vi "main4ChBK20240509.vi"() -> ()   [LabVIEW 2024]
doc: "Main VI for FLS imaging system."
uses:
  SubVI/DigitizerConfiguration/FLImDAQ.ctl
  <instrlib>/niScope/Controls/niScope trigger source.ctl
  SubVI/LabJack/LJ Pin Setting.ctl
  ConfigFiles/AimingBeamVideoConfig.ctl
  LaguerreDeconLib/DeconEngineClass/LaguerreDeconEngineClass.lvclass/LaguerreDeconEngineClass.ctl
  <vilib>/Utility/error.llb/DialogType.ctl
  LaguerreDeconLib/DeconEngineClass/LaguerreDeconEngineClass.lvclass
  <vilib>/event_ctls.llb/usereventprio.ctl
  <vilib>/Utility/miscctls.llb/LVMinMaxIncTypeDef.ctl
  SubVI/APD/APDClass.lvclass
  <vilib>/Analysis/baseanly.llb/Mean (DBL).vi
  SubVI/GlobalVariables.vi
  <vilib>/addons/control/pid/pid.llb/PID (DBL).vi
  <instrlib>/niScope/Acquire/Fetch/niScope Multi Fetch Binary 16.vi
  <vilib>/Instr/_visa.llb/VISA Configure Serial Port (Instr).vi
  <userlib>/_OpenG.lib/file/file.llb/openg_file.lvlib
  <userlib>/_OpenG.lib/time/time.llb/openg_time.lvlib
  <vilib>/Analysis/NI_AALBase.lvlib
  <vilib>/Utility/miscctls.llb/LVPointTypeDef.ctl
  <vilib>/addons/control/pid/NI_PID_pid.lvlib
panel:
  out "Record Backlog 2":i32
  in  "Auto gain ch4":bool=TRUE caption="Auto gain ch3"
  in  "V 4":dbl caption="Gain 3" min=0.0 max=4.67 step=0.1
  out "Gain4":dbl
  out "Lifetime 4":dbl caption="Lifetime 3"
  out "IntR4":dbl format="%#_2g"
  out "SNR4":dbl format="%#_3g"
  out "Channel 4":dbl[][](graph) caption="Channel 3"
  out "RunStartTime":u32
  out "Dig1 Temp":dbl
  out "Dig2 Temp":dbl
  out "Visualization PC video source":T1
  in  "V target(1.0)":dbl=1.0 caption="V target(1.5)" min=0.3 max=1.5 step=0.1 format="%#_4g"
  out "SNR3":dbl format="%#_3g"
  out "SNR2":dbl format="%#_3g"
  out "SNR1":dbl format="%#_3g"
  in  "Show BG removed?":bool=TRUE
  out "IntR3":dbl format="%#_2g"
  out "IntR2":dbl format="%#_2g"
  out "IntR1":dbl format="%#_2g"
  in  "Video Display":bool
  out "Gain3":dbl
  out "Gain2":dbl
  out "Gain1":dbl
  in  "Skip Data Save?":bool
  out "Aq Loop?":bool
  out "ML?":bool
  out "aquisition loop Error Out":errorcluster
  out "Laser f (Hz)":dbl
  out "Record Backlog":i32
  out "Fetch Record #":i32
  out "Sync Success?":bool
  out "Disclamer":picture
  out "Calibration #":i8
  out "BG #":i8
  in  "TCP Connect":bool
  out "Help":string
  in  "355nm Laser toggle":bool caption="355nm 460Hz"
  in  "Cali&iRF alignment":bool
  in  "Background":bool
  in  "Aiming beam toggle":bool caption="445nm 0Hz 18mA"
  out "Lifetime 3":dbl
  out "Lifetime 2":dbl
  in  "Auto gain ch3":bool=TRUE
  in  "Auto gain ch2":bool=TRUE
  in  "Auto gain ch1":bool=TRUE
  out "Run #":i8
  in  "StopButton":bool caption="Stop"
  out "Aquisition Status:":bool
  in  "StartButton":bool caption="Start"
  in  "V 3":dbl caption="Gain 3" min=0.0 max=4.68 step=0.1
  in  "V 2":dbl caption="Gain 2" min=0.0 max=4.62 step=0.1
  out "Lifetime 1":dbl
  in  "V 1":dbl caption="Gain 1" min=0.0 max=4.66 step=0.1 format="%#_4g"
  in  "Video Source":enum32{"Camera", "FrameGrabber"}(radio)
  out "Case #":string
  out "System Hardware Connection Status":T2
  out "Channel 3":dbl[][](graph)
  out "Channel 2":dbl[][](graph)
  out "Channel 1":dbl[][](graph)
  in  "Tab Control":T3(tab)
  out "display loop timing(ms)":u32
  out "Aquisition loop timing(ms)":u32 format="%.2f"
  out "DisplayLoop":i32
  out "PID loop":i32 caption="processing loop"
  out "PID loop timing(ms)":u32 caption="processing loop timing(ms)"
  out "Communication loop(ms)":u32
  out "laser EM lamp V":dbl format="%0.6f"
  out "Decon Loop timing (ms)":dbl
  out "Auisition Loop idx":i32
  out "LJ process (ms)":u32
  out "LJ time(ms)":u32[](array[numeric])
  out "output variable":i32
  out "Lifetime (ns)":dbl(graph)
  out "Waveform Chart":dbl(graph)
  in  "Truncation":u32=600
  out "iRF Graph":dbl[][](graph)
  in  "Show BG":bool
  out "iRF length":i32
  out "BG length":i32
  out "data length":i32
  out "SysConfigCluster":T4
  out "LJ Pinout":T5={"Ch1 Bias"="DAC0", "Ch2 Bias"="DAC1", "Ch3 Bias"="DAC2", "Ch4 Bias"="DAC0", "355 PWM"="FIO0", "AimingBeam PWM"="FIO2", "Laser Ready"="FIO3", "Interlock"="FIO1", "Laser Start/Stop"="FIO1", "Red LED"="FIO1", "Green LED"="DIO3", "Foot Pedal"="DIO15"}
  out "FLImDAQ":T6={"Digitizer 1"="", "Digitizer 2"="", "Channel"=enum."Channel 0", "trigger source"="VAL_EXTERNAL", "trigger level"=0.5, "trigger delay"=1.35e-07, "min sample rate"=12500000000.0, "min record length"=2500, "vertical range"=1.0, "vertical offset"=-0.25, "Waveform to Avg"=2000} caption="FLIm DAQ Configuration" {"trigger delay" format="%^#.4e"; "trigger level" min=0.0 max=3.5 step=0.5 format="%.2f"; "vertical offset" format="%.4f"; "vertical range" format="%.2f"; "min sample rate" format="%#.2p"}
  in  "Sys Reconfig":bool
  out "data out(communcation loop)":string
  out "PID loop error out":errorcluster caption="processing Error Out"
  out "decon error out":errorcluster
  out "Laser Rep Rate":dbl
  out "V4 Size":i32 caption="V3 Size"
  in  "Data Class":enum16{"Data", "BG", "Cali"}(ring)
  out "V1 Size":i32
  out "V2 Size":i32
  out "V3 Size":i32
  out "data Size":i32[](array[numeric])
  out "State log":string
  in  "Ch4 PID gains":T8={"proportional gain (Kc)"=30.0, "integral time (Ti, min)"=0.0003, "derivative time (Td, min)"=1e-05}
  in  "Ch3 PID gains":T8={"proportional gain (Kc)"=30.0, "integral time (Ti, min)"=0.0003, "derivative time (Td, min)"=1e-05}
  in  "Ch2 PID gains":T8={"proportional gain (Kc)"=30.0, "integral time (Ti, min)"=0.0003, "derivative time (Td, min)"=1e-05}
  in  "Ch1 PID gains":T8={"proportional gain (Kc)"=30.0, "integral time (Ti, min)"=0.0003, "derivative time (Td, min)"=1e-05}
  in  "Quit":bool
  in  "Radio Buttons":T9(radio)=enum."Ch2" caption="DeCon Chan"
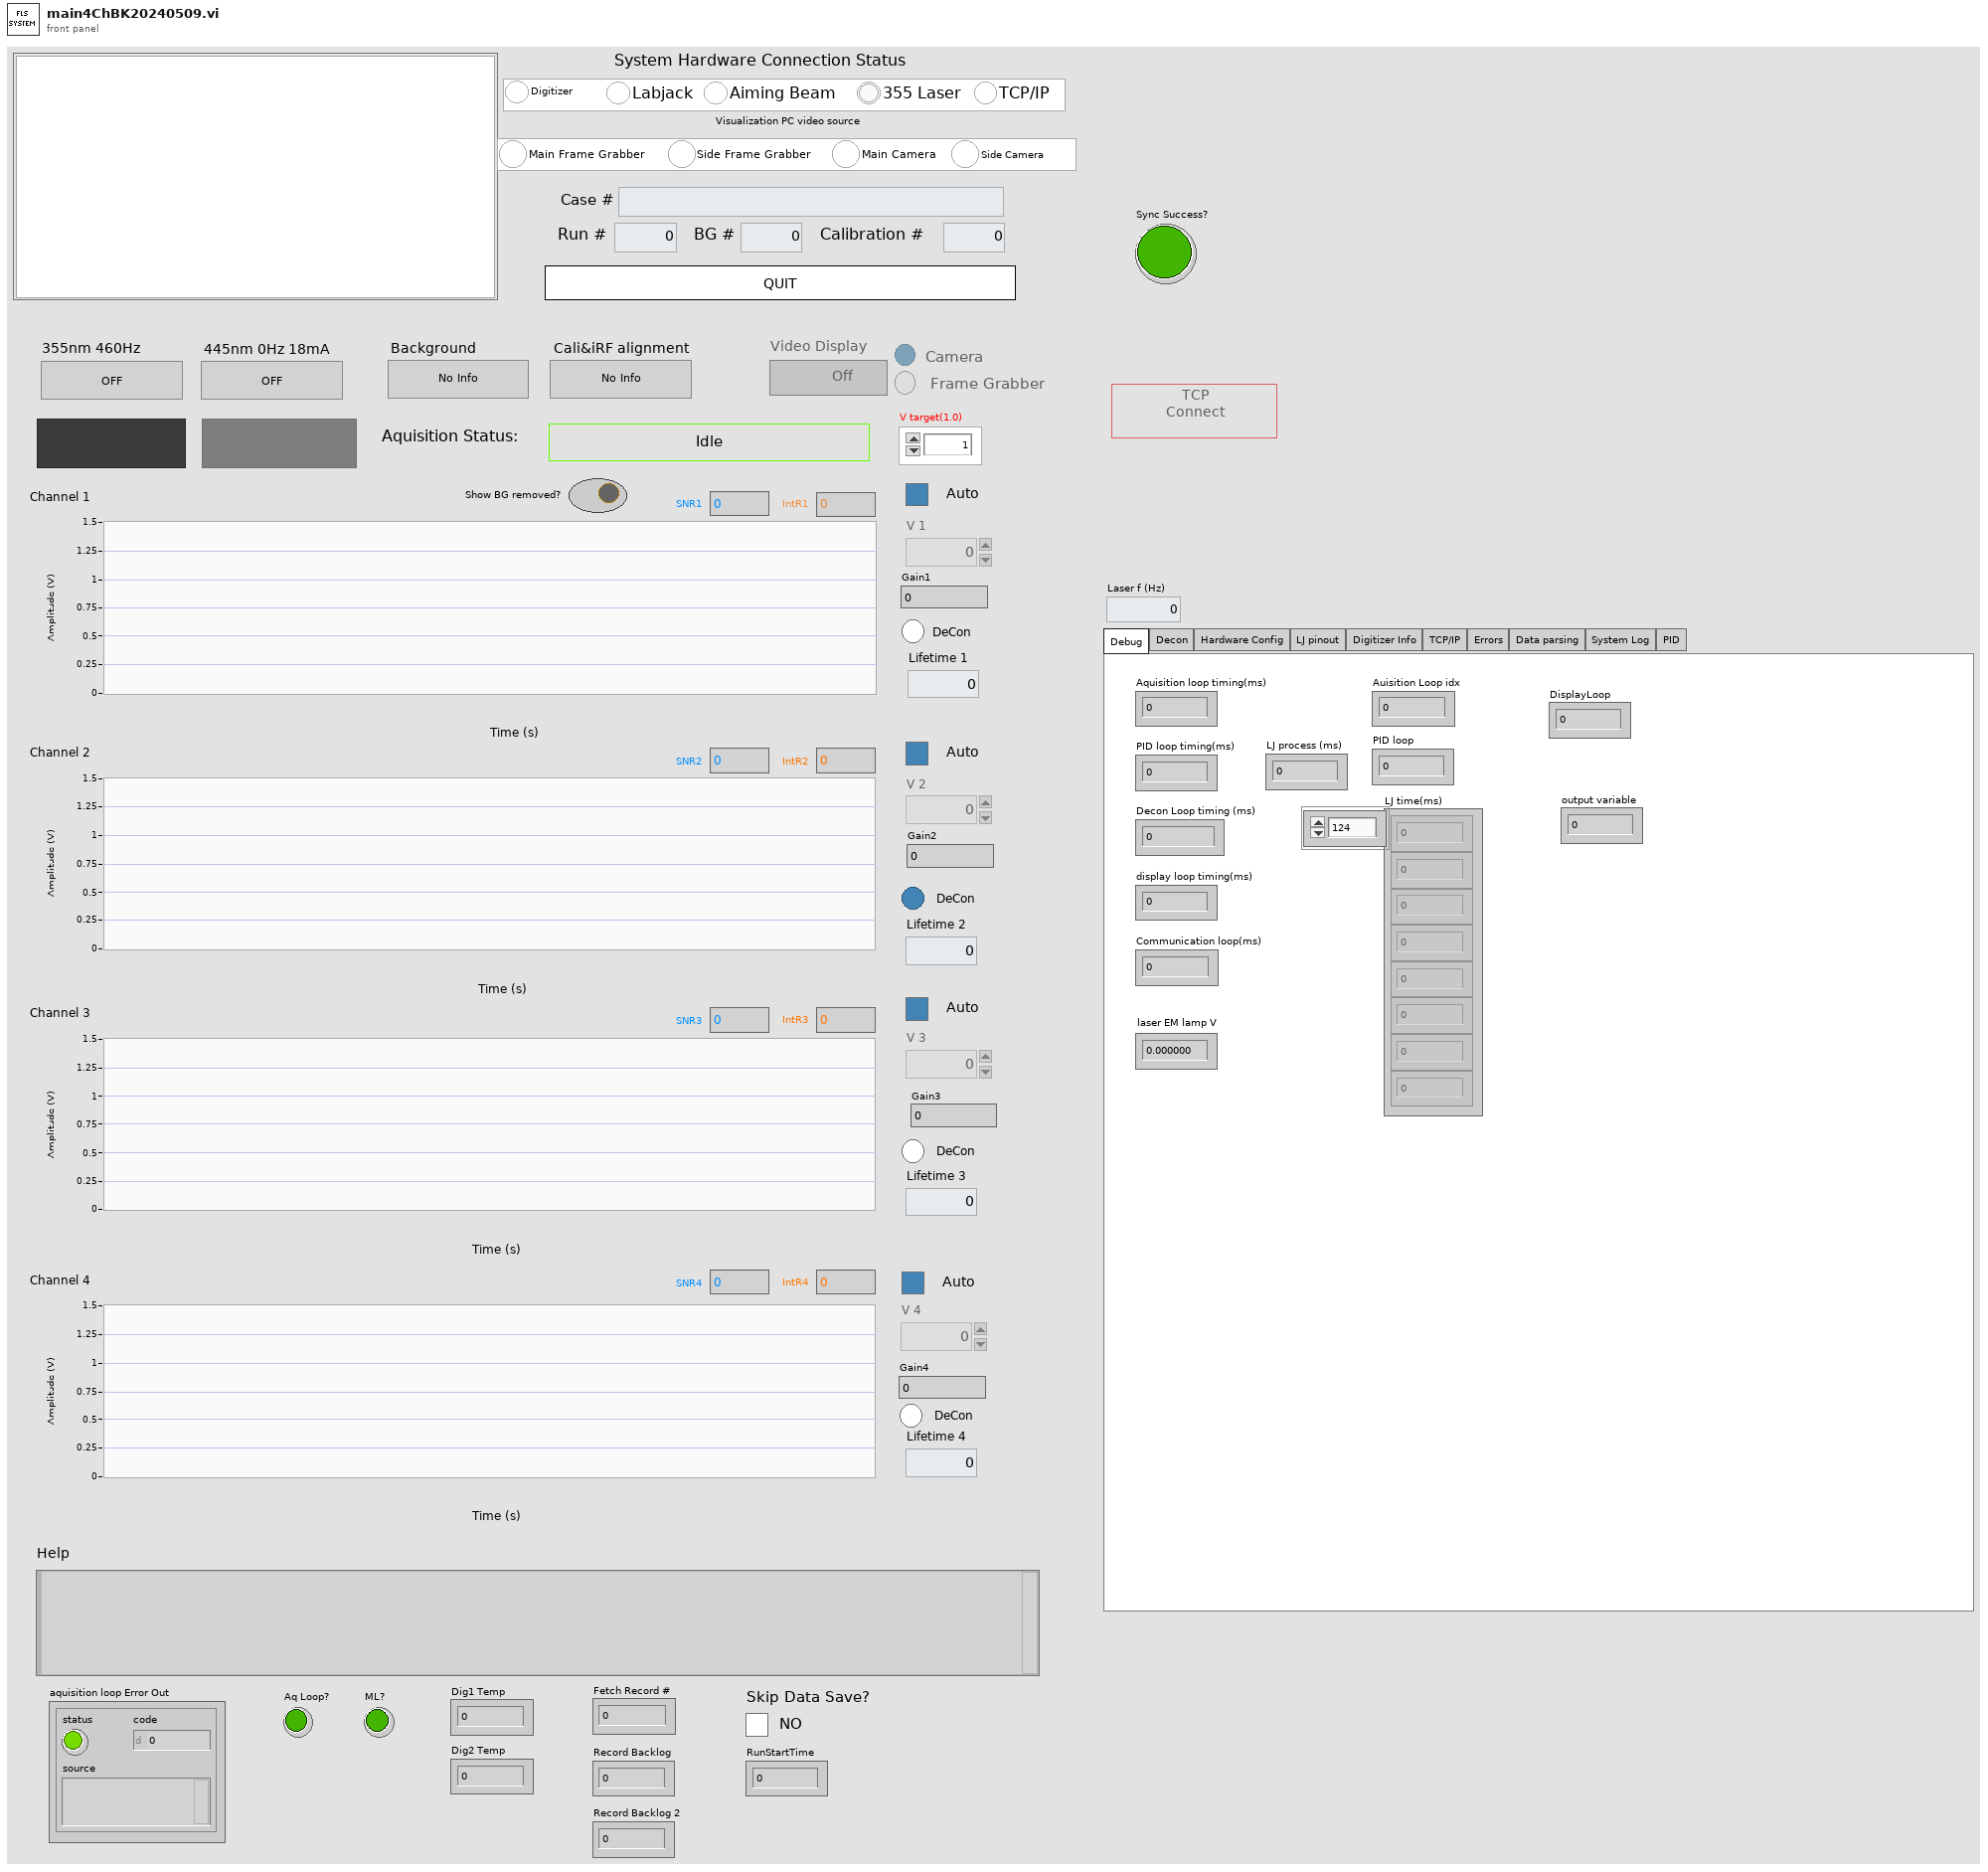
[diagram p1: front panel]
types:
  T1 = cluster{"Main Frame Grabber":bool, "Side Frame Grabber":bool, "Main Camera":bool, "Side Camera":bool}
  T2 = cluster{"Digitizer":bool, "Labjack":bool, "Aiming Beam":bool, "355 Laser":bool, "TCP/IP":bool}
  T3 = enum32{"Debug", "Decon", "Hardware Config", "LJ pinout", "Digitizer Info", "TCP/IP", "Errors", "Data parsing", "System Log", "PID"}
  T4 = cluster{"Ch1Enable?":bool, "Ch2Enable?":bool, "Ch3Enable?":bool, "Ch1AutoGain?":bool, "Ch2AutoGain?":bool, "Ch3AutoGain?":bool, "AimingBeamEnable?":bool}
  T5 = typedef "LJ Pin Setting.ctl" = cluster{"Ch1 Bias":string, "Ch2 Bias":string, "Ch3 Bias":string, "Ch4 Bias":string, "355 PWM":string, "AimingBeam PWM":string, "Laser Ready":string, "Interlock":string, "Laser Start/Stop":string, "Red LED":string, "Green LED":string, "Foot Pedal":string}
  T6 = typedef "FLImDAQ.ctl" = cluster{"Digitizer 1":refnum<k15>, "Digitizer 2":refnum<k15>, "Channel":enum16{"Channel 0", "Channel 1", "Channel 0&1"}, "trigger source":T7, "trigger level":dbl, "trigger delay":dbl, "min sample rate":dbl, "min record length":i32, "vertical range":dbl, "vertical offset":dbl, "Waveform to Avg":i16}
  T7 = typedef "niScope trigger source.ctl" = string
  T8 = cluster{"proportional gain (Kc)":dbl, "integral time (Ti, min)":dbl, "derivative time (Td, min)":dbl}
  T9 = enum32{"No Selection", "Ch1", "Ch2", "Ch3", "Ch4"}
  T10 = cluster{"remote start event":refnum<user-event>, "remote stop  event":refnum<user-event>}
  T11 = enum8{"Enabled", "Disabled", "Disabled and Grayed Out"}
  T12 = enum16{"open", "replace", "create", "open or create", "replace or create", "replace or create with confirmation"}
  T13 = cluster{"CH1":dbl[][], "CH2":dbl[][], "CH3":dbl[][], "CH4":dbl[][], "Gain cluster":cluster{"V1":dbl, "V2":dbl, "V3":dbl, "V4":dbl}}
  T14 = cluster{"idx":i32, "CH1&2":dbl[][], "CH3":dbl[][], "V cluster":cluster{"V1":dbl, "V2":dbl, "V3":dbl, "V4":dbl}}
  T15 = typedef "usereventprio.ctl" = enum32{"high priority", "normal priority"}
  T16 = cluster{"actualSamples":i32, "absoluteInitialX":dbl, "relativeInitialX":dbl, "xIncrement":dbl, "offset":dbl, "gain":dbl, "reserved1":dbl, "reserved2":dbl}[]
  T17 = cluster{"V1 out":dbl, "V2 out":dbl, "V3 out":dbl, "V3 out":dbl}
  T18 = cluster{i32, dbl[][], dbl[][], cluster{"V1 out":dbl, "V2 out":dbl, "V3 out":dbl, "V3 out":dbl}}
  T19 = cluster{"Ch1 iRF":dbl[], "Ch2 iRF":dbl[], "Ch3 iRF":dbl[], "Ch4 iRF":dbl[]}
  T20 = enum16{"open", "open or create", "create or replace", "create", "open (read-only)"}
  T21 = enum32{"Invalid", "Standard", "Closed", "Hidden", "Minimized", "Maximized"}
  T22 = enum32{"invalid app kind", "Development System", "Run Time System", "Student Edition", "Embedded LabVIEW", "Evaluation", "Custom"}
  T23 = enum32{"Bad", "Idle", "Run top level", "Running"}
  T24 = enum16{"Standard", "Buffered", "CRLF", "Immediate"}
  T25 = typedef "AimingBeamVideoConfig.ctl" = cluster{"DeCon Channel":enum16{"1", "2", "3"}, "Scale Bar":bool, "Scale Low":dbl, "Scale High":dbl, "ANSI":dbl, "Radius":dbl, "3D?":bool, "Firefly?":bool, "Pentero?":bool}
  T26 = cluster{"Core":cluster{"Current VI Reference":refnum<vi>, "Close Panel on Exit?":bool}, "SysConfigCluster":cluster{"Ch1Enable?":bool, "Ch2Enable?":bool, "Ch3Enable?":bool, "Ch1AutoGain?":bool, "Ch2AutoGain?":bool, "Ch3AutoGain?":bool, "AimingBeamEnable?":bool}, "System Status":cluster{"Digitizer":bool, "Labjack":bool, "Aiming Beam":bool, "355 Laser":bool, "TCP/IP":bool}, "IDs":cluster{"RunID":i8, "BG ID":i8, "Cali ID":i8}, "CaseID":string, "DefaultPath":path, "Pathes":cluster{"DataPath":path, "BG Path":path, "iRFPath":path, "CaliPath":path}, "FLImDAQ":cluster{"resource name":refnum<k15>, "resource name 2":refnum<k15>, "Channel":enum16{"Channel 0", "Channel 1", "Channel 0&1"}, "trigger source":T7, "trigger level":dbl, "trigger delay":dbl, "min sample rate":dbl, "min record length":i32, "vertical range":dbl, "vertical offset":dbl, "Waveform to Avg":i32}, "SysRunning?":bool, "AB Cluster":cluster{"Aiming Beam COM Port":refnum<visa-resource-name>, "Min Current":dbl, "Max Current":dbl, "Default Current":dbl, "Freq":i32}, "LJ Pinout":T5, "355 PWM setting":cluster{"DIO_EF_CLOCK1_DIVISOR":i16, "DIO_EF_CLOCK1_ROLL_VALUE":i32, "DIO#_EF_INDEX":i16, "DIO#_EF_OPTIONS":i16, "DIO#_EF_CONFIG_A":i32}, "AB PWM setting":cluster{"DIO_EF_CLOCK1_DIVISOR":i16, "DIO_EF_CLOCK1_ROLL_VALUE":i32, "DIO#_EF_INDEX":i16, "DIO#_EF_OPTIONS":i16, "DIO#_EF_CONFIG_A":i32}, "Last Trigger":u32, "niTClk sessions":refnum<k20>[], "Laser start tic":u32, "TCP attempt count":i32, "Ch1Data":dbl[][], "Ch2Data":dbl[][], "Ch3Data":dbl[][], "Ch4Data":dbl[][], "V1":dbl[], "V2":dbl[], "V3":dbl[], "V4":dbl[], "SlowTimer":u32, "FastTimer":u32, "listener ID":refnum<k5>, "TempPath":path, "CaliPath":path, "LED vi reference":refnum<vi>, "Aquisition Timer":u32, "APDSerialNum":cluster{"Ch1APDSerial#":string, "Ch2APDSerial#":string, "Ch3APDSerial#":string, "Ch4APDSerial#":string}, "VideoConfig":T25, "LED vi ref open?":bool, "video source":cluster{"Main Frame Grabber":bool, "Side Frame Grabber":bool, "Main Camera":bool, "Side Camera":bool}, "bothVidSourceAvail":bool}
  T27 = typedef "LVCursorListTypeDef.ctl" = cluster{"Name":string, "Color":u32, "Style":u8, "Point Style":u8, "Name Visible":bool, "Allow Drag":bool, "Cursor Mode":u32, "Plot":i32, "Index":i32, "Position":cluster{"X":dbl, "Y":dbl}, "X Scale":u32, "Y Scale":u32, "Watch Plots":i32[], "Watch All Plots":bool, "Plot Area":i32, "Label Offset":cluster{"X":dbl, "Y":dbl}}[]
  T28 = cluster{"Name":string, "Color":u32, "Style":u8, "Point Style":u8, "Name Visible":bool, "Allow Drag":bool, "Cursor Mode":u32, "Plot":i32, "Index":i32, "Position":cluster{"X":dbl, "Y":dbl}, "X Scale":u32, "Y Scale":u32, "Watch Plots":i32[], "Watch All Plots":bool, "Plot Area":i32, "Label Offset":cluster{"X":dbl, "Y":dbl}}
  T29 = cluster{"Ch1APDSerial#":string, "Ch2APDSerial#":string, "Ch3APDSerial#":string, "Ch4APDSerial#":string}
  T30 = cluster{"DataPath":path, "BG Path":path, "iRFPath":path, "CaliPath":path}
  T31 = cluster{"DIO_EF_CLOCK1_DIVISOR":i16, "DIO_EF_CLOCK1_ROLL_VALUE":i32, "DIO#_EF_INDEX":i16, "DIO#_EF_OPTIONS":i16, "DIO#_EF_CONFIG_A":i32}
  T32 = cluster{"Aiming Beam COM Port":refnum<visa-resource-name>, "Min Current":dbl, "Max Current":dbl, "Default Current":dbl, "Freq":i32}
  T33 = cluster{"resource name":refnum<k15>, "resource name 2":refnum<k15>, "Channel":enum16{"Channel 0", "Channel 1", "Channel 0&1"}, "trigger source":T7, "trigger level":dbl, "trigger delay":dbl, "min sample rate":dbl, "min record length":i32, "vertical range":dbl, "vertical offset":dbl, "Waveform to Avg":i32}
  T34 = cluster{"Current VI Reference":refnum<vi>, "Close Panel on Exit?":bool}
  T35 = cluster{"Channel 1":dbl[], "Channel 2":dbl[], "Channel 3":dbl[], "Channel 4":dbl[]}
  T36 = cluster{"V 1":dbl[], "V 2":dbl[], "V 3":dbl[], "V 4":dbl[]}
  T37 = cluster{"Ch1 WF":dbl[], "Ch2 WF":dbl[], "Ch3 WF":dbl[], "Ch4 WF":dbl[], "V1":dbl, "V2":dbl, "V3":dbl, "V4":dbl}
  T38 = typedef "iRFData.ctl" = cluster{"dt":dbl, "NumOfWFs":i32, "WFLength":i32, "iRFCtrlV":dbl[], "iRFWFsAvg":dbl[][], "iRFRaw":dbl[][]}
  T39 = cluster{"mean":dbl, "mean":dbl, "mean":dbl, "mean":dbl}
  T40 = cluster{"V1":dbl, "V2":dbl, "V3":dbl, "V4":dbl}[]
  T41 = cluster{"DataPath":path, "CaseID":string, "RunID":i16, "Ch1Data":dbl[][], "Ch2Data":dbl[][], "Ch3Data":dbl[][], "Ch4Data":dbl[][], "V1":dbl[], "V2":dbl[], "V3":dbl[], "V4":dbl[], "LaserRepRate":u16, "WFAverage":i16, "RunStartTime":u64}
  T42 = typedef "DialogType.ctl" = u16
  T43 = typedef "LJ PWM Setting.ctl" = cluster{"DIO_EF_CLOCK1_DIVISOR":i16, "DIO_EF_CLOCK1_ROLL_VALUE":i32, "DIO#_EF_INDEX":i16, "DIO#_EF_OPTIONS":i16, "DIO#_EF_CONFIG_A":i32}
  T44 = typedef "AimingBeam.ctl" = cluster{"Aiming Beam COM Port":refnum<visa-resource-name>, "Min Current":dbl, "Max Current":dbl, "Default Current":dbl, "Frequency(Hz)":u32}
  T45 = cluster{"DC1":i32, "DC2":i32, "BG1":i32, "BG2":i32}
  T46 = typedef "LVMinMaxIncTypeDef.ctl" = cluster{"Minimum":dbl, "Maximum":dbl, "Increment":dbl}
  T47 = typedef "LVBoundsTypeDef.ctl" = cluster{"Width":u32, "Height":u32}
  T48 = typedef "imagedata.ctl" = cluster{"image type":i32, "image depth":i32, "image":u8[], "mask":u8[], "colors":u32[], "Rectangle":cluster{"left":i16, "top":i16, "right":i16, "bottom":i16}}
  T49 = cluster{"DC Idx1":i32, "DC Idx2":i32, "BG Idx1":i32, "BG Idx2":i32}
  T50 = cluster{dbl[][], dbl[][], dbl[][], dbl[][], "V cluster":cluster{"V1":dbl, "V2":dbl, "V3":dbl, "V4":dbl}}
  T51 = typedef "LVPointTypeDef.ctl" = cluster{"Horizontal":i16, "Vertical":i16}
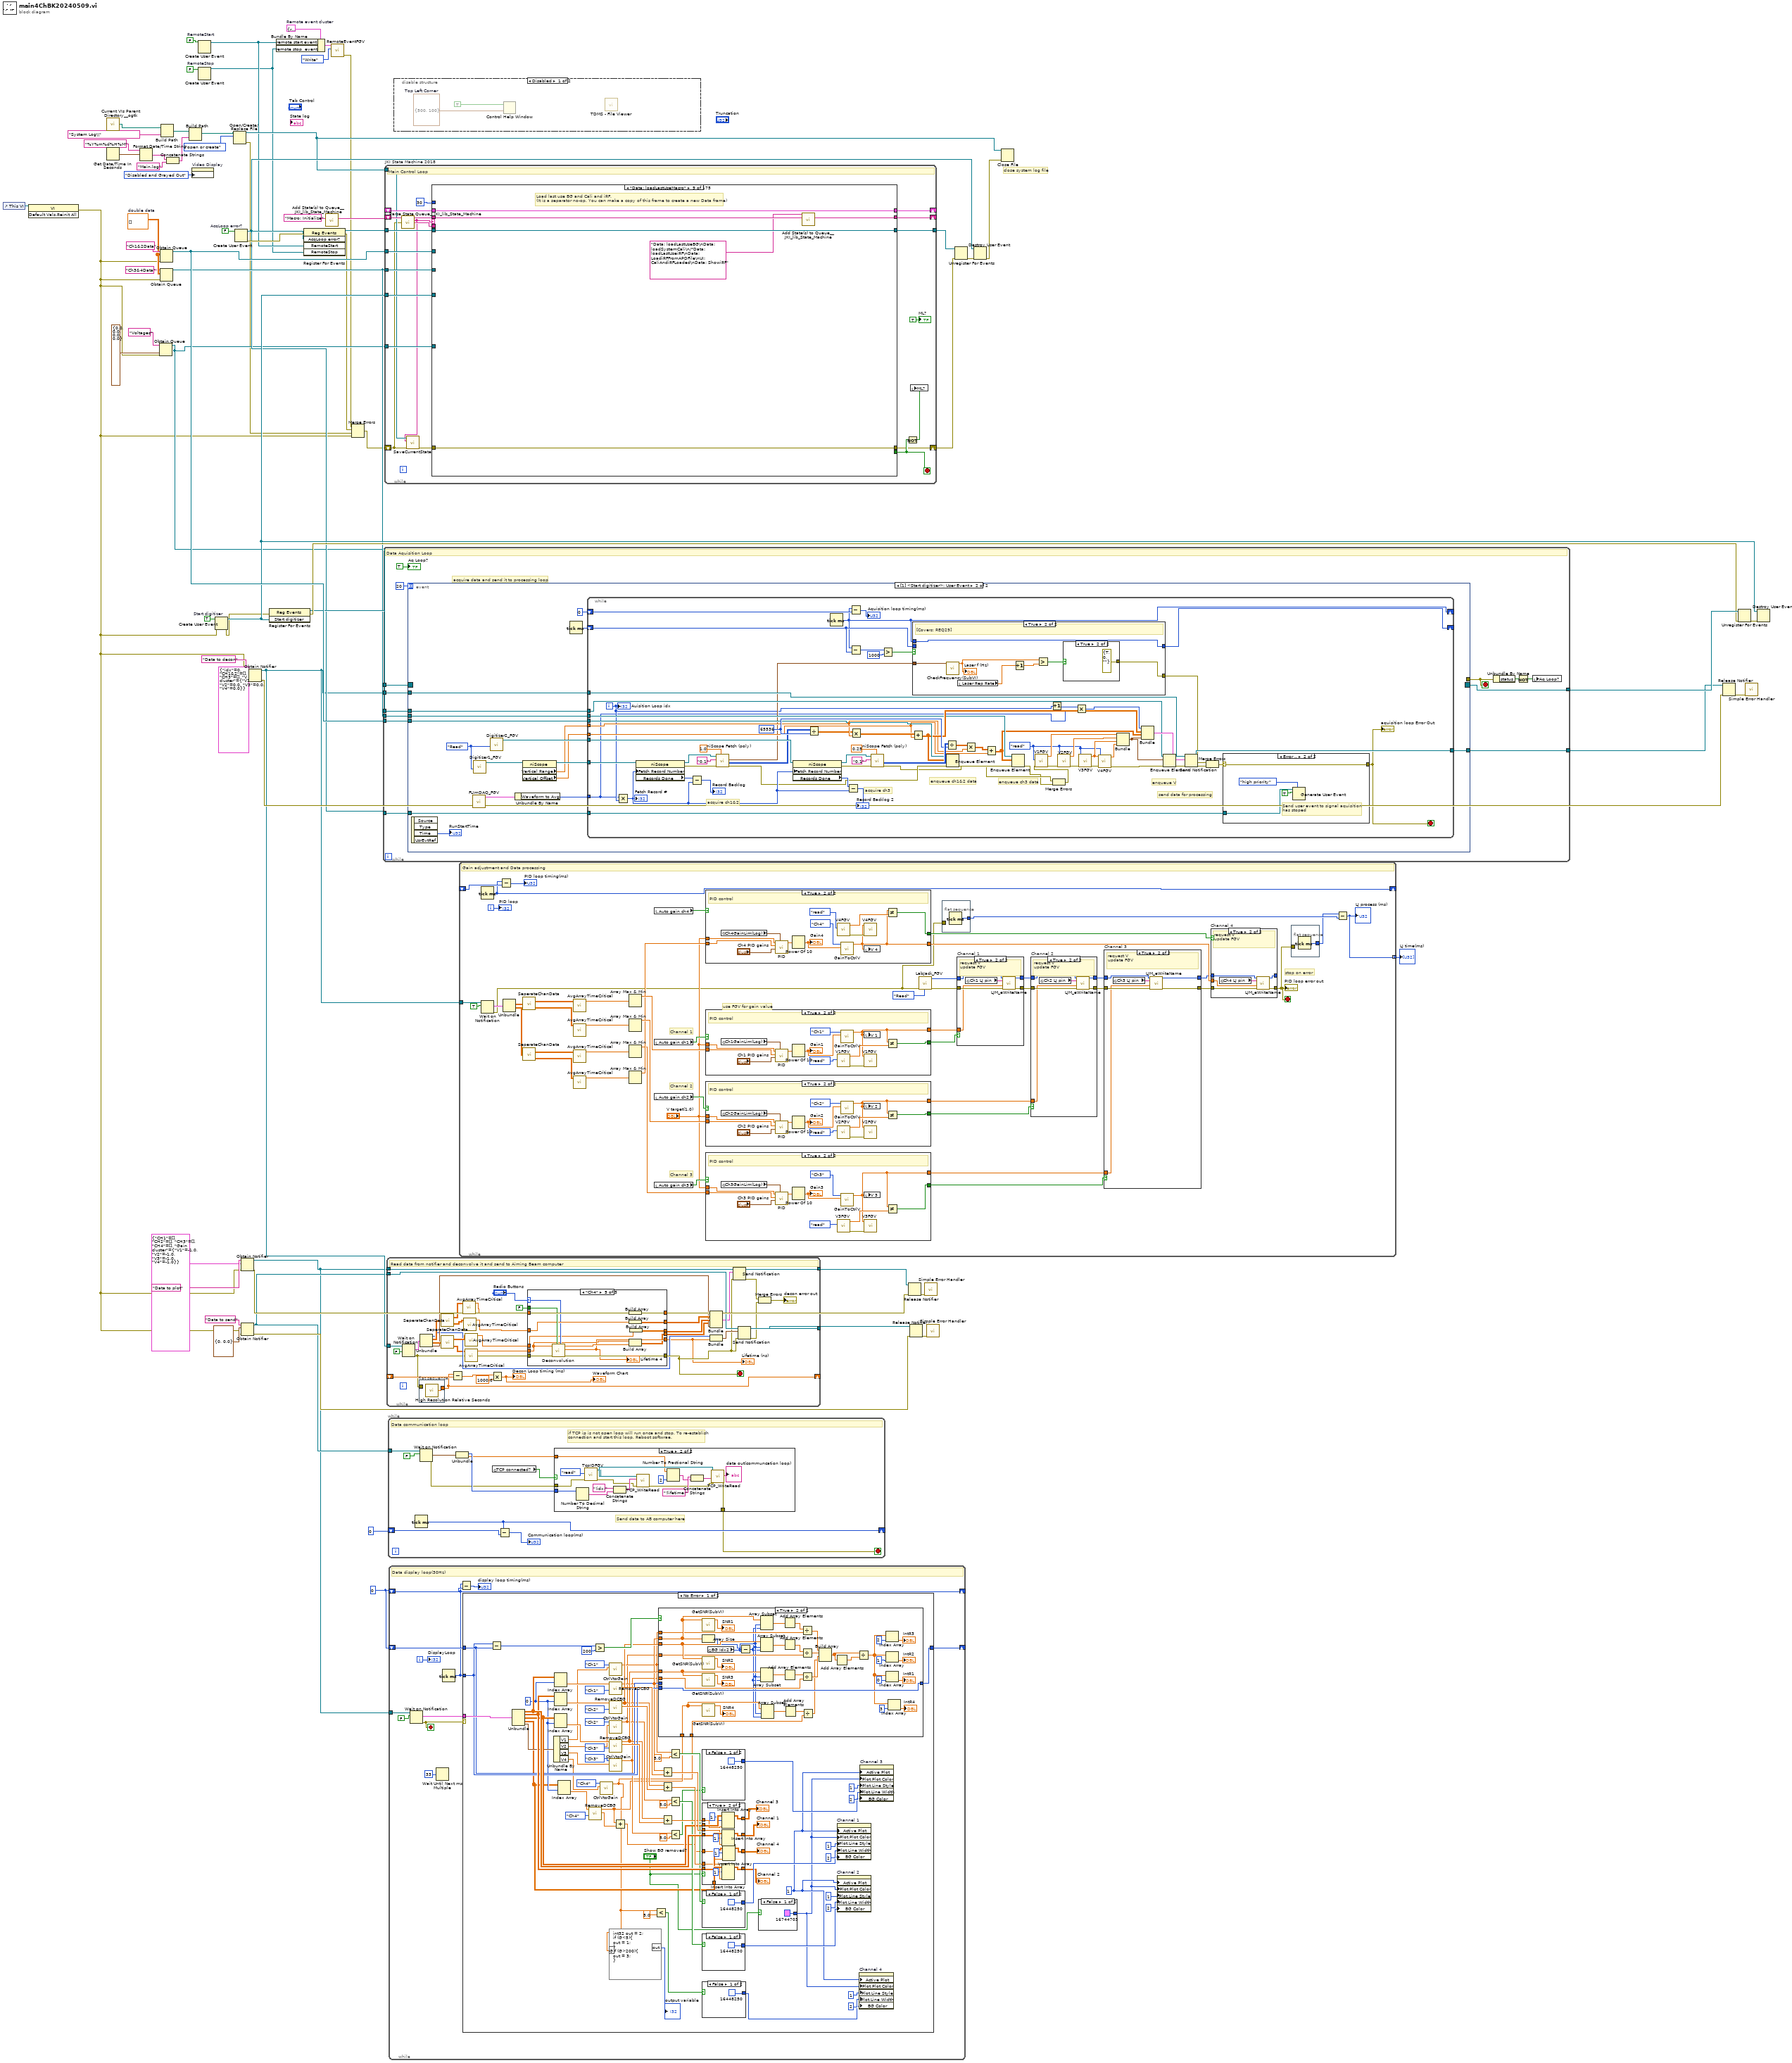
[diagram p0: block diagram]
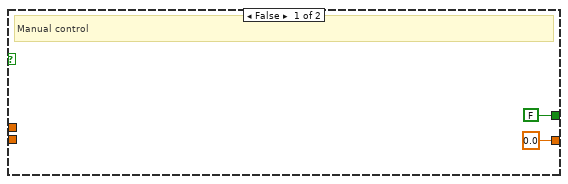
[diagram p6: hidden frame]
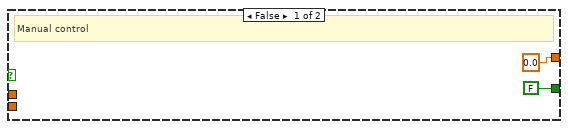
[diagram p7: hidden frame]
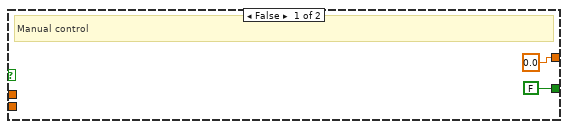
[diagram p8: hidden frame]
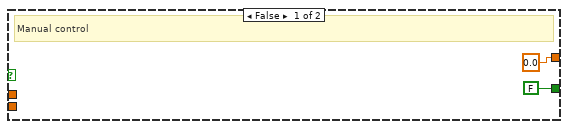
[diagram p9: hidden frame]
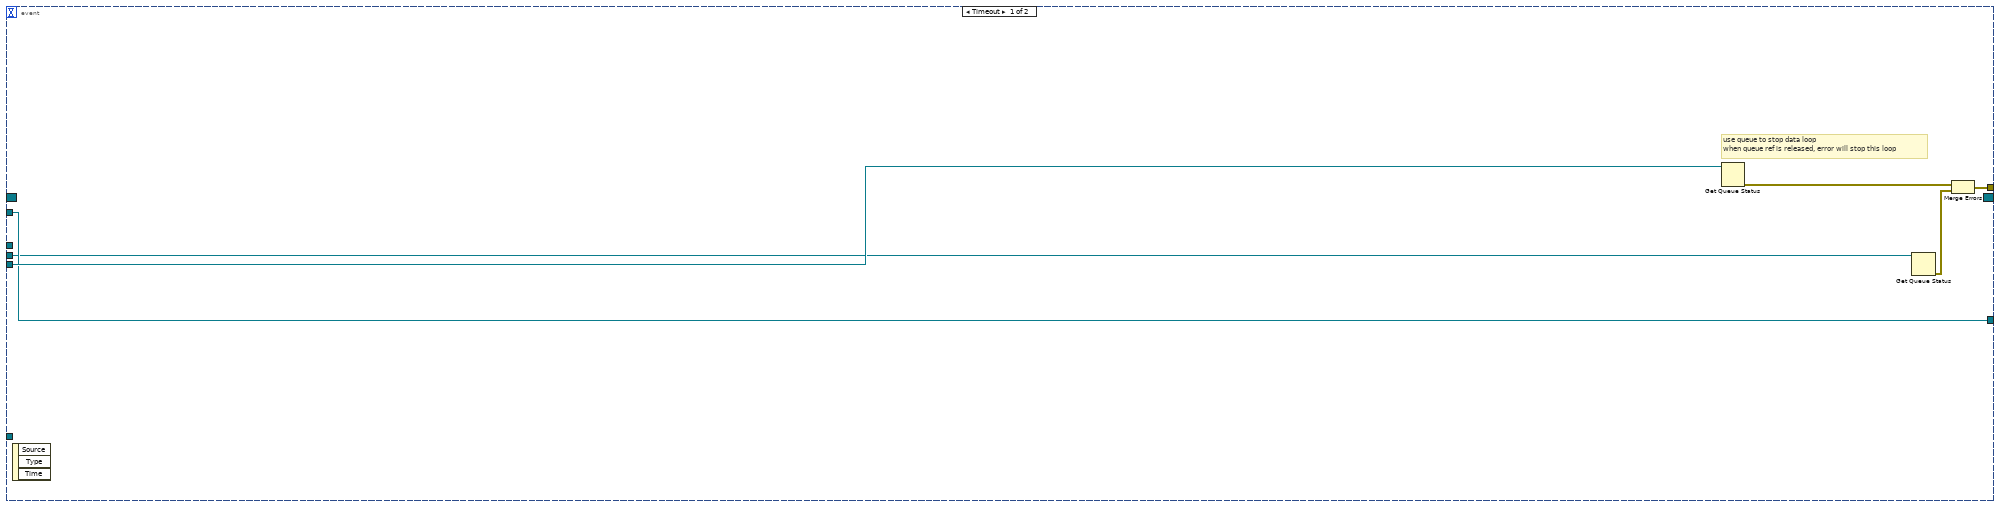
[diagram p10: hidden frame]
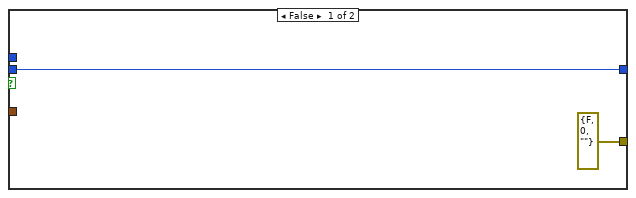
[diagram p11: hidden frame]
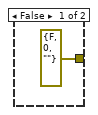
[diagram p12: hidden frame]
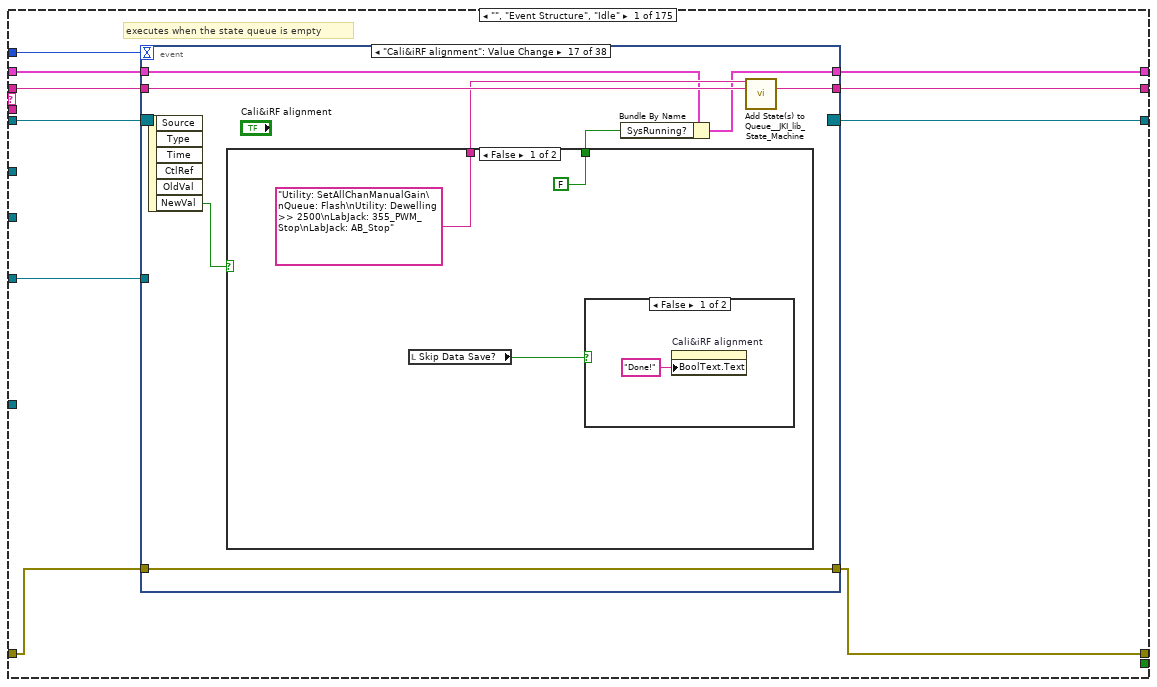
[diagram p14: hidden frame]
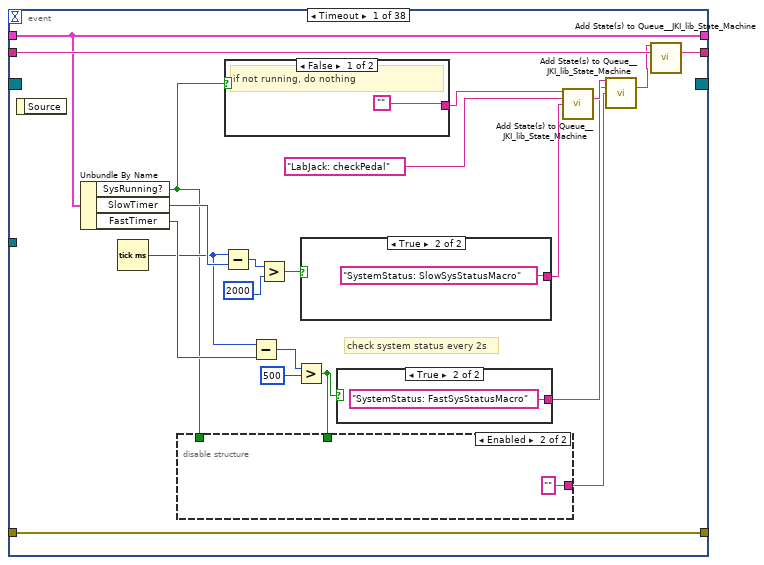
[diagram p15: hidden frame]
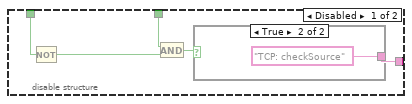
[diagram p16: hidden frame]
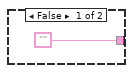
[diagram p17: hidden frame]
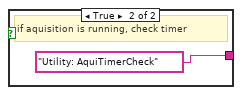
[diagram p18: hidden frame]
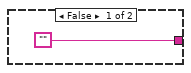
[diagram p19: hidden frame]
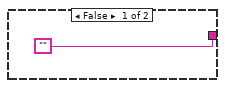
[diagram p20: hidden frame]
diagram:
  w8 = T10 {"remote start event"=refnum, "remote stop  event"=refnum}  # Remote event cluster
  w11 = FALSE  # RemoteStop
  w12 = FALSE  # RemoteStart
  w15 = u32 0 ("millisecond timer value")
  w54 = FALSE  # AcqLoop error?
  w64 = TRUE  # Start digitizer
  w67 = dbl[][] []  # double data
  # "close system log file"
  n1 = control-ref of="This VI"() -> (w69:refnum<vi>)
  n2 = invoke on="Invoke Node" class="VI" method="Default Vals.Reinit All"(reference=w69) -> (error out=w23:errorcluster)  [unwired: 2 in, 2 out]
  n3 = call <userlib>:"Current VIs Parent Directory__ogtk.vi"() -> ("Parent Directory (+ Relative)"=w34:path)  [unwired: 5 in]
  n4 = Get Date/Time In Seconds() -> (seconds since 1Jan1904=w32:timestamp)
  n5 = Format Date/Time String(time format string (%c)="%Y%m%d%H%M", seconds (now)=w32) -> (date/time string=w29:string)  [unwired: 1 in]
  n6 = Obtain Queue(name (unnamed)="Voltages", element data type=cluster{"V1":dbl, "V2":dbl, "V3":dbl, "V4":dbl} {"V1"=0.0, "V2"=0.0, "V3"=0.0, "V4"=0.0}, error in (no error)=w23) -> (queue out=w35:refnum<queue>)  [unwired: 2 in, 2 out]
  n7 = Obtain Queue(name (unnamed)="Ch3&4Data", element data type=w67, error in (no error)=w23) -> (queue out=w48:refnum<queue>)  [unwired: 2 in, 2 out]
  n8 = Obtain Queue(name (unnamed)="Ch1&2Data", element data type=w67, error in (no error)=w23) -> (queue out=w65:refnum<queue>)  [unwired: 2 in, 2 out]
  n9 = Build Path(base path=w34, name or relative path="System Log\\") -> (appended path=w25:path)
  n10 = Concatenate Strings(w29, "Main.log" ("string")) -> (w27:string)
  n11 = Build Path(base path=w25, name or relative path=w27) -> (appended path=w30:path)
  n12 = property on="Video Display" class="Bool (strict)"("DisabledEnum"=T11."Disabled and Grayed Out" ("Disabled")) -> ()  [unwired: 2 in, 2 out]
  n13 = Create User Event(user event datatype=w12) -> (user event=w10:refnum<user-event>)  [unwired: 1 in, 1 out]
  n14 = Create User Event(user event datatype=w11) -> (user event=w9:refnum<user-event>)  [unwired: 1 in, 1 out]
  n15 = Create User Event(user event datatype=w64, error in=w23) -> (user event=w53:refnum<user-event>, error out=w40:errorcluster)
  n16 = Open/Create/Replace File(file path (use dialog)=w30, operation (0:open)=T12."open or create") -> (refnum out=w21:refnum<file>, error out=w22:errorcluster)  [unwired: 4 in, 1 out]
  n17 = Create User Event(user event datatype=w54) -> (user event=w39:refnum<user-event>, error out=w41:errorcluster)  [unwired: 1 in]
  n18 = Obtain Notifier(name (unnamed)="Data to plot", notification data type=T13 {"CH1"=[], "CH2"=[], "CH3"=[], "CH4"=[], "Gain cluster"={"V1"=-1.0, "V2"=-1.0, "V3"=-1.0, "V4"=-1.0}}, error in (no error)=w23) -> (notifier out=w13:refnum<notifier>, error out=w49:errorcluster)  [unwired: 1 in, 1 out]
  n19 = Obtain Notifier(name (unnamed)="Data to send", notification data type=cluster{"idx":i32, "lifetime":dbl} {"idx"=0, "lifetime"=0.0}, error in (no error)=w23) -> (notifier out=w18:refnum<notifier>, error out=w38:errorcluster)  [unwired: 1 in, 1 out]
  n20 = Obtain Notifier(name (unnamed)="Data to decon", notification data type=T14 {"idx"=0, "CH1&2"=[], "CH3"=[], "V cluster"={"V1"=0.0, "V2"=0.0, "V3"=0.0, "V4"=0.0}}, error in (no error)=w23) -> (notifier out=w19:refnum<notifier>, error out=w58:errorcluster)  [unwired: 1 in, 1 out]
  n21 = register-events(error in=w40, w53) -> (reference out=w55:refnum<event-registration>, error out=w61:errorcluster)  [unwired: 1 in]
  n22 = Bundle By Name(cluster=w8, "remote start event"=w10, "remote stop  event"=w9) -> (w6:T10)
  n23 = register-events(error in=w41, w39, w10, w9) -> (reference out=w47:refnum<event-registration>, error out=w5:errorcluster)  [unwired: 1 in]
  n24 = call <vilib>:"Add State(s) to Queue__JKI_lib_State_Machine.vi"("State(s) in (\"\")"="Macro: Initialize") -> ("States Out"=w71:string)  [unwired: 14 in]
  n25 = call "RemoteEventFGV.vi"("Operation (Read)"=enum16{"Read", "Write"}."Write", "Remote Event in"=w6) -> ("Error Out"=w2:errorcluster)  [unwired: 8 in, 1 out]
  n26 = Merge Errors(w2, w5, w22, w23) -> (w24:errorcluster)
  n27 = while {
    tunnel: w65 -> [w84]
    tunnel: w55 -> [w83]
    tunnel: [w82] -> w63
    tunnel: w19 -> [w81]
    tunnel: [w80] -> w59
    tunnel: w39 -> [w78]
    tunnel: w48 -> [w77]
    tunnel: w35 -> [w72]
    stop <- w75 stop-if-true
    # "acquire data and send it to processing loop"
    # "Data Aquisition Loop"
    n28 = event shown="[1] <Start digitizer>: User Event" {
      selector: w83 -> [_ _]
      dyn-events: [_ _] -> w82
      timeout: 20 -> [_ _]
      tunnel: w84 -> [w90 w100]
      tunnel: [w85 _] -> w75
      tunnel: w81 -> [w89 w107]
      tunnel: [w89 w106] -> w80
      tunnel: w78 -> [_ w104]
      tunnel: w77 -> [w88 w99]
      tunnel: w72 -> [_ w97]
      event Timeout {
        # "use queue to stop data loop\nwhen queue ref is released, error will stop this loop"
        n29 = event-data() -> ()  [unwired: 1 in, 3 out]
        n30 = Get Queue Status(queue=w90) -> (error out=w87:errorcluster)  [unwired: 2 in, 7 out]
        n31 = Get Queue Status(queue=w88) -> (error out=w86:errorcluster)  [unwired: 2 in, 7 out]
        n32 = Merge Errors(w87, w86) -> (w85:errorcluster)
      }
      event User Event {
        w105 = enum16{"Write", "Read"}."Read" ("Operation")
        n33 = event-data() -> ("Time"=→"RunStartTime":u32)  [unwired: 1 in, 3 out]
        n34 = call "FLImDAQ_FGV.vi"() -> ("Read data"=w102:T6)  [unwired: 10 in, 1 out]
        n35 = call "Digitizer1_FGV.vi"("Operation (Read)"=w105) -> ("Read data"=w96:refnum<k15>)  [unwired: 9 in, 1 out]
        n36 = call "Digitizer2_FGV.vi"("Operation (Read)"=w105) -> ("Read data"=w103:refnum<k15>)  [unwired: 9 in, 1 out]
        n37 = Unbundle By Name(w102) -> ("Waveform to Avg"=w101:i16)
        n38 = property on="Property Node" class="niScope"(reference=w96) -> (reference out=w95:refnum<k15>, "Vertical Range"=w94:dbl, "Vertical Offset"=w93:dbl)  [unwired: 1 in, 1 out]
        n39 = Tick Count (ms)() -> (millisecond timer value=w92:u32)
        n40 = while {
          tunnel: w107 -> [w169]
          tunnel: [w168] -> w106
          tunnel: w103 -> [w162]
          tunnel: w95 -> [w161]
          tunnel: w104 -> [w160]
          shift-right: [w129] -> _
          shift-left: u32 0 ("millisecond timer value") -> [w154]
          tunnel: w101 -> [w108]
          tunnel: w100 -> [w151]
          tunnel: w99 -> [w149]
          tunnel: w97 -> [w142]
          tunnel: w94 -> [w139]
          tunnel: w93 -> [w140]
          shift-right: [w134] -> _
          shift-left: w92 -> [w133]
          i -> [w111]
          stop <- w132 stop-if-true
          w122 = enum16{"write", "read"}."read" ("action")
          w155 = 65536
          # "enqueue V"
          # "enqueue ch3 data"
          # "enqueue ch1&2 data"
          # "acquire ch3"
          # "acquire ch1&2"
          # "send data for processing"
          n41 = Multiply(x=w108, y=w111) -> (x*y=w119:i32)
          "Fetch Record #" <- w119
          n42 = property on="Property Node" class="niScope"(reference=w161, "Fetch Record Number"=w119) -> (reference out=w173:refnum<k15>, error out=w172:errorcluster, "Records Done"=w141:i32)  [unwired: 1 in]
          n43 = Subtract(x=w141, y=w119) -> (x-y=→"Record Backlog":i32)
          n44 = call-poly <instrlib>:"niScope Fetch (poly).vi"("timeout"=1.0, "error in"=w172, "channels"="0,1", "instrument handle"=w173) -> ("error out"=w116:errorcluster, "wfm"=w117:i16[][], "wfm info"=w138:T16)  [unwired: 4 in, 1 out]
          n45 = property on="Property Node" class="niScope"(reference=w162, "Fetch Record Number"=w119) -> (reference out=w166:refnum<k15>, error out=w163:errorcluster, "Records Done"=w120:i32)  [unwired: 1 in]
          n46 = Divide(x=w117, y=w155) -> (x/y=w128:dbl[][])
          n47 = Tick Count (ms)() -> (millisecond timer value=w129:u32)
          n48 = Subtract(x=w120, y=w119) -> (x-y=→"Record Backlog 2":i32)
          n49 = Subtract(x=w129, y=w154) -> (x-y=→"Aquisition loop timing(ms)":u32)
          n50 = Subtract(x=w129, y=w133) -> (x-y=w137:u32)
          n51 = Multiply(x=w128, y=w139) -> (x*y=w159:dbl[][])
          n52 = call-poly <instrlib>:"niScope Fetch (poly).vi"("timeout"=0.25, "error in"=w163, "channels"="0,1", "instrument handle"=w166) -> ("error out"=w115:errorcluster, "wfm"=w156:i16[][])  [unwired: 4 in, 2 out]
          n53 = Greater?(x=w137, y=u32 1000) -> (0:w135:bool)
          n54 = Add(x=w159, y=w140) -> (x+y=w150:dbl[][])
          n55 = case shown="True" w135 {
            tunnel: w138 -> [_ w182]
            tunnel: w129 -> [_ w181]
            tunnel: [w175 w181] -> w134
            tunnel: w133 -> [w175 _]
            tunnel: [errorcluster {"status"=FALSE, "code"=0, "source"=""} ("error constant") w178] -> w130
            frame False {
            }
            frame True {
              # "[Covers: REQ29]"
              n56 = call "CheckFrequency(SubVI).vi"("wfm info"=w182) -> ("f (Hz)"=w180:dbl)  [unwired: 10 in]
              "Laser f (Hz)" <- w180
              n57 = local read "Laser Rep Rate"() -> (w177:dbl)
              n58 = Increment(x=w177) -> (x+1=w176:dbl)
              n59 = Greater?(x=w180, y=w176) -> (0:w179:bool)
              n60 = case shown="True" w179 {
                tunnel: [errorcluster {"status"=FALSE, "code"=0, "source"=""} ("error constant") errorcluster {"status"=TRUE, "code"=0, "source"=""} ("error constant")] -> w178
                frame False {
                }
                frame True {
                }
              }
            }
          }
          n61 = Divide(x=w156, y=w155) -> (x/y=w158:dbl[][])
          n62 = Enqueue Element(queue=w151, element=w150, error in (no error)=w116) -> (error out=w114:errorcluster)  [unwired: 1 in, 2 out]
          n63 = Multiply(x=w158, y=w139) -> (x*y=w157:dbl[][])
          n64 = Add(x=w157, y=w140) -> (x+y=w148:dbl[][])
          n65 = Enqueue Element(queue=w149, element=w148, error in (no error)=w115) -> (error out=w113:errorcluster)  [unwired: 1 in, 2 out]
          n66 = Increment(x=w111) -> (x+1=w110:i32)
          n67 = Merge Errors(w114, w113) -> (w112:errorcluster)
          n68 = call "V1FGV.vi"("Error In"=w112, "action (write)"=w122) -> ("Error Out"=w146:errorcluster, "V1 out"=w144:dbl)  [unwired: 8 in]
          n69 = call "V2FGV.vi"("Error In"=w146, "action(write)"=w122) -> ("Error Out"=w145:errorcluster, "V2 out"=w143:dbl)  [unwired: 8 in]
          n70 = Multiply(x=w110, y=w108) -> (x*y=w109:i32)
          n71 = call "V3FGV.vi"("Error In"=w145, "action(write)"=w122) -> ("Error Out"=w125:errorcluster, "V3 out"=w124:dbl)  [unwired: 8 in]
          n72 = call "V4FGV.vi"("Error In"=w125, "action(write)"=w122, "V3 in"=w124) -> ("Error Out"=w123:errorcluster, "V3 out"=w121:dbl)  [unwired: 7 in]
          n73 = Bundle("V1 out"=w144, "V2 out"=w143, "V3 out"=w124, "V3 out"=w121) -> (w127:T17)  [unwired: 1 in]
          n74 = Bundle(w109, w150, w148, w127) -> (w152:T18)  [unwired: 1 in]
          n75 = Enqueue Element(queue=w142, element=w127, error in (no error)=w123) -> (error out=w126:errorcluster)  [unwired: 1 in, 2 out]
          n76 = Send Notification(notification=w152, notifier=w169, error in (no error)=w126) -> (notifier out=w168:refnum<notifier>, error out=w131:errorcluster)
          n77 = Merge Errors(w130, w131) -> (w147:errorcluster)
          n78 = case shown="Error .." w147 {
            selector: w147 -> [w185 w186]
            tunnel: w160 -> [_ w189]
            tunnel: [w185 w186] -> w132
            frame No Error {
            }
            frame Error {
              # "Send user event to signal aquisition has stoped"
              n79 = Generate User Event(priority (normal)=usereventprio."high priority", user event=w189, event data cluster=TRUE ("event data")) -> ()  [unwired: 1 in, 2 out]
            }
          }
          "aquisition loop Error Out" <- w132
          "Auisition Loop idx" <- w111
        }
      }
    }
    n80 = Unbundle By Name(w75) -> ("status"=w74:bool)
    n81 = Not(x=w74) -> (.not. x?=w73:bool)
    n82 = local write "Aq Loop?"(w73) -> ()
    "Aq Loop?" <- TRUE ("Aq L?")
  }
  n83 = while "JKI State Machine 2018" {
    shift-right: [w206] -> _
    shift-left: _ -> [w205]
    shift-right: [w190] -> w4
    shift-left: w24 -> [w192]
    shift-right: [w207] -> _
    shift-left: w71 -> [w208]
    tunnel: w65 -> [w203]
    tunnel: w48 -> [w202]
    tunnel: w53 -> [w201]
    tunnel: w47 -> [w200]
    tunnel: [w199] -> w46
    tunnel: w35 -> [w195]
    tunnel: w21 -> [w194]
    stop <- w198 stop-if-true
    # "Main Control Loop"
    n84 = call <vilib>:"Parse State Queue__JKI_lib_State_Machine.vi"("State Queue"=w208, "Error In (no error)"=w192) -> ("Remaining States"=w210:string, "Current State"=w193:string, "Arguments"=w209:string)  [unwired: 11 in]
    n85 = call "SaveCurrentState.vi"("error in (no error)"=w192, "Current State"=w193, "Byte Stream File in"=w194) -> ("error out"=w191:errorcluster)  [unwired: 8 in]
    n86 = case shown="\"Data: loadLastUseMacro\"" w193 {
      selector: w193 -> [_ _ _ _ _ _ _ _ _ _ _ _ _ _ _ _ _ _ _ _ _ _ _ _ w1196 _ _ _ _ _ _ _ _ _ _ _ _ _ _ _ _ _ _ _ _ _ _ _ _ _ _ _ _ _ _ _ _ _ _ _ _ _ _ _ _ _ _ _ _ _ _ _ _ _ _ _ _ _ _ _ _ _ _ _ _ _ _ _ _ _ _ _ _ _ _ _ _ _ _ _ _ _ _ _ _ _ _ _ _ _ _ _ _ _ _ _ _ _ _ _ _ _ _ _ _ _ _ _ _ _ _ _ _ _ _ _ _ _ _ _ _ _ _ _ _ _ _ _ _ _ _ _ _ _ _ _ _ _ _ _ _ _ _ _ _ _ _ _ _ _ _ _ _ _ _]
      tunnel: w210 -> [w220 w628 w637 w643 w649 w671 w684 w726 w732 w759 w778 w849 w864 w899 w926 w958 w972 w1001 w1015 w1100 w1137 w1176 w1189 w1194 w1200 w1228 w1236 w1259 w1264 w1277 w1296 w1324 w1352 w1390 w1395 w1401 w1425 w1449 w1473 w1497 w1502 w1519 w1566 w1588 w1604 w1619 w1639 w1644 w1656 w1685 w1711 w1723 w1761 w1774 w1780 w1791 w1803 w1834 w1847 w1861 w1876 w1895 w1930 w1935 w1949 w1959 w1975 w1987 w1999 w2027 w2042 w2047 w2059 w2071 w2076 w2084 w2092 w2101 w2110 w2115 w2123 w2132 w2150 w2167 w2187 w2198 w2220 w2235 w2252 w2257 w2265 w2273 w2278 w2286 w2293 w2301 w2308 w2318 w2346 w2354 w2361 w2369 w2374 w2382 w2389 w2395 w2404 w2420 w2425 w2432 w2444 w2514 w2526 w2535 w2552 w2561 w2584 w2601 w2612 w2625 w2650 w2673 w2679 w2695 w2717 w2725 w2731 w2736 w2743 w2753 w2765 w2774 w2779 w2791 w2796 w2806 w2812 w2818 w2823 w2828 w2833 w2843 w2867 w2888 w2893 w2904 w2929 w2956 w2979 w2984 w2999 w3050 w3096 w3141 w3152 w3170 w3190 w3204 w3217 w3225 w3242 w3264 w3288 w3307 w3325 w3343 w3361 w3375 w3389 w3408 w3422 w3437 w3452 w3461 w3466]
      tunnel: w209 -> [_ _ _ _ _ _ _ _ _ _ _ _ _ _ _ _ _ _ _ _ _ _ _ _ _ _ _ _ _ _ _ _ _ _ _ _ _ _ _ _ _ _ _ _ _ _ _ _ _ _ _ _ _ _ _ _ w1801 _ _ _ _ _ _ _ _ _ _ _ _ _ _ _ _ _ _ _ _ _ _ _ _ _ _ _ _ _ _ _ _ _ _ _ _ _ _ _ _ w2309 _ _ _ _ _ _ _ _ _ _ _ w2427 w2438 _ _ _ _ w2558 _ _ _ _ _ w2669 _ _ _ _ _ _ w2738 _ _ _ _ _ _ w2802 _ _ _ _ _ _ _ _ _ _ _ _ _ _ _ _ _ _ _ _ _ _ _ _ _ _ _ _ _ _ _ _ _ _ _ _ _ _ _]
      tunnel: w205 -> [w218 w625 w633 w640 w646 w668 w681 _ w728 w755 w774 w846 w855 w896 w918 w949 w969 w998 w1012 w1061 w1129 w1164 w1184 w1191 w1198 w1221 w1233 w1257 w1261 w1265 w1286 w1316 w1344 w1386 w1392 w1398 w1406 w1430 w1455 w1479 w1499 w1512 w1556 w1585 w1589 w1616 w1636 w1641 w1645 w1674 w1701 w1716 w1744 w1772 w1777 w1784 w1799 w1817 w1842 w1853 w1871 w1888 w1913 w1932 w1945 w1953 w1972 w1984 w1996 w2015 w2031 w2044 w2057 w2069 w2073 w2078 w2085 w2097 w2106 w2112 w2119 w2129 w2137 w2154 w2182 w2188 w2217 w2228 w2250 w2254 w2258 w2266 w2275 w2284 w2290 w2298 w2305 w2315 w2343 w2351 w2358 w2366 w2371 w2376 w2387 w2392 w2398 w2417 w2422 w2430 w2440 w2511 w2516 w2529 w2550 w2559 w2574 w2598 w2609 w2619 w2643 w2670 w2676 w2688 w2713 w2722 w2728 w2733 w2740 w2747 w2761 w2771 w2776 w2788 w2793 w2799 w2809 w2815 w2820 w2825 w2830 w2840 w2865 w2886 w2890 w2902 w2927 w2954 w2977 w2981 w2992 w3044 w3092 w3138 w3148 w3165 w3185 w3199 w3213 w3219 w3237 w3259 w3283 w3302 w3320 w3338 w3356 w3370 w3384 w3403 w3417 w3432 w3449 w3459 w3463]
      tunnel: [w211 w626 w635 w641 w647 w669 w682 w724 w730 w751 w770 w823 w851 w897 w906 w938 w962 w989 w1013 w1037 w1126 w1163 w1185 w1192 w1202 w1225 errorcluster {"status"=FALSE, "code"=0, "source"=""} ("error out") w1256 w1262 w1275 w1294 w1308 w1331 w1388 w1393 w1399 w1407 w1431 w1456 w1480 w1500 w1503 w1548 w1579 w1593 w1617 w1627 w1642 w1648 w1672 w1700 w1715 w1731 w1766 w1778 w1789 w1793 w1808 w1837 w1849 w1867 w1887 w1904 w1933 w1937 w1955 w1970 w1982 w1994 w2017 w2032 w2045 w2049 w2066 w2074 w2082 w2090 w2094 w2103 w2113 w2116 w2125 w2140 w2162 w2181 w2192 w2210 w2232 w2248 w2255 w2263 w2271 w2276 w2283 w2291 w2299 w2306 w2316 w2344 w2352 w2359 w2367 w2372 w2380 w2386 w2393 w2401 w2418 w2423 w2428 w2441 w2512 w2520 w2532 w2542 w2555 w2575 w2599 w2608 w2621 w2645 w2671 w2677 w2685 w2707 w2723 w2729 w2734 w2741 w2751 w2763 w2772 w2777 w2789 w2794 w2804 w2810 w2816 w2821 w2826 w2831 w2841 w2855 w2879 w2891 w2895 w2914 w2946 w2971 w2982 w2986 w3045 w3093 w3139 w3147 w3167 w3187 w3201 w3215 w3221 w3239 w3261 w3285 w3304 w3322 w3340 w3358 w3372 w3386 w3405 w3419 w3433 w3450 w3457 w3464] -> w190
      tunnel: w191 -> [w217 w626 w635 w641 w647 w669 w682 w724 w730 w752 w768 w823 w850 w897 w907 w945 w962 w979 w1013 w1037 w1127 w1166 w1186 w1192 w1201 w1225 w1229 w1256 w1262 w1275 w1294 w1307 w1343 w1388 w1393 w1399 w1411 w1435 w1460 w1484 w1500 w1510 w1551 w1578 w1592 w1617 w1629 w1642 w1647 w1673 w1691 w1721 w1742 w1765 w1778 w1786 w1796 w1807 w1836 w1852 w1866 w1886 w1903 w1933 w1943 w1956 w1969 w1981 w1993 w2016 w2033 w2045 w2048 w2061 w2074 w2082 w2090 w2093 w2102 w2113 w2117 w2126 w2145 w2161 w2180 w2191 w2216 w2231 w2247 w2255 w2263 w2271 w2276 w2283 w2291 w2299 w2306 w2316 w2344 w2352 w2359 w2367 w2372 w2380 w2386 w2393 w2401 w2418 w2423 w2429 w2442 w2512 w2521 w2531 w2538 w2554 w2576 w2599 w2608 w2616 w2648 w2671 w2677 w2690 w2706 w2723 w2729 w2734 w2741 w2751 w2763 w2772 w2777 w2789 w2794 w2804 w2810 w2816 w2821 w2826 w2831 w2841 w2854 w2878 w2891 w2894 w2913 w2936 w2962 w2982 _ w3046 w3093 w3139 w3146 w3166 w3186 w3200 w3215 w3220 w3238 w3260 w3284 w3303 w3321 w3339 w3357 w3371 w3385 w3404 w3418 w3431 w3450 w3456 w3464]
      tunnel: [w219 w627 w636 w642 w648 w670 w683 w725 w731 w758 w777 w848 w863 w898 w925 w957 w971 w1000 w1014 w1099 w1136 w1175 w1188 w1193 w1199 w1227 w1235 w1258 w1263 w1276 w1295 w1323 w1351 w1389 w1394 w1400 w1424 w1448 w1472 w1496 w1501 w1518 w1565 w1587 w1603 w1618 w1638 w1643 w1655 w1684 w1710 w1722 w1760 w1773 w1779 w1790 w1802 w1833 w1846 w1860 w1875 w1894 w1929 w1934 w1948 w1958 w1974 w1986 w1998 w2026 w2041 w2046 w2058 w2070 w2075 w2083 w2091 w2100 w2109 w2114 w2122 w2131 w2149 w2166 w2186 w2197 w2219 w2234 w2251 w2256 w2264 w2272 w2277 w2285 w2292 w2300 w2307 w2317 w2345 w2353 w2360 w2368 w2373 w2381 w2388 w2394 w2403 w2419 w2424 w2431 w2443 w2513 w2525 w2534 w2551 w2560 w2583 w2600 w2611 w2624 w2649 w2672 w2678 w2694 w2716 w2724 w2730 w2735 w2742 w2752 w2764 w2773 w2778 w2790 w2795 w2805 w2811 w2817 w2822 w2827 w2832 w2842 w2866 w2887 w2892 w2903 w2928 w2955 w2978 w2983 w2998 w3049 w3095 w3140 w3151 w3169 w3189 w3203 w3216 w3224 w3241 w3263 w3287 w3306 w3324 w3342 w3360 w3374 w3388 w3407 w3421 w3436 w3451 w3460 w3465] -> w207
      tunnel: [_ _ _ _ _ _ _ _ _ _ _ _ _ _ _ _ _ _ _ _ _ _ _ _ _ _ _ TRUE _ _ _ _ _ _ _ _ _ _ _ _ _ _ _ _ _ _ _ _ _ _ _ _ _ _ _ _ _ _ _ _ _ _ _ _ _ _ _ _ _ _ _ _ _ _ _ _ _ _ _ _ _ _ _ _ _ _ _ _ _ _ _ _ _ _ _ _ _ _ _ _ _ _ _ _ _ _ _ _ _ _ _ _ _ _ _ _ _ _ _ _ _ _ _ _ _ _ _ _ _ _ _ _ _ _ _ _ _ _ _ _ _ _ _ _ _ _ _ _ _ _ _ _ _ _ _ _ _ _ _ _ _ _ _ _ _ _ _ _ _ _ _ _ _ _ _] -> w198
      tunnel: [w216 w625 w633 w640 w646 w668 w681 w699 w728 w755 w774 w846 w855 w896 w918 w949 w969 w998 w1012 w1061 w1130 w1165 w1184 w1191 w1198 w1226 w1233 w1257 w1261 w1266 w1287 w1317 w1345 w1387 w1392 w1398 w1406 w1430 w1455 w1479 w1499 w1512 w1557 w1585 w1590 w1616 w1637 w1641 w1646 w1674 w1701 w1720 w1744 w1772 w1777 w1787 w1799 w1817 w1842 w1853 w1871 w1888 w1913 w1932 w1946 w1953 w1972 w1984 w1996 w2015 w2031 w2044 w2057 w2069 w2073 w2079 w2086 w2098 w2107 w2112 w2120 w2130 w2138 w2160 w2169 w2193 w2218 w2229 w2250 w2254 w2259 w2267 w2275 w2284 w2290 w2298 w2305 w2315 w2343 w2351 w2358 w2366 w2371 w2376 w2387 w2392 w2398 w2417 w2422 w2430 w2440 w2511 w2517 w2530 w2550 w2559 w2574 w2598 w2609 w2620 w2644 w2670 w2676 w2689 w2713 w2722 w2728 w2733 w2740 w2748 w2761 w2771 w2776 w2788 w2793 w2799 w2809 w2815 w2820 w2825 w2830 w2840 w2865 w2886 w2890 w2902 w2927 w2954 w2977 w2981 w2997 w3043 w3092 w3138 w3148 w3165 w3185 w3199 w3213 w3219 w3237 w3259 w3283 w3302 w3320 w3338 w3356 w3370 w3384 w3403 w3417 w3434 w3449 w3459 w3463] -> w206
      tunnel: 30 ("Timeout") -> [w215 _ _ _ _ _ _ _ _ _ _ _ _ _ _ _ _ _ _ _ _ _ _ _ _ _ _ _ _ _ _ _ _ _ _ _ _ _ _ _ _ _ _ _ _ _ _ _ _ _ _ _ _ _ _ _ _ _ _ _ _ _ _ _ _ _ _ _ _ _ _ _ _ _ _ _ _ _ _ _ _ _ _ _ _ _ _ _ _ _ _ _ _ _ _ _ _ _ _ _ _ _ _ _ _ _ _ _ _ _ _ _ _ _ _ _ _ _ _ _ _ _ _ _ _ _ _ _ _ _ _ _ _ _ _ _ _ _ _ _ _ _ _ _ _ _ _ _ _ _ _ _ _ _ _ _ _ _ _ _ _ _ _ _ _ _ _ _ _ _ _ _ _ _ _]
      tunnel: w203 -> [_ _ _ _ _ _ _ _ _ _ _ _ _ _ _ _ _ _ _ _ w1134 _ _ _ _ _ _ _ _ _ _ _ _ _ _ _ _ _ _ _ _ _ _ _ _ _ _ _ _ _ _ _ _ _ _ _ _ _ _ _ _ _ _ _ _ _ _ _ _ _ _ _ w2054 w2065 _ _ _ _ _ _ _ _ _ _ _ _ _ _ _ _ _ _ _ _ _ _ _ _ _ _ _ _ _ _ _ _ _ _ _ _ _ _ _ _ _ _ _ _ _ _ _ _ _ _ _ _ _ _ _ _ _ _ _ _ _ _ _ _ _ _ _ _ _ _ _ _ _ _ _ _ _ _ _ _ _ _ _ _ _ _ _ _ _ _ _ _ _ _ _ _ _ _ _ _ _]
      tunnel: w202 -> [_ _ _ _ _ _ _ _ _ _ _ _ _ _ _ _ _ _ _ _ w1133 _ _ _ _ _ _ _ _ _ _ _ _ _ _ _ _ _ _ _ _ _ _ _ _ _ _ _ _ _ _ _ _ _ _ _ _ _ _ _ _ _ _ _ _ _ _ _ _ _ _ _ w2055 w2064 _ _ _ _ _ _ _ _ _ _ _ _ _ _ _ _ _ _ _ _ _ _ _ _ _ _ _ _ _ _ _ _ _ _ _ _ _ _ _ _ _ _ _ _ _ _ _ _ _ _ _ _ _ _ _ _ _ _ _ _ _ _ _ _ _ _ _ _ _ _ _ _ _ _ _ _ _ _ _ _ _ _ _ _ _ _ _ _ _ _ _ _ _ _ _ _ _ _ _ _ _]
      tunnel: w201 -> [w214 _ _ _ _ _ _ _ _ _ _ _ _ _ _ _ _ _ _ _ _ _ _ _ _ _ _ _ _ _ _ _ _ _ _ _ _ _ _ _ _ _ _ w1581 _ _ _ _ _ _ _ _ _ _ _ _ _ _ _ _ _ _ _ _ _ _ _ _ _ _ _ _ _ _ _ _ _ _ _ _ _ _ _ _ _ _ _ _ _ _ _ _ _ _ _ _ _ _ _ _ _ _ _ _ _ _ _ _ _ _ _ _ _ _ _ _ _ _ _ _ _ _ _ _ _ _ _ _ _ _ _ _ _ _ _ _ _ _ _ _ _ _ _ _ _ _ _ _ _ _ _ _ _ _ _ _ _ _ _ _ _ _ _ _ _ _ _ _ _ _ _ _ _ _ _]
      tunnel: w200 -> [w213 w624 w634 w639 w645 w660 w680 w709 w729 w757 w776 w847 w862 w895 w924 w956 w970 w999 w1011 w1098 w1135 w1174 w1183 w1190 w1195 w1213 w1232 w1255 w1260 w1274 w1293 w1322 w1342 w1385 w1391 w1397 w1405 w1429 w1454 w1478 w1498 w1507 w1531 w1586 w1602 w1615 w1624 w1640 w1654 w1683 w1709 w1714 w1759 w1764 w1776 w1783 w1792 w1804 w1835 w1851 w1865 w1885 w1900 w1931 w1947 w1957 w1973 w1985 w1997 w2025 w2028 w2043 w2056 w2063 w2072 w2081 w2089 w2096 w2105 w2111 w2121 w2124 w2136 w2155 w2170 w2189 w2215 w2233 w2249 w2253 w2261 w2269 w2274 w2282 w2289 w2297 w2304 w2314 w2342 w2350 w2357 w2362 w2370 w2379 w2385 w2391 w2400 w2412 w2421 w2426 w2437 w2510 w2515 w2527 w2537 w2553 w2582 w2597 w2610 w2622 w2646 w2666 w2674 w2687 w2715 w2720 w2726 w2732 w2739 w2750 w2762 w2770 w2775 w2787 w2792 w2803 w2808 w2814 w2819 w2824 w2829 w2839 w2864 w2885 w2889 w2901 w2926 w2953 w2976 w2980 w2996 w3048 w3094 w3135 w3150 w3168 w3188 w3202 w3214 w3223 w3240 w3262 w3286 w3305 w3323 w3341 w3359 w3373 w3387 w3406 w3420 w3435 w3448 w3458 w3462]
      tunnel: [w212 w624 w634 w639 w645 w660 w680 w709 w729 w757 w776 w847 w862 w895 w924 w956 w970 w999 w1011 w1098 w1135 w1174 w1183 w1190 w1195 w1213 w1232 w1255 w1260 w1274 w1293 w1322 w1342 w1385 w1391 w1397 w1405 w1429 w1454 w1478 w1498 w1507 w1531 w1586 w1602 w1615 w1624 w1640 w1654 w1683 w1709 w1714 w1759 w1764 w1776 w1783 w1792 w1804 w1835 w1851 w1865 w1885 w1900 w1931 w1947 w1957 w1973 w1985 w1997 w2025 w2028 w2043 w2056 w2063 w2072 w2081 w2089 w2096 w2105 w2111 w2121 w2124 w2136 w2155 w2170 w2189 w2215 w2233 w2249 w2253 w2261 w2269 w2274 w2282 w2289 w2297 w2304 w2314 w2342 w2350 w2357 w2362 w2370 w2379 w2385 w2391 w2400 w2412 w2421 w2426 w2437 w2510 w2515 w2527 w2537 w2553 w2582 w2597 w2610 w2622 w2646 w2666 w2674 w2687 w2715 w2720 w2726 w2732 w2739 w2750 w2762 w2770 w2775 w2787 w2792 w2803 w2808 w2814 w2819 w2824 w2829 w2839 w2864 w2885 w2889 w2901 w2926 w2953 w2976 w2980 w2996 w3048 w3094 w3135 w3150 w3168 w3188 w3202 w3214 w3223 w3240 w3262 w3286 w3305 w3323 w3341 w3359 w3373 w3387 w3406 w3420 w3435 w3448 w3458 w3462] -> w199
      tunnel: w195 -> [_ _ _ _ _ _ _ _ _ _ _ _ _ _ _ _ _ _ _ _ w1128 _ _ _ _ _ _ _ _ _ _ _ _ _ _ _ _ _ _ _ _ _ _ _ _ _ _ _ _ _ _ _ _ _ _ _ _ _ _ _ _ _ _ _ _ _ _ _ _ _ _ _ w2053 w2062 _ _ _ _ _ _ _ _ _ _ _ _ _ _ _ _ _ _ _ _ _ _ _ _ _ _ _ _ _ _ _ _ _ _ _ _ _ _ _ _ _ _ _ _ _ _ _ _ _ _ _ _ _ _ _ _ _ _ _ _ _ _ _ _ _ _ _ _ _ _ _ _ _ _ _ _ _ _ _ _ _ _ _ _ _ _ _ _ _ _ _ _ _ _ _ _ _ _ _ _ _]
      frame "", "Event Structure", "Idle" {
        # "executes when the state queue is empty"
        n87 = event shown="[16] \"Cali&iRF alignment\": Value Change" {
          selector: w213 -> [_ _ _ _ _ _ _ _ _ _ _ _ _ _ _ _ _ _ _ _ _ _ _ _ _ _ _ _ _ _ _ _ _ _ _ _ _ _]
          dyn-events: [_ _ _ _ _ _ _ _ _ _ _ _ _ _ _ _ _ _ _ _ _ _ _ _ _ _ _ _ _ _ _ _ _ _ _ _ _ _] -> w212
          timeout: w215 -> [_ _ _ _ _ _ _ _ _ _ _ _ _ _ _ _ _ _ _ _ _ _ _ _ _ _ _ _ _ _ _ _ _ _ _ _ _ _]
          tunnel: w220 -> [w240 w259 w267 w271 w275 w283 w289 w297 w305 w315 w322 w351 w371 w391 w411 w415 w422 w445 w459 w473 w487 w492 w495 w501 w508 w515 w521 w527 w533 w540 w553 w564 w576 w583 w587 w591 w607 w623]
          tunnel: [w241 w259 w266 w271 w274 w283 w289 w297 w305 w315 w321 w351 w371 w391 w411 w415 w421 w445 w459 w473 w487 w491 w494 w501 w509 w516 w520 w526 w533 w541 w554 w564 w577 w583 w587 w590 w608 w622] -> w219
          tunnel: w218 -> [w224 w257 w261 w269 w276 w282 w290 w298 w306 w313 w317 w349 w369 w389 w409 w413 w417 w444 w458 w472 w486 w488 w496 w499 w504 w511 w523 w528 w531 w535 w548 w562 w572 w581 w585 w592 w605 w620]
          tunnel: [w239 w258 w262 w270 w277 w281 w288 w296 w304 w314 w323 w350 w370 w390 w410 w414 w423 w442 w446 w469 w484 w490 w497 w500 w505 w512 w524 w529 w532 w539 w552 w563 w573 w582 w586 w593 w609 w621] -> w211
          tunnel: w217 -> [w239 w258 w262 w270 w277 w281 w288 w296 w304 w314 w323 w350 w370 w390 w410 w414 w423 w439 w448 w460 w476 w490 w497 w500 w505 w512 w524 w529 w532 w539 w552 w563 w575 w582 w586 w593 w609 w621]
          tunnel: [w224 w257 w261 w269 w276 w282 w290 w298 w306 w313 w318 w349 w369 w389 w409 w413 w418 w444 w458 w472 w486 w488 w496 w499 w506 w513 w523 w528 w531 w536 w549 w562 w578 w581 w585 w592 w606 w620] -> w216
          tunnel: w214 -> [_ _ _ _ _ _ _ _ _ _ _ _ _ _ _ _ _ _ _ _ _ _ _ _ _ _ _ _ _ _ _ _ _ _ _ _ _ _]
          event Timeout {
            # "check system status every 2s"
            n88 = event-data() -> ()  [unwired: 1 in, 1 out]
            n89 = Unbundle By Name(w224) -> ("SysRunning?"=w222:bool, "SlowTimer"=w238:u32, "FastTimer"=w232:u32)
            n90 = Tick Count (ms)() -> (millisecond timer value=w225:u32)
            n91 = Subtract(x=w225, y=w238) -> (x-y=w235:u32)
            n92 = case shown="False" w222 {
              tunnel: ["" "Utility: AquiTimerCheck" ("State(s) in Front (\"\")")] -> w230
              frame False {
                # "if not running, do nothing"
              }
              frame True {
                # "if aquisition is running, check timer"
              }
            }
            n93 = Subtract(x=w225, y=w232) -> (x-y=w233:u32)
            n94 = Greater?(x=w235, y=u32 2000) -> (0:w236:bool)
            n95 = Greater?(x=w233, y=u32 500) -> (0:w223:bool)
            n96 = disable-structure shown="Enabled" {
              disable-tunnel: w223 -> [w246 _]
              disable-tunnel: w222 -> [w245 _]
              disable-tunnel: [w242 "" ("State(s) at Back (\"\")")] -> w221
              frame Disabled {
                n97 = Not(x=w245) -> (.not. x?=w244:bool)
                n98 = And(x=w246, y=w244) -> (x .and. y?=w243:bool)
                n99 = case shown="True" w243 {
                  tunnel: ["" ("Empty String Constant") "TCP: checkSource" ("State(s) in Front (\"\")")] -> w242
                  frame False {
                  }
                  frame True {
                  }
                }
              }
              frame Enabled {
              }
            }
            n100 = case shown="True" w236 {
              tunnel: ["" ("Empty String Constant") "SystemStatus: SlowSysStatusMacro" ("State(s) in Front (\"\")")] -> w228
              frame False {
              }
              frame True {
              }
            }
            n101 = case shown="True" w223 {
              tunnel: ["" ("Empty String Constant") "SystemStatus: FastSysStatusMacro" ("State(s) in Front (\"\")")] -> w226
              frame False {
              }
              frame True {
              }
            }
            n102 = call <vilib>:"Add State(s) to Queue__JKI_lib_State_Machine.vi"("State(s) in Front (\"\")"=w230, "State(s) in (\"\")"="LabJack: checkPedal" ("State(s) in Front (\"\")"), "State(s) at Back (\"\")"=w228) -> ("States Out"=w227:string)  [unwired: 12 in]
            n103 = call <vilib>:"Add State(s) to Queue__JKI_lib_State_Machine.vi"("State(s) in Front (\"\")"=w227, "State(s) in (\"\")"=w226, "State(s) at Back (\"\")"=w221) -> ("States Out"=w231:string)  [unwired: 12 in]
            n104 = call <vilib>:"Add State(s) to Queue__JKI_lib_State_Machine.vi"("State(s) in Front (\"\")"=w231, "State(s) in (\"\")"=w240) -> ("States Out"=w241:string)  [unwired: 13 in]
          }
          event "355nm Laser toggle": Mouse Enter {
            n105 = event-data() -> ()  [unwired: 1 in, 4 out]
            n106 = local write "Help"("Toggle 355nm laser." ("Help")) -> ()
          }
          event "355nm Laser toggle": Value Change {
            # "[Covers: REQ34]"
            n107 = event-data() -> ()  [unwired: 1 in, 6 out]
            n108 = Select(t="LabJack: 355_PWM_Start\nLabJack: AB_Start", s="355nm Laser toggle", f="LabJack: 355_PWM_Stop\nLabJack: AB_Stop") -> (s? t:f=w264:string)
            n109 = call <vilib>:"Add State(s) to Queue__JKI_lib_State_Machine.vi"("State(s) in Front (\"\")"=w264, "State(s) in (\"\")"=w267) -> ("States Out"=w266:string)  [unwired: 13 in]
          }
          event "Aiming beam toggle": Mouse Enter {
            n110 = event-data() -> ()  [unwired: 1 in, 4 out]
            n111 = local write "Help"("Toggle aiming beam laser." ("Help")) -> ()
          }
          event "Aiming beam toggle": Value Change {
            # "[Covers: REQ33]"
            n112 = event-data() -> ()  [unwired: 1 in, 6 out]
            n113 = case shown="True" "Aiming beam toggle" {
              tunnel: ["LabJack: AB_Stop" ("State(s) in Front (\"\")") "LabJack: AB_Start" ("State(s) in Front (\"\")")] -> w273
              frame False {
              }
              frame True {
              }
            }
            n114 = call <vilib>:"Add State(s) to Queue__JKI_lib_State_Machine.vi"("State(s) in Front (\"\")"=w273, "State(s) in (\"\")"=w275) -> ("States Out"=w274:string)  [unwired: 13 in]
          }
          event "Auto gain ch1": Value Change {
            n115 = event-data() -> ("NewVal"=w280:bool)  [unwired: 1 in, 5 out]
            n116 = case shown="True" w280 {
              frame False {
                n117 = local read "V 1"() -> (w284:dbl)
                n118 = call "V1FGV.vi"("action (write)"=enum16{"write", "read"}."write" ("action"), "V1 in"=w284) -> ()  [unwired: 8 in, 2 out]
                n119 = property on="V 1" class="DigNum (strict)"("DisabledEnum"=T11."Enabled" ("Disabled")) -> ()  [unwired: 2 in, 2 out]
              }
              frame True {
                n120 = property on="V 1" class="DigNum (strict)"("DisabledEnum"=T11."Disabled and Grayed Out" ("Disabled")) -> ()  [unwired: 2 in, 2 out]
              }
            }
          }
          event "Auto gain ch2": Value Change {
            n121 = event-data() -> ("NewVal"=w291:bool)  [unwired: 1 in, 5 out]
            n122 = case shown="False" w291 {
              frame False {
                n123 = local read "V 2"() -> (w292:dbl)
                n124 = property on="V 2" class="DigNum (strict)"("DisabledEnum"=T11."Enabled" ("Disabled")) -> ()  [unwired: 2 in, 2 out]
                n125 = call "V2FGV.vi"("action(write)"=enum16{"write", "read"}."write" ("action"), "V2 in"=w292) -> ()  [unwired: 8 in, 2 out]
              }
              frame True {
                n126 = property on="V 2" class="DigNum (strict)"("DisabledEnum"=T11."Disabled and Grayed Out" ("Disabled")) -> ()  [unwired: 2 in, 2 out]
              }
            }
          }
          event "Auto gain ch3": Value Change {
            n127 = event-data() -> ("NewVal"=w299:bool)  [unwired: 1 in, 5 out]
            n128 = case shown="False" w299 {
              frame False {
                n129 = local read "V 3"() -> (w300:dbl)
                n130 = property on="V 3" class="DigNum (strict)"("DisabledEnum"=T11."Enabled" ("Disabled")) -> ()  [unwired: 2 in, 2 out]
                n131 = call "V3FGV.vi"("action(write)"=enum16{"write", "read"}."write" ("action"), "V3 in"=w300) -> ()  [unwired: 8 in, 2 out]
              }
              frame True {
                n132 = property on="V 3" class="DigNum (strict)"("DisabledEnum"=T11."Disabled and Grayed Out" ("Disabled")) -> ()  [unwired: 2 in, 2 out]
              }
            }
          }
          event "Auto gain ch4": Value Change {
            n133 = event-data() -> ("NewVal"=w307:bool)  [unwired: 1 in, 5 out]
            n134 = case shown="False" w307 {
              frame False {
                n135 = local read "V 4"() -> (w308:dbl)
                n136 = property on="V 4" class="DigNum (strict)"("DisabledEnum"=T11."Enabled" ("Disabled")) -> ()  [unwired: 2 in, 2 out]
                n137 = call "V4FGV.vi"("action(write)"=enum16{"write", "read"}."write" ("action"), "V3 in"=w308) -> ()  [unwired: 8 in, 2 out]
              }
              frame True {
                n138 = property on="V 4" class="DigNum (strict)"("DisabledEnum"=T11."Disabled and Grayed Out" ("Disabled")) -> ()  [unwired: 2 in, 2 out]
              }
            }
          }
          event "Background": Mouse Enter {
            n139 = event-data() -> ()  [unwired: 1 in, 4 out]
            n140 = local write "Help"("Click to record a background." ("Help")) -> ()
          }
          event "Background": Value Change {
            n141 = event-data() -> ("NewVal"=w319:bool)  [unwired: 1 in, 5 out]
            n142 = case shown="True" w319 {
              tunnel: ["Utility: SetAllChanManualGain\nQueue: Flash\nUtility: Dewelling >> 2500\nLabJack: 355_PWM_Stop\nLabJack: AB_Stop" "Utility: SetDataClass >> Bg\nUI: Update\nLabJack: 355_PWM_Start\nLabJack: AB_Start\nUtility: SaveDeconChan\nUtility: Dewelling >> 50\nLabJack: SetV\nDigitizer: Start\nUtility: AquiTimerReset\nLED: BreathGreen\nUI: duringBGAcquire"] -> w320
              tunnel: [FALSE TRUE] -> w316
              frame False {
                n143 = local read "Skip Data Save?"() -> (w324:bool)
                n144 = case shown="False" w324 {
                  frame False {
                    n145 = property on="Background" class="Bool (strict)"("BoolText.Text"="Done!" ("Boolean Text.Text")) -> ()  [unwired: 2 in, 2 out]
                  }
                  frame True {
                  }
                }
              }
              frame True {
                # "[Covers: REQ6]"
                n146 = property on="Background" class="Bool (strict)"("BoolText.Text"="Running" ("Boolean Text.Text"), "Colors [4]"=cluster{u32, u32}[] [{6618880, 6618880}, {16711680, 16711680}]) -> ()  [unwired: 2 in, 2 out]
              }
            }
            n147 = Bundle By Name(cluster=w317, "SysRunning?"=w316) -> (w318:T26)
            n148 = call <vilib>:"Add State(s) to Queue__JKI_lib_State_Machine.vi"("State(s) in Front (\"\")"=w320, "State(s) in (\"\")"=w322) -> ("States Out"=w321:string)  [unwired: 13 in]
          }
          event "Channel 1": Cursor Move {
            n149 = event-data() -> ("CursIdx"=w335:i32, "CursLoc"=w347:cluster{"X":dbl, "Y":dbl})  [unwired: 1 in, 7 out]
            n150 = property on="Channel 3" class="WFGraph (strict)"() -> ("CrsrList"=w342:T27)  [unwired: 2 in, 2 out]
            n151 = property on="Channel 4" class="WFGraph (strict)"() -> ("CrsrList"=w334:T27)  [unwired: 2 in, 2 out]
            n152 = property on="Channel 2" class="WFGraph (strict)"() -> ("CrsrList"=w345:T27)  [unwired: 2 in, 2 out]
            n153 = Index Array(array=w342, index=w335) -> (element=w346:T28)
            n154 = Index Array(array=w334, index=w335) -> (element=w337:T28)
            n155 = Unbundle By Name(w347) -> ("X"=w336:dbl)
            n156 = Index Array(array=w345, index=w335) -> (element=w348:T28)
            n157 = Bundle By Name(cluster=w346, "Position.X"=w336) -> (w341:T28)
            n158 = Bundle By Name(cluster=w337, "Position.X"=w336) -> (w333:T28)
            n159 = Bundle By Name(cluster=w348, "Position.X"=w336) -> (w344:T28)
            n160 = control-ref of="Channel 1"() -> (w338:refnum<vi>)
            n161 = Replace Array Subset(array=w342, new element=w341, index=w335) -> (w340:T27)
            n162 = Replace Array Subset(array=w334, new element=w333, index=w335) -> (w332:T27)
            n163 = Replace Array Subset(array=w345, new element=w344, index=w335) -> (w343:T27)
            n164 = property on="Channel 3" class="WFGraph (strict)"("CrsrList"=w340) -> (error out=w339:errorcluster)  [unwired: 2 in, 1 out]
            n165 = property on="Channel 4" class="WFGraph (strict)"("CrsrList"=w332) -> ()  [unwired: 2 in, 2 out]
            n166 = property on="Channel 2" class="WFGraph (strict)"("CrsrList"=w343) -> ()  [unwired: 2 in, 2 out]
            n167 = call "UpdateCurserIdx(SubVI).vi"("error in (no error)"=w339, "WaveformGraph in"=w338) -> ()  [unwired: 9 in, 1 out]
          }
          event "Channel 2": Cursor Move {
            n168 = event-data() -> ("CursIdx"=w354:i32, "CursLoc"=w368:cluster{"X":dbl, "Y":dbl})  [unwired: 1 in, 7 out]
            n169 = Unbundle By Name(w368) -> ("X"=w356:dbl)
            n170 = property on="Channel 1" class="WFGraph (strict)"() -> ("CrsrList"=w362:T27)  [unwired: 2 in, 2 out]
            n171 = property on="Channel 3" class="WFGraph (strict)"() -> ("CrsrList"=w364:T27)  [unwired: 2 in, 2 out]
            n172 = property on="Channel 4" class="WFGraph (strict)"() -> ("CrsrList"=w355:T27)  [unwired: 2 in, 2 out]
            n173 = Index Array(array=w362, index=w354) -> (element=w367:T28)
            n174 = Index Array(array=w364, index=w354) -> (element=w366:T28)
            n175 = Index Array(array=w355, index=w354) -> (element=w357:T28)
            n176 = Bundle By Name(cluster=w357, "Position.X"=w356) -> (w353:T28)
            n177 = Bundle By Name(cluster=w367, "Position.X"=w356) -> (w365:T28)
            n178 = Bundle By Name(cluster=w366, "Position.X"=w356) -> (w363:T28)
            n179 = Replace Array Subset(array=w362, new element=w365, index=w354) -> (w361:T27)
            n180 = Replace Array Subset(array=w364, new element=w363, index=w354) -> (w360:T27)
            n181 = Replace Array Subset(array=w355, new element=w353, index=w354) -> (w352:T27)
            n182 = control-ref of="Channel 1"() -> (w359:refnum<vi>)
            n183 = property on="Channel 1" class="WFGraph (strict)"("CrsrList"=w361) -> ()  [unwired: 2 in, 2 out]
            n184 = property on="Channel 3" class="WFGraph (strict)"("CrsrList"=w360) -> (error out=w358:errorcluster)  [unwired: 2 in, 1 out]
            n185 = property on="Channel 4" class="WFGraph (strict)"("CrsrList"=w352) -> ()  [unwired: 2 in, 2 out]
            n186 = call "UpdateCurserIdx(SubVI).vi"("error in (no error)"=w358, "WaveformGraph in"=w359) -> ()  [unwired: 9 in, 1 out]
          }
          event "Channel 3": Cursor Move {
            n187 = event-data() -> ("CursIdx"=w374:i32, "CursLoc"=w388:cluster{"X":dbl, "Y":dbl})  [unwired: 1 in, 7 out]
            n188 = Unbundle By Name(w388) -> ("X"=w376:dbl)
            n189 = property on="Channel 4" class="WFGraph (strict)"() -> ("CrsrList"=w375:T27)  [unwired: 2 in, 2 out]
            n190 = property on="Channel 1" class="WFGraph (strict)"() -> ("CrsrList"=w385:T27)  [unwired: 2 in, 2 out]
            n191 = property on="Channel 2" class="WFGraph (strict)"() -> ("CrsrList"=w383:T27)  [unwired: 2 in, 2 out]
            n192 = Index Array(array=w375, index=w374) -> (element=w377:T28)
            n193 = Index Array(array=w385, index=w374) -> (element=w387:T28)
            n194 = Index Array(array=w383, index=w374) -> (element=w386:T28)
            n195 = Bundle By Name(cluster=w377, "Position.X"=w376) -> (w373:T28)
            n196 = Bundle By Name(cluster=w387, "Position.X"=w376) -> (w384:T28)
            n197 = Bundle By Name(cluster=w386, "Position.X"=w376) -> (w382:T28)
            n198 = Replace Array Subset(array=w375, new element=w373, index=w374) -> (w372:T27)
            n199 = Replace Array Subset(array=w385, new element=w384, index=w374) -> (w381:T27)
            n200 = Replace Array Subset(array=w383, new element=w382, index=w374) -> (w380:T27)
            n201 = control-ref of="Channel 1"() -> (w378:refnum<vi>)
            n202 = property on="Channel 4" class="WFGraph (strict)"("CrsrList"=w372) -> ()  [unwired: 2 in, 2 out]
            n203 = property on="Channel 1" class="WFGraph (strict)"("CrsrList"=w381) -> ()  [unwired: 2 in, 2 out]
            n204 = property on="Channel 2" class="WFGraph (strict)"("CrsrList"=w380) -> (error out=w379:errorcluster)  [unwired: 2 in, 1 out]
            n205 = call "UpdateCurserIdx(SubVI).vi"("error in (no error)"=w379, "WaveformGraph in"=w378) -> ()  [unwired: 9 in, 1 out]
          }
          event "Channel 4": Cursor Move {
            n206 = event-data() -> ("CursIdx"=w396:i32, "CursLoc"=w408:cluster{"X":dbl, "Y":dbl})  [unwired: 1 in, 7 out]
            n207 = Unbundle By Name(w408) -> ("X"=w394:dbl)
            n208 = property on="Channel 1" class="WFGraph (strict)"() -> ("CrsrList"=w406:T27)  [unwired: 2 in, 2 out]
            n209 = property on="Channel 2" class="WFGraph (strict)"() -> ("CrsrList"=w402:T27)  [unwired: 2 in, 2 out]
            n210 = property on="Channel 3" class="WFGraph (strict)"() -> ("CrsrList"=w397:T27)  [unwired: 2 in, 2 out]
            n211 = Index Array(array=w406, index=w396) -> (element=w407:T28)
            n212 = Index Array(array=w402, index=w396) -> (element=w403:T28)
            n213 = Index Array(array=w397, index=w396) -> (element=w399:T28)
            n214 = Bundle By Name(cluster=w407, "Position.X"=w394) -> (w405:T28)
            n215 = Bundle By Name(cluster=w403, "Position.X"=w394) -> (w401:T28)
            n216 = Bundle By Name(cluster=w399, "Position.X"=w394) -> (w398:T28)
            n217 = Replace Array Subset(array=w406, new element=w405, index=w396) -> (w404:T27)
            n218 = Replace Array Subset(array=w402, new element=w401, index=w396) -> (w400:T27)
            n219 = Replace Array Subset(array=w397, new element=w398, index=w396) -> (w395:T27)
            n220 = control-ref of="Channel 1"() -> (w392:refnum<vi>)
            n221 = call "UpdateCurserIdx(SubVI).vi"() -> ()  [unwired: 11 in, 1 out]
            n222 = call "UpdateCurserIdx(SubVI).vi"() -> ()  [unwired: 11 in, 1 out]
            n223 = property on="Channel 1" class="WFGraph (strict)"("CrsrList"=w404) -> ()  [unwired: 2 in, 2 out]
            n224 = property on="Channel 2" class="WFGraph (strict)"("CrsrList"=w400) -> ()  [unwired: 2 in, 2 out]
            n225 = property on="Channel 3" class="WFGraph (strict)"("CrsrList"=w395) -> (error out=w393:errorcluster)  [unwired: 2 in, 1 out]
            n226 = call "UpdateCurserIdx(SubVI).vi"("error in (no error)"=w393, "WaveformGraph in"=w392) -> ()  [unwired: 9 in, 1 out]
          }
          event "Cali&iRF alignment": Mouse Enter {
            n227 = event-data() -> ()  [unwired: 1 in, 4 out]
            n228 = local write "Help"("Click to run system intensity calibration and irf alignment" ("Help")) -> ()
          }
          event "Cali&iRF alignment": Value Change {
            n229 = event-data() -> ("NewVal"=w419:bool)  [unwired: 1 in, 5 out]
            n230 = case shown="False" w419 {
              tunnel: ["Utility: SetAllChanManualGain\nQueue: Flash\nUtility: Dewelling >> 2500\nLabJack: 355_PWM_Stop\nLabJack: AB_Stop" "Utility: SetDataClass >> Cali\nUI: Update\nUtility: SaveDeconChan\nLabJack: 355_PWM_Start\nLabJack: AB_Start\nLabJack: SetV\nDigitizer: Start\nUtility: AquiTimerReset\nLED: BreathGreen\nUI: duringIRFAlign"] -> w420
              tunnel: [FALSE TRUE] -> w416
              frame False {
                n231 = local read "Skip Data Save?"() -> (w424:bool)
                n232 = case shown="False" w424 {
                  frame False {
                    n233 = property on="Cali&iRF alignment" class="Bool (strict)"("BoolText.Text"="Done!" ("Boolean Text.Text")) -> ()  [unwired: 2 in, 2 out]
                  }
                  frame True {
                  }
                }
              }
              frame True {
                n234 = property on="Cali&iRF alignment" class="Bool (strict)"("BoolText.Text"="Running" ("Boolean Text.Text"), "Colors [4]"=cluster{u32, u32}[] [{6618880, 6618880}, {16711680, 16711680}]) -> ()  [unwired: 2 in, 2 out]
              }
            }
            n235 = Bundle By Name(cluster=w417, "SysRunning?"=w416) -> (w418:T26)
            n236 = call <vilib>:"Add State(s) to Queue__JKI_lib_State_Machine.vi"("State(s) in Front (\"\")"=w420, "State(s) in (\"\")"=w422) -> ("States Out"=w421:string)  [unwired: 13 in]
          }
          event "V 1": Value Change {
            n237 = event-data() -> ()  [unwired: 1 in, 6 out]
            n238 = call "LabJack_FGV.vi"("Operation(Read)"=enum16{"Write", "Read"}."Read" ("Operation"), "error in (no error)"=w439) -> ("error out"=w436:errorcluster, "Read data"=w437:i32)  [unwired: 8 in]
            n239 = global read "GlobalVariables.vi" "Ch1 LJ pin"() -> (w435:string)
            n240 = call "LJM_eWriteName.vi"("Handle In"=w437, "Name"=w435, "Value"="V 1", "error in"=w436) -> ("error out"=w433:errorcluster)  [unwired: 10 in, 1 out]
            n241 = call "V1FGV.vi"("Error In"=w433, "action (write)"=enum16{"write", "read"}."write" ("action"), "V1 in"="V 1") -> ("Error Out"=w432:errorcluster)  [unwired: 7 in, 1 out]
            n242 = call "CtrlVtoGain.vi"("error in (no error)"=w432, "CtrlV(V)"="V 1", "Channel"=enum16{"Ch1", "Ch2", "Ch3"}."Ch1" ("Enum")) -> ("error out"=w442:errorcluster, "Gain"=w441:dbl)  [unwired: 7 in]
            n243 = local write "Gain1"(w441) -> ()
          }
          event "V 2": Value Change {
            n244 = event-data() -> ()  [unwired: 1 in, 6 out]
            n245 = call "LabJack_FGV.vi"("Operation(Read)"=enum16{"Write", "Read"}."Read" ("Operation"), "error in (no error)"=w448) -> ("error out"=w453:errorcluster, "Read data"=w454:i32)  [unwired: 8 in]
            n246 = global read "GlobalVariables.vi" "Ch2 LJ pin"() -> (w452:string)
            n247 = call "LJM_eWriteName.vi"("Handle In"=w454, "Name"=w452, "Value"="V 2", "error in"=w453) -> ("error out"=w451:errorcluster)  [unwired: 10 in, 1 out]
            n248 = call "V2FGV.vi"("Error In"=w451, "action(write)"=enum16{"write", "read"}."write" ("action"), "V2 in"="V 2") -> ("Error Out"=w450:errorcluster)  [unwired: 7 in, 1 out]
            n249 = call "CtrlVtoGain.vi"("error in (no error)"=w450, "CtrlV(V)"="V 2", "Channel"=enum16{"Ch1", "Ch2", "Ch3"}."Ch2" ("Enum")) -> ("error out"=w446:errorcluster, "Gain"=w447:dbl)  [unwired: 7 in]
            n250 = local write "Gain2"(w447) -> ()
          }
          event "V 3": Value Change {
            n251 = event-data() -> ()  [unwired: 1 in, 6 out]
            n252 = call "LabJack_FGV.vi"("Operation(Read)"=enum16{"Write", "Read"}."Read" ("Operation"), "error in (no error)"=w460) -> ("error out"=w465:errorcluster, "Read data"=w466:i32)  [unwired: 8 in]
            n253 = global read "GlobalVariables.vi" "Ch3 LJ pin"() -> (w464:string)
            n254 = call "LJM_eWriteName.vi"("Handle In"=w466, "Name"=w464, "Value"="V 3", "error in"=w465) -> ("error out"=w462:errorcluster)  [unwired: 10 in, 1 out]
            n255 = call "V3FGV.vi"("Error In"=w462, "action(write)"=enum16{"write", "read"}."write" ("action"), "V3 in"="V 3") -> ("Error Out"=w461:errorcluster)  [unwired: 7 in, 1 out]
            n256 = call "CtrlVtoGain.vi"("error in (no error)"=w461, "CtrlV(V)"="V 3", "Channel"=enum16{"Ch1", "Ch2", "Ch3"}."Ch3" ("Enum")) -> ("error out"=w469:errorcluster, "Gain"=w468:dbl)  [unwired: 7 in]
            n257 = local write "Gain3"(w468) -> ()
          }
          event "V 4": Value Change {
            n258 = event-data() -> ()  [unwired: 1 in, 6 out]
            n259 = call "LabJack_FGV.vi"("Operation(Read)"=enum16{"Write", "Read"}."Read" ("Operation"), "error in (no error)"=w476) -> ("error out"=w480:errorcluster, "Read data"=w481:i32)  [unwired: 8 in]
            n260 = global read "GlobalVariables.vi" "Ch4 LJ pin"() -> (w479:string)
            n261 = call "LJM_eWriteName.vi"("Handle In"=w481, "Name"=w479, "Value"="V 4", "error in"=w480) -> ("error out"=w478:errorcluster)  [unwired: 10 in, 1 out]
            n262 = call "V4FGV.vi"("Error In"=w478, "action(write)"=enum16{"write", "read"}."write" ("action"), "V3 in"="V 4") -> ("Error Out"=w477:errorcluster)  [unwired: 7 in, 1 out]
            n263 = call "CtrlVtoGain.vi"("error in (no error)"=w477, "CtrlV(V)"="V 4", "Channel"=enum16{"Ch1", "Ch2", "Ch3", "Ch4"}."Ch4") -> ("error out"=w484:errorcluster, "Gain"=w483:dbl)  [unwired: 7 in]
            n264 = local write "Gain4"(w483) -> ()
          }
          event "Quit": Value Change {
            # "Exit Button Value Change (pressed) Event\n(when pressed.  quite)"
            n265 = event-data() -> ()  [unwired: 1 in, 1 out]
            n266 = call <vilib>:"Add State(s) to Queue__JKI_lib_State_Machine.vi"("State(s) in Front (\"\")"="LED: Off\nMacro: Exit", "State(s) in (\"\")"=w492) -> ("States Out"=w491:string)  [unwired: 13 in]
          }
          event "Show BG": Value Change {
            n267 = event-data() -> ()  [unwired: 1 in, 6 out]
            n268 = call <vilib>:"Add State(s) to Queue__JKI_lib_State_Machine.vi"("State(s) in Front (\"\")"="Data: showBG" ("State(s) in Front (\"\")"), "State(s) in (\"\")"=w495) -> ("States Out"=w494:string)  [unwired: 13 in]
          }
          event "StartButton": Mouse Enter {
            n269 = event-data() -> ()  [unwired: 1 in, 4 out]
            n270 = local write "Help"("Press to start aquisition." ("Help")) -> ()
          }
          event "StartButton": Value Change {
            # "[Covers: REQ32]"
            # "start PWM before acquisition"
            # "Initialize both digitizer aquisition and\n send user event to trigger aquisition loop"
            n271 = event-data() -> ()  [unwired: 1 in, 6 out]
            n272 = local write "StartButton"(FALSE ("StartButton")) -> ()
            n273 = Bundle By Name(cluster=w504, "SysRunning?"=TRUE) -> (w506:T26)
            n274 = call <vilib>:"Add State(s) to Queue__JKI_lib_State_Machine.vi"("State(s) in Front (\"\")"="TCP: stopCam\nUtility: SetDataClass >> Data\nQueue: Flash\nUI: Update\nUtility: StartBeep\nLabJack: 355_PWM_Start\nLabJack: AB_Start\nLabJack: SetV\nDigitizer: Start\nUtility: AquiTimerReset\nUI: DuringAquisition\nLED: BreathGreen\nTCP: sendRunNum\nTCP: sendVideoSource\nTCP: sendChannel\nTCP: startRun", "State(s) in (\"\")"=w508) -> ("States Out"=w509:string)  [unwired: 13 in]
          }
          event User Event {
            # "[Covers: REQ32]"
            # "start PWM before acquisition"
            # "Initialize both digitizer aquisition and\n send user event to trigger aquisition loop"
            n275 = event-data() -> ()  [unwired: 1 in, 5 out]
            n276 = Bundle By Name(cluster=w511, "SysRunning?"=TRUE) -> (w513:T26)
            n277 = call <vilib>:"Add State(s) to Queue__JKI_lib_State_Machine.vi"("State(s) in Front (\"\")"="TCP: stopCam\nUtility: SetDataClass >> Data\nQueue: Flash\nUI: Update\nUtility: StartBeep\nLabJack: 355_PWM_Start\nLabJack: AB_Start\nLabJack: SetV\nDigitizer: Start\nUtility: AquiTimerReset\nUI: DuringAquisition\nLED: BreathGreen\nTCP: sendRunNum\nTCP: sendVideoSource\nTCP: sendChannel\nTCP: startRun", "State(s) in (\"\")"=w515) -> ("States Out"=w516:string)  [unwired: 13 in]
          }
          event "Video Display": Value Change {
            n278 = event-data() -> ("NewVal"=w522:bool)  [unwired: 1 in, 5 out]
            n279 = Select(t="TCP: startCam", s=w522, f="TCP: stopCam") -> (s? t:f=w519:string)
            n280 = call <vilib>:"Add State(s) to Queue__JKI_lib_State_Machine.vi"("State(s) in (\"\")"=w521, "State(s) at Back (\"\")"=w519) -> ("States Out"=w520:string)  [unwired: 13 in]
          }
          event "Video Source": Value Change {
            n281 = event-data() -> ()  [unwired: 1 in, 6 out]
            n282 = call <vilib>:"Add State(s) to Queue__JKI_lib_State_Machine.vi"("State(s) in Front (\"\")"="TCP: sendVideoSource" ("State(s) in Front (\"\")"), "State(s) in (\"\")"=w527) -> ("States Out"=w526:string)  [unwired: 13 in]
          }
          event "StopButton": Mouse Enter {
            n283 = event-data() -> ()  [unwired: 1 in, 4 out]
            n284 = local write "Help"("Press to stop data aquisition." ("Help")) -> ()
          }
          event "StopButton": Value Change {
            # "if system is running, send stop command, if not do nothing."
            # "stop aquisition\nupdate UI"
            n285 = event-data() -> ()  [unwired: 1 in, 6 out]
            n286 = Unbundle By Name(w535) -> ("SysRunning?"=w537:bool)
            n287 = case shown="True" w537 {
              tunnel: ["" ("Empty String Constant") "LabJack: AB_Stop\nLabJack: 355_PWM_Stop\n/*Digitizer: Abort"] -> w538
              tunnel: w535 -> [w542 w546]
              tunnel: [w542 w545] -> w536
              frame False {
              }
              frame True {
                n288 = Bundle By Name(cluster=w546, "SysRunning?"=FALSE) -> (w545:T26)
              }
            }
            n289 = call <vilib>:"Add State(s) to Queue__JKI_lib_State_Machine.vi"("State(s) in Front (\"\")"=w538, "State(s) in (\"\")"=w540) -> ("States Out"=w541:string)  [unwired: 13 in]
            n290 = local write "StopButton"(FALSE ("StopButton")) -> ()
          }
          event User Event {
            # "if system is running, send stop command, if not do nothing."
            # "stop aquisition\nupdate UI"
            n291 = event-data() -> ()  [unwired: 1 in, 5 out]
            n292 = Unbundle By Name(w548) -> ("SysRunning?"=w550:bool)
            n293 = case shown="True" w550 {
              tunnel: ["" ("Empty String Constant") "LabJack: AB_Stop\nLabJack: 355_PWM_Stop\n/*Digitizer: Abort"] -> w551
              tunnel: w548 -> [w555 w559]
              tunnel: [w555 w558] -> w549
              frame False {
              }
              frame True {
                n294 = Bundle By Name(cluster=w559, "SysRunning?"=FALSE) -> (w558:T26)
              }
            }
            n295 = call <vilib>:"Add State(s) to Queue__JKI_lib_State_Machine.vi"("State(s) in Front (\"\")"=w551, "State(s) in (\"\")"=w553) -> ("States Out"=w554:string)  [unwired: 13 in]
          }
          event "Sys Reconfig": Mouse Enter {
            n296 = event-data() -> ()  [unwired: 1 in, 4 out]
            n297 = local write "Help"("Click to reconfig digitizer settings." ("Help")) -> ()
          }
          event "Sys Reconfig": Value Change {
            # "everytime the user change data aquisition setting, need to reinitilize decon engine and realign iRF.\ncheck whether data length has changed, if changed, reinitialize Decon engine\nreset BG ready, need a new BG"
            # "update DAQ FGV"
            n298 = event-data() -> ()  [unwired: 1 in, 6 out]
            n299 = call "SystemConfigEditorV6.vi"("error in"=w575) -> ("error out"=w574:errorcluster, "FLImDAQ out"=w569:T6)  [unwired: 1 in]
            n300 = Unbundle By Name(w572) -> ("FLImDAQ.min record length"=w571:i32)
            n301 = Unbundle By Name(w569) -> ("min record length"=w570:i32)
            n302 = call "FLImDAQ_FGV.vi"("error in (no error)"=w574, "Operation (Read)"=enum16{"Write", "Read"}."Write" ("Operation"), "Write data"=w569) -> ("error out"=w573:errorcluster, "Read data"=w568:T6)  [unwired: 7 in]
            n303 = Equal?(x=w571, y=w570) -> (x = y?=w567:bool)
            n304 = case shown="False" w567 {
              tunnel: ["UI: Cursor Set >> Busy\nDigitizer: Config\nDeconEngine: InitializeCh1\nDeconEngine: InitializeCh2\nDeconEngine: InitializeCh3\nUI: CaliAndiRFNotReady\n/*UI iRF not ready\nUI: Update\nUI: Cursor Set >> Idle" "UI: Cursor Set >> Busy\nDigitizer: Config\nUI: Update\nUI: Cursor Set >> Idle"] -> w566
              frame False {
              }
              frame True {
              }
            }
            n305 = Bundle By Name(cluster=w572, "FLImDAQ"=w568) -> (w578:T26)
            n306 = call <vilib>:"Add State(s) to Queue__JKI_lib_State_Machine.vi"("State(s) in Front (\"\")"=w566, "State(s) in (\"\")"=w576) -> ("States Out"=w577:string)  [unwired: 13 in]
          }
          event "System Hardware Connection Status", "StartButton", "StopButton", "355nm Laser toggle", "Aiming beam toggle", "Cali&iRF alignment", "Background", "Sys Reconfig": Mouse Leave {
            n307 = event-data() -> ()  [unwired: 1 in, 4 out]
            n308 = invoke on="Help" class="Str" method="Reinit To Default"() -> ()  [unwired: 3 in, 3 out]
          }
          event "System Hardware Connection Status.Digitizer": Mouse Enter {
            n309 = event-data() -> ()  [unwired: 1 in, 4 out]
            n310 = local write "Help"("Status of hardware connections. TCP/IP is optional." ("Help")) -> ()
          }
          event "TCP Connect": Value Change {
            n311 = event-data() -> ("NewVal"=w588:bool)  [unwired: 1 in, 5 out]
            n312 = case shown="True" w588 {
              tunnel: ["TCP: Close\nUI: Update" ("State(s) in Front (\"\")") "TCP: SendSettingMacro\nUI: Update" ("State(s) in Front (\"\")")] -> w589
              frame False {
              }
              frame True {
              }
            }
            n313 = call <vilib>:"Add State(s) to Queue__JKI_lib_State_Machine.vi"("State(s) in Front (\"\")"=w589, "State(s) in (\"\")"=w591) -> ("States Out"=w590:string)  [unwired: 13 in]
          }
          event User Event {
            # "if aquisition loop is error out. Stop digitizer, update front panel indicator, stop both laser and \nOption 1: parse and save data\nOption 2: Flash queue if scout run. [Covers: REQ23]"
            n314 = event-data() -> ()  [unwired: 1 in, 5 out]
            n315 = case shown="\"Cali\"" "Data Class" {
              tunnel: [w613 "UI: Cursor Set >> Busy\nUtility: SetAllChanAutoGain\nUtility: RestoreDeConChan\nData: parseRunData\nData: irfAlignment\nUI: Cursor Set >> Idle" "UI: Cursor Set >> Busy\nUtility: SetAllChanAutoGain\nUtility: RestoreDeConChan\nData: parseRunData\nData: saveBGtoFGV\nData: saveBGtoFile\nUI: Cursor Set >> Idle\nData: showBG\nRun: BGIncrement"] -> w603
              frame "Data", Default {
                n316 = local read "Video Display"() -> (w615:bool)
                n317 = Select(t="TCP: startCam", s=w615, f="") -> (s? t:f=w611:string)
                n318 = call <vilib>:"Add State(s) to Queue__JKI_lib_State_Machine.vi"("State(s) in Front (\"\")"="UI: Cursor Set >> Busy\nData: parseRunData\nData: saveRunData\nUI: Cursor Set>>Idle" ("State(s) in Front (\"\")"), "State(s) in (\"\")"=w611) -> ("States Out"=w613:string)  [unwired: 13 in]
              }
              frame "Cali" {
              }
              frame "BG" {
              }
            }
            n319 = Bundle By Name(cluster=w605, "SysRunning?"=FALSE) -> (w606:T26)
            n320 = Select(t="" ("State(s) in Front (\"\")"), s="Skip Data Save?", f=w603) -> (s? t:f=w600:string)
            n321 = call <vilib>:"Add State(s) to Queue__JKI_lib_State_Machine.vi"("State(s) in Front (\"\")"="TCP: stopRun\nUI: Update\nLabJack: AB_Stop\nLabJack: 355_PWM_Stop\nDigitizer: Abort\nLabJack: ZeroV\nUtility: EndBeep\nLED: BreathOff" ("State(s) in Front (\"\")"), "State(s) in (\"\")"=w600, "State(s) at Back (\"\")"="Macro: SysReadyForAq\nUI: Update" ("State(s) in Front (\"\")")) -> ("States Out"=w598:string)  [unwired: 12 in]
            n322 = call <vilib>:"Add State(s) to Queue__JKI_lib_State_Machine.vi"("State(s) in Front (\"\")"=w598, "State(s) in (\"\")"=w607) -> ("States Out"=w608:string)  [unwired: 13 in]
          }
          event Panel Close? {
            # "Discard the event because we'll close the front panel ourselves in Macro: Exit"
            # "Close Panel button (pressed) Event\n(this executes Macro: Exit to terminate the VI)"
            n323 = event-data() -> ()  [unwired: 1 in, 1 out]
            n324 = event-data ("Event Filter Node")("Discard?"=TRUE) -> ()  [unwired: 1 in, 1 out]
            n325 = call <vilib>:"Add State(s) to Queue__JKI_lib_State_Machine.vi"("State(s) in Front (\"\")"="Macro: Exit", "State(s) in (\"\")"=w623) -> ("States Out"=w622:string)  [unwired: 13 in]
          }
        }
      }
      frame "---------- Macro ----------" {
        # "Do not put any code in this frame.\n(It is a separator no-op. You can make a copy of this frame to create a new Macro frame)"
        n326 = call <vilib>:"Add State(s) to Queue__JKI_lib_State_Machine.vi"("State(s) in (\"\")"=w628) -> ("States Out"=w627:string)  [unwired: 14 in]
      }
      frame "Macro: Initialize" {
        # "load Labjack setting 1st as it contaisn laser pin infortmation"
        # "start laser 1st, need 7.5s for laser to get ready"
        # "Initialization Macro\n(This is called once, when the VI starts)"
        n327 = call <vilib>:"Add State(s) to Queue__JKI_lib_State_Machine.vi"("State(s) in Front (\"\")"="UI: showDisclaimer\nUI: Cursor Set >> Busy\nData: Initialize\nInitialize Core Data\nUI: Initialize\nUI: Front Panel State >> Open\nMacro: LoadSysConfig\nTCP: InitializeNew\nTCP: checkSource\nUI: Update\nLabJack: Open\nLabJack: SetDefaultSub\nLED: OpenVIRef\nLED: BreathOrange\nUI: Update\n355 Laser: CheckControllerStatus\n355 Laser: Laser enable\n355 Laser: Dewelling>>500\n355 Laser: CheckControllerStatus\nUI: Update\nLabJack: 355_PWM_Config\nLabJack: AB_PWM_Config\nUI: Update", "State(s) in (\"\")"="Digitizer: Initialize\nDigitizer: Config\nUI: Update\nAimingBeam: Initialize\nAimingBeam: Set Status>>Enable\nAimingBeam: Set Current\nUI: Update\n355 Laser: Check Dewelling\nUI: Cursor Set >> Idle\nCase: GetID\nUI: Update\nTCP: SendSettingMacro\nCase: CreatFileStruct\nUI: Update\nData: loadLastUseMacro\nDeconEngine: InitilizeMacro\nGraph: SetXMultiplier\nGraph: AddCursors\nAPD: Initialize\nAPD: LoadFromSerial\nAPD: UpdateCtrlVLimit\nAPD: GetGainLimits\nPID: loadPID\nLED: BreathOff\nMacro: SysReadyForAq") -> ("States Out"=w629:string)  [unwired: 13 in]
        n328 = call <vilib>:"Add State(s) to Queue__JKI_lib_State_Machine.vi"("State(s) in Front (\"\")"=w629, "State(s) in (\"\")"=w637) -> ("States Out"=w636:string)  [unwired: 13 in]
        "Help" <- "Hover over controls to see help!" ("Help")
      }
      frame "Macro: LoadSysConfig" {
        # "System configuration Macro. [Covers: REQ15]\n(Load configurations for different component of the system)"
        n329 = call <vilib>:"Add State(s) to Queue__JKI_lib_State_Machine.vi"("State(s) in Front (\"\")"="SysConfig: Load Sys Config\nSysConfig: Load Digitizer Setting\nSysConfig: Load AB setting\nSysConfig: Load LJ Pinout\nSysConfig: Load 355 PWM\nSysConfig: LoadAPDSerialNumber\nSysConfig: LoadABVideoSetting\nSysConfig: LoadCursorLocation", "State(s) in (\"\")"=w643) -> ("States Out"=w642:string)  [unwired: 13 in]
      }
      frame "Macro: SysReadyForAq" {
        # "Macro for system ready\n(It is a separator no-op. You can make a copy of this frame to create a new Macro frame)"
        n330 = call <vilib>:"Add State(s) to Queue__JKI_lib_State_Machine.vi"("State(s) in Front (\"\")"="UI: ReadyForAquisition\nLED: Green" ("State(s) in Front (\"\")"), "State(s) in (\"\")"=w649) -> ("States Out"=w648:string)  [unwired: 13 in]
      }
      frame "Macro: Exit" {
        # "close LJ last"
        # "check whether hardware is initilized, if so close, if not do nothing"
        # "Exit Macro, close all hardware\n(This is called once, when the VI exits)"
        n331 = Unbundle By Name(w668) -> ("System Status.Digitizer"=w664:bool, "System Status.Aiming Beam"=w663:bool, "System Status.355 Laser"=w662:bool, "System Status.Labjack"=w653:bool, "Core.Close Panel on Exit?"=w657:bool)
        n332 = case shown="True" w664 {
          tunnel: ["" ("Empty String Constant") "Digitizer: Close"] -> w659
          frame False {
          }
          frame True {
          }
        }
        n333 = case shown="True" w653 {
          tunnel: ["" ("Empty String Constant") "LabJack: SetDefaultAndClose"] -> w650
          frame False {
          }
          frame True {
          }
        }
        n334 = case shown="True" w663 {
          tunnel: ["" ("Empty String Constant") w675] -> w652
          frame False {
          }
          frame True {
            w675 = "AimingBeam: Set Status >> Disable\nAimingBeam: Close"  # AimingBeam: Set Status >> Disable AimingBeam: Close
          }
        }
        n335 = case shown="True" w662 {
          tunnel: ["" ("Empty String Constant") "355 Laser: Close\n355 Laser: CheckControllerStatus"] -> w651
          frame False {
          }
          frame True {
          }
        }
        n336 = Select(t="UI: Front Panel State >> Close", s=w657, f="" ("Empty String Constant")) -> (s? t:f=w654:string)
        n337 = call <vilib>:"Add State(s) to Queue__JKI_lib_State_Machine.vi"("State(s) in Front (\"\")"="TCP: Close", "State(s) in (\"\")"=w659, "State(s) at Back (\"\")"=w652) -> ("States Out"=w661:string)  [unwired: 12 in]
        n338 = call <vilib>:"Add State(s) to Queue__JKI_lib_State_Machine.vi"("State(s) in Front (\"\")"=w661, "State(s) in (\"\")"=w651, "State(s) at Back (\"\")"=w650) -> ("States Out"=w656:string)  [unwired: 12 in]
        n339 = call <vilib>:"Add State(s) to Queue__JKI_lib_State_Machine.vi"("State(s) in Front (\"\")"=w656, "State(s) in (\"\")"="UI: Update\nUI: Reset\nGraph: SaveCursorLoc\nLED: CloseVIRef\nQueue: Destory\nData: Cleanup\nExit", "State(s) at Back (\"\")"=w654) -> ("States Out"=w665:string)  [unwired: 12 in]
        n340 = call <vilib>:"Add State(s) to Queue__JKI_lib_State_Machine.vi"("State(s) in Front (\"\")"=w665, "State(s) in (\"\")"=w671) -> ("States Out"=w670:string)  [unwired: 13 in]
      }
      frame "---------- Data ----------" {
        # "Do not put any code in this frame.\n(It is a separator no-op. You can make a copy of this frame to create a new Data frame)"
        n341 = call <vilib>:"Add State(s) to Queue__JKI_lib_State_Machine.vi"("State(s) in (\"\")"=w684) -> ("States Out"=w683:string)  [unwired: 14 in]
      }
      frame "Data: Initialize" {
        w685 = path ""  # CaliPath
        w686 = dbl[] []  # V4
        w687 = dbl[][] []  # Ch4Data
        w688 = FALSE  # bothVidSourceAvail
        w689 = T1 {"Main Frame Grabber"=FALSE, "Side Frame Grabber"=FALSE, "Main Camera"=FALSE, "Side Camera"=FALSE}  # video source
        w690 = FALSE  # LED vi ref open?
        w692 = T25 {"DeCon Channel"=enum."1", "Scale Bar"=FALSE, "Scale Low"=3.0, "Scale High"=8.0, "ANSI"=20.0, "Radius"=1.0, "3D?"=FALSE, "Firefly?"=FALSE, "Pentero?"=FALSE}  # VideoConfig
        w693 = T29 {"Ch1APDSerial#"="", "Ch2APDSerial#"="", "Ch3APDSerial#"="", "Ch4APDSerial#"=""}  # APDSerialNum
        w694 = u32 0  # Aquisition Timer
        w695 = cluster{"RunID":i8, "BG ID":i8, "Cali ID":i8} {"RunID"=1, "BG ID"=1, "Cali ID"=1}  # IDs
        w696 = refnum<vi> refnum  # LED vi reference
        w697 = path ""  # TempPath
        w698 = T30 {"DataPath"=path "", "BG Path"=path "", "iRFPath"=path "", "CaliPath"=path ""}  # Pathes
        w700 = dbl[] []  # V3
        w701 = dbl[] []  # V2
        w702 = dbl[] []  # V1
        w704 = u32 0  # FastTimer
        w705 = u32 0  # SlowTimer
        w706 = dbl[][] []  # Ch3Data
        w707 = dbl[][] []  # Ch2Data
        w691 = dbl[][] []  # Ch1Data
        w710 = T2 {"Digitizer"=FALSE, "Labjack"=FALSE, "Aiming Beam"=FALSE, "355 Laser"=FALSE, "TCP/IP"=FALSE}  # System Status
        w711 = T31 {"DIO_EF_CLOCK1_DIVISOR"=16, "DIO_EF_CLOCK1_ROLL_VALUE"=25000, "DIO#_EF_INDEX"=0, "DIO#_EF_OPTIONS"=1, "DIO#_EF_CONFIG_A"=6250}  # AB PWM setting
        w712 = T5 {"Ch1 Bias"="TDA11", "Ch2 Bias"="DAC10", "Ch3 Bias"="DAC0", "Ch4 Bias"="DAC0", "355 PWM"="FIO0", "AimingBeam PWM"="FIO2", "Laser Ready"="FIO3", "Interlock"="FIO1", "Laser Start/Stop"="FIO1", "Red LED"="FIO1", "Green LED"="FIO1", "Foot Pedal"="DIO15"}  # LJ Pinout
        w713 = 0  # TCP attempt count
        w714 = u32 0  # Laser start tic
        w715 = refnum<k20>[] []  # niTClk sessions
        w716 = u32 0  # Last Trigger
        w717 = T31 {"DIO_EF_CLOCK1_DIVISOR"=16, "DIO_EF_CLOCK1_ROLL_VALUE"=25000, "DIO#_EF_INDEX"=0, "DIO#_EF_OPTIONS"=1, "DIO#_EF_CONFIG_A"=6250}  # 355 PWM setting
        w718 = T32 {"Aiming Beam COM Port"="COM3", "Min Current"=0.0, "Max Current"=63.0, "Default Current"=20.0, "Freq"=0}  # AB Cluster
        w719 = T33 {"resource name"="", "resource name 2"="", "Channel"=enum."Channel 0", "trigger source"="VAL_EXTERNAL", "trigger level"=0.5, "trigger delay"=1.35e-07, "min sample rate"=12500000000.0, "min record length"=2500, "vertical range"=1.0, "vertical offset"=-0.25, "Waveform to Avg"=2000}  # FLImDAQ
        w720 = FALSE  # SysRunning?
        w708 = path ""  # DefaultPath
        w721 = ""  # CaseID
        w722 = T4 {"Ch1Enable?"=FALSE, "Ch2Enable?"=FALSE, "Ch3Enable?"=FALSE, "Ch1AutoGain?"=FALSE, "Ch2AutoGain?"=FALSE, "Ch3AutoGain?"=FALSE, "AimingBeamEnable?"=FALSE}  # SysConfigCluster
        w723 = T34 {"Current VI Reference"=refnum, "Close Panel on Exit?"=FALSE}  # Core
        # "Initialize the shift-register data, here.\n(data names are defined by what you wire into the bundle function)"
        n342 = Bundle("Core"=w723, "SysConfigCluster"=w722, "System Status"=w710, "IDs"=w695, "CaseID"=w721, "DefaultPath"=w708, "Pathes"=w698, "FLImDAQ"=w719, "SysRunning?"=w720, "AB Cluster"=w718, "LJ Pinout"=w712, "355 PWM setting"=w717, "AB PWM setting"=w711, "Last Trigger"=w716, "niTClk sessions"=w715, "Laser start tic"=w714, "TCP attempt count"=w713, "Ch1Data"=w691, "Ch2Data"=w707, "Ch3Data"=w706, "Ch4Data"=w687, "V1"=w702, "V2"=w701, "V3"=w700, "V4"=w686, "SlowTimer"=w705, "FastTimer"=w704, "listener ID"=refnum<k5> refnum, "TempPath"=w697, "CaliPath"=w685, "LED vi reference"=w696, "Aquisition Timer"=w694, "APDSerialNum"=w693, "VideoConfig"=w692, "LED vi ref open?"=w690, "video source"=w689, "bothVidSourceAvail"=w688) -> (w699:T26)  [unwired: 1 in]
        n343 = call <vilib>:"Add State(s) to Queue__JKI_lib_State_Machine.vi"("State(s) in (\"\")"=w726) -> ("States Out"=w725:string)  [unwired: 14 in]
      }
      frame "Data: loadLastUseMacro" {
        # "Load last use BG and Cali and iRF.\n(It is a separator no-op. You can make a copy of this frame to create a new Data frame)"
        n344 = call <vilib>:"Add State(s) to Queue__JKI_lib_State_Machine.vi"("State(s) in Front (\"\")"="Data: loadLastUseBG\nData: loadSystemCali\n/*Data: loadLastUseiRF\nData: LoadiRFFromAPDFile\nUI: CaliAndiRFLoaded\nData: ShowiRF" ("State(s) in Front (\"\")"), "State(s) in (\"\")"=w732) -> ("States Out"=w731:string)  [unwired: 13 in]
      }
      frame "Data: loadLastUseBG" {
        w736 = enum16{"write", "read"}."write" ("action")
        # "Load last use BG.\n()"
        n345 = Unbundle By Name(w755) -> ("TempPath"=w754:path)
        n346 = call "FLImDAQ_FGV.vi"() -> ("Read data"=w750:T6)  [unwired: 10 in, 1 out]
        n347 = Build Path(base path=w754, name or relative path="Background.tdms") -> (appended path=w753:path)
        n348 = call "ReadBGorCali (SubVI).vi"("DataType"=enum16{"BG", "Cali"}."BG", "error in (no error)"=w752, "file path in"=w753) -> ("error out"=w751:errorcluster, "AvgDataCluster"=w746:T35)  [unwired: 6 in, 1 out]
        n349 = Unbundle By Name(w746) -> ("Channel 1"=w733:dbl[], "Channel 2"=w745:dbl[], "Channel 3"=w738:dbl[], "Channel 4"=w735:dbl[])
        n350 = Unbundle By Name(w750) -> ("min record length"=w742:i32)
        n351 = Array Size(array=w733) -> (size(s)=w744:i32)
        "BG length" <- w744
        n352 = Equal?(x=w744, y=w742) -> (x = y?=w743:bool)
        n353 = Select(t="UI: BGLoaded" ("State(s) in Front (\"\")"), s=w743, f="UI: BGSizeError" ("State(s) in Front (\"\")")) -> (s? t:f=w747:string)
        n354 = case shown="True" w743 {
          tunnel: w733 -> [_ w766]
          tunnel: w745 -> [_ w765]
          tunnel: w738 -> [_ w764]
          tunnel: w742 -> [w761 _]
          tunnel: [w760 w766] -> w741
          tunnel: [w760 w765] -> w740
          tunnel: [w760 w764] -> w739
          tunnel: w735 -> [_ w763]
          tunnel: [w760 w763] -> w734
          frame False {
            # "If error set BG all 0, update UI"
            n355 = for {
              N: w761 -> [_]
              tunnel: [0.0] -> w760 mode=indexing
            }
          }
          frame True {
            # "If no error, check size match"
          }
        }
        n356 = call "BG4FGV.vi"("action"=w736, "BG4 in"=w734) -> ()  [unwired: 8 in, 2 out]
        n357 = call "BG3FGV.vi"("action"=w736, "BG3 in"=w739) -> ()  [unwired: 8 in, 2 out]
        n358 = call "BG1FGV.vi"("action"=w736, "BG1 in"=w741) -> ()  [unwired: 8 in, 2 out]
        n359 = call "BG2FGV.vi"("action"=w736, "BG2 in"=w740) -> ()  [unwired: 8 in, 2 out]
        n360 = call <vilib>:"Add State(s) to Queue__JKI_lib_State_Machine.vi"("State(s) in Front (\"\")"=w747, "State(s) in (\"\")"=w759) -> ("States Out"=w758:string)  [unwired: 13 in]
      }
      frame "Data: loadSystemCali" {
        # "Load last use calibration.\n()"
        n361 = Unbundle By Name(w774) -> ("CaliPath"=w773:path)
        n362 = Build Path(base path=w773, name or relative path="Calibration.tdms") -> (appended path=w769:path)
        n363 = call "ReadBGorCali (SubVI).vi"("DataType"=enum16{"BG", "Cali"}."Cali", "error in (no error)"=w768, "file path in"=w769) -> ("error out"=w770:errorcluster, "CtrlVCluster"=w772:T36, "AvgDataCluster"=w771:T35)  [unwired: 6 in]
        n364 = case shown="No Error" w770 {
          tunnel: w772 -> [w793 _]
          tunnel: w771 -> [w792 _]
          frame No Error {
            w783 = T37 {"Ch1 WF"=[], "Ch2 WF"=[], "Ch3 WF"=[], "Ch4 WF"=[], "V1"=0.0, "V2"=0.0, "V3"=0.0, "V4"=0.0}  # SysCaliData
            n365 = Unbundle By Name(w792) -> ("Channel 1"=w791:dbl[], "Channel 2"=w790:dbl[], "Channel 3"=w789:dbl[], "Channel 4"=w782:dbl[])
            n366 = Unbundle By Name(w793) -> ("V 1"=w788:dbl[], "V 2"=w787:dbl[], "V 3"=w781:dbl[], "V 4"=w779:dbl[])
            n367 = Index Array(array=w788) -> (element=w786:dbl)  [unwired: 1 in]
            n368 = Index Array(array=w787) -> (element=w785:dbl)  [unwired: 1 in]
            n369 = Index Array(array=w781) -> (element=w784:dbl)  [unwired: 1 in]
            n370 = Index Array(array=w779) -> (element=w780:dbl)  [unwired: 1 in]
            n371 = Bundle By Name(cluster=w783, "Ch1 WF"=w791, "Ch2 WF"=w790, "Ch3 WF"=w789, "Ch4 WF"=w782, "V1"=w786, "V2"=w785, "V3"=w784, "V4"=w780) -> (w794:T37)
            n372 = global write "GlobalVariables.vi" "SysCaliData"(w794) -> ()
          }
          frame Error {
          }
        }
        n373 = call <vilib>:"Add State(s) to Queue__JKI_lib_State_Machine.vi"("State(s) in (\"\")"=w778) -> ("States Out"=w777:string)  [unwired: 14 in]
      }
      frame "Data: LoadiRFFromAPDFile" {
        w824 = T19 {"Ch1 iRF"=[], "Ch2 iRF"=[], "Ch3 iRF"=[], "Ch4 iRF"=[]}  # LastUseiRF
        # "only load the last 5th  iRF for the moment"
        # "Load APD detector data\n(It is a separator no-op. You can make a copy of this frame to create a new Data frame)"
        n374 = Unbundle By Name(w846) -> ("APDSerialNum.Ch1APDSerial#"=w845:string, "APDSerialNum.Ch2APDSerial#"=w826:string, "APDSerialNum.Ch3APDSerial#"=w825:string, "APDSerialNum.Ch4APDSerial#"=w822:string)
        n375 = call "CreatFromSerialNumNoRaw.vi"("error in (no error)"=w823, "APD Serial #"=w845) -> ("error out"=w843:errorcluster, "APDClass out"=w844:refnum<class "APDClass.lvclass">)  [unwired: 8 in]
        n376 = call "CreatFromSerialNumNoRaw.vi"("error in (no error)"=w823, "APD Serial #"=w826) -> ("error out"=w834:errorcluster, "APDClass out"=w835:refnum<class "APDClass.lvclass">)  [unwired: 8 in]
        n377 = call "CreatFromSerialNumNoRaw.vi"("error in (no error)"=w823, "APD Serial #"=w825) -> ("error out"=w828:errorcluster, "APDClass out"=w829:refnum<class "APDClass.lvclass">)  [unwired: 8 in]
        n378 = call "CreatFromSerialNumNoRaw.vi"("error in (no error)"=w823, "APD Serial #"=w822) -> ("error out"=w820:errorcluster, "APDClass out"=w821:refnum<class "APDClass.lvclass">)  [unwired: 8 in]
        n379 = call-dynamic "Read iRFData.vi"("error in (no error)"=w843, "APDClass in"=w844) -> ("iRFData"=w842:T38)  [unwired: 7 in, 2 out]
        n380 = call-dynamic "Read iRFData.vi"("error in (no error)"=w834, "APDClass in"=w835) -> ("iRFData"=w838:T38)  [unwired: 7 in, 2 out]
        n381 = call-dynamic "Read iRFData.vi"("error in (no error)"=w828, "APDClass in"=w829) -> ("iRFData"=w832:T38)  [unwired: 7 in, 2 out]
        n382 = call-dynamic "Read iRFData.vi"("error in (no error)"=w820, "APDClass in"=w821) -> ("iRFData"=w819:T38)  [unwired: 7 in, 2 out]
        n383 = Unbundle By Name(w842) -> ("iRFWFsAvg"=w841:dbl[][])
        n384 = Unbundle By Name(w838) -> ("iRFWFsAvg"=w837:dbl[][])
        n385 = Unbundle By Name(w832) -> ("iRFWFsAvg"=w831:dbl[][])
        n386 = Unbundle By Name(w819) -> ("iRFWFsAvg"=w816:dbl[][])
        n387 = Array Size(array=w841) -> (size(s)=w840:i32[])
        n388 = Array Size(array=w837) -> (size(s)=w833:i32[])
        n389 = Array Size(array=w831) -> (size(s)=w827:i32[])
        n390 = Array Size(array=w816) -> (size(s)=w817:i32[])
        n391 = Index Array(array=w840, index=0) -> (element=w815:i32)
        n392 = Index Array(array=w833, index=0) -> (element=w811:i32)
        n393 = Index Array(array=w827, index=0) -> (element=w808:i32)
        n394 = Index Array(array=w817, index=0) -> (element=w805:i32)
        n395 = Subtract(x=w815, y=5) -> (x-y=w813:i32)
        n396 = Subtract(x=w811, y=5) -> (x-y=w810:i32)
        n397 = Subtract(x=w808, y=5) -> (x-y=w807:i32)
        n398 = Subtract(x=w805, y=5) -> (x-y=w804:i32)
        n399 = Index Array(array=w841, index (row)=w813) -> (element=w803:dbl[])  [unwired: 1 in]
        n400 = Index Array(array=w837, index (row)=w810) -> (element=w802:dbl[])  [unwired: 1 in]
        n401 = Index Array(array=w831, index (row)=w807) -> (element=w801:dbl[])  [unwired: 1 in]
        n402 = Index Array(array=w816, index (row)=w804) -> (element=w800:dbl[])  [unwired: 1 in]
        n403 = call "DownSampleAndShiftiRF (SubVI).vi"("ArrayIn"=w803) -> ("ArrayOut"=w799:dbl[])  [unwired: 10 in]
        n404 = call "DownSampleAndShiftiRF (SubVI).vi"("ArrayIn"=w802) -> ("ArrayOut"=w795:dbl[])  [unwired: 10 in]
        n405 = call "DownSampleAndShiftiRF (SubVI).vi"("ArrayIn"=w801) -> ("ArrayOut"=w796:dbl[])  [unwired: 10 in]
        n406 = call "DownSampleAndShiftiRF (SubVI).vi"("ArrayIn"=w800) -> ("ArrayOut"=w798:dbl[])  [unwired: 10 in]
        n407 = call <vilib>:"Add State(s) to Queue__JKI_lib_State_Machine.vi"("State(s) in (\"\")"=w849) -> ("States Out"=w848:string)  [unwired: 14 in]
        n408 = Bundle(cluster=w824, "Ch1 iRF"=w799, "Ch2 iRF"=w795, "Ch3 iRF"=w796, "Ch4 iRF"=w798) -> (w797:T19)
        n409 = global write "GlobalVariables.vi" "LastUseiRF"(w797) -> ()
      }
      frame "Data: loadLastUseiRF" {
        # "Load last use iRF.\n()"
        n410 = Unbundle By Name(w855) -> ("TempPath"=w854:path)
        n411 = Build Path(base path=w854, name or relative path="iRF.tdms") -> (appended path=w860:path)
        n412 = TDMS Open(8:w850, 11:w860) -> (0:w858:errorcluster, 3:w859:refnum<k34>)  [unwired: 5 in]
        n413 = TDMS Read(0:w859, 11:w858, 12:dbl[][] []) -> (4:w853:refnum<k34>, 10:w856:dbl[][], 15:w852:errorcluster)  [unwired: 5 in, 3 out]
        n414 = TDMS Close(8:w852, 11:w853) -> (0:w851:errorcluster)  [unwired: 1 out]
        n415 = case shown="No Error" w852 {
          tunnel: w856 -> [w874 _]
          frame No Error {
            w877 = T19 {"Ch1 iRF"=[], "Ch2 iRF"=[], "Ch3 iRF"=[], "Ch4 iRF"=[]}  # LastUseiRF
            n416 = Index Array(array=w874, index (row)=0) -> (element=w866:dbl[])  [unwired: 1 in]
            n417 = Index Array(array=w874, index (row)=1) -> (element=w868:dbl[])  [unwired: 1 in]
            n418 = Index Array(array=w874, index (row)=2) -> (element=w870:dbl[])  [unwired: 1 in]
            n419 = Index Array(array=w874, index (row)=3) -> (element=w872:dbl[])  [unwired: 1 in]
            n420 = call "TrancateData(SubVI).vi"("DataIn"=w866) -> ("DataOut"=w865:dbl[])  [unwired: 10 in]
            n421 = call "TrancateData(SubVI).vi"("DataIn"=w868) -> ("DataOut"=w867:dbl[])  [unwired: 10 in]
            n422 = call "TrancateData(SubVI).vi"("DataIn"=w870) -> ("DataOut"=w869:dbl[])  [unwired: 10 in]
            n423 = call "TrancateData(SubVI).vi"("DataIn"=w872) -> ("DataOut"=w871:dbl[])  [unwired: 10 in]
            n424 = Add Array Elements(numeric array=w865) -> (sum=w883:dbl)
            n425 = Add Array Elements(numeric array=w867) -> (sum=w881:dbl)
            n426 = Add Array Elements(numeric array=w869) -> (sum=w879:dbl)
            n427 = Add Array Elements(numeric array=w871) -> (sum=w875:dbl)
            n428 = Divide(x=w865, y=w883) -> (x/y=w882:dbl[])
            n429 = Divide(x=w867, y=w881) -> (x/y=w880:dbl[])
            n430 = Divide(x=w869, y=w879) -> (x/y=w878:dbl[])
            n431 = Divide(x=w871, y=w875) -> (x/y=w873:dbl[])
            n432 = Bundle(cluster=w877, "Ch1 iRF"=w882, "Ch2 iRF"=w880, "Ch3 iRF"=w878, "Ch4 iRF"=w873) -> (w885:T19)
            n433 = Array Size(array=w865) -> (size(s)=→"iRF length":i32)
            n434 = global write "GlobalVariables.vi" "LastUseiRF"(w885) -> ()
          }
          frame Error {
          }
        }
        n435 = call <vilib>:"Add State(s) to Queue__JKI_lib_State_Machine.vi"("State(s) in (\"\")"=w864) -> ("States Out"=w863:string)  [unwired: 14 in]
      }
      frame "Data: ShowiRF" {
        # "Show loaded iRF.\n(It is a separator no-op. You can make a copy of this frame to create a new Data frame)"
        n436 = global read "GlobalVariables.vi" "LastUseiRF"() -> (w894:T19)
        n437 = Unbundle By Name(w894) -> ("Ch1 iRF"=w893:dbl[], "Ch2 iRF"=w892:dbl[], "Ch3 iRF"=w891:dbl[], "Ch4 iRF"=w890:dbl[])
        n438 = Build Array(w893, w892, w891, w890) -> (→"iRF Graph":dbl[][])
        n439 = call <vilib>:"Add State(s) to Queue__JKI_lib_State_Machine.vi"("State(s) in (\"\")"=w899) -> ("States Out"=w898:string)  [unwired: 14 in]
      }
      frame "Data: saveCalibration" {
        # "Average data and save calibration file. [Covers: REQ11]\n(It is a separator no-op. You can make a copy of this frame to create a new Data frame)"
        n440 = Unbundle By Name(w918) -> ("Ch1Data"=w917:dbl[][], "V1"=w916:dbl[], "Ch2Data"=w915:dbl[][], "V2"=w914:dbl[], "Ch3Data"=w913:dbl[][], "V3"=w912:dbl[], "Ch4Data"=w903:dbl[][], "V4"=w902:dbl[], "Pathes.CaliPath"=w921:path, "IDs.Cali ID"=w920:i8)
        n441 = Increment(x=w920) -> (x+1=w904:i8)
        n442 = Bundle("Ch1Data"=w917, "V1"=w916) -> (w911:cluster{"Ch1Data":dbl[][], "V1":dbl[]})  [unwired: 1 in]
        n443 = Bundle("Ch4Data"=w903, "V4"=w902) -> (w901:cluster{"Ch4Data":dbl[][], "V4":dbl[]})  [unwired: 1 in]
        n444 = Bundle("Ch2Data"=w915, "V2"=w914) -> (w910:cluster{"Ch2Data":dbl[][], "V2":dbl[]})  [unwired: 1 in]
        n445 = Bundle("Ch3Data"=w913, "V3"=w912) -> (w909:cluster{"Ch3Data":dbl[][], "V3":dbl[]})  [unwired: 1 in]
        n446 = Format Value(string ("")="Calibration" ("default name"), format string="%02d", value (0)=w904) -> (output string=w923:string)
        n447 = Build Path(base path=w921, name or relative path=w923) -> (appended path=w908:path)
        n448 = call "SaveBGorCali(SubVI).vi"("Channel1"=w911, "BG path"=w908, "DataType"=enum16{"BG", "Cali"}."Cali", "Channel 2"=w910, "Channel 3"=w909, "Channel 4"=w901, "error in (no error)"=w907, "SytemID"="UCDVetMed") -> ("error out"=w906:errorcluster)  [unwired: 7 in]
        n449 = call <vilib>:"Add State(s) to Queue__JKI_lib_State_Machine.vi"("State(s) in (\"\")"=w926) -> ("States Out"=w925:string)  [unwired: 14 in]
      }
      frame "Data: saveiRF" {
        w932 = enum16{"write", "read"}."read" ("action")
        # "Get iRF from decon stracture and save it on disk.\n(It is a separator no-op. You can make a copy of this frame to create a new Data frame)"
        n450 = Unbundle By Name(w949) -> ("TempPath"=w948:path)
        n451 = call "Ch1DeconEngineFGV.vi"("action(read)"=w932) -> ("Error Out"=w954:errorcluster, "Ch1DeconEngine out"=w955:refnum<class "LaguerreDeconEngineClass.lvclass">)  [unwired: 9 in]
        n452 = call "Ch2DeconEngineFGV.vi"("action(read)"=w932) -> ("Error Out"=w952:errorcluster, "Ch2DeconEngine out"=w953:refnum<class "LaguerreDeconEngineClass.lvclass">)  [unwired: 9 in]
        n453 = call "Ch3DeconEngineFGV.vi"("action(read)"=w932) -> ("Error Out"=w950:errorcluster, "Ch3DeconEngine out"=w951:refnum<class "LaguerreDeconEngineClass.lvclass">)  [unwired: 9 in]
        n454 = call "Ch4DeconEngineFGV.vi"("action(read)"=w932) -> ("Error Out"=w931:errorcluster, "Ch3DeconEngine out"=w930:refnum<class "LaguerreDeconEngineClass.lvclass">)  [unwired: 9 in]
        n455 = Build Path(base path=w948, name or relative path="iRF" ("default name")) -> (appended path=w946:path)
        n456 = call "getIRF.vi"("error in (no error)"=w931, "LaguerreDeconEngineClass in"=w930) -> ("iRF"=w929:dbl[])  [unwired: 7 in, 2 out]
        n457 = call "getIRF.vi"("error in (no error)"=w954, "LaguerreDeconEngineClass in"=w955) -> ("iRF"=w937:dbl[])  [unwired: 7 in, 2 out]
        n458 = call "getIRF.vi"("error in (no error)"=w952, "LaguerreDeconEngineClass in"=w953) -> ("iRF"=w936:dbl[])  [unwired: 7 in, 2 out]
        n459 = call "getIRF.vi"("error in (no error)"=w950, "LaguerreDeconEngineClass in"=w951) -> ("iRF"=w935:dbl[])  [unwired: 7 in, 2 out]
        n460 = TDMS Open(8:w945, 10:T20."create or replace" ("operation (0:open)"), 11:w946) -> (0:w942:errorcluster, 3:w943:refnum<k34>)  [unwired: 4 in]
        n461 = Bundle(cluster=T19 {"Ch1 iRF"=[], "Ch2 iRF"=[], "Ch3 iRF"=[], "Ch4 iRF"=[]} ("LastUseiRF"), "Ch1 iRF"=w937, "Ch2 iRF"=w936, "Ch3 iRF"=w935, "Ch4 iRF"=w929) -> (w933:T19)
        n462 = Build Array(w937, w936, w935, w929) -> (w941:dbl[][])
        n463 = global write "GlobalVariables.vi" "LastUseiRF"(w933) -> ()
        n464 = TDMS Write(0:w943, 5:"iRF" ("group name in (Untitled)"), 7:string[] ["Ch1", "Ch2", "Ch3", "Ch4"] ("channel name(s) in (Untitled)"), 9:w941, 11:w942) -> (4:w940:refnum<k34>, 15:w939:errorcluster)  [unwired: 1 in, 2 out]
        n465 = TDMS Close(8:w939, 11:w940) -> (0:w938:errorcluster)  [unwired: 1 out]
        n466 = call <vilib>:"Add State(s) to Queue__JKI_lib_State_Machine.vi"("State(s) in (\"\")"=w958) -> ("States Out"=w957:string)  [unwired: 14 in]
      }
      frame "Data: saveBGtoFGV" {
        w959 = enum16{"write", "read"}."write" ("action")
        # "Save BG and pass it to FGV.\n(save BG to disk and set it to FGV)"
        n467 = Unbundle By Name(w969) -> ("Ch1Data"=w968:dbl[][], "Ch2Data"=w967:dbl[][], "Ch3Data"=w966:dbl[][], "Ch4Data"=w961:dbl[][])
        n468 = call "AvgArrayTimeCritical.vi"("2D array"=w968) -> ("1D Avg"=w965:dbl[])  [unwired: 10 in]
        n469 = call "AvgArrayTimeCritical.vi"("2D array"=w967) -> ("1D Avg"=w964:dbl[])  [unwired: 10 in]
        n470 = call "AvgArrayTimeCritical.vi"("2D array"=w966) -> ("1D Avg"=w963:dbl[])  [unwired: 10 in]
        n471 = call "AvgArrayTimeCritical.vi"("2D array"=w961) -> ("1D Avg"=w960:dbl[])  [unwired: 10 in]
        n472 = call "BG1FGV.vi"("action"=w959, "BG1 in"=w965) -> ()  [unwired: 8 in, 2 out]
        n473 = call "BG2FGV.vi"("action"=w959, "BG2 in"=w964) -> ()  [unwired: 8 in, 2 out]
        n474 = call "BG3FGV.vi"("action"=w959, "BG3 in"=w963) -> ()  [unwired: 8 in, 2 out]
        n475 = call "BG4FGV.vi"("action"=w959, "BG4 in"=w960) -> ()  [unwired: 8 in, 2 out]
        n476 = call <vilib>:"Add State(s) to Queue__JKI_lib_State_Machine.vi"("State(s) in (\"\")"=w972) -> ("States Out"=w971:string)  [unwired: 14 in]
      }
      frame "Data: saveBGtoFile" {
        w994 = "Background" ("name or relative path")
        # "Save BG to file.\n(save BG to disk both data folder and temp folder)"
        n477 = Unbundle By Name(w998) -> ("Pathes.BG Path"=w991:path, "IDs.BG ID"=w990:i8, "Ch1Data"=w988:dbl[][], "V1"=w987:dbl[], "Ch2Data"=w986:dbl[][], "V2"=w985:dbl[], "Ch3Data"=w984:dbl[][], "V3"=w983:dbl[], "Ch4Data"=w975:dbl[][], "V4"=w974:dbl[], "TempPath"=w996:path)
        n478 = Increment(x=w990) -> (x+1=w995:i8)
        n479 = Format Value(string ("")=w994, format string="%02d", value (0)=w995) -> (output string=w993:string)
        n480 = Build Path(base path=w996, name or relative path=w994) -> (appended path=w977:path)
        n481 = call "File Dialog2"("start path"=w991, "prompt"="Please select BG name, DO NOT CANCEL!", "default name"=w993) -> ("selected path"=w978:path)  [unwired: 9 in, 3 out]
        n482 = Bundle("Ch1Data"=w988, "V1"=w987) -> (w982:cluster{"Ch1Data":dbl[][], "V1":dbl[]})  [unwired: 1 in]
        n483 = Bundle("Ch4Data"=w975, "V4"=w974) -> (w973:cluster{"Ch4Data":dbl[][], "V4":dbl[]})  [unwired: 1 in]
        n484 = Bundle("Ch2Data"=w986, "V2"=w985) -> (w981:cluster{"Ch2Data":dbl[][], "V2":dbl[]})  [unwired: 1 in]
        n485 = Bundle("Ch3Data"=w984, "V3"=w983) -> (w980:cluster{"Ch3Data":dbl[][], "V3":dbl[]})  [unwired: 1 in]
        n486 = Build Array(w978, w977) -> (w976:path[])
        n487 = for {
          tunnel: w982 -> [w1009]
          tunnel: w981 -> [w1008]
          tunnel: w980 -> [w1007]
          shift-right: [w1010] -> w989
          shift-left: w979 -> [w1006]
          tunnel: w976 -> [w1005] mode=indexing
          tunnel: w973 -> [w1003]
          n488 = call "SaveBGorCali(SubVI).vi"("Channel1"=w1009, "BG path"=w1005, "DataType"=enum16{"BG", "Cali"}."BG", "Channel 2"=w1008, "Channel 3"=w1007, "Channel 4"=w1003, "error in (no error)"=w1006, "SytemID"="UCDVetMed") -> ("error out"=w1010:errorcluster)  [unwired: 7 in]
        }
        n489 = call <vilib>:"Add State(s) to Queue__JKI_lib_State_Machine.vi"("State(s) in (\"\")"=w1001) -> ("States Out"=w1000:string)  [unwired: 14 in]
      }
      frame "Data: showBG" {
        # "Show BG in seperate window.\n()"
        n490 = call "showBG.vi"() -> ()  [unwired: 12 in]
        n491 = call <vilib>:"Add State(s) to Queue__JKI_lib_State_Machine.vi"("State(s) in (\"\")"=w1015) -> ("States Out"=w1014:string)  [unwired: 14 in]
      }
      frame "Data: irfAlignment" {
        w1016 = enum16{"write", "read"}."write" ("action")
        # "do iRF alignment in this state\n(It is a separator no-op. You can make a copy of this frame to create a new Data frame)"
        n492 = Unbundle By Name(w1061) -> ("Ch1Data"=w1097:dbl[][], "Ch2Data"=w1096:dbl[][], "Ch3Data"=w1095:dbl[][], "Ch4Data"=w1038:dbl[][])
        n493 = call "Ch1DeconEngineFGV.vi"("Error In"=w1037) -> ("Error Out"=w1093:errorcluster, "Ch1DeconEngine out"=w1094:refnum<class "LaguerreDeconEngineClass.lvclass">)  [unwired: 9 in]
        n494 = call "Ch2DeconEngineFGV.vi"("Error In"=w1037) -> ("Error Out"=w1091:errorcluster, "Ch2DeconEngine out"=w1092:refnum<class "LaguerreDeconEngineClass.lvclass">)  [unwired: 9 in]
        n495 = call "Ch3DeconEngineFGV.vi"("Error In"=w1037) -> ("Error Out"=w1089:errorcluster, "Ch3DeconEngine out"=w1090:refnum<class "LaguerreDeconEngineClass.lvclass">)  [unwired: 9 in]
        n496 = call "Ch4DeconEngineFGV.vi"("Error In"=w1037) -> ("Error Out"=w1028:errorcluster, "Ch3DeconEngine out"=w1027:refnum<class "LaguerreDeconEngineClass.lvclass">)  [unwired: 9 in]
        n497 = call "AvgArray.vi"("2D array in"=w1096) -> ("1D Avg out"=w1043:dbl[])  [unwired: 10 in]
        n498 = call "AvgArray.vi"("2D array in"=w1095) -> ("1D Avg out"=w1042:dbl[])  [unwired: 10 in]
        n499 = call "AvgArray.vi"("2D array in"=w1038) -> ("1D Avg out"=w1017:dbl[])  [unwired: 10 in]
        n500 = call "AvgArray.vi"("2D array in"=w1097) -> ("1D Avg out"=w1044:dbl[])  [unwired: 10 in]
        n501 = call "RemoveDCBG.vi"("WF in"=w1044) -> ("DC"=w1051:dbl, "WF out"=w1041:dbl[])  [unwired: 8 in, 1 out]
        n502 = call "RemoveDCBG.vi"("WF in"=w1043) -> ("DC"=w1048:dbl, "WF out"=w1054:dbl[])  [unwired: 8 in, 1 out]
        n503 = call "RemoveDCBG.vi"("WF in"=w1042) -> ("DC"=w1046:dbl, "WF out"=w1053:dbl[])  [unwired: 8 in, 1 out]
        n504 = call "RemoveDCBG.vi"("WF in"=w1017) -> ("DC"=w1021:dbl, "WF out"=w1019:dbl[])  [unwired: 8 in, 1 out]
        n505 = call "computeIRFAlignment.vi"("error in (no error)"=w1093, "fIRF temp"=w1041, "LaguerreDeconEngineClass in"=w1094) -> ("error out"=w1085:errorcluster, "LaguerreDeconEngineClass out"=w1086:refnum<class "LaguerreDeconEngineClass.lvclass">)  [unwired: 6 in, 1 out]
        n506 = call "computeIRFAlignment.vi"("error in (no error)"=w1091, "fIRF temp"=w1054, "LaguerreDeconEngineClass in"=w1092) -> ("error out"=w1083:errorcluster, "LaguerreDeconEngineClass out"=w1084:refnum<class "LaguerreDeconEngineClass.lvclass">)  [unwired: 6 in, 1 out]
        n507 = call "computeIRFAlignment.vi"("error in (no error)"=w1089, "fIRF temp"=w1053, "LaguerreDeconEngineClass in"=w1090) -> ("error out"=w1087:errorcluster, "LaguerreDeconEngineClass out"=w1088:refnum<class "LaguerreDeconEngineClass.lvclass">)  [unwired: 6 in, 1 out]
        n508 = call "computeIRFAlignment.vi"("error in (no error)"=w1028, "fIRF temp"=w1019, "LaguerreDeconEngineClass in"=w1027) -> ("error out"=w1035:errorcluster, "LaguerreDeconEngineClass out"=w1036:refnum<class "LaguerreDeconEngineClass.lvclass">)  [unwired: 6 in, 1 out]
        n509 = call "Ch1DeconEngineFGV.vi"("Error In"=w1085, "action(read)"=w1016, "Ch1DeconEngine in"=w1086) -> ("Error Out"=w1081:errorcluster, "Ch1DeconEngine out"=w1082:refnum<class "LaguerreDeconEngineClass.lvclass">)  [unwired: 7 in]
        n510 = call "Ch2DeconEngineFGV.vi"("Error In"=w1083, "action(read)"=w1016, "Ch2DeconEngine in"=w1084) -> ("Error Out"=w1071:errorcluster, "Ch2DeconEngine out"=w1072:refnum<class "LaguerreDeconEngineClass.lvclass">)  [unwired: 7 in]
        n511 = call "Ch3DeconEngineFGV.vi"("Error In"=w1087, "action(read)"=w1016, "Ch3DeconEngine in"=w1088) -> ("Error Out"=w1065:errorcluster, "Ch3DeconEngine out"=w1066:refnum<class "LaguerreDeconEngineClass.lvclass">)  [unwired: 7 in]
        n512 = call "Ch4DeconEngineFGV.vi"("Error In"=w1035, "action(read)"=w1016, "Ch3DeconEngine in"=w1036) -> ("Error Out"=w1029:errorcluster, "Ch3DeconEngine out"=w1030:refnum<class "LaguerreDeconEngineClass.lvclass">)  [unwired: 7 in]
        n513 = call "setfIRF.vi"("error in (no error)"=w1065, "fIRF"=w1053, "LaguerreDeconEngineClass in"=w1066) -> ("error out"=w1069:errorcluster, "LaguerreDeconEngineClass out"=w1070:refnum<class "LaguerreDeconEngineClass.lvclass">)  [unwired: 7 in]
        n514 = call "setfIRF.vi"("error in (no error)"=w1029, "fIRF"=w1019, "LaguerreDeconEngineClass in"=w1030) -> ("error out"=w1033:errorcluster, "LaguerreDeconEngineClass out"=w1034:refnum<class "LaguerreDeconEngineClass.lvclass">)  [unwired: 7 in]
        n515 = call "setfIRF.vi"("error in (no error)"=w1071, "fIRF"=w1054, "LaguerreDeconEngineClass in"=w1072) -> ("error out"=w1075:errorcluster, "LaguerreDeconEngineClass out"=w1076:refnum<class "LaguerreDeconEngineClass.lvclass">)  [unwired: 7 in]
        n516 = call "setfIRF.vi"("error in (no error)"=w1081, "fIRF"=w1041, "LaguerreDeconEngineClass in"=w1082) -> ("error out"=w1079:errorcluster, "LaguerreDeconEngineClass out"=w1080:refnum<class "LaguerreDeconEngineClass.lvclass">)  [unwired: 7 in]
        n517 = Unbundle By Name(w1061) -> ("V1"=w1040:dbl[], "V2"=w1060:dbl[], "V3"=w1059:dbl[], "V4"=w1026:dbl[])
        n518 = call "computeLCs.vi"("error in (no error)"=w1079, "LaguerreDeconClass in"=w1080) -> ("error out"=w1077:errorcluster, "LaguerreDeconClass out"=w1078:refnum<class "LaguerreDeconEngineClass.lvclass">)  [unwired: 8 in]
        n519 = call "computeLCs.vi"("error in (no error)"=w1075, "LaguerreDeconClass in"=w1076) -> ("error out"=w1073:errorcluster, "LaguerreDeconClass out"=w1074:refnum<class "LaguerreDeconEngineClass.lvclass">)  [unwired: 8 in]
        n520 = call "computeLCs.vi"("error in (no error)"=w1069, "LaguerreDeconClass in"=w1070) -> ("error out"=w1067:errorcluster, "LaguerreDeconClass out"=w1068:refnum<class "LaguerreDeconEngineClass.lvclass">)  [unwired: 8 in]
        n521 = call "computeLCs.vi"("error in (no error)"=w1033, "LaguerreDeconClass in"=w1034) -> ("error out"=w1031:errorcluster, "LaguerreDeconClass out"=w1032:refnum<class "LaguerreDeconEngineClass.lvclass">)  [unwired: 8 in]
        n522 = call-poly <vilib>:"Mean.vi"("X"=w1040) -> ("mean"=w1039:dbl)  [unwired: 1 out]
        n523 = call-poly <vilib>:"Mean.vi"("X"=w1026) -> ("mean"=w1025:dbl)  [unwired: 1 out]
        n524 = call-poly <vilib>:"Mean.vi"("X"=w1060) -> ("mean"=w1058:dbl)  [unwired: 1 out]
        n525 = call "getFitting.vi"("error in (no error)"=w1077, "LaguerreDeconEngineClass in"=w1078) -> ("Fitting"=w1050:dbl[])  [unwired: 7 in, 2 out]
        n526 = call "getFitting.vi"("error in (no error)"=w1073, "LaguerreDeconEngineClass in"=w1074) -> ("Fitting"=w1047:dbl[])  [unwired: 7 in, 2 out]
        n527 = call "getFitting.vi"("error in (no error)"=w1067, "LaguerreDeconEngineClass in"=w1068) -> ("Fitting"=w1023:dbl[])  [unwired: 7 in, 2 out]
        n528 = call "getFitting.vi"("error in (no error)"=w1031, "LaguerreDeconEngineClass in"=w1032) -> ("Fitting"=w1022:dbl[])  [unwired: 7 in, 2 out]
        n529 = Add(x=w1051, y=w1050) -> (x+y=w1052:dbl[])
        n530 = Add(x=w1048, y=w1047) -> (x+y=w1049:dbl[])
        n531 = call-poly <vilib>:"Mean.vi"("X"=w1059) -> ("mean"=w1057:dbl)  [unwired: 1 out]
        n532 = Add(x=w1046, y=w1023) -> (x+y=w1045:dbl[])
        n533 = Build Array(w1044, w1052) -> (w1064:dbl[][])
        n534 = Build Array(w1043, w1049) -> (w1063:dbl[][])
        n535 = Build Array(w1042, w1045) -> (w1062:dbl[][])
        n536 = Add(x=w1021, y=w1022) -> (x+y=w1020:dbl[])
        n537 = Bundle("mean"=w1039, "mean"=w1058, "mean"=w1057, "mean"=w1025) -> (w1024:T39)  [unwired: 1 in]
        n538 = Build Array(w1017, w1020) -> (w1018:dbl[][])
        n539 = call "Calib_and_iRFAlign_confirm.vi"("Current V"=w1024, "Ch4 Data"=w1018, "Ch3 Data"=w1062, "Ch2 Data"=w1063, "Ch1 Data"=w1064) -> ("Save?"=w1056:bool)  [unwired: 6 in]
        n540 = case shown="True" w1056 {
          tunnel: ["" ("Empty String Constant") "Data: saveCalibration\nData: saveiRF\nRun: CaliIncrement"] -> w1055
          frame False {
          }
          frame True {
            # "[Covers: REQ2]"
          }
        }
        n541 = call <vilib>:"Add State(s) to Queue__JKI_lib_State_Machine.vi"("State(s) in Front (\"\")"=w1055, "State(s) in (\"\")"=w1100) -> ("States Out"=w1099:string)  [unwired: 13 in]
      }
      frame "Data: parseRunData" {
        # "All APD bias"
        # "flash queue"
        # "Ch3&4"
        # "Ch1&2"
        # "Flash data from queue and save it in structure\n()"
        n542 = Flush Queue(queue=w1128, error in (no error)=w1127) -> (remaining elements=w1122:T40, error out=w1123:errorcluster)  [unwired: 1 out]
        n543 = Flush Queue(queue=w1133, error in (no error)=w1127) -> (remaining elements=w1131:cluster{"double data":dbl[][]}[], error out=w1124:errorcluster)  [unwired: 1 out]
        n544 = Flush Queue(queue=w1134, error in (no error)=w1127) -> (remaining elements=w1132:cluster{"double data":dbl[][]}[], error out=w1125:errorcluster)  [unwired: 1 out]
        n545 = for {
          tunnel: w1132 -> [w1150] mode=indexing
          tunnel: [w1148] -> w1117 mode=concatenating
          tunnel: [w1147] -> w1118 mode=concatenating
          n546 = Unbundle By Name(w1150) -> ("double data"=w1149:dbl[][])
          n547 = call "SeperateChanData.vi"("Input (Ch1&2)"=w1149) -> ("Ch1"=w1148:dbl[][], "Ch2"=w1147:dbl[][])
        }
        n548 = for {
          tunnel: w1131 -> [w1146] mode=indexing
          tunnel: [w1145] -> w1107 mode=concatenating
          tunnel: [w1143] -> w1108 mode=concatenating
          n549 = Unbundle By Name(w1146) -> ("double data"=w1144:dbl[][])
          n550 = call "SeperateChanData.vi"("Input (Ch1&2)"=w1144) -> ("Ch1"=w1145:dbl[][], "Ch2"=w1143:dbl[][])
        }
        n551 = call "FLImDAQ_FGV.vi"() -> ("Read data"=w1115:T6)  [unwired: 10 in, 1 out]
        n552 = Unbundle By Name(w1115) -> ("Waveform to Avg"=w1105:i16)
        n553 = for {
          tunnel: w1122 -> [w1142] mode=indexing
          tunnel: [w1141] -> w1114 mode=indexing
          tunnel: [w1140] -> w1112 mode=indexing
          tunnel: [w1139] -> w1110 mode=indexing
          tunnel: [w1138] -> w1106 mode=indexing
          n554 = Unbundle By Name(w1142) -> ("V1"=w1141:dbl, "V2"=w1140:dbl, "V3"=w1139:dbl, "V4"=w1138:dbl)
        }
        n555 = call "DuplicateV(SubVI).vi"("Averaging"=w1105, "V in"=w1114) -> ("V out"=w1113:dbl[])  [unwired: 9 in]
        n556 = Array Size(array=w1107) -> (size(s)=→"data Size":i32[])
        n557 = call "DuplicateV(SubVI).vi"("Averaging"=w1105, "V in"=w1112) -> ("V out"=w1111:dbl[])  [unwired: 9 in]
        n558 = call "DuplicateV(SubVI).vi"("Averaging"=w1105, "V in"=w1110) -> ("V out"=w1109:dbl[])  [unwired: 9 in]
        n559 = call "DuplicateV(SubVI).vi"("Averaging"=w1105, "V in"=w1106) -> ("V out"=w1103:dbl[])  [unwired: 9 in]
        n560 = Bundle By Name(cluster=w1129, "Ch1Data"=w1117, "Ch2Data"=w1118, "Ch3Data"=w1107, "Ch4Data"=w1108, "V1"=w1113, "V2"=w1111, "V3"=w1109, "V4"=w1103) -> (w1130:T26)
        n561 = Merge Errors(w1125, w1124, w1123) -> (w1126:errorcluster)
        n562 = Array Size(array=w1113) -> (size(s)=→"V1 Size":i32)
        n563 = Array Size(array=w1111) -> (size(s)=→"V2 Size":i32)
        n564 = Array Size(array=w1109) -> (size(s)=→"V3 Size":i32)
        n565 = Array Size(array=w1103) -> (size(s)=→"V4 Size":i32)
        n566 = call <vilib>:"Add State(s) to Queue__JKI_lib_State_Machine.vi"("State(s) in (\"\")"=w1137) -> ("States Out"=w1136:string)  [unwired: 14 in]
      }
      frame "Data: saveRunData" {
        w1153 = T41 {"DataPath"=path "", "CaseID"="", "RunID"=0, "Ch1Data"=[], "Ch2Data"=[], "Ch3Data"=[], "Ch4Data"=[], "V1"=[], "V2"=[], "V3"=[], "V4"=[], "LaserRepRate"=0, "WFAverage"=0, "RunStartTime"=0}  # Data cluster
        # "Save FLIm data to disk.\n(Save to LV tdms file format)"
        n567 = Unbundle By Name(w1164) -> ("Pathes.DataPath"=w1160:path, "CaseID"=w1172:string, "IDs.RunID"=w1162:i8, "Ch1Data"=w1171:dbl[][], "Ch2Data"=w1170:dbl[][], "Ch3Data"=w1159:dbl[][], "Ch4Data"=w1152:dbl[][], "V1"=w1154:dbl[], "V2"=w1169:dbl[], "V3"=w1168:dbl[], "V4"=w1151:dbl[])
        n568 = call "FLImDAQ_FGV.vi"() -> ("Read data"=w1157:T6)  [unwired: 10 in, 1 out]
        n569 = Unbundle By Name(w1157) -> ("Waveform to Avg"=w1156:i16)
        n570 = local read "RunStartTime"() -> (w1155:u32)
        n571 = local read "Laser Rep Rate"() -> (w1158:dbl)
        n572 = Increment(x=w1162) -> (x+1=w1161:i8)
        n573 = Bundle By Name(cluster=w1153, "DataPath"=w1160, "CaseID"=w1172, "RunID"=w1161, "Ch1Data"=w1171, "Ch2Data"=w1170, "Ch3Data"=w1159, "Ch4Data"=w1152, "V1"=w1154, "V2"=w1169, "V3"=w1168, "V4"=w1151, "LaserRepRate"=w1158, "WFAverage"=w1156, "RunStartTime"=w1155) -> (w1167:T41)
        n574 = call "SaveRunData(SubVI).vi"("Data cluster"=w1167, "error in (no error)"=w1166) -> ("error out"=w1163:errorcluster)  [unwired: 13 in]
        n575 = flat-sequence {
          tunnel: w1164 -> [w1180]
          tunnel: [w1179] -> w1165
          tunnel: w1163 -> [_]
          frame #0 {
            w1177 = dbl[][] [] ("Ch1Data")
            w1178 = dbl[] [] ("V1")
            # "reset local data"
            n576 = Bundle By Name(cluster=w1180, "Ch1Data"=w1177, "Ch2Data"=w1177, "Ch3Data"=w1177, "Ch4Data"=w1177, "V1"=w1178, "V2"=w1178, "V3"=w1178, "V4"=w1178) -> (w1179:T26)
          }
        }
        n577 = case shown="No Error" w1163 {
          tunnel: ["Run: Increment" "" ("Empty String Constant")] -> w1173
          frame No Error {
          }
          frame Error {
          }
        }
        n578 = call <vilib>:"Add State(s) to Queue__JKI_lib_State_Machine.vi"("State(s) in Front (\"\")"=w1173, "State(s) in (\"\")"=w1176) -> ("States Out"=w1175:string)  [unwired: 13 in]
      }
      frame "Data: Cleanup" {
        # "Cleanup any data and references, here.\n(this is called automatically, by the Macro: Exit)"
        n579 = Unbundle By Name(w1184) -> ("Core.Current VI Reference"=w1187:refnum<vi>)
        n580 = Close Reference(reference=w1187, error in (no error)=w1186) -> (error out=w1185:errorcluster)
        n581 = call <vilib>:"Add State(s) to Queue__JKI_lib_State_Machine.vi"("State(s) in (\"\")"=w1189) -> ("States Out"=w1188:string)  [unwired: 14 in]
      }
      frame "---------- Core ----------" {
        # "Do not put any code in this frame.\n(it is a separator no-op)"
        n582 = call <vilib>:"Add State(s) to Queue__JKI_lib_State_Machine.vi"("State(s) in (\"\")"=w1194) -> ("States Out"=w1193:string)  [unwired: 14 in]
      }
      frame Default {
        w1205 = 42 items=["No error", "Argument error", "Memory is full", "Out of zone", "End of file", "File already open", "Generic file I/O error", "File not found", "File permission error", "Disk is full", "Duplicate path", "Too many files open", "System feature not enabled", "Resource file not found", "Cannot add resource", "Resource not found", "Image not found", "Image memory error", "Pen does not exist", "Config type invalid", "Config token not found", "Config parse error", "Config memory error", "Bad external code format", "Bad external code offset", "External code not present", "Null window", "Destroy window error", "Null menu", "Print aborted", "Bad print record", "Print driver error", "Windows error during printing", "Memory error during printing", "Print dialog error", "Generic print error", "Invalid device refnum", "Device not found", "Device parameter error", "Device unit error", "Cannot open device", "Device call aborted", "Generic error", "Cancelled by user", "Object ID too low", "Object ID too high", "Object not in heap", "Unknown heap", "Unknown object (invalid DefProc)", "Unknown object (DefProc not in table)", "Message out of range", "Invalid (null) method", "Unknown message", "Manager call not supported", "Bad address", "Network operation in progress", "Network operation timed out", "Connection is busy", "Network attribute not supported", "Network error", "Address in use", "System out of memory", "Connection aborted", "Connection refused", "Not connected", "Already connected", "Connection closed", "Initialization error (interapplication manager)", "Bad occurrence", "Wait on unbound occurrence handler", "Occurrence queue overflow", "Datalog type conflict", "Unused", "Unrecognized type (interapplication manager)", "Memory corrupt", "Failed to make temporary DLL", "Old CIN version", "Drag socket not found", "Failed to load drop-object", "Failed to register OLE object", "Failed to release OLE object", "Format specifier type mismatch", "Unknown format specifier", "Too few format specifiers", "Too many format specifiers", "Scan failed", "Newer CIN version", "Error converting to variant", "Runtime menu error", "Password tampered", "Variant attribute not found", "Incompatible variant data type", "Event data is not available", "Event Store is not present", "Occurrence is not found", "Event Queue is not created", "Event info is not available", "Refnum passed is NULL", "Error retrieving Class GUID", "Error retrieving CoClass GUID", "Error retrieving TypeLib GUID.", "Bad built application magic bytes.", "Specific driver is different from the specific driver associated with the Logical Name.", "There is no session opened to the class driver.", "Max Error", "MAX - Error with config objects", "MAX - Error loading configuration", "MAX - Group not supported"]
        # "Current State"
        # "Do not delete, rename, or modify this frame.\n(this is used to capture unhandled states and typos)"
        # "Handle mistyped state name (developer tool)"
        n583 = Format Into String(format string="Software Exception: Unhandled State \"%s\"." ("message"), error in=w1201, w1196) -> (resulting string=w1204:string, error out=w1203:errorcluster)  [unwired: 1 in]
        n584 = call <vilib>:"Error Cluster From Error Code.vi"("show call chain? (False)"=TRUE, "error in (no error)"=w1203, "error message (\"\")"=w1204, "error code (0)"=w1205) -> ("error out"=w1202:errorcluster)  [unwired: 5 in]
        n585 = call <vilib>:"Add State(s) to Queue__JKI_lib_State_Machine.vi"("State(s) in (\"\")"=w1200) -> ("States Out"=w1199:string)  [unwired: 14 in]
      }
      frame "Initialize Core Data" {
        # "Build default path based on the location of project"
        # "Do not delete, rename, or modify this frame.\n(this is used to determine panel behavior on exit)"
        # "originally closed?"
        # "exe?"
        # "If panel starts closed or is an EXE, then close it when we exit"
        n586 = call <vilib>:"Application Directory.vi"() -> ("Application Directory"=w1208:path)
        n587 = property on="Property Node" class="App"() -> ("App.Kind"=w1224:T22)  [unwired: 2 in, 2 out]
        n588 = property on="Property Node" class="VI"() -> ("FP.State"=w1218:T21)  [unwired: 2 in, 2 out]
        n589 = control-ref of="Current VI Reference"() -> (w1219:refnum<vi>)
        n590 = Equal?(x=w1218, y=T21."Closed" ("Front Panel Window:State")) -> (x = y?=w1216:bool)
        n591 = Strip Path(path=w1208) -> (stripped path=w1207:path)  [unwired: 1 out]
        n592 = Equal?(x=w1224, y=T22."Run Time System" ("Application:Kind")) -> (x = y?=w1222:bool)
        n593 = Build Path(base path=w1207, name or relative path="Data") -> (appended path=w1214:path)
        n594 = Build Path(base path=w1208, name or relative path="SystemTemp") -> (appended path=w1211:path)
        n595 = Build Path(base path=w1208, name or relative path="SystemCalibrationFile") -> (appended path=w1209:path)
        n596 = Or(x=w1216, y=w1222) -> (x .or. y?=w1220:bool)
        n597 = Bundle By Name(cluster=w1221, "Core.Current VI Reference"=w1219, "Core.Close Panel on Exit?"=w1220, "DefaultPath"=w1214, "TempPath"=w1211, "CaliPath"=w1209) -> (w1226:T26)
        n598 = call <vilib>:"Add State(s) to Queue__JKI_lib_State_Machine.vi"("State(s) in (\"\")"=w1228) -> ("States Out"=w1227:string)  [unwired: 14 in]
      }
      frame "Error Handler" {
        # "Unhandled Error -- Display it"
        # "Handle any errors here.\nYou can also output any states to clean-up after errors occur"
        # "Clear error"
        n599 = Unbundle By Name(w1229) -> ("code"=w1231:i32)
        n600 = case shown="Default" w1231 {
          tunnel: ["Macro: Exit" w1241 w1247] -> w1230
          tunnel: w1229 -> [w1237 _ _]
          frame Default {
            w1239 = T42 1 items=["no dialog", "OK message", "continue or stop message", "OK message + warnings", "continue/stop + warnings"] ("type of dialog (OK msg:1)")
            n601 = call <vilib>:"General Error Handler.vi"("type of dialog (OK msg:1)"=w1239, "error in (no error)"=w1237) -> ()  [unwired: 9 in, 5 out]
          }
          frame 5002 {
            n602 = Two Button Dialog(message="Laser interlock open! Please close interlock and try again! ", 1:"Safely Shutdown" ("F button name (\"Cancel\")"), 2:"OK" ("T button name (\"OK\")")) -> (T button?=w1242:bool)
            n603 = case shown="True" w1242 {
              tunnel: ["Macro: Exit" "355 Laser: CheckControllerStatus"] -> w1241
              frame False {
              }
              frame True {
              }
            }
          }
          frame 5001 {
            n604 = Two Button Dialog(message="Unable to connect to imaging computer, do you want to run data aquisiton alone? ", 1:"No" ("F button name (\"Cancel\")"), 2:"Yes" ("T button name (\"OK\")")) -> (T button?=w1248:bool)
            n605 = case shown="False" w1248 {
              tunnel: ["Macro: Exit" "" ("Empty String Constant")] -> w1247
              frame False {
              }
              frame True {
              }
            }
          }
        }
        n606 = call <vilib>:"Add State(s) to Queue__JKI_lib_State_Machine.vi"("State(s) in Front (\"\")"=w1230, "State(s) in (\"\")"=w1236) -> ("States Out"=w1235:string)  [unwired: 13 in]
      }
      frame "Exit" {
        # "Do not put any code in this frame.\n(No errors that occur here will be handled.)"
        n607 = call <vilib>:"Add State(s) to Queue__JKI_lib_State_Machine.vi"("State(s) in (\"\")"=w1259) -> ("States Out"=w1258:string)  [unwired: 14 in]
      }
      frame "---------- Case ----------" {
        # "Template Separator\n(You can make a copy of, or modify, this frame)"
        n608 = call <vilib>:"Add State(s) to Queue__JKI_lib_State_Machine.vi"("State(s) in (\"\")"=w1264) -> ("States Out"=w1263:string)  [unwired: 14 in]
      }
      frame "Case: getCaliID" {
        # "Get Calibration file #\n(You can make a copy of, or modify, this frame)"
        n609 = Unbundle By Name(w1265) -> ("Pathes.CaliPath"=w1268:path)
        n610 = call <vilib>:"Recursive File List.vi"("pattern"="*.tdms", "Treat LLBs as Folders?"=FALSE, "Folder Path"=w1268) -> ("All Files in Dir"=w1273:path[])  [unwired: 4 in, 4 out]
        n611 = for {
          tunnel: w1273 -> [w1283] mode=indexing
          tunnel: [w1282] -> w1272 mode=indexing
          tunnel: "Calibration" -> [w1279]
          n612 = Strip Path(path=w1283) -> (name=w1280:string)  [unwired: 1 out]
          n613 = Search and Replace String(input string=w1280, search string=w1279) -> (result string=w1278:string)  [unwired: 6 in, 3 out]
          n614 = Scan From String(format string="%d" ("string"), input string=w1278) -> (output 1=w1282:i32)  [unwired: 3 in, 3 out]
        }
        n615 = Array Max & Min(array=w1272) -> (max value=w1271:i32)  [unwired: 3 out]
        n616 = Bundle By Name(cluster=w1265, "IDs.Cali ID"=w1271) -> (w1266:T26)
        n617 = call <vilib>:"Add State(s) to Queue__JKI_lib_State_Machine.vi"("State(s) in (\"\")"=w1277) -> ("States Out"=w1276:string)  [unwired: 14 in]
      }
      frame "Case: getBGID" {
        # "Get background #\n(You can make a copy of, or modify, this frame)"
        n618 = Unbundle By Name(w1286) -> ("Pathes.BG Path"=w1291:path)
        n619 = call <vilib>:"Recursive File List.vi"("pattern"="*.tdms", "Treat LLBs as Folders?"=FALSE, "Folder Path"=w1291) -> ("All Files in Dir"=w1289:path[])  [unwired: 4 in, 4 out]
        n620 = for {
          tunnel: w1289 -> [w1306] mode=indexing
          tunnel: "Background" ("name or relative path") -> [w1304]
          shift-right: [w1297] -> w1284
          shift-left: 0 -> [w1301]
          n621 = Strip Path(path=w1306) -> (name=w1305:string)  [unwired: 1 out]
          n622 = Search and Replace String(input string=w1305, search string=w1304) -> (number of replacements=w1303:i32)  [unwired: 6 in, 3 out]
          n623 = Greater Than 0?(x=w1303) -> (x > 0?=w1302:bool)
          n624 = Select(t=1, s=w1302, f=0) -> (s? t:f=w1300:i32)
          n625 = Add(x=w1300, y=w1301) -> (x+y=w1297:i32)
        }
        n626 = Bundle By Name(cluster=w1286, "IDs.BG ID"=w1284) -> (w1287:T26)
        n627 = call <vilib>:"Add State(s) to Queue__JKI_lib_State_Machine.vi"("State(s) in (\"\")"=w1296) -> ("States Out"=w1295:string)  [unwired: 14 in]
      }
      frame "Case: getRunID" {
        # "Check folder for run ID\n(You can make a copy of, or modify, this frame)"
        n628 = Unbundle By Name(w1316) -> ("Pathes.DataPath"=w1315:path, "CaseID"=w1311:string)
        n629 = Build Array("Background" ("name or relative path"), "Calibration", "3DScanData" ("element")) -> (w1321:string[])
        n630 = call <vilib>:"Recursive File List.vi"("Folders to Exclude"=w1321, "pattern"="*.tdms", "Treat LLBs as Folders?"=FALSE, "Folder Path"=w1315) -> ("All Files in Dir"=w1312:path[])  [unwired: 3 in, 4 out]
        n631 = for {
          tunnel: w1312 -> [w1330] mode=indexing
          tunnel: [w1329] -> w1318 mode=indexing
          tunnel: w1311 -> [w1326]
          n632 = Strip Path(path=w1330) -> (name=w1327:string)  [unwired: 1 out]
          n633 = Search and Replace String(input string=w1327, search string=w1326) -> (result string=w1325:string)  [unwired: 6 in, 3 out]
          n634 = Scan From String(format string="_%d" ("string"), input string=w1325) -> (output 1=w1329:i32)  [unwired: 3 in, 3 out]
        }
        n635 = Array Max & Min(array=w1318) -> (max value=w1309:i32)  [unwired: 3 out]
        n636 = Bundle By Name(cluster=w1316, "IDs.RunID"=w1309) -> (w1317:T26)
        n637 = call "RunIDFGV.vi"("Error In"=w1307, "RunID in"=w1309) -> ("Error Out"=w1308:errorcluster)  [unwired: 8 in, 1 out]
        n638 = call <vilib>:"Add State(s) to Queue__JKI_lib_State_Machine.vi"("State(s) in (\"\")"=w1324) -> ("States Out"=w1323:string)  [unwired: 14 in]
      }
      frame "Case: CreatFileStruct" {
        # "Creat case file structure"
        n639 = Unbundle By Name(w1344) -> ("DefaultPath"=w1350:path, "CaseID"=w1337:string)
        n640 = Build Path(base path=w1350, name or relative path=w1337) -> (appended path=w1349:path)
        n641 = call <vilib>:"Check if File or Folder Exists.vi"("error in (no error)"=w1343, "path"=w1349) -> ("error out"=w1346:errorcluster, "file or folder exists?"=w1348:bool, "dup path"=w1347:path)  [unwired: 7 in]
        n642 = case shown="True" w1348 {
          tunnel: w1347 -> [w1367 w1375]
          tunnel: w1346 -> [w1365 w1370]
          tunnel: [w1359 w1375] -> w1335
          tunnel: [w1363 w1377] -> w1334
          tunnel: [u32 0 u32 0] -> w1333
          tunnel: [w1361 w1380] -> w1341
          tunnel: "Background" ("name or relative path") -> [w1360 w1372]
          tunnel: "Calibration" -> [w1358 w1371]
          tunnel: [w1354 w1373] -> w1338
          tunnel: w1337 -> [_ _]
          tunnel: ["" ("Empty String Constant") "Case: getRunID\nCase: getBGID\nCase: getCaliID\nUI: Update"] -> w1336
          frame False {
            # "Folder not exist. Creat folders."
            n643 = Create Folder(path (use dialog)=w1367, error in=w1365) -> (created path=w1359:path, error out=w1356:errorcluster)  [unwired: 1 in, 1 out]
            n644 = Build Path(base path=w1359, name or relative path=w1358) -> (appended path=w1357:path)
            n645 = Build Path(base path=w1359, name or relative path=w1360) -> (appended path=w1366:path)
            n646 = Create Folder(path (use dialog)=w1366, error in=w1356) -> (created path=w1361:path, error out=w1362:errorcluster)  [unwired: 1 in, 1 out]
            n647 = Create Folder(path (use dialog)=w1357, error in=w1356) -> (created path=w1354:path, error out=w1355:errorcluster)  [unwired: 1 in, 1 out]
            n648 = Merge Errors(w1362, w1355) -> (w1363:errorcluster)
          }
          frame True {
            # "Folder exsit, check file #"
            n649 = Build Path(base path=w1375, name or relative path=w1371) -> (appended path=w1376:path)
            n650 = Build Path(base path=w1375, name or relative path=w1372) -> (appended path=w1381:path)
            n651 = call <vilib>:"Check if File or Folder Exists.vi"("path"=w1376) -> ("file or folder exists?"=w1374:bool, "dup path"=w1373:path)  [unwired: 8 in, 1 out]
            n652 = call <vilib>:"Check if File or Folder Exists.vi"("path"=w1381) -> ("file or folder exists?"=w1379:bool, "dup path"=w1380:path)  [unwired: 8 in, 1 out]
            n653 = And(x=w1379, y=w1374) -> (x .and. y?=w1378:bool)
            n654 = case shown="False" w1378 {
              tunnel: w1370 -> [_ w1383]
              tunnel: [errorcluster {"status"=TRUE, "code"=5003, "source"="File structure error."} ("error out") w1383] -> w1377
              frame False {
              }
              frame True {
              }
            }
          }
        }
        n655 = Bundle By Name(cluster=w1344, "Pathes.DataPath"=w1335, "Pathes.BG Path"=w1341, "Pathes.CaliPath"=w1338, "IDs.RunID"=w1333, "IDs.BG ID"=w1333, "IDs.Cali ID"=w1333) -> (w1345:T26)
        n656 = call "DataRootPathFGV.vi"("Error In"=w1334, "PathIn"=w1335) -> ("Error Out"=w1332:errorcluster)  [unwired: 8 in, 1 out]
        n657 = call "RunIDFGV.vi"("Error In"=w1332, "RunID in"=w1333) -> ("Error Out"=w1331:errorcluster)  [unwired: 8 in, 1 out]
        n658 = call <vilib>:"Add State(s) to Queue__JKI_lib_State_Machine.vi"("State(s) in Front (\"\")"=w1336, "State(s) in (\"\")"=w1352) -> ("States Out"=w1351:string)  [unwired: 13 in]
      }
      frame "Case: GetID" {
        # "Template Separator\n(You can make a copy of, or modify, this frame)"
        n659 = call "set_subjectID.vi"() -> ("subject_id"=w1384:string)  [unwired: 10 in]
        n660 = Bundle By Name(cluster=w1386, "CaseID"=w1384) -> (w1387:T26)
        n661 = call <vilib>:"Add State(s) to Queue__JKI_lib_State_Machine.vi"("State(s) in (\"\")"=w1390) -> ("States Out"=w1389:string)  [unwired: 14 in]
      }
      frame "---------- DeconEngine ----------" {
        # "start data aquisition and then set irfAligh to ture and decon channel to 1,2 and 3."
        # "Template Separator\n(You can make a copy of, or modify, this frame)"
        n662 = call <vilib>:"Add State(s) to Queue__JKI_lib_State_Machine.vi"("State(s) in (\"\")"=w1395) -> ("States Out"=w1394:string)  [unwired: 14 in]
      }
      frame "DeconEngine: InitilizeMacro" {
        # "start data aquisition and then set irfAligh to ture and decon channel to 1,2 and 3."
        # "Initilize Decon Engine for all channel\n(You can make a copy of, or modify, this frame)"
        n663 = call <vilib>:"Add State(s) to Queue__JKI_lib_State_Machine.vi"("State(s) in Front (\"\")"="DeconEngine: InitializeCh1\nDeconEngine: InitializeCh2\nDeconEngine: InitializeCh3\nDeconEngine: InitializeCh4" ("State(s) in Front (\"\")"), "State(s) in (\"\")"=w1401) -> ("States Out"=w1400:string)  [unwired: 13 in]
      }
      frame "DeconEngine: InitializeCh1" {
        w1423 = refnum<class "LaguerreDeconEngineClass.lvclass"> refnum  # Ch1DeconObj
        # "Initilize Laguerre Deconvolution engine Object\n(You can make a copy of, or modify, this frame)"
        n664 = global read "GlobalVariables.vi" "LastUseiRF"() -> (w1404:T19)
        n665 = local read "Truncation"() -> (w1402:u32)
        n666 = call "setLaguerreOrder.vi"("error in (no error)"=w1411, "LaguerreOrder"=u32 12, "LaguerreDeconClass in"=w1423) -> ("error out"=w1420:errorcluster, "LaguerreDeconClass out"=w1421:refnum<class "LaguerreDeconEngineClass.lvclass">)  [unwired: 7 in]
        n667 = Unbundle By Name(w1404) -> ("Ch1 iRF"=w1403:dbl[])
        n668 = call "setDataLength.vi"("error in (no error)"=w1420, "dataLength"=w1402, "LaguerreDeconClass in"=w1421) -> ("error out"=w1419:errorcluster, "LaguerreDeconClass out"=w1418:refnum<class "LaguerreDeconEngineClass.lvclass">)  [unwired: 7 in]
        n669 = call "setIRF.vi"("error in (no error)"=w1419, "iRF"=w1403, "LaguerreDeconClass in"=w1418) -> ("error out"=w1416:errorcluster, "LaguerreDeconClass out"=w1417:refnum<class "LaguerreDeconEngineClass.lvclass">)  [unwired: 7 in]
        n670 = call "computeAlpha.vi"("error in (no error)"=w1416, "LaguerreDeconClass in"=w1417) -> ("error out"=w1414:errorcluster, "LaguerreDeconClass out"=w1415:refnum<class "LaguerreDeconEngineClass.lvclass">)  [unwired: 8 in]
        n671 = call "dataInitilize.vi"("error in (no error)"=w1414, "LaguerreDeconClass in"=w1415) -> ("error out"=w1412:errorcluster, "LaguerreDeconClass out"=w1413:refnum<class "LaguerreDeconEngineClass.lvclass">)  [unwired: 8 in]
        n672 = call "computeDeconMatrix.vi"("error in (no error)"=w1412, "LaguerreDeconClass in"=w1413) -> ("error out"=w1408:errorcluster, "LaguerreDeconClass out"=w1410:refnum<class "LaguerreDeconEngineClass.lvclass">)  [unwired: 8 in]
        n673 = call "Ch1DeconEngineFGV.vi"("Error In"=w1408, "action(read)"=enum16{"write", "read"}."write" ("action"), "Ch1DeconEngine in"=w1410) -> ("Error Out"=w1407:errorcluster)  [unwired: 7 in, 1 out]
        n674 = call <vilib>:"Add State(s) to Queue__JKI_lib_State_Machine.vi"("State(s) in (\"\")"=w1425) -> ("States Out"=w1424:string)  [unwired: 14 in]
      }
      frame "DeconEngine: InitializeCh2" {
        w1447 = refnum<class "LaguerreDeconEngineClass.lvclass"> refnum  # Ch2DeconObj
        # "Initilize Laguerre Deconvolution engine Object\n(You can make a copy of, or modify, this frame)"
        n675 = global read "GlobalVariables.vi" "LastUseiRF"() -> (w1428:T19)
        n676 = call "setLaguerreOrder.vi"("error in (no error)"=w1435, "LaguerreOrder"=u32 12, "LaguerreDeconClass in"=w1447) -> ("error out"=w1444:errorcluster, "LaguerreDeconClass out"=w1445:refnum<class "LaguerreDeconEngineClass.lvclass">)  [unwired: 7 in]
        n677 = local read "Truncation"() -> (w1426:u32)
        n678 = Unbundle By Name(w1428) -> ("Ch2 iRF"=w1427:dbl[])
        n679 = call "setDataLength.vi"("error in (no error)"=w1444, "dataLength"=w1426, "LaguerreDeconClass in"=w1445) -> ("error out"=w1443:errorcluster, "LaguerreDeconClass out"=w1442:refnum<class "LaguerreDeconEngineClass.lvclass">)  [unwired: 7 in]
        n680 = call "setIRF.vi"("error in (no error)"=w1443, "iRF"=w1427, "LaguerreDeconClass in"=w1442) -> ("error out"=w1440:errorcluster, "LaguerreDeconClass out"=w1441:refnum<class "LaguerreDeconEngineClass.lvclass">)  [unwired: 7 in]
        n681 = call "computeAlpha.vi"("error in (no error)"=w1440, "LaguerreDeconClass in"=w1441) -> ("error out"=w1438:errorcluster, "LaguerreDeconClass out"=w1439:refnum<class "LaguerreDeconEngineClass.lvclass">)  [unwired: 8 in]
        n682 = call "dataInitilize.vi"("error in (no error)"=w1438, "LaguerreDeconClass in"=w1439) -> ("error out"=w1436:errorcluster, "LaguerreDeconClass out"=w1437:refnum<class "LaguerreDeconEngineClass.lvclass">)  [unwired: 8 in]
        n683 = call "computeDeconMatrix.vi"("error in (no error)"=w1436, "LaguerreDeconClass in"=w1437) -> ("error out"=w1432:errorcluster, "LaguerreDeconClass out"=w1434:refnum<class "LaguerreDeconEngineClass.lvclass">)  [unwired: 8 in]
        n684 = call "Ch2DeconEngineFGV.vi"("Error In"=w1432, "action(read)"=enum16{"write", "read"}."write" ("action"), "Ch2DeconEngine in"=w1434) -> ("Error Out"=w1431:errorcluster)  [unwired: 7 in, 1 out]
        n685 = call <vilib>:"Add State(s) to Queue__JKI_lib_State_Machine.vi"("State(s) in (\"\")"=w1449) -> ("States Out"=w1448:string)  [unwired: 14 in]
      }
      frame "DeconEngine: InitializeCh3" {
        w1451 = refnum<class "LaguerreDeconEngineClass.lvclass"> refnum  # Ch3DeconObj
        # "Initilize Laguerre Deconvolution engine Object\n(You can make a copy of, or modify, this frame)"
        n686 = global read "GlobalVariables.vi" "LastUseiRF"() -> (w1453:T19)
        n687 = local read "Truncation"() -> (w1450:u32)
        n688 = call "setLaguerreOrder.vi"("error in (no error)"=w1460, "LaguerreOrder"=u32 12, "LaguerreDeconClass in"=w1451) -> ("error out"=w1469:errorcluster, "LaguerreDeconClass out"=w1470:refnum<class "LaguerreDeconEngineClass.lvclass">)  [unwired: 7 in]
        n689 = Unbundle By Name(w1453) -> ("Ch3 iRF"=w1452:dbl[])
        n690 = call "setDataLength.vi"("error in (no error)"=w1469, "dataLength"=w1450, "LaguerreDeconClass in"=w1470) -> ("error out"=w1468:errorcluster, "LaguerreDeconClass out"=w1467:refnum<class "LaguerreDeconEngineClass.lvclass">)  [unwired: 7 in]
        n691 = call "setIRF.vi"("error in (no error)"=w1468, "iRF"=w1452, "LaguerreDeconClass in"=w1467) -> ("error out"=w1465:errorcluster, "LaguerreDeconClass out"=w1466:refnum<class "LaguerreDeconEngineClass.lvclass">)  [unwired: 7 in]
        n692 = call "computeAlpha.vi"("error in (no error)"=w1465, "LaguerreDeconClass in"=w1466) -> ("error out"=w1463:errorcluster, "LaguerreDeconClass out"=w1464:refnum<class "LaguerreDeconEngineClass.lvclass">)  [unwired: 8 in]
        n693 = call "dataInitilize.vi"("error in (no error)"=w1463, "LaguerreDeconClass in"=w1464) -> ("error out"=w1461:errorcluster, "LaguerreDeconClass out"=w1462:refnum<class "LaguerreDeconEngineClass.lvclass">)  [unwired: 8 in]
        n694 = call "computeDeconMatrix.vi"("error in (no error)"=w1461, "LaguerreDeconClass in"=w1462) -> ("error out"=w1457:errorcluster, "LaguerreDeconClass out"=w1459:refnum<class "LaguerreDeconEngineClass.lvclass">)  [unwired: 8 in]
        n695 = call "Ch3DeconEngineFGV.vi"("Error In"=w1457, "action(read)"=enum16{"write", "read"}."write" ("action"), "Ch3DeconEngine in"=w1459) -> ("Error Out"=w1456:errorcluster)  [unwired: 7 in, 1 out]
        n696 = call <vilib>:"Add State(s) to Queue__JKI_lib_State_Machine.vi"("State(s) in (\"\")"=w1473) -> ("States Out"=w1472:string)  [unwired: 14 in]
      }
      frame "DeconEngine: InitializeCh4" {
        w1475 = refnum<class "LaguerreDeconEngineClass.lvclass"> refnum  # Ch3DeconObj
        # "Initilize Laguerre Deconvolution engine Object\n(You can make a copy of, or modify, this frame)"
        n697 = global read "GlobalVariables.vi" "LastUseiRF"() -> (w1477:T19)
        n698 = local read "Truncation"() -> (w1474:u32)
        n699 = call "setLaguerreOrder.vi"("error in (no error)"=w1484, "LaguerreOrder"=u32 12, "LaguerreDeconClass in"=w1475) -> ("error out"=w1493:errorcluster, "LaguerreDeconClass out"=w1494:refnum<class "LaguerreDeconEngineClass.lvclass">)  [unwired: 7 in]
        n700 = Unbundle By Name(w1477) -> ("Ch4 iRF"=w1476:dbl[])
        n701 = call "setDataLength.vi"("error in (no error)"=w1493, "dataLength"=w1474, "LaguerreDeconClass in"=w1494) -> ("error out"=w1492:errorcluster, "LaguerreDeconClass out"=w1491:refnum<class "LaguerreDeconEngineClass.lvclass">)  [unwired: 7 in]
        n702 = call "setIRF.vi"("error in (no error)"=w1492, "iRF"=w1476, "LaguerreDeconClass in"=w1491) -> ("error out"=w1489:errorcluster, "LaguerreDeconClass out"=w1490:refnum<class "LaguerreDeconEngineClass.lvclass">)  [unwired: 7 in]
        n703 = call "computeAlpha.vi"("error in (no error)"=w1489, "LaguerreDeconClass in"=w1490) -> ("error out"=w1487:errorcluster, "LaguerreDeconClass out"=w1488:refnum<class "LaguerreDeconEngineClass.lvclass">)  [unwired: 8 in]
        n704 = call "dataInitilize.vi"("error in (no error)"=w1487, "LaguerreDeconClass in"=w1488) -> ("error out"=w1485:errorcluster, "LaguerreDeconClass out"=w1486:refnum<class "LaguerreDeconEngineClass.lvclass">)  [unwired: 8 in]
        n705 = call "computeDeconMatrix.vi"("error in (no error)"=w1485, "LaguerreDeconClass in"=w1486) -> ("error out"=w1481:errorcluster, "LaguerreDeconClass out"=w1483:refnum<class "LaguerreDeconEngineClass.lvclass">)  [unwired: 8 in]
        n706 = call "Ch4DeconEngineFGV.vi"("Error In"=w1481, "action(read)"=enum16{"write", "read"}."write" ("action"), "Ch3DeconEngine in"=w1483) -> ("Error Out"=w1480:errorcluster)  [unwired: 7 in, 1 out]
        n707 = call <vilib>:"Add State(s) to Queue__JKI_lib_State_Machine.vi"("State(s) in (\"\")"=w1497) -> ("States Out"=w1496:string)  [unwired: 14 in]
      }
      frame "---------- Digitizer ----------" {
        # "Template Separator\n(You can make a copy of, or modify, this frame)"
        n708 = call <vilib>:"Add State(s) to Queue__JKI_lib_State_Machine.vi"("State(s) in (\"\")"=w1502) -> ("States Out"=w1501:string)  [unwired: 14 in]
      }
      frame "Digitizer: Initialize" {
        # "reset digitizer to everytime the system runs"
        # "reset digitizer to everytime the system runs"
        # "Initialize digitizer.\nInitialize both digitizer and update status."
        n709 = call "FLImDAQ_FGV.vi"("error in (no error)"=w1510) -> ("error out"=w1504:errorcluster, "Read data"=w1509:T6)  [unwired: 9 in]
        n710 = Unbundle By Name(w1512) -> ("SysConfigCluster.Ch1Enable?"=w1517:bool, "SysConfigCluster.Ch2Enable?"=w1516:bool, "SysConfigCluster.Ch3Enable?"=w1514:bool)
        n711 = Unbundle By Name(w1509) -> ("Digitizer 1"=w1505:refnum<k15>, "Digitizer 2"=w1508:refnum<k15>)
        n712 = property on="Digitizer" class="Bool (strict)"("Blinking"=TRUE) -> ()  [unwired: 2 in, 2 out]
        n713 = Or(x=w1517, y=w1516) -> (x .or. y?=w1515:bool)
        n714 = case shown="True" w1515 {
          tunnel: w1504 -> [w1525 w1528]
          tunnel: [w1525 w1527] -> w1506
          tunnel: w1505 -> [_ w1529]
          frame False {
          }
          frame True {
            n715 = call <instrlib>:"niScope Initialize.vi"("resource name"=w1529, "reset device"=TRUE, "error in"=w1528) -> ("error out"=w1527:errorcluster)  [unwired: 11 in, 1 out]
          }
        }
        n716 = case shown="True" w1514 {
          tunnel: w1504 -> [w1520 w1522]
          tunnel: [w1520 w1524] -> w1511
          tunnel: w1508 -> [_ w1523]
          frame False {
          }
          frame True {
            n717 = call <instrlib>:"niScope Initialize.vi"("resource name"=w1523, "reset device"=TRUE, "error in"=w1522) -> ("error out"=w1524:errorcluster)  [unwired: 11 in, 1 out]
          }
        }
        n718 = Merge Errors(w1506, w1511) -> (w1503:errorcluster)
        n719 = call <vilib>:"Add State(s) to Queue__JKI_lib_State_Machine.vi"("State(s) in (\"\")"=w1519) -> ("States Out"=w1518:string)  [unwired: 14 in]
      }
      frame "Digitizer: Config" {
        # "Synchronize is taking time ~3s."
        # "Config  digitizer\nCall subVi to config digitizer"
        n720 = call "FLImDAQ_FGV.vi"() -> ("Read data"=w1547:T6)  [unwired: 10 in, 1 out]
        n721 = Unbundle By Name(w1556) -> ("SysConfigCluster.Ch1Enable?"=w1564:bool, "SysConfigCluster.Ch2Enable?"=w1563:bool, "SysConfigCluster.Ch3Enable?"=w1561:bool, "FLImDAQ"=w1558:T33)
        n722 = Unbundle By Name(w1547) -> ("Digitizer 1"=w1550:refnum<k15>, "Digitizer 2"=w1549:refnum<k15>)
        n723 = property on="Digitizer" class="Bool (strict)"(error in=w1551, "Blinking"=TRUE) -> (error out=w1552:errorcluster)  [unwired: 1 in, 1 out]
        n724 = Or(x=w1564, y=w1563) -> (x .or. y?=w1562:bool)
        n725 = case shown="True" w1562 {
          tunnel: w1558 -> [_ w1577]
          tunnel: w1552 -> [w1573 w1576]
          tunnel: [w1573 w1575] -> w1559
          tunnel: w1550 -> [_ w1574]
          frame False {
          }
          frame True {
            n726 = call "DigitizerConfig.vi"("error in (no error)"=w1576, "FLImDAQ"=w1577, "IVI Refnum in"=w1574) -> ("error out"=w1575:errorcluster)  [unwired: 7 in, 1 out]
          }
        }
        n727 = case shown="True" w1561 {
          tunnel: w1558 -> [_ w1572]
          tunnel: w1559 -> [w1567 w1571]
          tunnel: [w1567 w1570] -> w1535
          tunnel: w1549 -> [_ w1568]
          frame False {
          }
          frame True {
            n728 = call "DigitizerConfig.vi"("Config Trigger? (T)"=FALSE ("Config Trigge(T)r:"), "error in (no error)"=w1571, "FLImDAQ"=w1572, "IVI Refnum in"=w1568) -> ("error out"=w1570:errorcluster)  [unwired: 6 in, 1 out]
          }
        }
        n729 = call "Digitizer1_FGV.vi"("error in (no error)"=w1535) -> ("error out"=w1545:errorcluster, "Read data"=w1546:refnum<k15>)  [unwired: 9 in]
        n730 = call <instrlib>:"niScope Get Session Reference.vi"("instrument handle"=w1546, "error in"=w1545) -> ("session reference"=w1539:refnum<k20>, "error out"=w1537:errorcluster)  [unwired: 11 in, 1 out]
        n731 = call "Digitizer2_FGV.vi"("error in (no error)"=w1537) -> ("error out"=w1543:errorcluster, "Read data"=w1544:refnum<k15>)  [unwired: 9 in]
        n732 = call <instrlib>:"niScope Get Session Reference.vi"("instrument handle"=w1544, "error in"=w1543) -> ("session reference"=w1538:refnum<k20>, "error out"=w1536:errorcluster)  [unwired: 11 in, 1 out]
        n733 = Build Array(w1539, w1538) -> (w1542:refnum<k20>[])
        n734 = call <instrlib>:"niTClk Configure For Homogeneous Triggers.vi"("error in (no error)"=w1536, "sessions"=w1542) -> ("error out"=w1541:errorcluster, "sessions out"=w1540:refnum<k20>[])  [unwired: 8 in]
        n735 = call <instrlib>:"niTClk Synchronize.vi"("error in (no error)"=w1541, "sessions"=w1540) -> ("error out"=w1534:errorcluster, "sessions out"=w1532:refnum<k20>[])  [unwired: 8 in]
        n736 = call <userlib>:"Wait (ms)__ogtk.vi"("error in (no error)"=w1534, "milliseconds to wait"=u32 1500) -> ("error out"=w1530:errorcluster)  [unwired: 8 in, 1 out]
        n737 = Unbundle By Name(w1530) -> ("status"=w1555:bool)
        n738 = Not(x=w1555) -> (.not. x?=w1554:bool)
        n739 = Bundle By Name(cluster=w1556, "System Status.Digitizer"=w1554, "niTClk sessions"=w1532) -> (w1557:T26)
        n740 = property on="Digitizer" class="Bool (strict)"(error in=w1530, "Blinking"=FALSE) -> (error out=w1548:errorcluster)  [unwired: 1 in, 1 out]
        n741 = call <vilib>:"Add State(s) to Queue__JKI_lib_State_Machine.vi"("State(s) in (\"\")"=w1566) -> ("States Out"=w1565:string)  [unwired: 14 in]
      }
      frame "Digitizer: Start" {
        # "send trigger to start acquisition loop"
        # "initilize aquisition"
        # "Start Digitizer\n(TClk start)"
        n742 = Unbundle By Name(w1585) -> ("niTClk sessions"=w1584:refnum<k20>[])
        n743 = call <instrlib>:"niTClk Initiate.vi"("error in (no error)"=w1578, "sessions"=w1584) -> ("error out"=w1580:errorcluster)  [unwired: 8 in, 1 out]
        n744 = Generate User Event(priority (normal)=usereventprio."high priority", user event=w1581, event data cluster=TRUE ("event data"), error in=w1580) -> (error out=w1579:errorcluster)  [unwired: 1 out]
        n745 = call <vilib>:"Add State(s) to Queue__JKI_lib_State_Machine.vi"("State(s) in (\"\")"=w1588) -> ("States Out"=w1587:string)  [unwired: 14 in]
      }
      frame "Digitizer: Abort" {
        # "Template Separator\n(You can make a copy of, or modify, this frame)"
        n746 = call "Digitizer1_FGV.vi"("error in (no error)"=w1592, "Operation (Read)"=enum16{"Write", "Read"}."Read" ("Operation")) -> ("error out"=w1599:errorcluster, "Read data"=w1596:refnum<k15>)  [unwired: 8 in]
        n747 = call "Digitizer2_FGV.vi"("error in (no error)"=w1592, "Operation (Read)"=enum16{"Write", "Read"}."Read" ("Operation")) -> ("error out"=w1595:errorcluster, "Read data"=w1597:refnum<k15>)  [unwired: 8 in]
        n748 = Bundle By Name(cluster=w1589, "SysRunning?"=FALSE ("System Status")) -> (w1590:T26)
        n749 = call <instrlib>:"niScope Abort.vi"("instrument handle"=w1596, "error in"=w1599) -> ("error out"=w1601:errorcluster)  [unwired: 12 in, 1 out]
        n750 = call <instrlib>:"niScope Abort.vi"("instrument handle"=w1597, "error in"=w1595) -> ("error out"=w1600:errorcluster)  [unwired: 12 in, 1 out]
        n751 = Merge Errors(w1601, w1600) -> (w1593:errorcluster)
        n752 = call <vilib>:"Add State(s) to Queue__JKI_lib_State_Machine.vi"("State(s) in (\"\")"=w1604) -> ("States Out"=w1603:string)  [unwired: 14 in]
      }
      frame "Digitizer: checkTemp" {
        w1607 = 65.0 ("y")
        w1612 = enum16{"Write", "Read"}."Read" ("Operation")
        # "Template Separator\n(You can make a copy of, or modify, this frame)"
        n753 = call "Digitizer1_FGV.vi"("Operation (Read)"=w1612) -> ("error out"=w1613:errorcluster, "Read data"=w1614:refnum<k15>)  [unwired: 9 in]
        n754 = call "Digitizer2_FGV.vi"("Operation (Read)"=w1612) -> ("error out"=w1610:errorcluster, "Read data"=w1611:refnum<k15>)  [unwired: 9 in]
        n755 = property on="Property Node" class="niScope"(reference=w1611, error in=w1610) -> ("Device Temperature"=w1608:dbl)  [unwired: 2 out]
        "Dig2 Temp" <- w1608
        n756 = property on="Property Node" class="niScope"(reference=w1614, error in=w1613) -> ("Device Temperature"=w1609:dbl)  [unwired: 2 out]
        "Dig1 Temp" <- w1609
        n757 = Greater?(x=w1609, y=w1607) -> (0:w1606:bool)
        n758 = Greater?(x=w1608, y=w1607) -> (0:w1605:bool)
        n759 = case shown="True" w1606 {
          frame False {
          }
          frame True {
            n760 = One Button Dialog(message="Digitizer 1 over heating!", button name ("OK")="OK") -> ()  [unwired: 1 out]
          }
        }
        n761 = case shown="True" w1605 {
          frame False {
          }
          frame True {
            n762 = One Button Dialog(message="Digitizer 2 over heating!", button name ("OK")="OK") -> ()  [unwired: 1 out]
          }
        }
        n763 = call <vilib>:"Add State(s) to Queue__JKI_lib_State_Machine.vi"("State(s) in (\"\")"=w1619) -> ("States Out"=w1618:string)  [unwired: 14 in]
      }
      frame "Digitizer: Close" {
        # "Close Digitizer"
        n764 = call "Digitizer1_FGV.vi"("error in (no error)"=w1629, "Operation (Read)"=enum16{"Write", "Read"}."Read" ("Operation")) -> ("error out"=w1631:errorcluster, "Read data"=w1635:refnum<k15>)  [unwired: 8 in]
        n765 = call "Digitizer2_FGV.vi"("error in (no error)"=w1629, "Operation (Read)"=enum16{"Write", "Read"}."Read" ("Operation")) -> ("error out"=w1630:errorcluster, "Read data"=w1633:refnum<k15>)  [unwired: 8 in]
        n766 = call <instrlib>:"niScope Close.vi"("instrument handle"=w1635, "error in"=w1631) -> ("error out"=w1628:errorcluster)  [unwired: 13 in]
        n767 = call <instrlib>:"niScope Close.vi"("instrument handle"=w1633, "error in"=w1630) -> ("error out"=w1627:errorcluster)  [unwired: 13 in]
        n768 = Merge Errors(w1628, w1627) -> (w1626:errorcluster)
        n769 = Unbundle By Name(w1626) -> ("status"=w1625:bool)
        n770 = Bundle By Name(cluster=w1636, "System Status.Digitizer"=w1625) -> (w1637:T26)
        n771 = call <vilib>:"Add State(s) to Queue__JKI_lib_State_Machine.vi"("State(s) in (\"\")"=w1639) -> ("States Out"=w1638:string)  [unwired: 14 in]
      }
      frame "---------- LabJack ----------" {
        # "Template Separator\n(You can make a copy of, or modify, this frame)"
        n772 = call <vilib>:"Add State(s) to Queue__JKI_lib_State_Machine.vi"("State(s) in (\"\")"=w1644) -> ("States Out"=w1643:string)  [unwired: 14 in]
      }
      frame "LabJack: checkPedal" {
        # "Template Separator\n(You can make a copy of, or modify, this frame)"
        n773 = Unbundle By Name(w1645) -> ("LJ Pinout.Foot Pedal"=w1649:string)
        n774 = call "LabJack_FGV.vi"("Operation(Read)"=enum16{"Write", "Read"}."Read" ("Operation"), "error in (no error)"=w1647) -> ("error out"=w1651:errorcluster, "Read data"=w1652:i32)  [unwired: 8 in]
        n775 = call "LJM_eReadName.vi"("Handle In"=w1652, "Name"=w1649, "error in"=w1651) -> ("Value"=w1650:dbl, "error out"=w1648:errorcluster)  [unwired: 10 in, 1 out]
        n776 = case shown="1" w1650 {
          tunnel: w1645 -> [w1657 w1660]
          tunnel: [w1657 w1658] -> w1646
          frame 0, Default {
          }
          frame 1 {
            # "If Pedal pressed"
            n777 = Tick Count (ms)() -> (millisecond timer value=w1664:u32)
            n778 = Unbundle By Name(w1660) -> ("Last Trigger"=w1659:u32)
            n779 = Subtract(x=w1664, y=w1659) -> (x-y=w1663:u32)
            n780 = Greater Or Equal?(x=w1663, y=u32 2000) -> (x >= y?=w1661:bool)
            n781 = case shown="True" w1661 {
              tunnel: w1660 -> [w1665 w1666]
              tunnel: w1659 -> [_ _]
              tunnel: [w1665 w1667] -> w1658
              frame False {
              }
              frame True {
                n782 = Tick Count (ms)() -> (millisecond timer value=w1668:u32)
                n783 = Unbundle By Name(w1666) -> ("SysRunning?"=w1669:bool)
                n784 = case shown="False" w1669 {
                  frame False {
                    n785 = property on="StartButton" class="Bool (strict)"("Val(Sgnl)"=TRUE ("Value (Signaling)")) -> ()  [unwired: 2 in, 2 out]
                  }
                  frame True {
                    n786 = property on="StopButton" class="Bool (strict)"("Val(Sgnl)"=TRUE ("Value (Signaling)")) -> ()  [unwired: 2 in, 2 out]
                  }
                }
                n787 = Bundle By Name(cluster=w1666, "Last Trigger"=w1668) -> (w1667:T26)
              }
            }
          }
        }
        n788 = call <vilib>:"Add State(s) to Queue__JKI_lib_State_Machine.vi"("State(s) in (\"\")"=w1656) -> ("States Out"=w1655:string)  [unwired: 14 in]
      }
      frame "LabJack: ZeroV" {
        # "Just Zero V\nDO not update FGV and front panel\nWIll resume from last V"
        # "set bias to 0"
        # "Zero APD bias\n(You can make a copy of, or modify, this frame)"
        n789 = Unbundle By Name(w1674) -> ("LJ Pinout.Ch1 Bias"=w1679:string, "LJ Pinout.Ch2 Bias"=w1678:string, "LJ Pinout.Ch3 Bias"=w1677:string)
        n790 = Build Array(w1679, w1678, w1677) -> (w1676:string[])
        n791 = call "LabJack_FGV.vi"("Operation(Read)"=enum16{"Write", "Read"}."Read" ("Operation"), "error in (no error)"=w1673) -> ("error out"=w1680:errorcluster, "Read data"=w1681:i32)  [unwired: 8 in]
        n792 = call "LJM_eWriteNames.vi"("Handle In"=w1681, "aNames"=w1676, "aValuesIn"=dbl[] [0.0, 0.0, 0.0], "error in"=w1680) -> ("error out"=w1672:errorcluster)  [unwired: 9 in, 2 out]
        n793 = call <vilib>:"Add State(s) to Queue__JKI_lib_State_Machine.vi"("State(s) in (\"\")"=w1685) -> ("States Out"=w1684:string)  [unwired: 14 in]
      }
      frame "LabJack: SetV" {
        w1692 = enum16{"write", "read"}."read" ("action (write)")
        # "set bias to user specifid"
        # "Set APD bias\n(You can make a copy of, or modify, this frame)"
        n794 = Unbundle By Name(w1701) -> ("LJ Pinout.Ch1 Bias"=w1705:string, "LJ Pinout.Ch2 Bias"=w1704:string, "LJ Pinout.Ch3 Bias"=w1703:string, "LJ Pinout.Ch4 Bias"=w1695:string)
        n795 = call "V2FGV.vi"("Error In"=w1691, "action(write)"=w1692) -> ("Error Out"=w1689:errorcluster, "V2 out"=w1697:dbl)  [unwired: 8 in]
        n796 = call "V4FGV.vi"("Error In"=w1691, "action(write)"=w1692) -> ("Error Out"=w1687:errorcluster, "V3 out"=w1693:dbl)  [unwired: 8 in]
        n797 = call "V1FGV.vi"("Error In"=w1691, "action (write)"=w1692) -> ("Error Out"=w1690:errorcluster, "V1 out"=w1694:dbl)  [unwired: 8 in]
        n798 = call "V3FGV.vi"("Error In"=w1691, "action(write)"=w1692) -> ("Error Out"=w1688:errorcluster, "V3 out"=w1696:dbl)  [unwired: 8 in]
        n799 = local write "V 3"(w1696) -> ()
        n800 = local write "V 2"(w1697) -> ()
        n801 = local write "V 4"(w1693) -> ()
        n802 = local write "V 1"(w1694) -> ()
        n803 = Build Array(w1705, w1704, w1703, w1695) -> (w1702:string[])
        n804 = call "LabJack_FGV.vi"("Operation(Read)"=enum16{"Write", "Read"}."Read" ("Operation"), "error in (no error)"=w1691) -> ("error out"=w1706:errorcluster, "Read data"=w1707:i32)  [unwired: 8 in]
        n805 = Build Array(w1694, w1697, w1696, w1693) -> (w1698:dbl[])
        n806 = call "LJM_eWriteNames.vi"("Handle In"=w1707, "aNames"=w1702, "aValuesIn"=w1698, "error in"=w1706) -> ("error out"=w1699:errorcluster)  [unwired: 9 in, 2 out]
        n807 = Merge Errors(w1690, w1689, w1688, w1687) -> (w1686:errorcluster)
        n808 = call <vilib>:"Add State(s) to Queue__JKI_lib_State_Machine.vi"("State(s) in (\"\")"=w1711) -> ("States Out"=w1710:string)  [unwired: 14 in]
        n809 = Merge Errors(w1686, w1699) -> (w1700:errorcluster)
      }
      frame "LabJack: Open" {
        # "Initialize LabJack T7\nEstablish connection and initialize pins"
        n810 = call "LJ_Open.vi"("error in"=w1721, "DeviceType"="LJM_dtT7") -> ("error out"=w1718:errorcluster, "Success?"=w1719:bool, "Handle Out"=w1713:i32)  [unwired: 7 in]
        n811 = call "LabJack_FGV.vi"("Operation(Read)"=enum16{"Write", "Read"}."Write" ("Operation"), "error in (no error)"=w1718, "Write data"=w1713) -> ("error out"=w1715:errorcluster)  [unwired: 7 in, 1 out]
        n812 = Bundle By Name(cluster=w1716, "System Status.Labjack"=w1719) -> (w1720:T26)
        n813 = call <vilib>:"Add State(s) to Queue__JKI_lib_State_Machine.vi"("State(s) in (\"\")"=w1723) -> ("States Out"=w1722:string)  [unwired: 14 in]
      }
      frame "LabJack: SetDefaultSub" {
        w1733 = enum16{"write", "read"}."write" ("action")
        w1734 = 0.0 ("V1 in")
        w1747 = "_EF_ENABLE" ("string")
        # "1. Disable PWM\n2. Set all V to 0\n3. Set 355 relay to open\n4. Set LED to off"
        # "read once to set DIO to input"
        # "set all initila V to 0. Set footpedal to input. Set PWM to low. Set laser relay to open. Set LEDs to yellow."
        # "Set Labjack to correct input and output state and initial values"
        n814 = disable-structure shown="Disabled" {
          frame Disabled {
            (unwired) dbl[] [0.0, 0.0, 0.0, 0.0, 0.0, 0.0, 0.0, 0.0, 0.0] ("aValuesIn")
          }
          frame Enabled {
          }
        }
        n815 = Unbundle By Name(w1744) -> ("LJ Pinout.355 PWM"=w1749:string, "LJ Pinout.AimingBeam PWM"=w1748:string, "LJ Pinout.Ch1 Bias"=w1754:string, "LJ Pinout.Ch2 Bias"=w1724:string, "LJ Pinout.Ch3 Bias"=w1758:string, "LJ Pinout.Ch4 Bias"=w1738:string, "LJ Pinout.Laser Start/Stop"=w1757:string, "LJ Pinout.Red LED"=w1756:string, "LJ Pinout.Green LED"=w1755:string)
        n816 = call "V1FGV.vi"("Error In"=w1742, "action (write)"=w1733, "V1 in"=w1734) -> ("Error Out"=w1737:errorcluster, "V1 out"=w1741:dbl)  [unwired: 7 in]
        n817 = local write "V 1"(w1741) -> ()
        n818 = call "V2FGV.vi"("Error In"=w1737, "action(write)"=w1733, "V2 in"=w1734) -> ("Error Out"=w1736:errorcluster, "V2 out"=w1740:dbl)  [unwired: 7 in]
        n819 = call "LabJack_FGV.vi"("Operation(Read)"=enum16{"Write", "Read"}."Read" ("Operation"), "error in (no error)"=w1742) -> ("error out"=w1730:errorcluster, "Read data"=w1752:i32)  [unwired: 8 in]
        n820 = Concatenate Strings(w1749, w1747) -> (w1746:string)
        n821 = Concatenate Strings(w1748, w1747) -> (w1745:string)
        n822 = local write "V 2"(w1740) -> ()
        n823 = call "V3FGV.vi"("Error In"=w1736, "action(write)"=w1733, "V3 in"=w1734) -> ("Error Out"=w1735:errorcluster, "V3 out"=w1739:dbl)  [unwired: 7 in]
        n824 = Build Array(w1746, w1745, w1754, w1724, w1758, w1738, w1757, w1756, w1755) -> (w1728:string[])
        n825 = local write "V 3"(w1739) -> ()
        n826 = call "V4FGV.vi"("Error In"=w1735, "action(write)"=w1733, "V3 in"=w1734) -> ("Error Out"=w1731:errorcluster, "V3 out"=w1732:dbl)  [unwired: 7 in]
        n827 = Array Size(array=w1728) -> (size(s)=w1727:i32)
        n828 = local write "V 4"(w1732) -> ()
        n829 = Initialize Array(0.0 ("element"), w1727) -> (w1725:dbl[])
        n830 = Unbundle By Name(w1744) -> ("LJ Pinout.Foot Pedal"=w1743:string)
        n831 = call "LJM_eWriteNames.vi"("Handle In"=w1752, "aNames"=w1728, "aValuesIn"=w1725, "error in"=w1730) -> ("Handle Out"=w1751:i32, "error out"=w1750:errorcluster)  [unwired: 9 in, 1 out]
        n832 = call "LJM_eReadName.vi"("Handle In"=w1751, "Name"=w1743, "error in"=w1750) -> ("error out"=w1729:errorcluster)  [unwired: 10 in, 2 out]
        n833 = case shown="Error .." w1729 {
          frame No Error {
            # "no error"
          }
          frame Error {
            # "handle error"
            n834 = One Button Dialog(message="Labjack error! The pin assignment is likely wrong. Please check pin setting of Labjack. Program will terminate.", button name ("OK")="OK") -> ()  [unwired: 1 out]
          }
        }
        n835 = call <vilib>:"Add State(s) to Queue__JKI_lib_State_Machine.vi"("State(s) in (\"\")"=w1761) -> ("States Out"=w1760:string)  [unwired: 14 in]
      }
      frame "LabJack: FootPedalConfig" {
        # "Setup footPedal\n(You can make a copy of, or modify, this frame)"
        n836 = call "LabJack_FGV.vi"("Operation(Read)"=enum16{"Write", "Read"}."Read" ("Operation"), "error in (no error)"=w1765) -> ("error out"=w1769:errorcluster, "Read data"=w1770:i32)  [unwired: 8 in]
        n837 = call "LJM_eWriteName.vi"("Handle In"=w1770, "Name"="DIO15", "Value"=1.0, "error in"=w1769) -> ("error out"=w1766:errorcluster)  [unwired: 10 in, 1 out]
        n838 = call <vilib>:"Add State(s) to Queue__JKI_lib_State_Machine.vi"("State(s) in (\"\")"=w1774) -> ("States Out"=w1773:string)  [unwired: 14 in]
      }
      frame "LabJack: SetDefaultAndClose" {
        # "Template Separator\n(You can make a copy of, or modify, this frame)"
        n839 = call <vilib>:"Add State(s) to Queue__JKI_lib_State_Machine.vi"("State(s) in Front (\"\")"="LabJack: SetDefaultSub\nLabJack: Close" ("State(s) in Front (\"\")"), "State(s) in (\"\")"=w1780) -> ("States Out"=w1779:string)  [unwired: 13 in]
      }
      frame "LabJack: Close" {
        # "Close LabJack Refnum"
        n840 = call "LabJack_FGV.vi"("Operation(Read)"=enum16{"Write", "Read"}."Read" ("Operation"), "error in (no error)"=w1786) -> ("error out"=w1781:errorcluster, "Read data"=w1782:i32)  [unwired: 8 in]
        n841 = Bundle By Name(cluster=w1784, "System Status.Labjack"=FALSE ("System Status.Gain Control")) -> (w1787:T26)
        n842 = call "LJM_Close.vi"("error in"=w1781, "Handle"=w1782) -> ("error out"=w1789:errorcluster)  [unwired: 9 in]
        n843 = call <vilib>:"Add State(s) to Queue__JKI_lib_State_Machine.vi"("State(s) in (\"\")"=w1791) -> ("States Out"=w1790:string)  [unwired: 14 in]
      }
      frame "LabJack: Interlock enable/disable" {
        w1800 = i8 0  # int8
        # "[Covers: REQ8]"
        # "Interlock enable/disable\n(Usage: \"LabJack: Interlock enable/disable >> 1|0\")"
        n844 = Fract/Exp String To Number(string=w1801, default (0 dbl)=w1800) -> (number=w1797:i8)  [unwired: 2 in, 1 out]
        n845 = Unbundle By Name(w1799) -> ("LJ Pinout.Interlock"=w1798:string)
        n846 = call "LabJack_FGV.vi"("Operation(Read)"=enum16{"Write", "Read"}."Read" ("Operation")) -> ("Read data"=w1795:i32)  [unwired: 9 in, 1 out]
        n847 = call "LJM_eWriteName.vi"("Handle In"=w1795, "Name"=w1798, "Value"=w1797, "error in"=w1796) -> ("error out"=w1793:errorcluster)  [unwired: 10 in, 1 out]
        n848 = call <vilib>:"Add State(s) to Queue__JKI_lib_State_Machine.vi"("State(s) in (\"\")"=w1803) -> ("States Out"=w1802:string)  [unwired: 14 in]
      }
      frame "LabJack: 355_PWM_Config" {
        w1805 = 0.0 ("element")
        w1825 = "DIO_EF_CLOCK1_ENABLE"
        # "Config PWM frequency"
        n849 = Unbundle By Name(w1817) -> ("LJ Pinout.355 PWM"=w1824:string)
        n850 = Unbundle By Name(w1817) -> ("355 PWM setting.DIO_EF_CLOCK1_DIVISOR"=w1816:i16, "355 PWM setting.DIO_EF_CLOCK1_ROLL_VALUE"=w1815:i32, "355 PWM setting.DIO#_EF_INDEX"=w1812:i16, "355 PWM setting.DIO#_EF_OPTIONS"=w1811:i16, "355 PWM setting.DIO#_EF_CONFIG_A"=w1810:i32)
        n851 = Concatenate Strings(w1824, "_EF_ENABLE" ("string")) -> (w1820:string)
        n852 = Concatenate Strings(w1824, "_EF_INDEX") -> (w1823:string)
        n853 = Concatenate Strings(w1824, "_EF_OPTIONS") -> (w1822:string)
        n854 = Concatenate Strings(w1824, "_EF_CONFIG_A") -> (w1821:string)
        n855 = call "LabJack_FGV.vi"("Operation(Read)"=enum16{"Write", "Read"}."Read" ("Operation")) -> ("Read data"=w1818:i32)  [unwired: 9 in, 1 out]
        n856 = Build Array(w1805, w1805, w1816, w1815, 1.0 ("element"), 0.0 ("element"), w1812, w1811, w1810) -> (w1809:dbl[])
        n857 = Build Array("DIO_EF_CLOCK0_ENABLE", w1825, "DIO_EF_CLOCK1_DIVISOR", "DIO_EF_CLOCK1_ROLL_VALUE", w1825, w1820, w1823, w1822, w1821) -> (w1819:string[])
        n858 = call "LJM_eWriteNames.vi"("Handle In"=w1818, "aNames"=w1819, "aValuesIn"=w1809, "error in"=w1807) -> ("error out"=w1808:errorcluster)  [unwired: 9 in, 2 out]
        n859 = call <vilib>:"Add State(s) to Queue__JKI_lib_State_Machine.vi"("State(s) in (\"\")"=w1834) -> ("States Out"=w1833:string)  [unwired: 14 in]
      }
      frame "LabJack: 355_PWM_Start" {
        # "Template Separator\n(You can make a copy of, or modify, this frame)"
        n860 = Unbundle By Name(w1842) -> ("LJ Pinout.355 PWM"=w1841:string)
        n861 = call "LabJack_FGV.vi"("Operation(Read)"=enum16{"Write", "Read"}."Read" ("Operation"), "error in (no error)"=w1836) -> ("error out"=w1843:errorcluster, "Read data"=w1844:i32)  [unwired: 8 in]
        n862 = Concatenate Strings(w1841, "_EF_ENABLE" ("string")) -> (w1839:string)
        n863 = call "LJM_eWriteName.vi"("Handle In"=w1844, "Name"=w1839, "Value"=1.0, "error in"=w1843) -> ("error out"=w1837:errorcluster)  [unwired: 10 in, 1 out]
        n864 = call <vilib>:"Add State(s) to Queue__JKI_lib_State_Machine.vi"("State(s) in (\"\")"=w1847) -> ("States Out"=w1846:string)  [unwired: 14 in]
      }
      frame "LabJack: 355_PWM_Stop" {
        # "Template Separator\n(You can make a copy of, or modify, this frame)"
        n865 = Unbundle By Name(w1853) -> ("LJ Pinout.355 PWM"=w1857:string)
        n866 = call "LabJack_FGV.vi"("Operation(Read)"=enum16{"Write", "Read"}."Read" ("Operation"), "error in (no error)"=w1852) -> ("error out"=w1858:errorcluster, "Read data"=w1850:i32)  [unwired: 8 in]
        n867 = Concatenate Strings(w1857, "_EF_ENABLE" ("string")) -> (w1855:string)
        n868 = call "LJM_eWriteName.vi"("Handle In"=w1850, "Name"=w1855, "Value"=0.0, "error in"=w1858) -> ("error out"=w1849:errorcluster)  [unwired: 10 in, 1 out]
        n869 = local write "355nm Laser toggle"(FALSE ("355nm Laser toggle")) -> ()
        n870 = call <vilib>:"Add State(s) to Queue__JKI_lib_State_Machine.vi"("State(s) in (\"\")"=w1861) -> ("States Out"=w1860:string)  [unwired: 14 in]
      }
      frame "LabJack: AB_Start" {
        # "Aiming Beam Start\n(Based on aimging beam frequency, set LabJack pin)"
        n871 = Unbundle By Name(w1871) -> ("AB Cluster.Freq"=w1863:i32, "LJ Pinout.AimingBeam PWM"=w1870:string)
        n872 = Greater Than 0?(x=w1863) -> (x > 0?=w1862:bool)
        n873 = case shown="False" w1862 {
          tunnel: w1870 -> [w1877 w1880]
          tunnel: [w1877 w1878] -> w1869
          frame False {
            # "if 0 freq, set PWM pin"
          }
          frame True {
            # "if non zero freq, set PWM enable"
            n874 = Concatenate Strings(w1880, "_EF_ENABLE" ("string")) -> (w1878:string)
          }
        }
        n875 = call "LabJack_FGV.vi"("Operation(Read)"=enum16{"Write", "Read"}."Read" ("Operation"), "error in (no error)"=w1866) -> ("error out"=w1872:errorcluster, "Read data"=w1873:i32)  [unwired: 8 in]
        n876 = call "LJM_eWriteName.vi"("Handle In"=w1873, "Name"=w1869, "Value"=1.0, "error in"=w1872) -> ("error out"=w1867:errorcluster)  [unwired: 10 in, 1 out]
        n877 = local write "Aiming beam toggle"(TRUE ("Aiming beam toggle")) -> ()
        n878 = call <vilib>:"Add State(s) to Queue__JKI_lib_State_Machine.vi"("State(s) in (\"\")"=w1876) -> ("States Out"=w1875:string)  [unwired: 14 in]
      }
      frame "LabJack: AB_Stop" {
        # "Aiming Beam Stop\n(Based on aiming beam frequency, set LabJack pin low)"
        n879 = Unbundle By Name(w1888) -> ("AB Cluster.Freq"=w1883:i32, "LJ Pinout.AimingBeam PWM"=w1890:string)
        n880 = Greater Than 0?(x=w1883) -> (x > 0?=w1882:bool)
        n881 = case shown="False" w1882 {
          tunnel: w1890 -> [w1896 w1899]
          tunnel: [w1896 w1897] -> w1881
          frame False {
          }
          frame True {
            n882 = Concatenate Strings(w1899, "_EF_ENABLE" ("string")) -> (w1897:string)
          }
        }
        n883 = call "LabJack_FGV.vi"("Operation(Read)"=enum16{"Write", "Read"}."Read" ("Operation"), "error in (no error)"=w1886) -> ("error out"=w1891:errorcluster, "Read data"=w1892:i32)  [unwired: 8 in]
        n884 = call "LJM_eWriteName.vi"("Handle In"=w1892, "Name"=w1881, "Value"=0.0, "error in"=w1891) -> ("error out"=w1887:errorcluster)  [unwired: 10 in, 1 out]
        n885 = local write "Aiming beam toggle"(FALSE ("Aiming beam toggle")) -> ()
        n886 = call <vilib>:"Add State(s) to Queue__JKI_lib_State_Machine.vi"("State(s) in (\"\")"=w1895) -> ("States Out"=w1894:string)  [unwired: 14 in]
      }
      frame "LabJack: AB_PWM_Config" {
        w1901 = 0.0 ("element")
        w1921 = "DIO_EF_CLOCK2_ENABLE"
        # "Config PWM frequency"
        n887 = Unbundle By Name(w1913) -> ("LJ Pinout.AimingBeam PWM"=w1920:string)
        n888 = Unbundle By Name(w1913) -> ("AB PWM setting.DIO_EF_CLOCK1_DIVISOR"=w1912:i16, "AB PWM setting.DIO_EF_CLOCK1_ROLL_VALUE"=w1911:i32, "AB PWM setting.DIO#_EF_INDEX"=w1908:i16, "AB PWM setting.DIO#_EF_OPTIONS"=w1907:i16, "AB PWM setting.DIO#_EF_CONFIG_A"=w1906:i32)
        n889 = Concatenate Strings(w1920, "_EF_ENABLE" ("string")) -> (w1916:string)
        n890 = Concatenate Strings(w1920, "_EF_INDEX") -> (w1919:string)
        n891 = Concatenate Strings(w1920, "_EF_OPTIONS") -> (w1918:string)
        n892 = Concatenate Strings(w1920, "_EF_CONFIG_A") -> (w1917:string)
        n893 = call "LabJack_FGV.vi"("Operation(Read)"=enum16{"Write", "Read"}."Read" ("Operation")) -> ("Read data"=w1914:i32)  [unwired: 9 in, 1 out]
        n894 = Build Array(w1901, w1901, w1912, w1911, 1.0 ("element"), 0.0 ("element"), w1908, w1907, w1906) -> (w1905:dbl[])
        n895 = Build Array("DIO_EF_CLOCK0_ENABLE", w1921, "DIO_EF_CLOCK2_DIVISOR", "DIO_EF_CLOCK2_ROLL_VALUE", w1921, w1916, w1919, w1918, w1917) -> (w1915:string[])
        n896 = call "LJM_eWriteNames.vi"("Handle In"=w1914, "aNames"=w1915, "aValuesIn"=w1905, "error in"=w1903) -> ("error out"=w1904:errorcluster)  [unwired: 9 in, 2 out]
        n897 = call <vilib>:"Add State(s) to Queue__JKI_lib_State_Machine.vi"("State(s) in (\"\")"=w1930) -> ("States Out"=w1929:string)  [unwired: 14 in]
      }
      frame "---------- LED ----------" {
        # "Template Separator\n(You can make a copy of, or modify, this frame)"
        n898 = call <vilib>:"Add State(s) to Queue__JKI_lib_State_Machine.vi"("State(s) in (\"\")"=w1935) -> ("States Out"=w1934:string)  [unwired: 14 in]
      }
      frame "LED: OpenVIRef" {
        # "Template Separator\n(You can make a copy of, or modify, this frame)"
        n899 = call <vilib>:"Application Directory.vi"() -> ("Application Directory"=w1942:path)
        n900 = Build Path(base path=w1942, name or relative path="SubVI") -> (appended path=w1940:path)
        n901 = Build Path(base path=w1940, name or relative path="LEDBreath.vi") -> (appended path=w1938:path)
        n902 = Open VI Reference(vi path=w1938, error in (no error)=w1943) -> (vi reference=w1944:refnum<vi>, error out=w1937:errorcluster)  [unwired: 4 in]
        n903 = case shown="Error .." w1937 {
          tunnel: [TRUE FALSE] -> w1936
          frame No Error {
          }
          frame Error {
          }
        }
        n904 = Bundle By Name(cluster=w1945, "LED vi reference"=w1944, "LED vi ref open?"=w1936) -> (w1946:T26)
        n905 = call <vilib>:"Add State(s) to Queue__JKI_lib_State_Machine.vi"("State(s) in (\"\")"=w1949) -> ("States Out"=w1948:string)  [unwired: 14 in]
      }
      frame "LED: CloseVIRef" {
        # "Template Separator\n(You can make a copy of, or modify, this frame)"
        n906 = Unbundle By Name(w1953) -> ("LED vi reference"=w1954:refnum<vi>, "LED vi ref open?"=w1952:bool)
        n907 = case shown="True" w1952 {
          tunnel: w1956 -> [w1960 w1963]
          tunnel: [w1960 w1962] -> w1955
          tunnel: w1954 -> [_ w1961]
          frame False {
          }
          frame True {
            n908 = Close Reference(reference=w1961, error in (no error)=w1963) -> (error out=w1962:errorcluster)
          }
        }
        n909 = call <vilib>:"Add State(s) to Queue__JKI_lib_State_Machine.vi"("State(s) in (\"\")"=w1959) -> ("States Out"=w1958:string)  [unwired: 14 in]
      }
      frame "LED: BreathGreen" {
        w1964 = FALSE ("Wait Until Done")
        # "Breath system LED\n(LED: Breath >> True/False)"
        n910 = Unbundle By Name(w1972) -> ("LED vi reference"=w1971:refnum<vi>)
        n911 = invoke class="VI" method="Ctrl Val.Set"(reference=w1971, error in=w1969, "Control Name"="Color", "Value"=0) -> (reference out=w1968:refnum<vi>, error out=w1967:errorcluster)  [unwired: 1 in, 3 out]
        n912 = invoke on="Invoke Node" class="VI" method="Run VI"(reference=w1968, error in=w1967, "Wait until done"=w1964, "Auto Dispose Ref"=w1964) -> (error out=w1970:errorcluster)  [unwired: 1 in, 4 out]
        n913 = call <vilib>:"Add State(s) to Queue__JKI_lib_State_Machine.vi"("State(s) in (\"\")"=w1975) -> ("States Out"=w1974:string)  [unwired: 14 in]
      }
      frame "LED: BreathOrange" {
        w1976 = FALSE ("Wait Until Done")
        # "Breath system LED\n(LED: Breath >> True/False)"
        n914 = Unbundle By Name(w1984) -> ("LED vi reference"=w1983:refnum<vi>)
        n915 = invoke class="VI" method="Ctrl Val.Set"(reference=w1983, error in=w1981, "Control Name"="Color", "Value"=1) -> (reference out=w1980:refnum<vi>, error out=w1979:errorcluster)  [unwired: 1 in, 3 out]
        n916 = invoke on="Invoke Node" class="VI" method="Run VI"(reference=w1980, error in=w1979, "Wait until done"=w1976, "Auto Dispose Ref"=w1976) -> (error out=w1982:errorcluster)  [unwired: 1 in, 4 out]
        n917 = call <vilib>:"Add State(s) to Queue__JKI_lib_State_Machine.vi"("State(s) in (\"\")"=w1987) -> ("States Out"=w1986:string)  [unwired: 14 in]
      }
      frame "LED: BreathOff" {
        # "System LED Breath Off\n(Breath off, check VI status to make sure it is off)"
        n918 = Unbundle By Name(w1996) -> ("LED vi reference"=w1995:refnum<vi>)
        n919 = invoke on="Invoke Node" class="VI" method="Ctrl Val.Set"(reference=w1995, error in=w1993, "Control Name"="Stop", "Value"=TRUE) -> (reference out=w1988:refnum<vi>, error out=w1989:errorcluster)  [unwired: 1 in, 3 out]
        n920 = case shown="No Error" w1989 {
          selector: w1989 -> [w2001 _]
          tunnel: [w2000 errorcluster {"status"=FALSE, "code"=0, "source"=""} ("error IO")] -> w1994
          tunnel: ["" ("State(s) in Front (\"\")") "LED: BreathOff" ("State(s) in Front (\"\")")] -> w1992
          tunnel: w1988 -> [w2002 _]
          frame No Error {
            # "No error, wait for VI to stop"
            n921 = while {
              tunnel: w2002 -> [w2010]
              shift-right: [w2004] -> w2000
              shift-left: w2001 -> [w2009]
              stop <- w2006 stop-if-true
              # "continue check whether vi is running"
              n922 = property class="VI"(reference=w2010, error in=w2009) -> (error out=w2004:errorcluster, "Exec.State"=w2008:T23)  [unwired: 1 out]
              n923 = Wait (ms)(milliseconds to wait=u32 50) -> ()  [unwired: 1 out]
              n924 = Equal?(x=w2008, y=T23."Idle") -> (x = y?=w2006:bool)
            }
          }
          frame Error {
            # "try again when error"
          }
        }
        n925 = call <vilib>:"Add State(s) to Queue__JKI_lib_State_Machine.vi"("State(s) in Front (\"\")"=w1992, "State(s) in (\"\")"=w1999) -> ("States Out"=w1998:string)  [unwired: 13 in]
      }
      frame "LED: Off" {
        # "set LED to red"
        # "Template Separator\n(You can make a copy of, or modify, this frame)"
        n926 = Unbundle By Name(w2015) -> ("LJ Pinout.Red LED"=w2014:string, "LJ Pinout.Green LED"=w2013:string)
        n927 = call "LabJack_FGV.vi"("Operation(Read)"=enum16{"Write", "Read"}."Read" ("Operation"), "error in (no error)"=w2016) -> ("error out"=w2023:errorcluster, "Read data"=w2022:i32)  [unwired: 8 in]
        n928 = call "LJM_eWriteName.vi"("Handle In"=w2022, "Name"=w2014, "Value"=0.0, "error in"=w2023) -> ("Handle Out"=w2020:i32, "error out"=w2019:errorcluster)  [unwired: 10 in]
        n929 = call "LJM_eWriteName.vi"("Handle In"=w2020, "Name"=w2013, "Value"=0.0, "error in"=w2019) -> ("error out"=w2017:errorcluster)  [unwired: 10 in, 1 out]
        n930 = call <vilib>:"Add State(s) to Queue__JKI_lib_State_Machine.vi"("State(s) in (\"\")"=w2027) -> ("States Out"=w2026:string)  [unwired: 14 in]
      }
      frame "LED: Green" {
        # "set LED to green"
        # "Template Separator\n(You can make a copy of, or modify, this frame)"
        n931 = Unbundle By Name(w2031) -> ("LJ Pinout.Red LED"=w2029:string, "LJ Pinout.Green LED"=w2030:string)
        n932 = call "LabJack_FGV.vi"("Operation(Read)"=enum16{"Write", "Read"}."Read" ("Operation"), "error in (no error)"=w2033) -> ("error out"=w2039:errorcluster, "Read data"=w2038:i32)  [unwired: 8 in]
        n933 = call "LJM_eWriteName.vi"("Handle In"=w2038, "Name"=w2029, "Value"=0.0, "error in"=w2039) -> ("Handle Out"=w2036:i32, "error out"=w2035:errorcluster)  [unwired: 10 in]
        n934 = call "LJM_eWriteName.vi"("Handle In"=w2036, "Name"=w2030, "Value"=9.0, "error in"=w2035) -> ("error out"=w2032:errorcluster)  [unwired: 10 in, 1 out]
        n935 = call <vilib>:"Add State(s) to Queue__JKI_lib_State_Machine.vi"("State(s) in (\"\")"=w2042) -> ("States Out"=w2041:string)  [unwired: 14 in]
      }
      frame "---------- Queue ----------" {
        # "Template Separator\n(You can make a copy of, or modify, this frame)"
        n936 = call <vilib>:"Add State(s) to Queue__JKI_lib_State_Machine.vi"("State(s) in (\"\")"=w2047) -> ("States Out"=w2046:string)  [unwired: 14 in]
      }
      frame "Queue: Flash" {
        # "Clear queue contnet\n(clear queue content by flash it)"
        n937 = Flush Queue(queue=w2054, error in (no error)=w2048) -> (error out=w2052:errorcluster)  [unwired: 2 out]
        n938 = Flush Queue(queue=w2055, error in (no error)=w2048) -> (error out=w2051:errorcluster)  [unwired: 2 out]
        n939 = Flush Queue(queue=w2053, error in (no error)=w2048) -> (error out=w2050:errorcluster)  [unwired: 2 out]
        n940 = Merge Errors(w2052, w2051, w2050) -> (w2049:errorcluster)
        n941 = call <vilib>:"Add State(s) to Queue__JKI_lib_State_Machine.vi"("State(s) in (\"\")"=w2059) -> ("States Out"=w2058:string)  [unwired: 14 in]
      }
      frame "Queue: Destory" {
        # "Destory Data Queue\nDistory data queue ref so the aquisition loop stop"
        n942 = Release Queue(queue=w2065, error in (no error)=w2061) -> (error out=w2068:errorcluster)  [unwired: 1 in, 2 out]
        n943 = Release Queue(queue=w2064, error in (no error)=w2061) -> (error out=w2067:errorcluster)  [unwired: 1 in, 2 out]
        n944 = Release Queue(queue=w2062, error in (no error)=w2061) -> (error out=w2060:errorcluster)  [unwired: 1 in, 2 out]
        n945 = Merge Errors(w2068, w2067, w2060) -> (w2066:errorcluster)
        n946 = call <vilib>:"Simple Error Handler.vi"("error in (no error)"=w2066) -> ()  [unwired: 4 in, 5 out]
        n947 = call <vilib>:"Add State(s) to Queue__JKI_lib_State_Machine.vi"("State(s) in (\"\")"=w2071) -> ("States Out"=w2070:string)  [unwired: 14 in]
      }
      frame "---------- Run ----------" {
        # "Template Separator\n(You can make a copy of, or modify, this frame)"
        n948 = call <vilib>:"Add State(s) to Queue__JKI_lib_State_Machine.vi"("State(s) in (\"\")"=w2076) -> ("States Out"=w2075:string)  [unwired: 14 in]
      }
      frame "Run: CaliIncrement" {
        # "Increment Calibration #\n(You can make a copy of, or modify, this frame)"
        n949 = Unbundle By Name(w2078) -> ("IDs.Cali ID"=w2080:i8)
        n950 = Increment(x=w2080) -> (x+1=w2077:i8)
        n951 = Bundle By Name(cluster=w2078, "IDs.Cali ID"=w2077) -> (w2079:T26)
        n952 = call <vilib>:"Add State(s) to Queue__JKI_lib_State_Machine.vi"("State(s) in (\"\")"=w2084) -> ("States Out"=w2083:string)  [unwired: 14 in]
      }
      frame "Run: BGIncrement" {
        # "Increment BG #\n(You can make a copy of, or modify, this frame)"
        n953 = Unbundle By Name(w2085) -> ("IDs.BG ID"=w2088:i8)
        n954 = Increment(x=w2088) -> (x+1=w2087:i8)
        n955 = Bundle By Name(cluster=w2085, "IDs.BG ID"=w2087) -> (w2086:T26)
        n956 = call <vilib>:"Add State(s) to Queue__JKI_lib_State_Machine.vi"("State(s) in (\"\")"=w2092) -> ("States Out"=w2091:string)  [unwired: 14 in]
      }
      frame "Run: Increment" {
        # "Increase Run# by 1"
        n957 = Unbundle By Name(w2097) -> ("IDs.RunID"=w2099:i8)
        n958 = Increment(x=w2099) -> (x+1=w2095:i8)
        n959 = Bundle By Name(cluster=w2097, "IDs.RunID"=w2095) -> (w2098:T26)
        n960 = call "RunIDFGV.vi"("Error In"=w2093, "RunID in"=w2095) -> ("Error Out"=w2094:errorcluster)  [unwired: 8 in, 1 out]
        n961 = call <vilib>:"Add State(s) to Queue__JKI_lib_State_Machine.vi"("State(s) in (\"\")"=w2101) -> ("States Out"=w2100:string)  [unwired: 14 in]
      }
      frame "Run: Decrement" {
        # "Increase Run# by 1"
        n962 = Unbundle By Name(w2106) -> ("IDs.RunID"=w2108:i8)
        n963 = Decrement(x=w2108) -> (x-1=w2104:i8)
        n964 = Bundle By Name(cluster=w2106, "IDs.RunID"=w2104) -> (w2107:T26)
        n965 = call "RunIDFGV.vi"("Error In"=w2102, "RunID in"=w2104) -> ("Error Out"=w2103:errorcluster)  [unwired: 8 in, 1 out]
        n966 = call <vilib>:"Add State(s) to Queue__JKI_lib_State_Machine.vi"("State(s) in (\"\")"=w2110) -> ("States Out"=w2109:string)  [unwired: 14 in]
      }
      frame "---------- SysConfig ----------" {
        # "Template Separator\n(You can make a copy of, or modify, this frame)"
        n967 = call <vilib>:"Add State(s) to Queue__JKI_lib_State_Machine.vi"("State(s) in (\"\")"=w2115) -> ("States Out"=w2114:string)  [unwired: 14 in]
      }
      frame "SysConfig: LoadAPDSerialNumber" {
        # "Template Separator\n(You can make a copy of, or modify, this frame)"
        n968 = call "readAPDSerial.vi"("Error In"=w2117) -> ("Error Out"=w2116:errorcluster, "output cluster"=w2118:T29)  [unwired: 9 in]
        n969 = Bundle By Name(cluster=w2119, "APDSerialNum"=w2118) -> (w2120:T26)
        n970 = call <vilib>:"Add State(s) to Queue__JKI_lib_State_Machine.vi"("State(s) in (\"\")"=w2123) -> ("States Out"=w2122:string)  [unwired: 14 in]
      }
      frame "SysConfig: Load Sys Config" {
        # "[Covers: REQ5]"
        # "Load System config"
        # "Load system configuration\n(Load both hardware and DAQ config)"
        n971 = call "LoadSysConfig.vi"("Error In"=w2126, "Enum"=enum16{"LastUse", "Default"}."LastUse") -> ("Error Out"=w2125:errorcluster, "SysConfigCluster"=w2128:T4)  [unwired: 8 in]
        "SysConfigCluster" <- w2128
        n972 = Bundle By Name(cluster=w2129, "SysConfigCluster"=w2128) -> (w2130:T26)
        n973 = call <vilib>:"Add State(s) to Queue__JKI_lib_State_Machine.vi"("State(s) in (\"\")"=w2132) -> ("States Out"=w2131:string)  [unwired: 14 in]
      }
      frame "SysConfig: Load Digitizer Setting" {
        w2133 = enum16{"Write", "Read"}."Write" ("Operation")
        # "Load DAQ config\nSave to FGV"
        # "Template Separator\n(You can make a copy of, or modify, this frame)"
        n974 = call <userlib>:"Current VIs Parent Directory__ogtk.vi"() -> ("Parent Directory (+ Relative)"=w2147:path)  [unwired: 5 in]
        n975 = Build Path(base path=w2147, name or relative path="SubVI\\DigitizerConfiguration\\V6_Scope_last_use.config") -> (appended path=w2148:path)
        n976 = call "ReadDigitizerConfig(SubVI).vi"("error in (no error)"=w2145, "appended path"=w2148) -> ("error out"=w2141:errorcluster, "FLImDAQ"=w2139:T6)  [unwired: 8 in]
        n977 = call "FLImDAQ_FGV.vi"("error in (no error)"=w2141, "Operation (Read)"=w2133, "Write data"=w2139) -> ("error out"=w2143:errorcluster)  [unwired: 7 in, 1 out]
        n978 = Unbundle By Name(w2139) -> ("min record length"=→"data length":i32, "Digitizer 1"=w2135:refnum<k15>, "Digitizer 2"=w2142:refnum<k15>)
        n979 = Bundle By Name(cluster=w2137, "FLImDAQ"=w2139) -> (w2138:T26)
        n980 = call "Digitizer1_FGV.vi"("error in (no error)"=w2143, "Operation (Read)"=w2133, "Write data"=w2135) -> ("error out"=w2144:errorcluster)  [unwired: 7 in, 1 out]
        n981 = call "Digitizer2_FGV.vi"("error in (no error)"=w2144, "Operation (Read)"=w2133, "Write data"=w2142) -> ("error out"=w2140:errorcluster)  [unwired: 7 in, 1 out]
        n982 = call <vilib>:"Add State(s) to Queue__JKI_lib_State_Machine.vi"("State(s) in (\"\")"=w2150) -> ("States Out"=w2149:string)  [unwired: 14 in]
      }
      frame "SysConfig: Load LJ Pinout" {
        # "Template Separator\n(You can make a copy of, or modify, this frame)"
        n983 = call <userlib>:"Current VIs Parent Directory__ogtk.vi"() -> ("Parent Directory (+ Relative)"=w2165:path)  [unwired: 5 in]
        n984 = Build Path(base path=w2165, name or relative path="SubVI\\LabJack\\LJ_pin_setting.config") -> (appended path=w2163:path)
        n985 = call "ReadLabjackConfig(SubVI).vi"("error in (no error)"=w2161, "appended path"=w2163) -> ("error out"=w2162:errorcluster, "Utility"=w2159:T5)  [unwired: 8 in]
        n986 = Unbundle By Name(w2159) -> ("Ch1 Bias"=w2158:string, "Ch2 Bias"=w2157:string, "Ch3 Bias"=w2156:string, "Ch4 Bias"=w2151:string, "Red LED"=w2153:string, "Green LED"=w2152:string)
        n987 = global write "GlobalVariables.vi" "LED Green pin"(w2152) -> ()
        n988 = global write "GlobalVariables.vi" "Ch1 LJ pin"(w2158) -> ()
        n989 = global write "GlobalVariables.vi" "Ch2 LJ pin"(w2157) -> ()
        n990 = global write "GlobalVariables.vi" "Ch3 LJ pin"(w2156) -> ()
        n991 = global write "GlobalVariables.vi" "Ch4 LJ pin"(w2151) -> ()
        n992 = global write "GlobalVariables.vi" "LED Red pin"(w2153) -> ()
        n993 = Bundle By Name(cluster=w2154, "LJ Pinout"=w2159) -> (w2160:T26)
        n994 = call <vilib>:"Add State(s) to Queue__JKI_lib_State_Machine.vi"("State(s) in (\"\")"=w2167) -> ("States Out"=w2166:string)  [unwired: 14 in]
      }
      frame "SysConfig: Load 355 PWM" {
        # "Template Separator\n(You can make a copy of, or modify, this frame)"
        n995 = call <userlib>:"Current VIs Parent Directory__ogtk.vi"() -> ("Parent Directory (+ Relative)"=w2185:path)  [unwired: 5 in]
        n996 = Build Path(base path=w2185, name or relative path="SubVI\\LabJack\\PWM_setting_355.config") -> (appended path=w2183:path)
        n997 = call "ReadPWMConfig(SubVI).vi"("error in (no error)"=w2180, "appended path"=w2183) -> ("error out"=w2181:errorcluster, "PWM Setting"=w2179:T43)  [unwired: 8 in]
        n998 = Unbundle By Name(w2179) -> ("DIO_EF_CLOCK1_DIVISOR"=w2176:i16, "DIO_EF_CLOCK1_ROLL_VALUE"=w2175:i32)
        n999 = Multiply(x=w2176, y=w2175) -> (x*y=w2177:i32)
        n1000 = Bundle By Name(cluster=w2182, "355 PWM setting"=w2179) -> (w2169:T26)
        n1001 = Divide(x=80000000.0, y=w2177) -> (x/y=w2174:dbl)
        "Laser Rep Rate" <- w2174
        n1002 = Number To Decimal String(number=w2174) -> (decimal integer string=w2173:string)  [unwired: 1 in]
        n1003 = Concatenate Strings("355nm " ("string"), w2173, "Hz" ("string")) -> (w2171:string)
        n1004 = property on="355nm Laser toggle" class="Bool (strict)"("Caption.Text"=w2171) -> ()  [unwired: 2 in, 2 out]
        n1005 = call <vilib>:"Add State(s) to Queue__JKI_lib_State_Machine.vi"("State(s) in (\"\")"=w2187) -> ("States Out"=w2186:string)  [unwired: 14 in]
      }
      frame "SysConfig: Load AB PWM" {
        # "Template Separator\n(You can make a copy of, or modify, this frame)"
        n1006 = call <userlib>:"Current VIs Parent Directory__ogtk.vi"() -> ("Parent Directory (+ Relative)"=w2196:path)  [unwired: 5 in]
        n1007 = Build Path(base path=w2196, name or relative path="SubVI\\LabJack\\PWM_setting_AB.config") -> (appended path=w2194:path)
        n1008 = call "ReadPWMConfig(SubVI).vi"("error in (no error)"=w2191, "appended path"=w2194) -> ("error out"=w2192:errorcluster, "PWM Setting"=w2190:T43)  [unwired: 8 in]
        n1009 = Bundle By Name(cluster=w2188, "AB PWM setting"=w2190) -> (w2193:T26)
        n1010 = call <vilib>:"Add State(s) to Queue__JKI_lib_State_Machine.vi"("State(s) in (\"\")"=w2198) -> ("States Out"=w2197:string)  [unwired: 14 in]
      }
      frame "SysConfig: Load AB setting" {
        # "load aming beam setting\n(check frequency, if 0 do nothing, if not zero, config PWM)"
        n1011 = call "readAimingBeamSetting.vi"("error in (no error)"=w2216) -> ("error out"=w2211:errorcluster, "Aiming Beam Setting"=w2203:T44)  [unwired: 9 in]
        n1012 = Unbundle By Name(w2203) -> ("Default Current"=w2202:dbl)
        n1013 = Unbundle By Name(w2203) -> ("Frequency(Hz)"=w2199:u32)
        n1014 = Equal To 0?(x=w2199) -> (x = 0?=w2209:bool)
        n1015 = Select(t="", s=w2209, f="SysConfig: Load AB PWM" ("State(s) in Front (\"\")")) -> (s? t:f=w2212:string)
        n1016 = Number To Decimal String(number=w2199) -> (decimal integer string=w2208:string)  [unwired: 1 in]
        n1017 = Number To Decimal String(number=w2202, width (-)=i16 2) -> (decimal integer string=w2201:string)
        n1018 = Concatenate Strings("445nm " ("string"), w2208, "Hz " ("string"), w2201, "mA" ("string")) -> (w2207:string)
        n1019 = property on="Aiming beam toggle" class="Bool (strict)"("Caption.Text"=w2207) -> ()  [unwired: 2 in, 2 out]
        n1020 = case shown="False" w2209 {
          tunnel: w2211 -> [w2224 w2227]
          tunnel: [w2223 w2227] -> w2210
          tunnel: w2199 -> [w2222 _]
          frame False {
            n1021 = call "LJ_calculate_PWM_parameters.vi"("Duty Cycle (%)"=u32 10, "Error In"=w2224, "Show Confirmation"=FALSE, "Laser Rep Rate (Hz)"=w2222, "Laser"=enum16{"355nm", "AimingBeam"}."AimingBeam") -> ("Error Out"=w2223:errorcluster)  [unwired: 5 in, 1 out]
          }
          frame True {
          }
        }
        n1022 = Bundle By Name(cluster=w2217, "AB Cluster"=w2203) -> (w2218:T26)
        n1023 = call <vilib>:"Add State(s) to Queue__JKI_lib_State_Machine.vi"("State(s) in Front (\"\")"=w2212, "State(s) in (\"\")"=w2220) -> ("States Out"=w2219:string)  [unwired: 13 in]
      }
      frame "SysConfig: LoadABVideoSetting" {
        # "Load AB video setting form ini file\n()"
        n1024 = call "readVideoConfig.vi"("error in (no error)"=w2231) -> ("error out"=w2232:errorcluster, "Aiming Beam Config"=w2230:T25)  [unwired: 8 in, 1 out]
        n1025 = Bundle By Name(cluster=w2228, "VideoConfig"=w2230) -> (w2229:T26)
        n1026 = call <vilib>:"Add State(s) to Queue__JKI_lib_State_Machine.vi"("State(s) in (\"\")"=w2235) -> ("States Out"=w2234:string)  [unwired: 14 in]
      }
      frame "SysConfig: LoadCursorLocation" {
        # "Load cursor location from ini file\n(load cursor from system setting ini file)"
        n1027 = call "readCursorConfigMain.vi"("error in (no error)"=w2247) -> ("error out"=w2248:errorcluster, "Cursor Locations"=w2246:T45)  [unwired: 9 in]
        n1028 = Unbundle By Name(w2246) -> ("DC1"=w2245:i32, "DC2"=w2244:i32, "BG1"=w2239:i32, "BG2"=w2238:i32)
        n1029 = Build Array(w2245, w2244) -> (w2243:i32[])
        n1030 = Build Array(w2239, w2238) -> (w2240:i32[])
        n1031 = Array Max & Min(array=w2243) -> (max value=w2242:i32, min value=w2241:i32)  [unwired: 2 out]
        n1032 = Array Max & Min(array=w2240) -> (max value=w2237:i32, min value=w2236:i32)  [unwired: 2 out]
        n1033 = global write "GlobalVariables.vi" "DC Idx2"(w2242) -> ()
        n1034 = global write "GlobalVariables.vi" "DC Idx1"(w2241) -> ()
        n1035 = global write "GlobalVariables.vi" "BG Idx2"(w2237) -> ()
        n1036 = global write "GlobalVariables.vi" "BG Idx1"(w2236) -> ()
        n1037 = call <vilib>:"Add State(s) to Queue__JKI_lib_State_Machine.vi"("State(s) in (\"\")"=w2252) -> ("States Out"=w2251:string)  [unwired: 14 in]
      }
      frame "---------- SystemStatus ----------" {
        # "Template Separator\n(You can make a copy of, or modify, this frame)"
        n1038 = call <vilib>:"Add State(s) to Queue__JKI_lib_State_Machine.vi"("State(s) in (\"\")"=w2257) -> ("States Out"=w2256:string)  [unwired: 14 in]
      }
      frame "SystemStatus: SlowSysStatusMacro" {
        # "store system check time"
        # "Template Separator\n(You can make a copy of, or modify, this frame)"
        n1039 = Tick Count (ms)() -> (millisecond timer value=w2260:u32)
        n1040 = Bundle By Name(cluster=w2258, "SlowTimer"=w2260) -> (w2259:T26)
        n1041 = call <vilib>:"Add State(s) to Queue__JKI_lib_State_Machine.vi"("State(s) in Front (\"\")"="Digitizer: checkTemp\nTCP: CheckConnection" ("State(s) in Front (\"\")"), "State(s) in (\"\")"=w2265) -> ("States Out"=w2264:string)  [unwired: 13 in]
      }
      frame "SystemStatus: FastSysStatusMacro" {
        # "store system check time"
        # "Template Separator\n(You can make a copy of, or modify, this frame)"
        n1042 = Tick Count (ms)() -> (millisecond timer value=w2268:u32)
        n1043 = Bundle By Name(cluster=w2266, "FastTimer"=w2268) -> (w2267:T26)
        n1044 = call <vilib>:"Add State(s) to Queue__JKI_lib_State_Machine.vi"("State(s) in Front (\"\")"="355 Laser: CheckPWMStatus\nAimingBeam: GetPWMStatus\n/*355 Laser: CheckControllerStatus" ("State(s) in Front (\"\")"), "State(s) in (\"\")"=w2273) -> ("States Out"=w2272:string)  [unwired: 13 in]
      }
      frame "---------- UI ----------" {
        # "Do not put any code in this frame.\n(It is a separator no-op. You can make a copy of this frame to create a new UI frame)"
        n1045 = call <vilib>:"Add State(s) to Queue__JKI_lib_State_Machine.vi"("State(s) in (\"\")"=w2278) -> ("States Out"=w2277:string)  [unwired: 14 in]
      }
      frame "UI: Initialize" {
        w2280 = T46 {"Minimum"=0.0, "Maximum"=4.6, "Increment"=0.1} ("Data Entry Limits")
        w2279 = T11."Disabled and Grayed Out" ("Disabled")
        # "Disable all button on startup"
        # "Initialize the User Interface, here.\n(this is called automatically, by the Macro: Init)"
        n1046 = property on="V 1" class="DigNum (strict)"("DisabledEnum"=w2279) -> ()  [unwired: 2 in, 2 out]
        n1047 = property on="V 2" class="DigNum (strict)"("DisabledEnum"=w2279) -> ()  [unwired: 2 in, 2 out]
        n1048 = property on="StopButton" class="Bool (strict)"("DisabledEnum"=w2279) -> ()  [unwired: 2 in, 2 out]
        n1049 = property on="Sys Reconfig" class="Bool"("DisabledEnum"=w2279) -> ()  [unwired: 2 in, 2 out]
        n1050 = property on="StartButton" class="Bool (strict)"("DisabledEnum"=w2279) -> ()  [unwired: 2 in, 2 out]
        n1051 = property on="355nm Laser toggle" class="Bool (strict)"("DisabledEnum"=w2279) -> ()  [unwired: 2 in, 2 out]
        n1052 = property on="Aiming beam toggle" class="Bool (strict)"("DisabledEnum"=w2279) -> ()  [unwired: 2 in, 2 out]
        n1053 = property on="Background" class="Bool (strict)"("DisabledEnum"=w2279) -> ()  [unwired: 2 in, 2 out]
        n1054 = property on="Cali&iRF alignment" class="Bool (strict)"("DisabledEnum"=w2279) -> ()  [unwired: 2 in, 2 out]
        n1055 = property on="V 3" class="DigNum (strict)"("DisabledEnum"=w2279) -> ()  [unwired: 2 in, 2 out]
        n1056 = property on="Video Source" class="RadioBtnsControl (strict)"("DisabledEnum"=w2279) -> ()  [unwired: 2 in, 2 out]
        n1057 = property on="V 1" class="DigNum (strict)"("Data Range"=w2280) -> ()  [unwired: 2 in, 2 out]
        n1058 = property on="V 2" class="DigNum (strict)"("Data Range"=w2280) -> ()  [unwired: 2 in, 2 out]
        n1059 = property on="V 3" class="DigNum (strict)"("Data Range"=w2280) -> ()  [unwired: 2 in, 2 out]
        n1060 = call <vilib>:"Add State(s) to Queue__JKI_lib_State_Machine.vi"("State(s) in Front (\"\")"="UI: CaliAndiRFNotReady" ("State(s) in Front (\"\")"), "State(s) in (\"\")"=w2286) -> ("States Out"=w2285:string)  [unwired: 13 in]
      }
      frame "UI: BGLoaded" {
        # "[Covers: REQ24]"
        # "Do not put any code in this frame.\n(It is a separator no-op. You can make a copy of this frame to create a new UI frame)"
        n1061 = property on="Background" class="Bool (strict)"("BoolText.Text"="Loaded!" ("Boolean Text.Text"), "Colors [4]"=cluster{u32, u32}[] [{15764023, 15764023}, {16711680, 16711680}]) -> ()  [unwired: 2 in, 2 out]
        n1062 = call <vilib>:"Add State(s) to Queue__JKI_lib_State_Machine.vi"("State(s) in (\"\")"=w2293) -> ("States Out"=w2292:string)  [unwired: 14 in]
      }
      frame "UI: BGSizeError" {
        # "[Covers: REQ24]"
        # "Do not put any code in this frame.\n(It is a separator no-op. You can make a copy of this frame to create a new UI frame)"
        n1063 = property on="Background" class="Bool (strict)"("BoolText.Text"="Loaded!" ("Boolean Text.Text"), "Colors [4]"=cluster{u32, u32}[] [{7171459, 7171459}, {16711680, 16711680}]) -> ()  [unwired: 2 in, 2 out]
        n1064 = One Button Dialog(message="Background waveform length and current digitizer setting mismatch! Please take a new background before any aquisition!") -> ()  [unwired: 1 in, 1 out]
        n1065 = call <vilib>:"Add State(s) to Queue__JKI_lib_State_Machine.vi"("State(s) in (\"\")"=w2301) -> ("States Out"=w2300:string)  [unwired: 14 in]
      }
      frame "UI: CaliAndiRFLoaded" {
        # "[Covers: REQ24]"
        # "Do not put any code in this frame.\n(It is a separator no-op. You can make a copy of this frame to create a new UI frame)"
        n1066 = property on="Cali&iRF alignment" class="Bool (strict)"("BoolText.Text"="Loaded!" ("Boolean Text.Text"), "Colors [4]"=cluster{u32, u32}[] [{15764023, 15764023}, {16711680, 16711680}]) -> ()  [unwired: 2 in, 2 out]
        n1067 = call <vilib>:"Add State(s) to Queue__JKI_lib_State_Machine.vi"("State(s) in (\"\")"=w2308) -> ("States Out"=w2307:string)  [unwired: 14 in]
      }
      frame "UI: WFAutoScale" {
        # "Set graph auto scale.\n(UI: WFAutoScale >> T/F)"
        n1068 = Equal?(x=w2309, y="F") -> (x = y?=w2310:bool)
        n1069 = Equal?(x=w2309, y="T") -> (x = y?=w2312:bool)
        n1070 = case shown="True" w2312 {
          frame False {
          }
          frame True {
            w2328 = u8 2 ("Y Scale.Scale Fit")
            n1071 = property on="Channel 1" class="WFGraph (strict)"("YScale.ScaleFit"=w2328) -> ()  [unwired: 2 in, 2 out]
            n1072 = property on="Channel 2" class="WFGraph (strict)"("YScale.ScaleFit"=w2328) -> ()  [unwired: 2 in, 2 out]
            n1073 = property on="Channel 3" class="WFGraph (strict)"("YScale.ScaleFit"=w2328) -> ()  [unwired: 2 in, 2 out]
          }
        }
        n1074 = case shown="True" w2310 {
          frame False {
          }
          frame True {
            w2325 = 0.0 ("Y Scale.Range:Maximum")
            w2326 = 2.0 ("Y Scale.Range:Maximum")
            w2327 = u8 0 ("Y Scale.Scale Fit")
            n1075 = property on="Channel 1" class="WFGraph (strict)"("YScale.ScaleFit"=w2327) -> (error out=w2324:errorcluster)  [unwired: 2 in, 1 out]
            n1076 = property on="Channel 2" class="WFGraph (strict)"("YScale.ScaleFit"=w2327) -> (error out=w2323:errorcluster)  [unwired: 2 in, 1 out]
            n1077 = property on="Channel 3" class="WFGraph (strict)"("YScale.ScaleFit"=w2327) -> (error out=w2322:errorcluster)  [unwired: 2 in, 1 out]
            n1078 = property on="Channel 1" class="WFGraph (strict)"(error in=w2324, "YScale.Maximum"=w2326) -> (error out=w2321:errorcluster)  [unwired: 1 in, 1 out]
            n1079 = property on="Channel 2" class="WFGraph (strict)"(error in=w2323, "YScale.Maximum"=w2326) -> (error out=w2320:errorcluster)  [unwired: 1 in, 1 out]
            n1080 = property on="Channel 3" class="WFGraph (strict)"(error in=w2322, "YScale.Maximum"=w2326) -> (error out=w2319:errorcluster)  [unwired: 1 in, 1 out]
            n1081 = property on="Channel 1" class="WFGraph (strict)"(error in=w2321, "YScale.Minimum"=w2325) -> ()  [unwired: 1 in, 2 out]
            n1082 = property on="Channel 2" class="WFGraph (strict)"(error in=w2320, "YScale.Minimum"=w2325) -> ()  [unwired: 1 in, 2 out]
            n1083 = property on="Channel 3" class="WFGraph (strict)"(error in=w2319, "YScale.Minimum"=w2325) -> ()  [unwired: 1 in, 2 out]
          }
        }
        n1084 = call <vilib>:"Add State(s) to Queue__JKI_lib_State_Machine.vi"("State(s) in (\"\")"=w2318) -> ("States Out"=w2317:string)  [unwired: 14 in]
      }
      frame "UI: showDisclaimer" {
        # "Show disclamer window.\n(It is a separator no-op. You can make a copy of this frame to create a new UI frame)"
        n1085 = call <vilib>:"Application Directory.vi"() -> ("Application Directory"=w2341:path)
        n1086 = Build Path(base path=w2341, name or relative path="Disclamer.png") -> (appended path=w2339:path)
        n1087 = property on="Disclamer" class="Pict"() -> ("Draw Area Size"=w2337:T47)  [unwired: 2 in, 2 out]
        n1088 = disable-structure "Diagram Disable Structure" shown="Disabled" {
          frame Disabled {
            n1089 = flat-sequence {
              frame #0 {
                n1090 = call "disclaimer.vi"() -> ()  [unwired: 12 in]
              }
              frame #1 {
                n1091 = Wait (ms)(milliseconds to wait=u32 250) -> ()  [unwired: 1 out]
              }
              frame #2 {
                n1092 = call "SoftwareNote.vi"() -> ()  [unwired: 12 in]
              }
            }
          }
          frame Enabled {
          }
        }
        n1093 = call <vilib>:"Read PNG File.vi"("path to PNG file"=w2339) -> ("image data"=w2336:T48)  [unwired: 8 in, 2 out]
        n1094 = Unbundle By Name(w2336) -> ("Rectangle.right"=w2334:i16, "Rectangle.bottom"=w2332:i16)
        n1095 = Unbundle By Name(w2337) -> ("Width"=w2335:u32, "Height"=w2333:u32)
        n1096 = call <vilib>:"Draw Flattened Pixmap.vi"("image data"=w2336) -> ("new picture"=→"Disclamer":picture)  [unwired: 8 in]
        n1097 = Divide(x=w2335, y=w2334) -> (x/y=w2331:dbl)
        n1098 = Divide(x=w2333, y=w2332) -> (x/y=w2330:dbl)
        n1099 = Max & Min(x=w2331, y=w2330) -> (min(x,y)=w2329:dbl)  [unwired: 1 out]
        n1100 = property on="Disclamer" class="Pict"("ZoomFactor"=w2329) -> ()  [unwired: 2 in, 2 out]
        n1101 = call <vilib>:"Add State(s) to Queue__JKI_lib_State_Machine.vi"("State(s) in (\"\")"=w2346) -> ("States Out"=w2345:string)  [unwired: 14 in]
      }
      frame "UI: CaliAndiRFNotReady" {
        # "Do not put any code in this frame.\n(It is a separator no-op. You can make a copy of this frame to create a new UI frame)"
        n1102 = property on="Cali&iRF alignment" class="Bool (strict)"("BoolText.Text"="No Info" ("Boolean Text.Text"), "Colors [4]"=cluster{u32, u32}[] [{13816530, 13816530}, {16711680, 16711680}]) -> ()  [unwired: 2 in, 2 out]
        n1103 = call <vilib>:"Add State(s) to Queue__JKI_lib_State_Machine.vi"("State(s) in (\"\")"=w2354) -> ("States Out"=w2353:string)  [unwired: 14 in]
      }
      frame "UI: BGnotReady" {
        # "Do not put any code in this frame.\n(It is a separator no-op. You can make a copy of this frame to create a new UI frame)"
        n1104 = property on="Background" class="Bool (strict)"("BoolText.Text"="No Info" ("Boolean Text.Text"), "Colors [4]"=cluster{u32, u32}[] [{13816530, 13816530}, {16711680, 16711680}]) -> ()  [unwired: 2 in, 2 out]
        n1105 = call <vilib>:"Add State(s) to Queue__JKI_lib_State_Machine.vi"("State(s) in (\"\")"=w2361) -> ("States Out"=w2360:string)  [unwired: 14 in]
      }
      frame "UI: Reset" {
        w2363 = cluster{u32, u32}[] [{13816530, 13816530}, {13816530, 13816530}] ("Colors [4]")
        # "Do not put any code in this frame.\n(It is a separator no-op. You can make a copy of this frame to create a new UI frame)"
        n1106 = property on="Cali&iRF alignment" class="Bool (strict)"("BoolText.Text"="No Info" ("Boolean Text.Text"), "Colors [4]"=w2363) -> ()  [unwired: 2 in, 2 out]
        n1107 = property on="Background" class="Bool (strict)"("BoolText.Text"="No Info" ("Boolean Text.Text"), "Colors [4]"=w2363) -> ()  [unwired: 2 in, 2 out]
        n1108 = call <vilib>:"Add State(s) to Queue__JKI_lib_State_Machine.vi"("State(s) in (\"\")"=w2369) -> ("States Out"=w2368:string)  [unwired: 14 in]
      }
      frame "UI: SetButtonText" {
        # "Set button text of 355nm laser and aiming beam."
        n1109 = call <vilib>:"Add State(s) to Queue__JKI_lib_State_Machine.vi"("State(s) in (\"\")"=w2374) -> ("States Out"=w2373:string)  [unwired: 14 in]
      }
      frame "UI: DuringAquisition" {
        w2377 = T11."Disabled and Grayed Out" ("Disabled")
        # "Do not put any code in this frame.\n(It is a separator no-op. You can make a copy of this frame to create a new UI frame)"
        n1110 = Unbundle By Name(w2376) -> ("bothVidSourceAvail"=w2375:bool)
        n1111 = case shown="True" w2375 {
          tunnel: w2377 -> [_ w2383]
          frame False {
          }
          frame True {
            n1112 = property on="Video Source" class="RadioBtnsControl (strict)"("DisabledEnum"=w2383) -> ()  [unwired: 2 in, 2 out]
          }
        }
        n1113 = property on="StartButton" class="Bool (strict)"("DisabledEnum"=w2377) -> ()  [unwired: 2 in, 2 out]
        n1114 = property on="Sys Reconfig" class="Bool"("DisabledEnum"=w2377) -> ()  [unwired: 2 in, 2 out]
        n1115 = property on="355nm Laser toggle" class="Bool (strict)"("DisabledEnum"=w2377) -> ()  [unwired: 2 in, 2 out]
        n1116 = property on="Aiming beam toggle" class="Bool (strict)"("DisabledEnum"=w2377) -> ()  [unwired: 2 in, 2 out]
        n1117 = property on="Background" class="Bool (strict)"("DisabledEnum"=w2377) -> ()  [unwired: 2 in, 2 out]
        n1118 = property on="Radio Buttons" class="RadioBtnsControl (strict)"("DisabledEnum"=w2377) -> ()  [unwired: 2 in, 2 out]
        n1119 = property on="Cali&iRF alignment" class="Bool (strict)"("DisabledEnum"=w2377) -> ()  [unwired: 2 in, 2 out]
        n1120 = property on="Quit" class="Bool"("DisabledEnum"=w2377) -> ()  [unwired: 2 in, 2 out]
        n1121 = property on="Skip Data Save?" class="Bool (strict)"("DisabledEnum"=w2377) -> ()  [unwired: 2 in, 2 out]
        n1122 = property on="Video Display" class="Bool (strict)"("DisabledEnum"=w2377) -> ()  [unwired: 2 in, 2 out]
        n1123 = property on="StopButton" class="Bool (strict)"("DisabledEnum"=T11."Enabled" ("Disabled")) -> ()  [unwired: 2 in, 2 out]
        n1124 = call <vilib>:"Add State(s) to Queue__JKI_lib_State_Machine.vi"("State(s) in (\"\")"=w2382) -> ("States Out"=w2381:string)  [unwired: 14 in]
      }
      frame "UI: duringIRFAlign" {
        w2384 = T11."Disabled and Grayed Out" ("Disabled")
        # "Set UI to during iRF alignment\n(It is a separator no-op. You can make a copy of this frame to create a new UI frame)"
        n1125 = property on="StartButton" class="Bool (strict)"("DisabledEnum"=w2384) -> ()  [unwired: 2 in, 2 out]
        n1126 = property on="Sys Reconfig" class="Bool"("DisabledEnum"=w2384) -> ()  [unwired: 2 in, 2 out]
        n1127 = property on="355nm Laser toggle" class="Bool (strict)"("DisabledEnum"=w2384) -> ()  [unwired: 2 in, 2 out]
        n1128 = property on="Aiming beam toggle" class="Bool (strict)"("DisabledEnum"=w2384) -> ()  [unwired: 2 in, 2 out]
        n1129 = property on="Background" class="Bool (strict)"("DisabledEnum"=w2384) -> ()  [unwired: 2 in, 2 out]
        n1130 = property on="StopButton" class="Bool (strict)"("DisabledEnum"=w2384) -> ()  [unwired: 2 in, 2 out]
        n1131 = call <vilib>:"Add State(s) to Queue__JKI_lib_State_Machine.vi"("State(s) in (\"\")"=w2389) -> ("States Out"=w2388:string)  [unwired: 14 in]
      }
      frame "UI: duringBGAcquire" {
        w2390 = T11."Disabled and Grayed Out" ("Disabled")
        # "Do not put any code in this frame.\n(It is a separator no-op. You can make a copy of this frame to create a new UI frame)"
        n1132 = property on="StartButton" class="Bool (strict)"("DisabledEnum"=w2390) -> ()  [unwired: 2 in, 2 out]
        n1133 = property on="StopButton" class="Bool (strict)"("DisabledEnum"=w2390) -> ()  [unwired: 2 in, 2 out]
        n1134 = property on="Sys Reconfig" class="Bool"("DisabledEnum"=w2390) -> ()  [unwired: 2 in, 2 out]
        n1135 = property on="355nm Laser toggle" class="Bool (strict)"("DisabledEnum"=w2390) -> ()  [unwired: 2 in, 2 out]
        n1136 = property on="Aiming beam toggle" class="Bool (strict)"("DisabledEnum"=w2390) -> ()  [unwired: 2 in, 2 out]
        n1137 = property on="Cali&iRF alignment" class="Bool (strict)"("DisabledEnum"=w2390) -> ()  [unwired: 2 in, 2 out]
        n1138 = call <vilib>:"Add State(s) to Queue__JKI_lib_State_Machine.vi"("State(s) in (\"\")"=w2395) -> ("States Out"=w2394:string)  [unwired: 14 in]
      }
      frame "UI: ReadyForAquisition" {
        w2399 = T11."Enabled" ("Disabled")
        # "Do not put any code in this frame.\n(It is a separator no-op. You can make a copy of this frame to create a new UI frame)"
        n1139 = Unbundle By Name(w2398) -> ("System Status.TCP/IP"=w2397:bool, "bothVidSourceAvail"=w2396:bool)
        n1140 = property on="StartButton" class="Bool (strict)"("DisabledEnum"=w2399) -> ()  [unwired: 2 in, 2 out]
        n1141 = property on="Sys Reconfig" class="Bool"("DisabledEnum"=w2399) -> ()  [unwired: 2 in, 2 out]
        n1142 = property on="355nm Laser toggle" class="Bool (strict)"("DisabledEnum"=w2399) -> ()  [unwired: 2 in, 2 out]
        n1143 = property on="Aiming beam toggle" class="Bool (strict)"("DisabledEnum"=w2399) -> ()  [unwired: 2 in, 2 out]
        n1144 = property on="Cali&iRF alignment" class="Bool (strict)"("DisabledEnum"=w2399) -> ()  [unwired: 2 in, 2 out]
        n1145 = property on="Background" class="Bool (strict)"("DisabledEnum"=w2399) -> ()  [unwired: 2 in, 2 out]
        n1146 = property on="Quit" class="Bool"("DisabledEnum"=w2399) -> ()  [unwired: 2 in, 2 out]
        n1147 = property on="Radio Buttons" class="RadioBtnsControl (strict)"("DisabledEnum"=w2399) -> ()  [unwired: 2 in, 2 out]
        n1148 = case shown="True" w2396 {
          tunnel: w2399 -> [_ w2405]
          frame False {
          }
          frame True {
            n1149 = property on="Video Source" class="RadioBtnsControl (strict)"("DisabledEnum"=w2405) -> ()  [unwired: 2 in, 2 out]
          }
        }
        n1150 = property on="Skip Data Save?" class="Bool (strict)"("DisabledEnum"=w2399) -> ()  [unwired: 2 in, 2 out]
        n1151 = case shown="True" w2397 {
          tunnel: w2399 -> [_ w2406]
          frame False {
          }
          frame True {
            n1152 = property on="Video Display" class="Bool (strict)"("DisabledEnum"=w2406) -> ()  [unwired: 2 in, 2 out]
          }
        }
        n1153 = property on="StopButton" class="Bool (strict)"("DisabledEnum"=T11."Disabled and Grayed Out" ("Disabled")) -> ()  [unwired: 2 in, 2 out]
        n1154 = call <vilib>:"Add State(s) to Queue__JKI_lib_State_Machine.vi"("State(s) in (\"\")"=w2404) -> ("States Out"=w2403:string)  [unwired: 14 in]
      }
      frame "UI: Update" {
        # "Do not put any code in this frame.\n(It is a separator no-op. You can make a copy of this frame to create a new UI frame)"
        n1155 = Unbundle By Name(w2417) -> ("System Status"=→"System Hardware Connection Status":T2, "IDs.RunID"=→"Run #":i8, "CaseID"=→"Case #":string, "FLImDAQ"=→"FLImDAQ":T33, "SysRunning?"=→"Aquisition Status:":bool, "LJ Pinout"=→"LJ Pinout":T5, "IDs.BG ID"=→"BG #":i8, "IDs.Cali ID"=→"Calibration #":i8, "video source"=→"Visualization PC video source":T1)
        n1156 = call <vilib>:"Add State(s) to Queue__JKI_lib_State_Machine.vi"("State(s) in (\"\")"=w2420) -> ("States Out"=w2419:string)  [unwired: 14 in]
      }
      frame "UI: updateVideoToggle" {
        # "Set video toggle based on visualization PC video source.\n(take )"
        n1157 = call <vilib>:"Add State(s) to Queue__JKI_lib_State_Machine.vi"("State(s) in (\"\")"=w2425) -> ("States Out"=w2424:string)  [unwired: 14 in]
      }
      frame "UI: Cursor Set" {
        # "Argument"
        # "Set and Unset Cursor Busy.\n(Usage: \"UI: Cursor Set >> Busy|Idle\")"
        n1158 = case shown="\"Idle\", Default" w2427 {
          tunnel: w2429 -> [w2434 w2436]
          tunnel: [w2433 w2435] -> w2428
          frame "Idle", Default {
            n1159 = call <vilib>:"Unset Busy.vi"("error in (no error)"=w2434) -> ("error out"=w2433:errorcluster)  [unwired: 10 in]
          }
          frame "Busy" {
            n1160 = call <vilib>:"Set Busy.vi"("error in (no error)"=w2436) -> ("error out"=w2435:errorcluster)  [unwired: 9 in, 1 out]
          }
        }
        n1161 = call <vilib>:"Add State(s) to Queue__JKI_lib_State_Machine.vi"("State(s) in (\"\")"=w2432) -> ("States Out"=w2431:string)  [unwired: 14 in]
      }
      frame "UI: Front Panel State" {
        # "Argument"
        # "Set Front Panel Open or Closed\n(Usage: \"UI: Front Panel State >> Open|Close\")"
        n1162 = Unbundle By Name(w2440) -> ("Core.Current VI Reference"=w2439:refnum<vi>)
        n1163 = case shown="\"Open\", \"Standard\", Default" w2438 {
          tunnel: w2442 -> [w2450 w2465 w2476 w2489 w2502]
          tunnel: [w2452 w2466 w2478 w2491 w2504] -> w2441
          tunnel: w2439 -> [w2451 w2463 w2477 w2490 w2503]
          frame "Open", "Standard", Default {
            w2445 = T21."Standard" ("State")
            n1164 = property on="Property Node" class="VI"(reference=w2451, error in=w2450) -> (reference out=w2448:refnum<vi>, error out=w2449:errorcluster, "FP.State"=w2447:T21)
            n1165 = Not Equal?(x=w2447, y=w2445) -> (x != y?=w2446:bool)
            n1166 = case shown="True" w2446 {
              tunnel: [w2456 w2458] -> w2452
              tunnel: w2449 -> [w2455 w2458]
              tunnel: w2448 -> [w2454 _]
              tunnel: w2445 -> [w2453 _]
              frame True {
                n1167 = invoke on="Invoke Node" class="VI" method="FP.Open"(reference=w2454, error in=w2455, "Activate"=TRUE, "State"=w2453) -> (error out=w2456:errorcluster)  [unwired: 1 in, 4 out]
              }
              frame False {
              }
            }
          }
          frame "Close", "Closed" {
            n1168 = property on="Property Node" class="VI"(reference=w2463, error in=w2465) -> (reference out=w2462:refnum<vi>, error out=w2464:errorcluster, "FP.State"=w2460:T21)
            n1169 = Not Equal?(x=w2460, y=T21."Closed" ("Front Panel Window:State")) -> (x != y?=w2459:bool)
            n1170 = case shown="True" w2459 {
              tunnel: [w2467 w2470] -> w2466
              tunnel: w2464 -> [w2467 w2469]
              tunnel: w2462 -> [_ w2468]
              frame False {
              }
              frame True {
                n1171 = invoke on="Invoke Node" class="VI" method="FP.Close"(reference=w2468, error in=w2469) -> (error out=w2470:errorcluster)  [unwired: 1 in, 2 out]
              }
            }
          }
          frame "Hidden", "Hide" {
            w2471 = T21."Hidden" ("State")
            n1172 = property on="Property Node" class="VI"(reference=w2477, error in=w2476) -> (reference out=w2474:refnum<vi>, error out=w2475:errorcluster, "FP.State"=w2473:T21)
            n1173 = Not Equal?(x=w2473, y=w2471) -> (x != y?=w2472:bool)
            n1174 = case shown="True" w2472 {
              tunnel: [w2482 w2483] -> w2478
              tunnel: w2475 -> [w2481 w2483]
              tunnel: w2474 -> [w2480 _]
              tunnel: w2471 -> [w2479 _]
              frame True {
                n1175 = invoke on="Invoke Node" class="VI" method="FP.Open"(reference=w2480, error in=w2481, "State"=w2479) -> (error out=w2482:errorcluster)  [unwired: 2 in, 4 out]
              }
              frame False {
              }
            }
          }
          frame "Minimize", "Minimized" {
            w2484 = T21."Minimized" ("State")
            n1176 = property on="Property Node" class="VI"(reference=w2490, error in=w2489) -> (reference out=w2487:refnum<vi>, error out=w2488:errorcluster, "FP.State"=w2486:T21)
            n1177 = Not Equal?(x=w2486, y=w2484) -> (x != y?=w2485:bool)
            n1178 = case shown="True" w2485 {
              tunnel: [w2495 w2496] -> w2491
              tunnel: w2488 -> [w2494 w2496]
              tunnel: w2487 -> [w2493 _]
              tunnel: w2484 -> [w2492 _]
              frame True {
                n1179 = invoke on="Invoke Node" class="VI" method="FP.Open"(reference=w2493, error in=w2494, "State"=w2492) -> (error out=w2495:errorcluster)  [unwired: 2 in, 4 out]
              }
              frame False {
              }
            }
          }
          frame "Maximize", "Maximized" {
            w2497 = T21."Maximized" ("State")
            n1180 = property on="Property Node" class="VI"(reference=w2503, error in=w2502) -> (reference out=w2500:refnum<vi>, error out=w2501:errorcluster, "FP.State"=w2499:T21)
            n1181 = Not Equal?(x=w2499, y=w2497) -> (x != y?=w2498:bool)
            n1182 = case shown="True" w2498 {
              tunnel: [w2508 w2509] -> w2504
              tunnel: w2501 -> [w2507 w2509]
              tunnel: w2500 -> [w2506 _]
              tunnel: w2497 -> [w2505 _]
              frame True {
                n1183 = invoke on="Invoke Node" class="VI" method="FP.Open"(reference=w2506, error in=w2507, "State"=w2505) -> (error out=w2508:errorcluster)  [unwired: 2 in, 4 out]
              }
              frame False {
              }
            }
          }
        }
        n1184 = call <vilib>:"Add State(s) to Queue__JKI_lib_State_Machine.vi"("State(s) in (\"\")"=w2444) -> ("States Out"=w2443:string)  [unwired: 14 in]
      }
      frame "---------- AimingBeam ----------" {
        # "Template Separator\n(You can make a copy of, or modify, this frame)"
        n1185 = call <vilib>:"Add State(s) to Queue__JKI_lib_State_Machine.vi"("State(s) in (\"\")"=w2514) -> ("States Out"=w2513:string)  [unwired: 14 in]
      }
      frame "AimingBeam: Initialize" {
        # "set aiming beam button color"
        # "Open COM port for Aiming Beam\n(Require USB connection)"
        n1186 = Unbundle By Name(w2516) -> ("AB Cluster.Aiming Beam COM Port"=w2524:refnum<visa-resource-name>)
        n1187 = call-poly "VISA Configure Serial Port"("VISA resource name"=w2524, "Enable Termination\nChar (T)"=TRUE ("Enable Termination\nChar (T)"), "baud rate (9600)"=u32 9600, "error in (no error)"=w2521) -> ("error out"=w2520:errorcluster)  [unwired: 10 in, 1 out]
        n1188 = Unbundle By Name(w2520) -> ("status"=w2519:bool)
        n1189 = Not(x=w2519) -> (.not. x?=w2518:bool)
        n1190 = Bundle By Name(cluster=w2516, "System Status.Aiming Beam"=w2518) -> (w2517:T26)
        n1191 = call <vilib>:"Add State(s) to Queue__JKI_lib_State_Machine.vi"("State(s) in (\"\")"=w2526) -> ("States Out"=w2525:string)  [unwired: 14 in]
      }
      frame "AimingBeam: Close" {
        # "Close Aiming Beam COM port\n(Require USB connection to Aiming Beam Laser)"
        n1192 = Unbundle By Name(w2529) -> ("AB Cluster.Aiming Beam COM Port"=w2533:refnum<visa-resource-name>)
        n1193 = VISA Close(VISA resource name=w2533, error in (no error)=w2531) -> (error out=w2532:errorcluster)
        n1194 = Bundle By Name(cluster=w2529, "System Status.Aiming Beam"=FALSE) -> (w2530:T26)
        n1195 = call <vilib>:"Add State(s) to Queue__JKI_lib_State_Machine.vi"("State(s) in (\"\")"=w2535) -> ("States Out"=w2534:string)  [unwired: 14 in]
      }
      frame "AimingBeam: Set Current" {
        # "Set Aiming Beam Current\n(You can make a copy of, or modify, this frame)"
        n1196 = Unbundle By Name(w2550) -> ("AB Cluster.Aiming Beam COM Port"=w2543:refnum<visa-resource-name>, "AB Cluster.Max Current"=w2539:dbl, "AB Cluster.Default Current"=w2541:dbl, "AB Cluster.Min Current"=w2540:dbl)
        n1197 = In Range and Coerce(upper limit=w2539, x=w2541, lower limit=w2540) -> (coerced(x)=w2536:dbl)  [unwired: 1 out]
        n1198 = Number To Fractional String(number=w2536, precision (6)=i16 2) -> (F-format string=w2544:string)  [unwired: 2 in]
        n1199 = Concatenate Strings("slc:", w2544, "\r" ("Carriage Return Constant"), "\n" ("Line Feed Constant")) -> (w2547:string)
        n1200 = VISA Write(VISA resource name=w2543, write buffer=w2547, error in (no error)=w2538) -> (error out=w2542:errorcluster)  [unwired: 2 out]
        n1201 = call <vilib>:"Add State(s) to Queue__JKI_lib_State_Machine.vi"("State(s) in (\"\")"=w2552) -> ("States Out"=w2551:string)  [unwired: 14 in]
      }
      frame "AimingBeam: Set Status" {
        # "Enable Aiming Beam\n(Usage: \"AimingBeam: Set >> Enable|Disable\")"
        n1202 = Unbundle By Name(w2559) -> ("AB Cluster.Aiming Beam COM Port"=w2556:refnum<visa-resource-name>)
        n1203 = case shown="\"Enable\"" w2558 {
          tunnel: [w2562 w2566] -> w2557
          frame "Disable", Default {
            n1204 = Concatenate Strings("cof", "\r" ("Carriage Return Constant"), "\n" ("Line Feed Constant")) -> (w2562:string)
          }
          frame "Enable" {
            n1205 = Concatenate Strings("con", "\r" ("Carriage Return Constant"), "\n" ("Line Feed Constant")) -> (w2566:string)
          }
        }
        n1206 = VISA Write(VISA resource name=w2556, write buffer=w2557, error in (no error)=w2554) -> (error out=w2555:errorcluster)  [unwired: 2 out]
        n1207 = call <vilib>:"Add State(s) to Queue__JKI_lib_State_Machine.vi"("State(s) in (\"\")"=w2561) -> ("States Out"=w2560:string)  [unwired: 14 in]
      }
      frame "AimingBeam: GetPWMStatus" {
        # "Get aiming beam PWM status\n()"
        n1208 = Unbundle By Name(w2574) -> ("AB Cluster.Freq"=w2573:i32, "LJ Pinout.AimingBeam PWM"=w2580:string)
        n1209 = Equal To 0?(x=w2573) -> (x = 0?=w2572:bool)
        n1210 = call "LabJack_FGV.vi"("Operation(Read)"=enum16{"Write", "Read"}."Read" ("Operation"), "error in (no error)"=w2576) -> ("error out"=w2578:errorcluster, "Read data"=w2579:i32)  [unwired: 8 in]
        n1211 = case shown="True" w2572 {
          tunnel: w2580 -> [w2593 _]
          tunnel: [w2591 "DIO_STATE"] -> w2577
          frame False {
            n1212 = Concatenate Strings(w2593, "_EF_ENABLE" ("string")) -> (w2591:string)
          }
          frame True {
          }
        }
        n1213 = call "LJM_eReadName.vi"("Handle In"=w2579, "Name"=w2577, "error in"=w2578) -> ("Value"=w2571:dbl, "error out"=w2575:errorcluster)  [unwired: 10 in, 1 out]
        n1214 = case shown="True" w2572 {
          tunnel: w2571 -> [w2586 w2590]
          tunnel: [w2585 w2587] -> w2570
          frame False {
            n1215 = Greater Than 0?(x=w2586) -> (x > 0?=w2585:bool)
          }
          frame True {
            n1216 = Number To Boolean Array(number=w2590) -> (Boolean array=w2589:bool[])
            n1217 = Index Array(array=w2589, index=3) -> (element=w2587:bool)
          }
        }
        n1218 = case shown="False" w2570 {
          frame False {
            # "PWM is off\nset color to dark green"
            n1219 = local write "Aiming beam toggle"(FALSE ("Aimging beam")) -> ()
          }
          frame True {
            # "PWM is on\nset color to light green"
            n1220 = local write "Aiming beam toggle"(TRUE ("Aimging beam")) -> ()
          }
        }
        n1221 = call <vilib>:"Add State(s) to Queue__JKI_lib_State_Machine.vi"("State(s) in (\"\")"=w2584) -> ("States Out"=w2583:string)  [unwired: 14 in]
      }
      frame "---------- 355 Laser ----------" {
        # "Template Separator\n(You can make a copy of, or modify, this frame)"
        n1222 = call <vilib>:"Add State(s) to Queue__JKI_lib_State_Machine.vi"("State(s) in (\"\")"=w2601) -> ("States Out"=w2600:string)  [unwired: 14 in]
      }
      frame "355 Laser: Check Dewelling" {
        # "if time laser start time is less than 7.5s before, wait 250ms then check again."
        # "Template Separator\n(You can make a copy of, or modify, this frame)"
        n1223 = Unbundle By Name(w2609) -> ("Laser start tic"=w2606:u32)
        n1224 = Tick Count (ms)() -> (millisecond timer value=w2607:u32)
        n1225 = Subtract(x=w2607, y=w2606) -> (x-y=w2605:u32)
        n1226 = Greater?(x=w2605, y=u32 5000) -> (0:w2603:bool)
        n1227 = case shown="False" w2603 {
          tunnel: ["355 Laser: Check Dewelling" ""] -> w2602
          frame False {
            n1228 = Wait (ms)(milliseconds to wait=u32 250) -> ()  [unwired: 1 out]
          }
          frame True {
          }
        }
        n1229 = call <vilib>:"Add State(s) to Queue__JKI_lib_State_Machine.vi"("State(s) in Front (\"\")"=w2602, "State(s) in (\"\")"=w2612) -> ("States Out"=w2611:string)  [unwired: 13 in]
      }
      frame "355 Laser: Laser enable" {
        # "Laser enable/disable\n(Usage: \"LabJack: Laser enable/disable >> 1|0\")"
        n1230 = Unbundle By Name(w2619) -> ("LJ Pinout.Laser Start/Stop"=w2623:string, "System Status.355 Laser"=w2617:bool)
        n1231 = case shown="False" w2617 {
          tunnel: w2616 -> [w2638 w2639]
          tunnel: w2623 -> [w2632 _]
          tunnel: [w2627 w2639] -> w2621
          tunnel: [w2626 u32 0 ("millisecond timer value")] -> w2618
          frame False {
            n1232 = call "LabJack_FGV.vi"("Operation(Read)"=enum16{"Write", "Read"}."Read" ("Operation")) -> ("Read data"=w2634:i32)  [unwired: 9 in, 1 out]
            n1233 = call "LJM_eWriteName.vi"("Handle In"=w2634, "Name"=w2632, "Value"=1.0, "error in"=w2638) -> ("Handle Out"=w2633:i32, "error out"=w2631:errorcluster)  [unwired: 10 in]
            n1234 = call <userlib>:"Wait (ms)__ogtk.vi"("error in (no error)"=w2631, "milliseconds to wait"=u32 250) -> ("error out"=w2630:errorcluster)  [unwired: 8 in, 1 out]
            n1235 = call "LJM_eWriteName.vi"("Handle In"=w2633, "Name"=w2632, "Value"=0.0, "error in"=w2630) -> ("error out"=w2628:errorcluster)  [unwired: 10 in, 1 out]
            n1236 = call <userlib>:"Tick Count (ms)__ogtk.vi"("error in (no error)"=w2628) -> ("error out"=w2627:errorcluster, "millisecond timer value"=w2626:u32)  [unwired: 9 in]
          }
          frame True {
          }
        }
        n1237 = Bundle By Name(cluster=w2619, "Laser start tic"=w2618) -> (w2620:T26)
        n1238 = call <vilib>:"Add State(s) to Queue__JKI_lib_State_Machine.vi"("State(s) in (\"\")"=w2625) -> ("States Out"=w2624:string)  [unwired: 14 in]
      }
      frame "355 Laser: Laser disable" {
        # "Laser enable/disable\n(Usage: \"LabJack: Laser enable/disable >> 1|0\")"
        n1239 = Unbundle By Name(w2643) -> ("LJ Pinout.Laser Start/Stop"=w2647:string, "System Status.355 Laser"=w2641:bool)
        n1240 = case shown="True" w2641 {
          tunnel: w2648 -> [w2651 w2665]
          tunnel: w2647 -> [_ w2659]
          tunnel: [w2651 w2654] -> w2645
          tunnel: [u32 0 ("millisecond timer value") w2653] -> w2642
          frame False {
          }
          frame True {
            n1241 = call "LabJack_FGV.vi"("Operation(Read)"=enum16{"Write", "Read"}."Read" ("Operation")) -> ("Read data"=w2661:i32)  [unwired: 9 in, 1 out]
            n1242 = call "LJM_eWriteName.vi"("Handle In"=w2661, "Name"=w2659, "Value"=1.0, "error in"=w2665) -> ("Handle Out"=w2660:i32, "error out"=w2658:errorcluster)  [unwired: 10 in]
            n1243 = call <userlib>:"Wait (ms)__ogtk.vi"("error in (no error)"=w2658, "milliseconds to wait"=u32 250) -> ("error out"=w2657:errorcluster)  [unwired: 8 in, 1 out]
            n1244 = call "LJM_eWriteName.vi"("Handle In"=w2660, "Name"=w2659, "Value"=0.0, "error in"=w2657) -> ("error out"=w2655:errorcluster)  [unwired: 10 in, 1 out]
            n1245 = call <userlib>:"Tick Count (ms)__ogtk.vi"("error in (no error)"=w2655) -> ("error out"=w2654:errorcluster, "millisecond timer value"=w2653:u32)  [unwired: 9 in]
          }
        }
        n1246 = Bundle By Name(cluster=w2643, "Laser start tic"=w2642) -> (w2644:T26)
        n1247 = call <vilib>:"Add State(s) to Queue__JKI_lib_State_Machine.vi"("State(s) in (\"\")"=w2650) -> ("States Out"=w2649:string)  [unwired: 14 in]
      }
      frame "355 Laser: Dewelling" {
        # "Wait some time (ms)\n(355 Laser: Dewelling >> #)"
        n1248 = Fract/Exp String To Number(string=w2669, default (0 dbl)=0) -> (number=w2667:i32)  [unwired: 2 in, 1 out]
        n1249 = Wait (ms)(milliseconds to wait=w2667) -> ()  [unwired: 1 out]
        n1250 = call <vilib>:"Add State(s) to Queue__JKI_lib_State_Machine.vi"("State(s) in (\"\")"=w2673) -> ("States Out"=w2672:string)  [unwired: 14 in]
      }
      frame "355 Laser: Close" {
        # "Template Separator\n(You can make a copy of, or modify, this frame)"
        n1251 = call <vilib>:"Add State(s) to Queue__JKI_lib_State_Machine.vi"("State(s) in Front (\"\")"="355 Laser: CheckControllerStatus\n355 Laser: Laser disable\n355 Laser: Dewelling >>1000", "State(s) in (\"\")"=w2679) -> ("States Out"=w2678:string)  [unwired: 13 in]
      }
      frame "355 Laser: CheckControllerStatus" {
        # "if average < 2, laser no power\nif average 2 < average < 9.3, laser on\nif 9.3<average<10, interlock open, blink indicator\nif average > 10, laser off\n[Covers: REQ30]"
        # "take 10 measuremt and look at average"
        # "Check 355 laser controller status\nBy probing Emisison Lamp negative terminal voltage"
        n1252 = Unbundle By Name(w2688) -> ("LJ Pinout.Laser Ready"=w2691:string)
        n1253 = call "LabJack_FGV.vi"("Operation(Read)"=enum16{"Write", "Read"}."Read" ("Operation")) -> ("Read data"=w2692:i32)  [unwired: 9 in, 1 out]
        n1254 = for {
          N: 20 -> [_]
          tunnel: w2692 -> [w2703]
          tunnel: w2691 -> [w2702]
          shift-right: [w2701] -> w2684
          shift-left: w2690 -> [w2700]
          tunnel: [w2698] -> w2683 mode=indexing
          n1255 = call "LJM_eReadName.vi"("Handle In"=w2703, "Name"=w2702, "error in"=w2700) -> ("Value"=w2698:dbl, "error out"=w2701:errorcluster)  [unwired: 10 in, 1 out]
          n1256 = Wait (ms)(milliseconds to wait=u32 25) -> ()  [unwired: 1 out]
        }
        n1257 = call "checkLaserStatus.vi"("error in (no error)"=w2684, "Laser LED voltage"=w2683) -> ("error out"=w2685:errorcluster, "Interlock open?"=w2680:bool, "Laser on?"=w2682:bool, "Mean voltage"=→"laser EM lamp V":dbl)  [unwired: 6 in]
        n1258 = Bundle By Name(cluster=w2688, "System Status.355 Laser"=w2682) -> (w2689:T26)
        n1259 = case shown="True" w2680 {
          frame False {
            n1260 = property on="355 Laser" class="Bool (strict)"("Blinking"=FALSE) -> ()  [unwired: 2 in, 2 out]
          }
          frame True {
            n1261 = property on="355 Laser" class="Bool (strict)"("Blinking"=TRUE) -> ()  [unwired: 2 in, 2 out]
          }
        }
        n1262 = call <vilib>:"Add State(s) to Queue__JKI_lib_State_Machine.vi"("State(s) in (\"\")"=w2695) -> ("States Out"=w2694:string)  [unwired: 14 in]
      }
      frame "355 Laser: CheckPWMStatus" {
        # "Check 355 laser PWM status\n(Read LJ DIO#EF_ENABLE register to determine PWM status)"
        n1263 = Unbundle By Name(w2713) -> ("LJ Pinout.355 PWM"=w2712:string)
        n1264 = call "LabJack_FGV.vi"("Operation(Read)"=enum16{"Write", "Read"}."Read" ("Operation"), "error in (no error)"=w2706) -> ("error out"=w2709:errorcluster, "Read data"=w2710:i32)  [unwired: 8 in]
        n1265 = Concatenate Strings(w2712, "_EF_ENABLE" ("string")) -> (w2708:string)
        n1266 = call "LJM_eReadName.vi"("Handle In"=w2710, "Name"=w2708, "error in"=w2709) -> ("Value"=w2705:dbl, "error out"=w2707:errorcluster)  [unwired: 10 in, 1 out]
        n1267 = Greater Than 0?(x=w2705) -> (x > 0?=w2704:bool)
        n1268 = case shown="False" w2704 {
          frame False {
            # "PWM is off\nset color to gray"
            n1269 = local write "355nm Laser toggle"(FALSE ("355nm Laser")) -> ()
          }
          frame True {
            # "PWM is on\nset color to light green"
            n1270 = local write "355nm Laser toggle"(TRUE ("355nm Laser")) -> ()
          }
        }
        n1271 = call <vilib>:"Add State(s) to Queue__JKI_lib_State_Machine.vi"("State(s) in (\"\")"=w2717) -> ("States Out"=w2716:string)  [unwired: 14 in]
      }
      frame "355 Laser: Start" {
        # "Template Separator\n(You can make a copy of, or modify, this frame)"
        n1272 = call <vilib>:"Add State(s) to Queue__JKI_lib_State_Machine.vi"("State(s) in Front (\"\")"="LabJack: 355_PWM_Start", "State(s) in (\"\")"=w2725) -> ("States Out"=w2724:string)  [unwired: 13 in]
      }
      frame "355 Laser: Stop" {
        # "Template Separator\n(You can make a copy of, or modify, this frame)"
        n1273 = call <vilib>:"Add State(s) to Queue__JKI_lib_State_Machine.vi"("State(s) in Front (\"\")"="LabJack: 355_PWM_Stop", "State(s) in (\"\")"=w2731) -> ("States Out"=w2730:string)  [unwired: 13 in]
      }
      frame "---------- Utility ----------" {
        # "Template Separator\n(You can make a copy of, or modify, this frame)"
        n1274 = call <vilib>:"Add State(s) to Queue__JKI_lib_State_Machine.vi"("State(s) in (\"\")"=w2736) -> ("States Out"=w2735:string)  [unwired: 14 in]
      }
      frame "Utility: SetDataClass" {
        # "Set Data Class in Queues\n(Set data class to either Data, Bg or Cali)"
        n1275 = case shown="\"Cali\"" w2738 {
          tunnel: [enum16{"Data", "BG", "Cali"}."Data" ("Data Class") enum16{"Data", "BG", "Cali"}."BG" ("Data Class") enum16{"Data", "BG", "Cali"}."Cali" ("Data Class")] -> w2737
          frame "Data", Default {
          }
          frame "Bg" {
          }
          frame "Cali" {
          }
        }
        n1276 = local write "Data Class"(w2737) -> ()
        n1277 = call <vilib>:"Add State(s) to Queue__JKI_lib_State_Machine.vi"("State(s) in (\"\")"=w2743) -> ("States Out"=w2742:string)  [unwired: 14 in]
      }
      frame "Utility: AquiTimerReset" {
        # "Set Aquisition Timer\n(You can make a copy of, or modify, this frame)"
        n1278 = Tick Count (ms)() -> (millisecond timer value=w2749:u32)
        n1279 = Bundle By Name(cluster=w2747, "Aquisition Timer"=w2749) -> (w2748:T26)
        n1280 = call <vilib>:"Add State(s) to Queue__JKI_lib_State_Machine.vi"("State(s) in (\"\")"=w2753) -> ("States Out"=w2752:string)  [unwired: 14 in]
      }
      frame "Utility: AquiTimerCheck" {
        # "5min to ms"
        # "Set Aquisition Timer\n([Covers: REQ35])"
        n1281 = Unbundle By Name(w2761) -> ("Aquisition Timer"=w2759:u32)
        n1282 = Tick Count (ms)() -> (millisecond timer value=w2760:u32)
        n1283 = Subtract(x=w2760, y=w2759) -> (x-y=w2758:u32)
        n1284 = Multiply(x=1000, y=300) -> (x*y=w2755:i32)
        n1285 = Greater Or Equal?(x=w2758, y=w2755) -> (x >= y?=w2754:bool)
        n1286 = case shown="True" w2754 {
          frame False {
            # "do nothing"
          }
          frame True {
            # "if timed out, stop aquisition"
            n1287 = property on="StopButton" class="Bool (strict)"("Val(Sgnl)"=TRUE ("Value (Signaling)")) -> ()  [unwired: 2 in, 2 out]
          }
        }
        n1288 = call <vilib>:"Add State(s) to Queue__JKI_lib_State_Machine.vi"("State(s) in (\"\")"=w2765) -> ("States Out"=w2764:string)  [unwired: 14 in]
      }
      frame "Utility: StartBeep" {
        # "Beep\n([Covers: REQ18])"
        n1289 = call <vilib>:"Beep.vi"("use system alert? (T)"=FALSE, "duration (msec)"=u32 1000, "frequency (Hz)"=u32 2000) -> ()  [unwired: 9 in]
        n1290 = call <vilib>:"Add State(s) to Queue__JKI_lib_State_Machine.vi"("State(s) in (\"\")"=w2774) -> ("States Out"=w2773:string)  [unwired: 14 in]
      }
      frame "Utility: EndBeep" {
        # "Beep\n([Covers: REQ18])"
        n1291 = flat-sequence {
          frame #0 {
            n1292 = call <vilib>:"Beep.vi"("use system alert? (T)"=FALSE, "duration (msec)"=u32 500, "frequency (Hz)"=u32 2000) -> ()  [unwired: 9 in]
          }
          frame #1 {
            n1293 = call <vilib>:"Beep.vi"("use system alert? (T)"=FALSE, "duration (msec)"=u32 500, "frequency (Hz)"=u32 2000) -> ()  [unwired: 9 in]
          }
        }
        n1294 = call <vilib>:"Add State(s) to Queue__JKI_lib_State_Machine.vi"("State(s) in (\"\")"=w2779) -> ("States Out"=w2778:string)  [unwired: 14 in]
      }
      frame "Utility: RestoreDeConChan" {
        # "Template Separator\n(You can make a copy of, or modify, this frame)"
        n1295 = global read "GlobalVariables.vi" "DeconChan Temp"() -> (w2786:T9)
        n1296 = local write "Radio Buttons"(w2786) -> ()
        n1297 = call <vilib>:"Add State(s) to Queue__JKI_lib_State_Machine.vi"("State(s) in (\"\")"=w2791) -> ("States Out"=w2790:string)  [unwired: 14 in]
      }
      frame "Utility: SaveDeconChan" {
        # "Save Decon Channel to global temp\n(You can make a copy of, or modify, this frame)"
        n1298 = flat-sequence {
          frame #0 {
            n1299 = local read "Radio Buttons"() -> (w2797:T9)
            n1300 = global write "GlobalVariables.vi" "DeconChan Temp"(w2797) -> ()
          }
          frame #1 {
            n1301 = local write "Radio Buttons"(T9."No Selection" ("Radio Buttons")) -> ()
          }
        }
        n1302 = flat-sequence {
          frame #0 {
          }
          frame #1 {
            (unwired) enum32{"No Selection", "Ch1", "Ch2", "Ch3"}."No Selection" ("Radio Buttons")
          }
        }
        n1303 = call <vilib>:"Add State(s) to Queue__JKI_lib_State_Machine.vi"("State(s) in (\"\")"=w2796) -> ("States Out"=w2795:string)  [unwired: 14 in]
      }
      frame "Utility: Dewelling" {
        # "Main loop dewell\n(Dewelling >> #)"
        n1304 = Fract/Exp String To Number(string=w2802, default (0 dbl)=0) -> (number=w2800:i32)  [unwired: 2 in, 1 out]
        n1305 = Wait (ms)(milliseconds to wait=w2800) -> ()  [unwired: 1 out]
        n1306 = call <vilib>:"Add State(s) to Queue__JKI_lib_State_Machine.vi"("State(s) in (\"\")"=w2806) -> ("States Out"=w2805:string)  [unwired: 14 in]
      }
      frame "Utility: SetAllChanManualGain" {
        w2807 = FALSE ("Value (Signaling)")
        # "Set all channel to manual gain\n(You can make a copy of, or modify, this frame)"
        n1307 = property on="Auto gain ch1" class="Bool (strict)"("Val(Sgnl)"=w2807) -> ()  [unwired: 2 in, 2 out]
        n1308 = property on="Auto gain ch2" class="Bool (strict)"("Val(Sgnl)"=w2807) -> ()  [unwired: 2 in, 2 out]
        n1309 = property on="Auto gain ch3" class="Bool (strict)"("Val(Sgnl)"=w2807) -> ()  [unwired: 2 in, 2 out]
        n1310 = property on="Auto gain ch4" class="Bool (strict)"("Val(Sgnl)"=w2807) -> ()  [unwired: 2 in, 2 out]
        n1311 = call <vilib>:"Add State(s) to Queue__JKI_lib_State_Machine.vi"("State(s) in (\"\")"=w2812) -> ("States Out"=w2811:string)  [unwired: 14 in]
      }
      frame "Utility: SetAllChanAutoGain" {
        w2813 = TRUE ("Value (Signaling)")
        # "Set all channels to auto gain\n(You can make a copy of, or modify, this frame)"
        n1312 = property on="Auto gain ch1" class="Bool (strict)"("Val(Sgnl)"=w2813) -> ()  [unwired: 2 in, 2 out]
        n1313 = property on="Auto gain ch2" class="Bool (strict)"("Val(Sgnl)"=w2813) -> ()  [unwired: 2 in, 2 out]
        n1314 = property on="Auto gain ch3" class="Bool (strict)"("Val(Sgnl)"=w2813) -> ()  [unwired: 2 in, 2 out]
        n1315 = property on="Auto gain ch4" class="Bool (strict)"("Val(Sgnl)"=w2813) -> ()  [unwired: 2 in, 2 out]
        n1316 = call <vilib>:"Add State(s) to Queue__JKI_lib_State_Machine.vi"("State(s) in (\"\")"=w2818) -> ("States Out"=w2817:string)  [unwired: 14 in]
      }
      frame "---------- SysLog ----------" {
        # "Template Separator\n(You can make a copy of, or modify, this frame)"
        n1317 = call <vilib>:"Add State(s) to Queue__JKI_lib_State_Machine.vi"("State(s) in (\"\")"=w2823) -> ("States Out"=w2822:string)  [unwired: 14 in]
      }
      frame "SysLog: OpenLogFile" {
        # "Template Separator\n(You can make a copy of, or modify, this frame)"
        n1318 = call <vilib>:"Add State(s) to Queue__JKI_lib_State_Machine.vi"("State(s) in (\"\")"=w2828) -> ("States Out"=w2827:string)  [unwired: 14 in]
      }
      frame "---------- Graph ----------" {
        # "Template Separator\n(You can make a copy of, or modify, this frame)"
        n1319 = call <vilib>:"Add State(s) to Queue__JKI_lib_State_Machine.vi"("State(s) in (\"\")"=w2833) -> ("States Out"=w2832:string)  [unwired: 14 in]
      }
      frame "Graph: SetXMultiplier" {
        # "Set X multiplier of WF graphs\n(You can make a copy of, or modify, this frame)"
        n1320 = call "Digitizer1_FGV.vi"() -> ("error out"=w2837:errorcluster, "Read data"=w2838:refnum<k15>)  [unwired: 10 in]
        n1321 = property class="niScope"(reference=w2838, error in=w2837) -> ("Min Sample Rate"=w2836:dbl)  [unwired: 2 out]
        n1322 = Divide(x=1.0, y=w2836) -> (x/y=w2834:dbl)
        n1323 = property on="Channel 1" class="WFGraph (strict)"("XScale.Multiplier"=w2834) -> ()  [unwired: 2 in, 2 out]
        n1324 = property on="Channel 2" class="WFGraph (strict)"("XScale.Multiplier"=w2834) -> ()  [unwired: 2 in, 2 out]
        n1325 = property on="Channel 3" class="WFGraph (strict)"("XScale.Multiplier"=w2834) -> ()  [unwired: 2 in, 2 out]
        n1326 = property on="Channel 4" class="WFGraph (strict)"("XScale.Multiplier"=w2834) -> ()  [unwired: 2 in, 2 out]
        n1327 = call <vilib>:"Add State(s) to Queue__JKI_lib_State_Machine.vi"("State(s) in (\"\")"=w2843) -> ("States Out"=w2842:string)  [unwired: 14 in]
      }
      frame "Graph: AddCursors" {
        # "Add BG and DC cursor to all graphs\n(You can make a copy of, or modify, this frame)"
        n1328 = property on="Channel 1" class="WFGraph (strict)"() -> ("XScale.Multiplier"=w2852:dbl)  [unwired: 2 in, 2 out]
        n1329 = global read "GlobalVariables.vi" "DC Idx1"() -> (w2851:i32)
        n1330 = global read "GlobalVariables.vi" "DC Idx2"() -> (w2850:i32)
        n1331 = global read "GlobalVariables.vi" "BG Idx1"() -> (w2849:i32)
        n1332 = global read "GlobalVariables.vi" "BG Idx2"() -> (w2848:i32)
        n1333 = property on="Channel 1" class="WFGraph (strict)"(error in=w2854) -> ("CrsrList"=w2863:T27)  [unwired: 1 in, 2 out]
        n1334 = property on="Channel 2" class="WFGraph (strict)"() -> ("CrsrList"=w2860:T27)  [unwired: 2 in, 2 out]
        n1335 = property on="Channel 3" class="WFGraph (strict)"() -> ("CrsrList"=w2859:T27)  [unwired: 2 in, 2 out]
        n1336 = property on="Channel 4" class="WFGraph (strict)"() -> ("CrsrList"=w2845:T27)  [unwired: 2 in, 2 out]
        n1337 = Build Array(w2851, w2850, w2849, w2848) -> (w2847:i32[])
        n1338 = Multiply(x=w2847, y=w2852) -> (x*y=w2846:dbl[])
        n1339 = for {
          tunnel: w2863 -> [w2877] mode=indexing
          tunnel: w2846 -> [w2870] mode=indexing
          tunnel: [w2876] -> w2862 mode=indexing
          tunnel: u32[] [6618880, 6618880, 16711680, 16711680] -> [w2869] mode=indexing
          tunnel: w2860 -> [w2875] mode=indexing
          tunnel: w2859 -> [w2874] mode=indexing
          tunnel: [w2873] -> w2858 mode=indexing
          tunnel: [w2872] -> w2857 mode=indexing
          tunnel: w2845 -> [w2871] mode=indexing
          tunnel: [w2868] -> w2844 mode=indexing
          n1340 = Bundle By Name(cluster=w2877, "Position.X"=w2870, "Color"=w2869) -> (w2876:T28)
          n1341 = Bundle By Name(cluster=w2875, "Position.X"=w2870, "Color"=w2869) -> (w2873:T28)
          n1342 = Bundle By Name(cluster=w2874, "Position.X"=w2870, "Color"=w2869) -> (w2872:T28)
          n1343 = Bundle By Name(cluster=w2871, "Position.X"=w2870, "Color"=w2869) -> (w2868:T28)
        }
        n1344 = property on="Channel 1" class="WFGraph (strict)"("CrsrList"=w2862) -> (error out=w2853:errorcluster)  [unwired: 2 in, 1 out]
        n1345 = property on="Channel 2" class="WFGraph (strict)"("CrsrList"=w2858) -> ()  [unwired: 2 in, 2 out]
        n1346 = property on="Channel 3" class="WFGraph (strict)"("CrsrList"=w2857) -> ()  [unwired: 2 in, 2 out]
        n1347 = property on="Channel 4" class="WFGraph (strict)"("CrsrList"=w2844) -> ()  [unwired: 2 in, 2 out]
        n1348 = control-ref of="Channel 1"() -> (w2856:refnum<vi>)
        n1349 = call <vilib>:"Add State(s) to Queue__JKI_lib_State_Machine.vi"("State(s) in (\"\")"=w2867) -> ("States Out"=w2866:string)  [unwired: 14 in]
        n1350 = call "UpdateCurserIdx(SubVI).vi"("error in (no error)"=w2853, "WaveformGraph in"=w2856) -> ("error out"=w2855:errorcluster)  [unwired: 9 in]
      }
      frame "Graph: SaveCursorLoc" {
        # "Save cursor location to ini file\n(Save cursor location to system setting ini file)"
        n1351 = global read "GlobalVariables.vi" "DC Idx1"() -> (w2884:i32)
        n1352 = global read "GlobalVariables.vi" "DC Idx2"() -> (w2883:i32)
        n1353 = global read "GlobalVariables.vi" "BG Idx1"() -> (w2882:i32)
        n1354 = global read "GlobalVariables.vi" "BG Idx2"() -> (w2881:i32)
        n1355 = Bundle("DC Idx1"=w2884, "DC Idx2"=w2883, "BG Idx1"=w2882, "BG Idx2"=w2881) -> (w2880:T49)  [unwired: 1 in]
        n1356 = call "writeCursorConfigMain.vi"("error in (no error)"=w2878, "Cursor Locations"=w2880) -> ("error out"=w2879:errorcluster)  [unwired: 9 in]
        n1357 = call <vilib>:"Add State(s) to Queue__JKI_lib_State_Machine.vi"("State(s) in (\"\")"=w2888) -> ("States Out"=w2887:string)  [unwired: 14 in]
      }
      frame "---------- APD ----------" {
        # "Template Separator\n(You can make a copy of, or modify, this frame)"
        n1358 = call <vilib>:"Add State(s) to Queue__JKI_lib_State_Machine.vi"("State(s) in (\"\")"=w2893) -> ("States Out"=w2892:string)  [unwired: 14 in]
      }
      frame "APD: Initialize" {
        w2900 = enum16{"Read", "Write"}."Write" ("Operation (Read)")
        w2899 = refnum<class "APDClass.lvclass"> refnum  # APDClass.lvclass
        # "Initialize APD FGV\n(Initialized APD FGV for holding data)"
        n1359 = call "APD1FGV.vi"("Error In"=w2894, "Operation (Read)"=w2900, "APDClass in"=w2899) -> ("Error Out"=w2898:errorcluster)  [unwired: 7 in, 1 out]
        n1360 = call "APD2FGV.vi"("Error In"=w2894, "Operation (Read)"=w2900, "APDClass in"=w2899) -> ("Error Out"=w2897:errorcluster)  [unwired: 7 in, 1 out]
        n1361 = call "APD3FGV.vi"("Error In"=w2894, "Operation (Read)"=w2900, "APDClass in"=w2899) -> ("Error Out"=w2896:errorcluster)  [unwired: 7 in, 1 out]
        n1362 = Merge Errors(w2898, w2897, w2896) -> (w2895:errorcluster)
        n1363 = call <vilib>:"Add State(s) to Queue__JKI_lib_State_Machine.vi"("State(s) in (\"\")"=w2904) -> ("States Out"=w2903:string)  [unwired: 14 in]
      }
      frame "APD: LoadFromSerial" {
        w2906 = enum16{"Read", "Write"}."Write" ("Operation (Read)")
        # "Load APD data from tdms file\n(load and update FGV)"
        n1364 = call "readAPDSerial.vi"("Error In"=w2913) -> ("Error Out"=w2909:errorcluster, "output cluster"=w2912:T29)  [unwired: 9 in]
        n1365 = Unbundle By Name(w2912) -> ("Ch1APDSerial#"=w2925:string, "Ch2APDSerial#"=w2911:string, "Ch3APDSerial#"=w2924:string, "Ch4APDSerial#"=w2910:string)
        n1366 = call "CreatFromSerialNumNoRaw.vi"("error in (no error)"=w2909, "APD Serial #"=w2925) -> ("error out"=w2922:errorcluster, "APDClass out"=w2923:refnum<class "APDClass.lvclass">)  [unwired: 8 in]
        n1367 = call "CreatFromSerialNumNoRaw.vi"("error in (no error)"=w2909, "APD Serial #"=w2911) -> ("error out"=w2920:errorcluster, "APDClass out"=w2921:refnum<class "APDClass.lvclass">)  [unwired: 8 in]
        n1368 = call "CreatFromSerialNumNoRaw.vi"("error in (no error)"=w2909, "APD Serial #"=w2924) -> ("error out"=w2918:errorcluster, "APDClass out"=w2919:refnum<class "APDClass.lvclass">)  [unwired: 8 in]
        n1369 = call "CreatFromSerialNumNoRaw.vi"("error in (no error)"=w2909, "APD Serial #"=w2910) -> ("error out"=w2907:errorcluster, "APDClass out"=w2908:refnum<class "APDClass.lvclass">)  [unwired: 8 in]
        n1370 = call "APD1FGV.vi"("Error In"=w2922, "Operation (Read)"=w2906, "APDClass in"=w2923) -> ("Error Out"=w2917:errorcluster)  [unwired: 7 in, 1 out]
        n1371 = call "APD2FGV.vi"("Error In"=w2920, "Operation (Read)"=w2906, "APDClass in"=w2921) -> ("Error Out"=w2915:errorcluster)  [unwired: 7 in, 1 out]
        n1372 = call "APD3FGV.vi"("Error In"=w2918, "Operation (Read)"=w2906, "APDClass in"=w2919) -> ("Error Out"=w2916:errorcluster)  [unwired: 7 in, 1 out]
        n1373 = call "APD4FGV.vi"("Error In"=w2907, "Operation (Read)"=w2906, "APDClass in"=w2908) -> ("Error Out"=w2905:errorcluster)  [unwired: 7 in, 1 out]
        n1374 = Merge Errors(w2917, w2915, w2916, w2905) -> (w2914:errorcluster)
        n1375 = call <vilib>:"Add State(s) to Queue__JKI_lib_State_Machine.vi"("State(s) in (\"\")"=w2929) -> ("States Out"=w2928:string)  [unwired: 14 in]
      }
      frame "APD: UpdateCtrlVLimit" {
        w2935 = enum16{"Read", "Write"}."Read" ("Operation (Read)")
        # "Set V limit\n(You can make a copy of, or modify, this frame)"
        n1376 = call "APD1FGV.vi"("Error In"=w2936, "Operation (Read)"=w2935) -> ("Error Out"=w2951:errorcluster, "APDClass out"=w2952:refnum<class "APDClass.lvclass">)  [unwired: 8 in]
        n1377 = call "APD2FGV.vi"("Error In"=w2936, "Operation (Read)"=w2935) -> ("Error Out"=w2949:errorcluster, "APDClass out"=w2950:refnum<class "APDClass.lvclass">)  [unwired: 8 in]
        n1378 = call "APD3FGV.vi"("Error In"=w2936, "Operation (Read)"=w2935) -> ("Error Out"=w2947:errorcluster, "APDClass out"=w2948:refnum<class "APDClass.lvclass">)  [unwired: 8 in]
        n1379 = call "APD4FGV.vi"("Error In"=w2936, "Operation (Read)"=w2935) -> ("Error Out"=w2933:errorcluster, "APDClass out"=w2934:refnum<class "APDClass.lvclass">)  [unwired: 8 in]
        n1380 = call-dynamic "ReadMaxCtrlV.vi"("error in (no error)"=w2951, "APDClass in"=w2952) -> ("error out"=w2942:errorcluster, "Numeric"=w2945:dbl)  [unwired: 7 in, 1 out]
        n1381 = call-dynamic "ReadMaxCtrlV.vi"("error in (no error)"=w2949, "APDClass in"=w2950) -> ("error out"=w2940:errorcluster, "Numeric"=w2944:dbl)  [unwired: 7 in, 1 out]
        n1382 = call-dynamic "ReadMaxCtrlV.vi"("error in (no error)"=w2947, "APDClass in"=w2948) -> ("error out"=w2938:errorcluster, "Numeric"=w2943:dbl)  [unwired: 7 in, 1 out]
        n1383 = call-dynamic "ReadMaxCtrlV.vi"("error in (no error)"=w2933, "APDClass in"=w2934) -> ("error out"=w2931:errorcluster, "Numeric"=w2932:dbl)  [unwired: 7 in, 1 out]
        n1384 = property on="V 1" class="DigNum (strict)"(error in=w2942, "Maximum"=w2945) -> (error out=w2941:errorcluster)  [unwired: 1 in, 1 out]
        n1385 = property on="V 2" class="DigNum (strict)"(error in=w2940, "Maximum"=w2944) -> (error out=w2939:errorcluster)  [unwired: 1 in, 1 out]
        n1386 = property on="V 4" class="DigNum (strict)"(error in=w2931, "Maximum"=w2932) -> (error out=w2930:errorcluster)  [unwired: 1 in, 1 out]
        n1387 = property on="V 3" class="DigNum (strict)"(error in=w2938, "Maximum"=w2943) -> (error out=w2937:errorcluster)  [unwired: 1 in, 1 out]
        n1388 = Merge Errors(w2941, w2939, w2937, w2930) -> (w2946:errorcluster)
        n1389 = call <vilib>:"Add State(s) to Queue__JKI_lib_State_Machine.vi"("State(s) in (\"\")"=w2956) -> ("States Out"=w2955:string)  [unwired: 14 in]
      }
      frame "APD: GetGainLimits" {
        w2961 = enum16{"Read", "Write"}."Read" ("Operation (Read)")
        # "Template Separator\n(You can make a copy of, or modify, this frame)"
        n1390 = call "APD1FGV.vi"("Error In"=w2962, "Operation (Read)"=w2961) -> ("Error Out"=w2967:errorcluster, "APDClass out"=w2968:refnum<class "APDClass.lvclass">)  [unwired: 8 in]
        n1391 = call "APD2FGV.vi"("Error In"=w2962, "Operation (Read)"=w2961) -> ("Error Out"=w2974:errorcluster, "APDClass out"=w2975:refnum<class "APDClass.lvclass">)  [unwired: 8 in]
        n1392 = call "APD3FGV.vi"("Error In"=w2962, "Operation (Read)"=w2961) -> ("Error Out"=w2972:errorcluster, "APDClass out"=w2973:refnum<class "APDClass.lvclass">)  [unwired: 8 in]
        n1393 = call "APD4FGV.vi"("Error In"=w2962, "Operation (Read)"=w2961) -> ("Error Out"=w2959:errorcluster, "APDClass out"=w2960:refnum<class "APDClass.lvclass">)  [unwired: 8 in]
        n1394 = call-dynamic "Read Gain Limits(Log).vi"("error in (no error)"=w2967, "APDClass in"=w2968) -> ("error out"=w2966:errorcluster, "GainLimits(Log)"=w2963:cluster{"GainMax":dbl, "GainMin":dbl})  [unwired: 7 in, 1 out]
        n1395 = call-dynamic "Read Gain Limits(Log).vi"("error in (no error)"=w2974, "APDClass in"=w2975) -> ("error out"=w2970:errorcluster, "GainLimits(Log)"=w2965:cluster{"GainMax":dbl, "GainMin":dbl})  [unwired: 7 in, 1 out]
        n1396 = call-dynamic "Read Gain Limits(Log).vi"("error in (no error)"=w2972, "APDClass in"=w2973) -> ("error out"=w2969:errorcluster, "GainLimits(Log)"=w2964:cluster{"GainMax":dbl, "GainMin":dbl})  [unwired: 7 in, 1 out]
        n1397 = call-dynamic "Read Gain Limits(Log).vi"("error in (no error)"=w2959, "APDClass in"=w2960) -> ("error out"=w2957:errorcluster, "GainLimits(Log)"=w2958:cluster{"GainMax":dbl, "GainMin":dbl})  [unwired: 7 in, 1 out]
        n1398 = Merge Errors(w2966, w2970, w2969, w2957) -> (w2971:errorcluster)
        n1399 = global write "GlobalVariables.vi" "Ch1GainLim(Log)"(w2963) -> ()
        n1400 = global write "GlobalVariables.vi" "Ch2GainLim(Log)"(w2965) -> ()
        n1401 = global write "GlobalVariables.vi" "Ch3GainLim(Log)"(w2964) -> ()
        n1402 = global write "GlobalVariables.vi" "Ch4GainLim(Log)"(w2958) -> ()
        n1403 = call <vilib>:"Add State(s) to Queue__JKI_lib_State_Machine.vi"("State(s) in (\"\")"=w2979) -> ("States Out"=w2978:string)  [unwired: 14 in]
      }
      frame "---------- TCP ----------" {
        # "Template Separator\n(You can make a copy of, or modify, this frame)"
        n1404 = call <vilib>:"Add State(s) to Queue__JKI_lib_State_Machine.vi"("State(s) in (\"\")"=w2984) -> ("States Out"=w2983:string)  [unwired: 14 in]
      }
      frame "TCP: InitializeNew" {
        # "if unsuccessful and count <10, increament count \nand try again"
        # "Initialize TCP connection to aimging beam computer\n(You can make a copy of, or modify, this frame)"
        n1405 = TCP Create Listener(10:u16 2100 ("port"), 11:"RTLT" ("service name")) -> (0:w2993:errorcluster, 3:w2985:refnum<k5>)  [unwired: 3 in, 1 out]
        n1406 = while {
          tunnel: w2985 -> [w3013]
          tunnel: w2993 -> [w3012]
          tunnel: [w3003] -> w2991
          tunnel: [w3000] -> w2987
          i -> [w3009]
          stop <- w3000 stop-if-true
          n1407 = TCP Wait On Listener(8:w3012, 9:200 ("timeout ms (wait forever: -1)"), 11:w3013) -> (0:w3010:errorcluster, 4:w3007:refnum<k5>)  [unwired: 1 in, 3 out]
          n1408 = Less Or Equal?(x=50, y=w3009) -> (x <= y?=w3006:bool)
          n1409 = case shown="No Error" w3010 {
            selector: w3010 -> [w3023 w3033]
            tunnel: w3007 -> [w3024 _]
            tunnel: [errorcluster {"status"=TRUE, "code"=0, "source"=""} ("No error") w3034] -> w3002
            tunnel: [w3015 FALSE ("TCP connected?")] -> w3003
            frame No Error {
              # "connection is ready, read data"
              n1410 = TCP Read(connection ID=w3024, bytes to read=512, error in (no error)=w3023, 7:T24."CRLF" ("mode (standard)"), 9:5000 ("timeout ms (25000)")) -> (connection ID out=w3017:refnum<k5>, data out=w3019:string, error out=w3016:errorcluster)
              n1411 = Concatenate Strings("alive" ("string"), "\r\n" ("End of Line Constant")) -> (w3020:string)
              n1412 = Equal?(x=w3020, y=w3019) -> (x = y?=w3018:bool)
              n1413 = case shown="False" w3018 {
                tunnel: w3017 -> [_ w3029]
                tunnel: w3016 -> [_ _]
                tunnel: [FALSE ("TCP connected?") TRUE ("TCP connected?")] -> w3015
                frame False {
                }
                frame True {
                  n1414 = call "TcpIDFGV.vi"("action"=enum16{"write", "read"}."write", "connection ID in"=w3029) -> ()  [unwired: 8 in, 2 out]
                }
              }
            }
            frame Error {
              # "connection not ready, keep waiting"
              n1415 = Unbundle By Name(w3033) -> ("code"=w3035:i32)
              n1416 = case shown="56" w3035 {
                tunnel: w3033 -> [w3036 _]
                tunnel: [w3036 w3037] -> w3034
                frame Default {
                }
                frame 56 {
                  w3037 = errorcluster {"status"=FALSE, "code"=0, "source"=""}  # No error
                }
              }
            }
          }
          n1417 = Select(t=errorcluster {"status"=TRUE, "code"=5001, "source"=""} ("error in (no error)"), s=w3006, f=errorcluster {"status"=FALSE, "code"=0, "source"=""} ("error in (no error)")) -> (s? t:f=w3001:errorcluster)
          n1418 = Merge Errors(w3002, w3001) -> (w3000:errorcluster)
        }
        n1419 = Unbundle By Name(w2987) -> ("code"=w2990:i32)
        n1420 = Bundle By Name(cluster=w2992, "System Status.TCP/IP"=w2991, "listener ID"=w2985) -> (w2997:T26)
        n1421 = global write "GlobalVariables.vi" "TCP connected?"(w2991) -> ()
        n1422 = Equal To 0?(x=w2990) -> (x = 0?=w2989:bool)
        n1423 = Select(t=errorcluster {"status"=FALSE, "code"=0, "source"=""} ("error in (no error)"), s=w2989, f=w2987) -> (s? t:f=w2986:errorcluster)
        n1424 = call <vilib>:"Add State(s) to Queue__JKI_lib_State_Machine.vi"("State(s) in (\"\")"=w2999) -> ("States Out"=w2998:string)  [unwired: 14 in]
      }
      frame "TCP: checkSource" {
        # "Check visualization PC video source\n(send !video_source message, listen for response, then parse it to binary mask)"
        n1425 = Unbundle By Name(w3044) -> ("System Status.TCP/IP"=w3047:bool)
        n1426 = case shown="True" w3047 {
          tunnel: w3046 -> [w3052 w3075]
          tunnel: [w3052 w3059] -> w3045
          tunnel: [w3051 w3064] -> w3042
          tunnel: [w3051 w3062] -> w3041
          tunnel: [w3051 w3063] -> w3040
          tunnel: [w3051 w3061] -> w3039
          tunnel: [w3051 w3053] -> w3038
          frame False {
            w3051 = FALSE
          }
          frame True {
            n1427 = call "TcpIDFGV.vi"("Error In"=w3075, "action"=enum16{"write", "read"}."read") -> ("Error Out"=w3072:errorcluster, "connection ID out"=w3074:refnum<k5>)  [unwired: 8 in]
            n1428 = call "TCP_WriteRead.vi"("error in (no error)"=w3072, "data in"="!video_source", "connectin ID in"=w3074) -> ("error out"=w3069:errorcluster, "data out"=w3071:string)  [unwired: 4 in, 1 out]
            n1429 = Scan From String(format string="!video_source:%d", input string=w3071, error in=w3069) -> (error out=w3060:errorcluster, output 1=w3058:i32)  [unwired: 2 in, 2 out]
            n1430 = case shown="5..7, 9..11, 13..15" w3058 {
              tunnel: w3060 -> [_ _ _ _]
              tunnel: [errorcluster {"status"=TRUE, "code"=5007, "source"="Visualization PC"} ("error out") errorcluster {"status"=FALSE, "code"=0, "source"=""} ("error out") errorcluster {"status"=FALSE, "code"=0, "source"=""} ("error out") errorcluster {"status"=FALSE, "code"=0, "source"=""} ("error out")] -> w3059
              tunnel: [FALSE FALSE FALSE TRUE] -> w3053
              frame 0, Default {
                # "No video source available or default"
                n1431 = property on="Video Source" class="RadioBtnsControl (strict)"("DisabledEnum"=T11."Disabled and Grayed Out" ("Disabled")) -> ()  [unwired: 2 in, 2 out]
              }
              frame 1..3 {
                # "one or both camera available"
                n1432 = local write "Video Source"(enum32{"Camera", "FrameGrabber"}."Camera" ("Video Source")) -> ()
                n1433 = property on="Video Source" class="RadioBtnsControl (strict)"("DisabledEnum"=T11."Disabled and Grayed Out" ("Disabled")) -> ()  [unwired: 2 in, 2 out]
              }
              frame 4, 8, 12 {
                # "one or both frame grabber available"
                n1434 = local write "Video Source"(enum32{"Camera", "FrameGrabber"}."FrameGrabber" ("Video Source")) -> ()
                n1435 = property on="Video Source" class="RadioBtnsControl (strict)"("DisabledEnum"=T11."Disabled and Grayed Out" ("Disabled")) -> ()  [unwired: 2 in, 2 out]
              }
              frame 5..7, 9..11, 13..15 {
                n1436 = property on="Video Source" class="RadioBtnsControl (strict)"("DisabledEnum"=T11."Enabled" ("Disabled")) -> ()  [unwired: 2 in, 2 out]
              }
            }
            n1437 = Integer to Fixed-Point Cast(fixed-point type=fxp<+,4,4> 0.0, integer=w3058) -> (fixed-point=w3057:fxp<+,4,4>)
            n1438 = Number To Boolean Array(number=w3057) -> (Boolean array=w3055:bool[])
            n1439 = Reverse 1D Array(array=w3055) -> (reversed array=w3054:bool[])
            n1440 = Index Array(array=w3054, index=0) -> (element=w3064:bool)
            n1441 = Index Array(array=w3054, index=1) -> (element=w3062:bool)
            n1442 = Index Array(array=w3054, index=2) -> (element=w3063:bool)
            n1443 = Index Array(array=w3054, index=3) -> (element=w3061:bool)
          }
        }
        n1444 = Bundle By Name(cluster=w3044, "video source.Main Frame Grabber"=w3042, "video source.Side Frame Grabber"=w3041, "video source.Main Camera"=w3040, "video source.Side Camera"=w3039, "bothVidSourceAvail"=w3038) -> (w3043:T26)
        n1445 = call <vilib>:"Add State(s) to Queue__JKI_lib_State_Machine.vi"("State(s) in (\"\")"=w3050) -> ("States Out"=w3049:string)  [unwired: 14 in]
      }
      frame "TCP: SyncTime" {
        # "Template Separator\n(You can make a copy of, or modify, this frame)"
        n1446 = Unbundle By Name(w3092) -> ("System Status.TCP/IP"=w3091:bool)
        n1447 = case shown="True" w3091 {
          tunnel: w3093 -> [_ w3101]
          frame False {
          }
          frame True {
            n1448 = call "TcpIDFGV.vi"("Error In"=w3101, "action"=enum16{"write", "read"}."read") -> ("Error Out"=w3100:errorcluster, "connection ID out"=w3097:refnum<k5>)  [unwired: 8 in]
            n1449 = call <userlib>:"Tick Count (ms)__ogtk.vi"("error in (no error)"=w3100) -> ("error out"=w3099:errorcluster, "millisecond timer value"=w3098:u32)  [unwired: 9 in]
            n1450 = while {
              tunnel: w3099 -> [w3121]
              tunnel: w3097 -> [w3120]
              tunnel: w3098 -> [w3109]
              stop <- w3104 stop-if-true
              n1451 = Concatenate Strings("latencycheck" ("string"), "\r\n" ("End of Line Constant")) -> (w3116:string)
              n1452 = TCP Read(connection ID=w3120, bytes to read=512, error in (no error)=w3121, 7:T24."CRLF" ("mode (standard)"), 9:2000 ("timeout ms (25000)")) -> (connection ID out=w3113:refnum<k5>, data out=w3111:string, error out=w3103:errorcluster)
              n1453 = Tick Count (ms)() -> (millisecond timer value=w3110:u32)
              n1454 = Subtract(x=w3110, y=w3109) -> (x-y=w3108:u32)
              n1455 = Equal?(x=w3111, y=w3116) -> (x = y?=w3112:bool)
              n1456 = case shown="True" w3112 {
                tunnel: w3113 -> [_ w3134]
                tunnel: w3111 -> [w3126 _]
                tunnel: [w3122 FALSE] -> w3106
                tunnel: w3103 -> [_ w3128]
                frame False {
                  n1457 = Concatenate Strings("synctimer" ("string"), "\r\n" ("End of Line Constant")) -> (w3123:string)
                  n1458 = Equal?(x=w3126, y=w3123) -> (x = y?=w3122:bool)
                  "Sync Success?" <- w3122
                }
                frame True {
                  n1459 = Concatenate Strings("latencycheck:" ("string"), "\r\n" ("End of Line Constant")) -> (w3133:string)
                  n1460 = TCP Write(connection ID=w3134, data in=w3133, error in (no error)=w3128, 9:1000 ("timeout ms (25000)")) -> (error out=w3127:errorcluster)  [unwired: 2 out]
                  n1461 = call <vilib>:"Clear Errors.vi"("error in (no error)"=w3127) -> ()  [unwired: 5 in, 2 out]
                }
              }
              n1462 = Greater?(x=w3108, y=u32 10000 ("x-y")) -> (0:w3105:bool)
              n1463 = Or(x=w3106, y=w3105) -> (x .or. y?=w3104:bool)
            }
          }
        }
        n1464 = call <vilib>:"Add State(s) to Queue__JKI_lib_State_Machine.vi"("State(s) in (\"\")"=w3096) -> ("States Out"=w3095:string)  [unwired: 14 in]
      }
      frame "TCP: SendSettingMacro" {
        # "Template Separator\n(You can make a copy of, or modify, this frame)"
        n1465 = Unbundle By Name(w3138) -> ("System Status.TCP/IP"=w3137:bool)
        n1466 = case shown="True" w3137 {
          tunnel: ["" ("Empty String Constant") "TCP: sendSubjectID\nTCP: sendScaleBarSetting\nTCP: sendScaleMaxMin\nTCP: sendDeconChannel\nTCP: sendANSI\nTCP: sendRadius\nTCP: send3Dsetting\nTCP: sendFirefly\nTCP: sendPentero"] -> w3136
          frame False {
          }
          frame True {
          }
        }
        n1467 = call <vilib>:"Add State(s) to Queue__JKI_lib_State_Machine.vi"("State(s) in Front (\"\")"=w3136, "State(s) in (\"\")"=w3141) -> ("States Out"=w3140:string)  [unwired: 13 in]
      }
      frame "TCP: sendRunNum" {
        # "Send run number to AB PC\n(You can make a copy of, or modify, this frame)"
        n1468 = Unbundle By Name(w3148) -> ("System Status.TCP/IP"=w3145:bool, "IDs.RunID"=w3149:i8)
        n1469 = Increment(x=w3149) -> (x+1=w3144:i8)
        n1470 = case shown="True" w3145 {
          tunnel: w3144 -> [_ w3163]
          tunnel: [w3153 w3155] -> w3147
          tunnel: w3146 -> [w3153 w3154]
          frame False {
          }
          frame True {
            n1471 = Number To Decimal String(number=w3163, width (-)=i16 3) -> (decimal integer string=w3158:string)
            n1472 = call "TcpIDFGV.vi"("Error In"=w3154, "action"=enum16{"write", "read"}."read") -> ("Error Out"=w3156:errorcluster, "connection ID out"=w3160:refnum<k5>)  [unwired: 8 in]
            n1473 = Concatenate Strings("!run:", w3158) -> (w3157:string)
            n1474 = call "TCP_WriteRead.vi"("error in (no error)"=w3156, "data in"=w3157, "connectin ID in"=w3160) -> ("error out"=w3155:errorcluster)  [unwired: 4 in, 2 out]
          }
        }
        n1475 = call <vilib>:"Add State(s) to Queue__JKI_lib_State_Machine.vi"("State(s) in (\"\")"=w3152) -> ("States Out"=w3151:string)  [unwired: 14 in]
      }
      frame "TCP: sendVideoSource" {
        # "Send video source \n(You can make a copy of, or modify, this frame)"
        n1476 = Unbundle By Name(w3165) -> ("System Status.TCP/IP"=w3164:bool)
        n1477 = case shown="True" w3164 {
          tunnel: [w3171 w3173] -> w3167
          tunnel: w3166 -> [w3171 w3172]
          frame False {
          }
          frame True {
            n1478 = case shown="\"Camera\", Default" "Video Source" {
              tunnel: [0 1] -> w3178
              frame "Camera", Default {
              }
              frame "FrameGrabber" {
              }
            }
            n1479 = call "TcpIDFGV.vi"("Error In"=w3172, "action"=enum16{"write", "read"}."read") -> ("Error Out"=w3174:errorcluster, "connection ID out"=w3180:refnum<k5>)  [unwired: 8 in]
            n1480 = Number To Decimal String(number=w3178) -> (decimal integer string=w3176:string)  [unwired: 1 in]
            n1481 = Concatenate Strings("!invivo:" ("data in"), w3176) -> (w3175:string)
            n1482 = call "TCP_WriteRead.vi"("error in (no error)"=w3174, "data in"=w3175, "connectin ID in"=w3180) -> ("error out"=w3173:errorcluster)  [unwired: 4 in, 2 out]
          }
        }
        n1483 = call <vilib>:"Add State(s) to Queue__JKI_lib_State_Machine.vi"("State(s) in (\"\")"=w3170) -> ("States Out"=w3169:string)  [unwired: 14 in]
      }
      frame "TCP: startRun" {
        # "Template Separator\n(You can make a copy of, or modify, this frame)"
        n1484 = Unbundle By Name(w3185) -> ("System Status.TCP/IP"=w3184:bool)
        n1485 = case shown="True" w3184 {
          tunnel: [w3191 w3193] -> w3187
          tunnel: w3186 -> [w3191 w3192]
          frame False {
          }
          frame True {
            n1486 = call "TcpIDFGV.vi"("Error In"=w3192, "action"=enum16{"write", "read"}."read") -> ("Error Out"=w3194:errorcluster, "connection ID out"=w3195:refnum<k5>)  [unwired: 8 in]
            n1487 = call "TCP_WriteRead.vi"("error in (no error)"=w3194, "data in"="!acquire:1", "connectin ID in"=w3195) -> ("error out"=w3193:errorcluster)  [unwired: 4 in, 2 out]
          }
        }
        n1488 = call <vilib>:"Add State(s) to Queue__JKI_lib_State_Machine.vi"("State(s) in (\"\")"=w3190) -> ("States Out"=w3189:string)  [unwired: 14 in]
      }
      frame "TCP: stopRun" {
        # "Send stop run to AB PC\n(You can make a copy of, or modify, this frame)"
        n1489 = Unbundle By Name(w3199) -> ("System Status.TCP/IP"=w3198:bool)
        n1490 = case shown="True" w3198 {
          tunnel: [w3205 w3207] -> w3201
          tunnel: w3200 -> [w3205 w3206]
          frame False {
            # "if not connected, do nothing"
          }
          frame True {
            # "If TCP connected, send stop run"
            n1491 = call "TcpIDFGV.vi"("Error In"=w3206, "action"=enum16{"write", "read"}."read") -> ("Error Out"=w3208:errorcluster, "connection ID out"=w3210:refnum<k5>)  [unwired: 8 in]
            n1492 = call "TCP_WriteRead.vi"("error in (no error)"=w3208, "data in"="!acquire:0", "connectin ID in"=w3210) -> ("error out"=w3207:errorcluster)  [unwired: 4 in, 2 out]
          }
        }
        n1493 = call <vilib>:"Add State(s) to Queue__JKI_lib_State_Machine.vi"("State(s) in (\"\")"=w3204) -> ("States Out"=w3203:string)  [unwired: 14 in]
      }
      frame "TCP: CheckConnection" {
        # "Check TCP/IP connection statuse\n(If connection is lost, throw error)"
        n1494 = Unbundle By Name(w3213) -> ("System Status.TCP/IP"=w3212:bool)
        n1495 = case shown="False" w3212 {
          frame False {
          }
          frame True {
            # "If TCP/IP is true check, otherwise skip"
          }
        }
        n1496 = call <vilib>:"Add State(s) to Queue__JKI_lib_State_Machine.vi"("State(s) in (\"\")"=w3217) -> ("States Out"=w3216:string)  [unwired: 14 in]
      }
      frame "TCP: sendSubjectID" {
        # "Send subject ID"
        n1497 = Unbundle By Name(w3219) -> ("System Status.TCP/IP"=w3218:bool, "CaseID"=w3222:string)
        n1498 = case shown="True" w3218 {
          tunnel: w3222 -> [_ w3233]
          tunnel: [w3226 w3228] -> w3221
          tunnel: w3220 -> [w3226 w3227]
          frame False {
          }
          frame True {
            n1499 = call "TcpIDFGV.vi"("Error In"=w3227, "action"=enum16{"write", "read"}."read") -> ("Error Out"=w3229:errorcluster, "connection ID out"=w3231:refnum<k5>)  [unwired: 8 in]
            n1500 = Concatenate Strings("!subject:", w3233) -> (w3230:string)
            n1501 = call "TCP_WriteRead.vi"("error in (no error)"=w3229, "data in"=w3230, "connectin ID in"=w3231) -> ("error out"=w3228:errorcluster)  [unwired: 4 in, 2 out]
          }
        }
        n1502 = call <vilib>:"Add State(s) to Queue__JKI_lib_State_Machine.vi"("State(s) in (\"\")"=w3225) -> ("States Out"=w3224:string)  [unwired: 14 in]
      }
      frame "TCP: sendScaleBarSetting" {
        # "Template Separator\n(You can make a copy of, or modify, this frame)"
        n1503 = Unbundle By Name(w3237) -> ("System Status.TCP/IP"=w3235:bool, "VideoConfig.Scale Bar"=w3236:bool)
        n1504 = case shown="True" w3235 {
          tunnel: [w3243 w3252] -> w3239
          tunnel: w3238 -> [w3243 w3251]
          tunnel: w3236 -> [_ w3250]
          frame False {
          }
          frame True {
            n1505 = Boolean To (0,1)(Boolean=w3250) -> (0, 1=w3249:i16)
            n1506 = call "TcpIDFGV.vi"("Error In"=w3251, "action"=enum16{"write", "read"}."read") -> ("Error Out"=w3253:errorcluster, "connection ID out"=w3254:refnum<k5>)  [unwired: 8 in]
            n1507 = Number To Fractional String(number=w3249, width (-)=i16 1, precision (6)=i16 0) -> (F-format string=w3247:string)  [unwired: 1 in]
            n1508 = Concatenate Strings("!autocolor:" ("data in"), w3247) -> (w3245:string)
            n1509 = call "TCP_WriteRead.vi"("error in (no error)"=w3253, "data in"=w3245, "connectin ID in"=w3254) -> ("error out"=w3252:errorcluster)  [unwired: 4 in, 2 out]
          }
        }
        n1510 = call <vilib>:"Add State(s) to Queue__JKI_lib_State_Machine.vi"("State(s) in (\"\")"=w3242) -> ("States Out"=w3241:string)  [unwired: 14 in]
      }
      frame "TCP: sendScaleMaxMin" {
        # "Send scale bar max and min to AB PC\n(You can make a copy of, or modify, this frame)"
        n1511 = Unbundle By Name(w3259) -> ("System Status.TCP/IP"=w3256:bool, "VideoConfig.Scale Low"=w3258:dbl, "VideoConfig.Scale High"=w3257:dbl)
        n1512 = case shown="True" w3256 {
          tunnel: [w3265 w3278] -> w3261
          tunnel: w3260 -> [w3265 w3277]
          tunnel: w3258 -> [_ w3276]
          tunnel: w3257 -> [_ w3267]
          frame False {
          }
          frame True {
            n1513 = call "TcpIDFGV.vi"("Error In"=w3277, "action"=enum16{"write", "read"}."read") -> ("Error Out"=w3279:errorcluster, "connection ID out"=w3280:refnum<k5>)  [unwired: 8 in]
            n1514 = Number To Fractional String(number=w3276, width (-)=i16 4, precision (6)=i16 2) -> (F-format string=w3272:string)  [unwired: 1 in]
            n1515 = Number To Fractional String(number=w3267, width (-)=i16 4, precision (6)=i16 2) -> (F-format string=w3268:string)  [unwired: 1 in]
            n1516 = Concatenate Strings("!color:" ("string"), w3272, ";" ("string"), w3268) -> (w3266:string)
            n1517 = call "TCP_WriteRead.vi"("error in (no error)"=w3279, "data in"=w3266, "connectin ID in"=w3280) -> ("error out"=w3278:errorcluster)  [unwired: 4 in, 2 out]
          }
        }
        n1518 = call <vilib>:"Add State(s) to Queue__JKI_lib_State_Machine.vi"("State(s) in (\"\")"=w3264) -> ("States Out"=w3263:string)  [unwired: 14 in]
      }
      frame "TCP: sendDeconChannel" {
        # "Send Decon channel\n(You can make a copy of, or modify, this frame)"
        n1519 = Unbundle By Name(w3283) -> ("System Status.TCP/IP"=w3282:bool)
        n1520 = case shown="True" w3282 {
          tunnel: [w3289 w3294] -> w3285
          tunnel: w3284 -> [w3289 w3293]
          frame False {
          }
          frame True {
            n1521 = local read "Radio Buttons"() -> (w3292:T9)
            n1522 = Increment(x=w3292) -> (x+1=w3291:T9)
            n1523 = Number To Decimal String(number=w3291) -> (decimal integer string=w3290:string)  [unwired: 1 in]
            n1524 = call "TcpIDFGV.vi"("Error In"=w3293, "action"=enum16{"write", "read"}."read") -> ("Error Out"=w3295:errorcluster, "connection ID out"=w3298:refnum<k5>)  [unwired: 8 in]
            n1525 = Concatenate Strings("!channel:", w3290) -> (w3296:string)
            n1526 = call "TCP_WriteRead.vi"("error in (no error)"=w3295, "data in"=w3296, "connectin ID in"=w3298) -> ("error out"=w3294:errorcluster)  [unwired: 4 in, 2 out]
          }
        }
        n1527 = call <vilib>:"Add State(s) to Queue__JKI_lib_State_Machine.vi"("State(s) in (\"\")"=w3288) -> ("States Out"=w3287:string)  [unwired: 14 in]
      }
      frame "TCP: sendANSI" {
        # "Template Separator\n(You can make a copy of, or modify, this frame)"
        n1528 = Unbundle By Name(w3302) -> ("System Status.TCP/IP"=w3300:bool, "VideoConfig.ANSI"=w3301:dbl)
        n1529 = case shown="True" w3300 {
          tunnel: [w3308 w3314] -> w3304
          tunnel: w3303 -> [w3308 w3313]
          tunnel: w3301 -> [_ w3312]
          frame False {
          }
          frame True {
            n1530 = Number To Fractional String(number=w3312) -> (F-format string=w3310:string)  [unwired: 3 in]
            n1531 = call "TcpIDFGV.vi"("Error In"=w3313, "action"=enum16{"write", "read"}."read") -> ("Error Out"=w3315:errorcluster, "connection ID out"=w3316:refnum<k5>)  [unwired: 8 in]
            n1532 = Concatenate Strings("!ansi:" ("data in"), w3310) -> (w3309:string)
            n1533 = call "TCP_WriteRead.vi"("error in (no error)"=w3315, "data in"=w3309, "connectin ID in"=w3316) -> ("error out"=w3314:errorcluster)  [unwired: 4 in, 2 out]
          }
        }
        n1534 = call <vilib>:"Add State(s) to Queue__JKI_lib_State_Machine.vi"("State(s) in (\"\")"=w3307) -> ("States Out"=w3306:string)  [unwired: 14 in]
      }
      frame "TCP: sendRadius" {
        # "Send drawing radius to AB PC\n(You can make a copy of, or modify, this frame)"
        n1535 = Unbundle By Name(w3320) -> ("System Status.TCP/IP"=w3318:bool, "VideoConfig.Radius"=w3319:dbl)
        n1536 = case shown="True" w3318 {
          tunnel: [w3326 w3332] -> w3322
          tunnel: w3321 -> [w3326 w3331]
          tunnel: w3319 -> [_ w3330]
          frame False {
          }
          frame True {
            n1537 = Number To Fractional String(number=w3330) -> (F-format string=w3329:string)  [unwired: 3 in]
            n1538 = Concatenate Strings("!radius:" ("data in"), w3329) -> (w3327:string)
            n1539 = call "TcpIDFGV.vi"("Error In"=w3331, "action"=enum16{"write", "read"}."read") -> ("Error Out"=w3333:errorcluster, "connection ID out"=w3334:refnum<k5>)  [unwired: 8 in]
            n1540 = call "TCP_WriteRead.vi"("error in (no error)"=w3333, "data in"=w3327, "connectin ID in"=w3334) -> ("error out"=w3332:errorcluster)  [unwired: 4 in, 2 out]
          }
        }
        n1541 = call <vilib>:"Add State(s) to Queue__JKI_lib_State_Machine.vi"("State(s) in (\"\")"=w3325) -> ("States Out"=w3324:string)  [unwired: 14 in]
      }
      frame "TCP: send3Dsetting" {
        # "Send 3D setting to AB computer\n(You can make a copy of, or modify, this frame)"
        n1542 = Unbundle By Name(w3338) -> ("System Status.TCP/IP"=w3336:bool, "VideoConfig.3D?"=w3337:bool)
        n1543 = case shown="True" w3336 {
          tunnel: [w3344 w3351] -> w3340
          tunnel: w3339 -> [w3344 w3350]
          tunnel: w3337 -> [_ w3349]
          frame False {
          }
          frame True {
            n1544 = Boolean To (0,1)(Boolean=w3349) -> (0, 1=w3348:i16)
            n1545 = Number To Fractional String(number=w3348) -> (F-format string=w3347:string)  [unwired: 3 in]
            n1546 = call "TcpIDFGV.vi"("Error In"=w3350, "action"=enum16{"write", "read"}."read") -> ("Error Out"=w3352:errorcluster, "connection ID out"=w3353:refnum<k5>)  [unwired: 8 in]
            n1547 = Concatenate Strings("!3dset:" ("data in"), w3347) -> (w3345:string)
            n1548 = call "TCP_WriteRead.vi"("error in (no error)"=w3352, "data in"=w3345, "connectin ID in"=w3353) -> ("error out"=w3351:errorcluster)  [unwired: 4 in, 2 out]
          }
        }
        n1549 = call <vilib>:"Add State(s) to Queue__JKI_lib_State_Machine.vi"("State(s) in (\"\")"=w3343) -> ("States Out"=w3342:string)  [unwired: 14 in]
      }
      frame "TCP: sendFirefly" {
        # "Template Separator\n(You can make a copy of, or modify, this frame)"
        n1550 = Unbundle By Name(w3356) -> ("System Status.TCP/IP"=w3355:bool)
        n1551 = case shown="False" w3355 {
          tunnel: [w3362 w3364] -> w3358
          tunnel: w3357 -> [w3362 w3363]
          frame False {
          }
          frame True {
            n1552 = call "TcpIDFGV.vi"("Error In"=w3363, "action"=enum16{"write", "read"}."read") -> ("Error Out"=w3365:errorcluster, "connection ID out"=w3367:refnum<k5>)  [unwired: 8 in]
            n1553 = call "TCP_WriteRead.vi"("error in (no error)"=w3365, "data in"="!firefly:0", "connectin ID in"=w3367) -> ("error out"=w3364:errorcluster)  [unwired: 4 in, 2 out]
          }
        }
        n1554 = call <vilib>:"Add State(s) to Queue__JKI_lib_State_Machine.vi"("State(s) in (\"\")"=w3361) -> ("States Out"=w3360:string)  [unwired: 14 in]
      }
      frame "TCP: sendPentero" {
        # "Send Pentero setting to AB computer\n(You can make a copy of, or modify, this frame)"
        n1555 = Unbundle By Name(w3370) -> ("System Status.TCP/IP"=w3369:bool)
        n1556 = case shown="True" w3369 {
          tunnel: [w3376 w3378] -> w3372
          tunnel: w3371 -> [w3376 w3377]
          frame False {
          }
          frame True {
            n1557 = call "TcpIDFGV.vi"("Error In"=w3377, "action"=enum16{"write", "read"}."read") -> ("Error Out"=w3379:errorcluster, "connection ID out"=w3381:refnum<k5>)  [unwired: 8 in]
            n1558 = call "TCP_WriteRead.vi"("error in (no error)"=w3379, "data in"="!pentero:0", "connectin ID in"=w3381) -> ("error out"=w3378:errorcluster)  [unwired: 4 in, 2 out]
          }
        }
        n1559 = call <vilib>:"Add State(s) to Queue__JKI_lib_State_Machine.vi"("State(s) in (\"\")"=w3375) -> ("States Out"=w3374:string)  [unwired: 14 in]
      }
      frame "TCP: sendChannel" {
        # "Send DeCon Channel to AB computer\n()"
        n1560 = Unbundle By Name(w3384) -> ("System Status.TCP/IP"=w3383:bool)
        n1561 = case shown="True" w3383 {
          tunnel: [w3390 w3394] -> w3386
          tunnel: w3385 -> [w3390 w3393]
          frame False {
          }
          frame True {
            n1562 = local read "Radio Buttons"() -> (w3392:T9)
            n1563 = case shown="\"No Selection\", Default" w3392 {
              tunnel: ["" ("data in") "!channel:1" ("data in") "!channel:2" ("data in") "!channel:3" ("data in")] -> w3391
              frame "No Selection", Default {
              }
              frame "Ch1" {
              }
              frame "Ch2" {
              }
              frame "Ch3" {
              }
            }
            n1564 = call "TcpIDFGV.vi"("Error In"=w3393, "action"=enum16{"write", "read"}."read") -> ("Error Out"=w3395:errorcluster, "connection ID out"=w3396:refnum<k5>)  [unwired: 8 in]
            n1565 = call "TCP_WriteRead.vi"("error in (no error)"=w3395, "data in"=w3391, "connectin ID in"=w3396) -> ("error out"=w3394:errorcluster)  [unwired: 4 in, 2 out]
          }
        }
        n1566 = call <vilib>:"Add State(s) to Queue__JKI_lib_State_Machine.vi"("State(s) in (\"\")"=w3389) -> ("States Out"=w3388:string)  [unwired: 14 in]
      }
      frame "TCP: startCam" {
        # "Send Pentero setting to AB computer\n(You can make a copy of, or modify, this frame)"
        n1567 = Unbundle By Name(w3403) -> ("System Status.TCP/IP"=w3402:bool)
        n1568 = case shown="True" w3402 {
          tunnel: [w3409 w3411] -> w3405
          tunnel: w3404 -> [w3409 w3410]
          frame False {
          }
          frame True {
            n1569 = call "TcpIDFGV.vi"("Error In"=w3410, "action"=enum16{"write", "read"}."read") -> ("Error Out"=w3412:errorcluster, "connection ID out"=w3414:refnum<k5>)  [unwired: 8 in]
            n1570 = call "TCP_WriteRead.vi"("error in (no error)"=w3412, "data in"="!focus:1", "connectin ID in"=w3414) -> ("error out"=w3411:errorcluster)  [unwired: 4 in, 2 out]
          }
        }
        n1571 = call <vilib>:"Add State(s) to Queue__JKI_lib_State_Machine.vi"("State(s) in (\"\")"=w3408) -> ("States Out"=w3407:string)  [unwired: 14 in]
      }
      frame "TCP: stopCam" {
        # "Send Pentero setting to AB computer\n(You can make a copy of, or modify, this frame)"
        n1572 = Unbundle By Name(w3417) -> ("System Status.TCP/IP"=w3416:bool)
        n1573 = case shown="True" w3416 {
          tunnel: [w3423 w3425] -> w3419
          tunnel: w3418 -> [w3423 w3424]
          frame False {
          }
          frame True {
            n1574 = call "TcpIDFGV.vi"("Error In"=w3424, "action"=enum16{"write", "read"}."read") -> ("Error Out"=w3426:errorcluster, "connection ID out"=w3428:refnum<k5>)  [unwired: 8 in]
            n1575 = call "TCP_WriteRead.vi"("error in (no error)"=w3426, "data in"="!focus:0", "connectin ID in"=w3428) -> ("error out"=w3425:errorcluster)  [unwired: 4 in, 2 out]
          }
        }
        n1576 = call <vilib>:"Add State(s) to Queue__JKI_lib_State_Machine.vi"("State(s) in (\"\")"=w3422) -> ("States Out"=w3421:string)  [unwired: 14 in]
      }
      frame "TCP: Close" {
        # "Close TCP connection\n()"
        n1577 = Unbundle By Name(w3432) -> ("System Status.TCP/IP"=w3430:bool)
        n1578 = case shown="True" w3430 {
          tunnel: [w3438 w3440] -> w3433
          tunnel: w3431 -> [w3438 w3439]
          frame False {
          }
          frame True {
            n1579 = call "TcpIDFGV.vi"("Error In"=w3439, "action"=enum16{"write", "read"}."read") -> ("Error Out"=w3442:errorcluster, "connection ID out"=w3443:refnum<k5>)  [unwired: 8 in]
            n1580 = TCP Close Connection(connection ID=w3443, error in (no error)=w3442) -> (error out=w3440:errorcluster)  [unwired: 1 in, 1 out]
          }
        }
        n1581 = case shown="Error .." w3433 {
          tunnel: [w3446 w3447] -> w3434
          tunnel: w3432 -> [w3445 w3447]
          frame No Error {
            w3444 = FALSE ("System Status.TCP/IP")
            n1582 = Bundle By Name(cluster=w3445, "System Status.TCP/IP"=w3444) -> (w3446:T26)
            n1583 = global write "GlobalVariables.vi" "TCP connected?"(w3444) -> ()
          }
          frame Error {
          }
        }
        n1584 = call <vilib>:"Add State(s) to Queue__JKI_lib_State_Machine.vi"("State(s) in (\"\")"=w3437) -> ("States Out"=w3436:string)  [unwired: 14 in]
      }
      frame "---------- PID ----------" {
        # "Template Separator\n(You can make a copy of, or modify, this frame)"
        n1585 = call <vilib>:"Add State(s) to Queue__JKI_lib_State_Machine.vi"("State(s) in (\"\")"=w3452) -> ("States Out"=w3451:string)  [unwired: 14 in]
      }
      frame "PID: loadPID" {
        # "Template Separator\n(You can make a copy of, or modify, this frame)"
        n1586 = call "readPIDSetting.vi"("Error In"=w3456) -> ("Error Out"=w3457:errorcluster, "Ch3 PID out"=w3453:T8, "Ch2 PID out"=w3454:T8, "Ch1 PID out"=w3455:T8)  [unwired: 7 in]
        n1587 = local write "Ch1 PID gains"(w3455) -> ()
        n1588 = local write "Ch2 PID gains"(w3454) -> ()
        n1589 = local write "Ch3 PID gains"(w3453) -> ()
        n1590 = local write "Ch4 PID gains"(w3453) -> ()
        n1591 = call <vilib>:"Add State(s) to Queue__JKI_lib_State_Machine.vi"("State(s) in (\"\")"=w3461) -> ("States Out"=w3460:string)  [unwired: 14 in]
      }
      frame "---------- Temp ----------" {
        # "Template Separator\n(You can make a copy of, or modify, this frame)"
        n1592 = call <vilib>:"Add State(s) to Queue__JKI_lib_State_Machine.vi"("State(s) in (\"\")"=w3466) -> ("States Out"=w3465:string)  [unwired: 14 in]
      }
    }
    n1593 = Not(x=w198) -> (.not. x?=w197:bool)
    n1594 = local write "ML?"(w197) -> ()
    "ML?" <- TRUE ("main loop running?")
  }
  n1595 = while {
    tunnel: w19 -> [w3504]
    tunnel: w18 -> [w3499]
    tunnel: [w3498] -> w17
    tunnel: w13 -> [w3494]
    tunnel: [w3493] -> w16
    shift-right: [w3485] -> _
    shift-left: _ -> [w3486]
    stop <- w3483 stop-if-true
    # "Read data from notifier and deconvolve it and send to Aiming Beam computer"
    n1596 = Wait on Notification(notifier=w3504, ignore previous (F)=FALSE) -> (notification=w3503:T14, error out=w3468:errorcluster)  [unwired: 2 in, 2 out]
    n1597 = flat-sequence {
      tunnel: [w3505] -> w3485
      tunnel: w3468 -> [_]
      frame #0 {
        n1598 = call <vilib>:"High Resolution Relative Seconds.vi"() -> ("relative seconds"=w3505:dbl)
      }
    }
    n1599 = Unbundle(w3503) -> ("idx"=w3473:i32, "CH1&2"=w3502:dbl[][], "CH3"=w3501:dbl[][], "V cluster"=w3489:cluster{"V1":dbl, "V2":dbl, "V3":dbl, "V4":dbl})
    n1600 = call "SeperateChanData.vi"("Input (Ch1&2)"=w3502) -> ("Ch1"=w3479:dbl[][], "Ch2"=w3477:dbl[][])
    n1601 = call "SeperateChanData.vi"("Input (Ch1&2)"=w3501) -> ("Ch1"=w3475:dbl[][], "Ch2"=w3472:dbl[][])
    n1602 = Subtract(x=w3485, y=w3486) -> (x-y=w3488:dbl)
    n1603 = call "AvgArrayTimeCritical.vi"("2D array"=w3479) -> ("1D Avg"=w3478:dbl[])  [unwired: 10 in]
    n1604 = call "AvgArrayTimeCritical.vi"("2D array"=w3477) -> ("1D Avg"=w3476:dbl[])  [unwired: 10 in]
    n1605 = call "AvgArrayTimeCritical.vi"("2D array"=w3475) -> ("1D Avg"=w3474:dbl[])  [unwired: 10 in]
    n1606 = call "AvgArrayTimeCritical.vi"("2D array"=w3472) -> ("1D Avg"=w3471:dbl[])  [unwired: 10 in]
    n1607 = Multiply(x=w3488, y=1000.0) -> (x*y=→"Decon Loop timing (ms)" →"Waveform Chart":dbl)
    n1608 = case shown="\"Ch4\"" "Radio Buttons" {
      selector: "Radio Buttons" -> [_ w3518 w3532 w3547 w3564]
      tunnel: w3478 -> [w3515 w3526 w3538 w3552 w3568]
      tunnel: w3476 -> [w3513 w3523 w3540 w3550 w3566]
      tunnel: w3474 -> [w3511 w3521 w3535 w3555 w3558]
      tunnel: FALSE -> [_ w3529 w3543 w3557 w3571]
      tunnel: w3468 -> [w3509 w3528 w3542 w3546 w3563]
      tunnel: [w3509 w3527 w3541 w3556 w3570] -> w3483
      tunnel: [w3514 w3524 w3536 w3551 w3567] -> w3492
      tunnel: [w3512 w3522 w3537 w3549 w3565] -> w3491
      tunnel: [w3510 w3520 w3534 w3553 w3559] -> w3490
      tunnel: [0.0 ("lifetime (ns)") w3519 w3533 w3548 w3562] -> w3467
      tunnel: w3471 -> [w3507 w3517 w3531 w3545 w3561]
      tunnel: [w3506 w3516 w3530 w3544 w3560] -> w3470
      frame "No Selection", Default {
        n1609 = Build Array(w3515) -> (w3514:dbl[][])
        n1610 = Build Array(w3513) -> (w3512:dbl[][])
        n1611 = Build Array(w3511) -> (w3510:dbl[][])
        n1612 = Build Array(w3507) -> (w3506:dbl[][])
      }
      frame "Ch1" {
        n1613 = call "Deconvolution.vi"("DeconChannel"=w3518, "iRF align"=w3529, "error in (no error)"=w3528, "Waveform"=w3526) -> ("error out"=w3527:errorcluster, "lifetime (ns)"=w3519:dbl, "Fitting"=w3525:dbl[])  [unwired: 5 in]
        "Lifetime 1" <- w3519
        n1614 = Build Array(w3526, w3525) -> (w3524:dbl[][])
        n1615 = Build Array(w3523) -> (w3522:dbl[][])
        n1616 = Build Array(w3521) -> (w3520:dbl[][])
        n1617 = Build Array(w3517) -> (w3516:dbl[][])
      }
      frame "Ch2" {
        n1618 = call "Deconvolution.vi"("DeconChannel"=w3532, "iRF align"=w3543, "error in (no error)"=w3542, "Waveform"=w3540) -> ("error out"=w3541:errorcluster, "lifetime (ns)"=w3533:dbl, "Fitting"=w3539:dbl[])  [unwired: 5 in]
        "Lifetime 2" <- w3533
        n1619 = Build Array(w3538) -> (w3536:dbl[][])
        n1620 = Build Array(w3540, w3539) -> (w3537:dbl[][])
        n1621 = Build Array(w3535) -> (w3534:dbl[][])
        n1622 = Build Array(w3531) -> (w3530:dbl[][])
      }
      frame "Ch3" {
        n1623 = call "Deconvolution.vi"("DeconChannel"=w3547, "iRF align"=w3557, "error in (no error)"=w3546, "Waveform"=w3555) -> ("error out"=w3556:errorcluster, "lifetime (ns)"=w3548:dbl, "Fitting"=w3554:dbl[])  [unwired: 5 in]
        "Lifetime 3" <- w3548
        n1624 = Build Array(w3552) -> (w3551:dbl[][])
        n1625 = Build Array(w3550) -> (w3549:dbl[][])
        n1626 = Build Array(w3555, w3554) -> (w3553:dbl[][])
        n1627 = Build Array(w3545) -> (w3544:dbl[][])
      }
      frame "Ch4" {
        n1628 = call "Deconvolution.vi"("DeconChannel"=w3564, "iRF align"=w3571, "error in (no error)"=w3563, "Waveform"=w3561) -> ("error out"=w3570:errorcluster, "lifetime (ns)"=w3562:dbl, "Fitting"=w3569:dbl[])  [unwired: 5 in]
        "Lifetime 4" <- w3562
        n1629 = Build Array(w3568) -> (w3567:dbl[][])
        n1630 = Build Array(w3566) -> (w3565:dbl[][])
        n1631 = Build Array(w3561, w3569) -> (w3560:dbl[][])
        n1632 = Build Array(w3558) -> (w3559:dbl[][])
      }
    }
    "Lifetime (ns)" <- w3467
    n1633 = Bundle(w3492, w3491, w3490, w3470, "V cluster"=w3489) -> (w3495:T50)  [unwired: 1 in]
    n1634 = Bundle("idx"=w3473, "lifetime (ns)"=w3467) -> (w3500:cluster{"idx":i32, "lifetime (ns)":dbl})  [unwired: 1 in]
    n1635 = Send Notification(notification=w3495, notifier=w3494, error in (no error)=w3483) -> (notifier out=w3493:refnum<notifier>, error out=w3482:errorcluster)
    n1636 = Send Notification(notification=w3500, notifier=w3499, error in (no error)=w3483) -> (notifier out=w3498:refnum<notifier>, error out=w3481:errorcluster)
    n1637 = Merge Errors(w3482, w3481) -> (→"decon error out":errorcluster)
  }
  n1638 = while {
    tunnel: w18 -> [w3582]
    shift-right: [w3575] -> _
    shift-left: u32 0 -> [w3576]
    stop <- w3573 stop-if-true
    # "Send data to AB computer here"
    # "if TCP ip is not open loop will run once and stop. To re-establish connection and start this loop. Reboot softwrae."
    # "Data communication loop"
    n1639 = Tick Count (ms)() -> (millisecond timer value=w3575:u32)
    n1640 = Wait on Notification(notifier=w3582, ignore previous (F)=FALSE) -> (notification=w3580:cluster{"idx":i32, "lifetime":dbl}, error out=w3574:errorcluster)  [unwired: 2 in, 2 out]
    n1641 = Unbundle(w3580) -> ("idx"=w3579:i32, "lifetime"=w3578:dbl)
    n1642 = global read "GlobalVariables.vi" "TCP connected?"() -> (w3572:bool)
    n1643 = Subtract(x=w3575, y=w3576) -> (x-y=→"Communication loop(ms)":u32)
    n1644 = case shown="True" w3572 {
      tunnel: w3579 -> [_ w3591]
      tunnel: w3578 -> [_ w3590]
      tunnel: w3574 -> [w3583 w3587]
      tunnel: [w3583 w3584] -> w3573
      frame False {
      }
      frame True {
        n1645 = Number To Decimal String(number=w3591) -> (decimal integer string=w3599:string)  [unwired: 1 in]
        n1646 = call "TcpIDFGV.vi"("Error In"=w3587, "action"=enum16{"write", "read"}."read") -> ("Error Out"=w3586:errorcluster, "connection ID out"=w3597:refnum<k5>)  [unwired: 8 in]
        n1647 = Concatenate Strings("!idx:", w3599) -> (w3600:string)
        n1648 = call "TCP_WriteRead.vi"("error in (no error)"=w3586, "data in"=w3600, "connectin ID in"=w3597) -> ("error out"=w3585:errorcluster, "connectin ID out"=w3598:refnum<k5>)  [unwired: 4 in, 1 out]
        n1649 = Number To Fractional String(number=w3590, precision (6)=i16 2) -> (F-format string=w3589:string)  [unwired: 2 in]
        n1650 = Concatenate Strings("!lifetime:", w3589) -> (w3596:string)
        n1651 = call "TCP_WriteRead.vi"("error in (no error)"=w3585, "data in"=w3596, "connectin ID in"=w3598) -> ("error out"=w3584:errorcluster, "data out"=→"data out(communcation loop)":string)  [unwired: 4 in, 1 out]
      }
    }
  }
  n1652 = while {
    tunnel: w13 -> [w3611]
    shift-right: [w3602] -> _
    shift-left: w15 -> [w3609]
    shift-right: [w3604] -> _
    shift-left: w15 -> [w3603]
    i -> [w3605]
    stop <- w3606 stop-if-true
    # "Data display loop(30Hz)"
    n1653 = Wait on Notification(notifier=w3611, ignore previous (F)=FALSE) -> (notification=w3607:T13, error out=w3606:errorcluster)  [unwired: 2 in, 2 out]
    n1654 = Wait Until Next ms Multiple(millisecond multiple=u32 33) -> ()  [unwired: 1 out]
    n1655 = Tick Count (ms)() -> (millisecond timer value=w3602:u32)
    n1656 = Subtract(x=w3602, y=w3609) -> (x-y=→"display loop timing(ms)":u32)
    n1657 = case shown="No Error" w3606 {
      tunnel: w3607 -> [w3684 _]
      tunnel: w3603 -> [w3656 w3756]
      tunnel: [w3658 w3756] -> w3604
      tunnel: w3602 -> [w3655 _]
      frame No Error {
        w3613 = u32 1 ("Active Plot")
        w3632 = 0 ("index (row)")
        n1658 = Subtract(x=w3655, y=w3656) -> (x-y=w3657:u32)
        n1659 = Unbundle(w3684) -> ("CH1"=w3679:dbl[][], "CH2"=w3677:dbl[][], "CH3"=w3674:dbl[][], "CH4"=w3627:dbl[][], "Gain cluster"=w3633:cluster{"V1":dbl, "V2":dbl, "V3":dbl, "V4":dbl})
        n1660 = Unbundle By Name(w3633) -> ("V1"=w3651:dbl, "V2"=w3649:dbl, "V3"=w3647:dbl, "V4"=w3625:dbl)
        n1661 = Index Array(array=w3679, index (row)=w3632) -> (element=w3663:dbl[])  [unwired: 1 in]
        n1662 = Index Array(array=w3677, index (row)=w3632) -> (element=w3661:dbl[])  [unwired: 1 in]
        n1663 = Index Array(array=w3674, index (row)=w3632) -> (element=w3662:dbl[])  [unwired: 1 in]
        n1664 = Index Array(array=w3627, index (row)=w3632) -> (element=w3631:dbl[])  [unwired: 1 in]
        n1665 = call "RemoveDCBG.vi"("Channel"=enum16{"DC Only", "Ch1", "Ch2", "Ch3", "Ch4"}."Ch4", "WF in"=w3631) -> ("DC"=w3629:dbl, "WF out"=w3618:dbl[])  [unwired: 7 in, 1 out]
        n1666 = Greater?(x=w3657, y=u32 200) -> (0:w3659:bool)
        n1667 = call "CtrlVtoGain.vi"("CtrlV(V)"=w3625, "Channel"=enum16{"Ch1", "Ch2", "Ch3", "Ch4"}."Ch4") -> ("Gain"=w3617:dbl)  [unwired: 8 in, 1 out]
        n1668 = call "CtrlVtoGain.vi"("CtrlV(V)"=w3651, "Channel"=enum16{"Ch1", "Ch2", "Ch3"}."Ch1") -> ("Gain"=w3645:dbl)  [unwired: 8 in, 1 out]
        n1669 = call "RemoveDCBG.vi"("Channel"=enum16{"DC Only", "Ch1", "Ch2", "Ch3"}."Ch1", "WF in"=w3663) -> ("DC"=w3680:dbl, "WF out"=w3652:dbl[])  [unwired: 7 in, 1 out]
        n1670 = call "RemoveDCBG.vi"("Channel"=enum16{"DC Only", "Ch1", "Ch2", "Ch3"}."Ch2", "WF in"=w3661) -> ("DC"=w3676:dbl, "WF out"=w3653:dbl[])  [unwired: 7 in, 1 out]
        n1671 = call "CtrlVtoGain.vi"("CtrlV(V)"=w3649, "Channel"=enum16{"Ch1", "Ch2", "Ch3"}."Ch2") -> ("Gain"=w3640:dbl)  [unwired: 8 in, 1 out]
        n1672 = call "RemoveDCBG.vi"("Channel"=enum16{"DC Only", "Ch1", "Ch2", "Ch3"}."Ch3", "WF in"=w3662) -> ("DC"=w3673:dbl, "WF out"=w3654:dbl[])  [unwired: 7 in, 1 out]
        n1673 = call "CtrlVtoGain.vi"("CtrlV(V)"=w3647, "Channel"=enum16{"Ch1", "Ch2", "Ch3"}."Ch3") -> ("Gain"=w3636:dbl)  [unwired: 8 in, 1 out]
        n1674 = formula code="int32 out = 2;\nif (G<5){\nout = 1;\n}\nif (G>200){\nout = 3;\n}"("G"=w3617) -> ("out"=→"output variable":i32)
        n1675 = Add(x=w3618, y=w3629) -> (x+y=w3628:dbl[])
        n1676 = Less?(x=w3617, y=5.0) -> (x < y?=w3623:bool)
        n1677 = case shown="True" w3659 {
          tunnel: w3652 -> [_ w3713]
          tunnel: w3653 -> [_ w3716]
          tunnel: w3654 -> [_ w3715]
          tunnel: w3655 -> [_ w3731]
          tunnel: [w3695 w3731] -> w3658
          tunnel: w3656 -> [w3695 _]
          tunnel: w3645 -> [_ w3709]
          tunnel: w3640 -> [_ w3708]
          tunnel: w3636 -> [_ w3707]
          tunnel: w3618 -> [_ w3703]
          tunnel: w3617 -> [_ w3700]
          frame False {
          }
          frame True {
            n1678 = call "GetSNR(SubVI).vi"("Waveform"=w3713) -> ("SNR"=→"SNR1":dbl)  [unwired: 10 in]
            n1679 = Array Size(array=w3713) -> (size(s)=w3714:i32)
            n1680 = call "GetSNR(SubVI).vi"("Waveform"=w3716) -> ("SNR"=→"SNR2":dbl)  [unwired: 10 in]
            n1681 = call "GetSNR(SubVI).vi"("Waveform"=w3715) -> ("SNR"=→"SNR3":dbl)  [unwired: 10 in]
            n1682 = call "GetSNR(SubVI).vi"("Waveform"=w3703) -> ("SNR"=→"SNR4":dbl)  [unwired: 10 in]
            n1683 = global read "GlobalVariables.vi" "BG Idx2"() -> (w3702:i32)
            n1684 = Subtract(x=w3714, y=w3702) -> (x-y=w3701:i32)
            n1685 = Array Subset(array=w3713, index=w3702, length=w3701) -> (w3720:dbl[])
            n1686 = Array Subset(array=w3716, index=w3702, length=w3701) -> (w3722:dbl[])
            n1687 = Array Subset(array=w3715, index=w3702, length=w3701) -> (w3724:dbl[])
            n1688 = Array Subset(array=w3703, index=w3702, length=w3701) -> (w3704:dbl[])
            n1689 = Add Array Elements(numeric array=w3720) -> (sum=w3721:dbl)
            n1690 = Add Array Elements(numeric array=w3722) -> (sum=w3723:dbl)
            n1691 = Add Array Elements(numeric array=w3724) -> (sum=w3725:dbl)
            n1692 = Add Array Elements(numeric array=w3704) -> (sum=w3705:dbl)
            n1693 = Divide(x=w3721, y=w3709) -> (x/y=w3726:dbl)
            n1694 = Divide(x=w3723, y=w3708) -> (x/y=w3727:dbl)
            n1695 = Divide(x=w3725, y=w3707) -> (x/y=w3728:dbl)
            n1696 = Divide(x=w3705, y=w3700) -> (x/y=w3699:dbl)
            n1697 = Build Array(w3726, w3727, w3728, w3699) -> (w3729:dbl[])
            n1698 = Add Array Elements(numeric array=w3729) -> (sum=w3730:dbl)
            n1699 = Divide(x=w3729, y=w3730) -> (x/y=w3698:dbl[])
            n1700 = Index Array(array=w3698, index=2) -> (element=→"IntR3":dbl)
            n1701 = Index Array(array=w3698, index=1) -> (element=→"IntR2":dbl)
            n1702 = Index Array(array=w3698, index=0) -> (element=→"IntR1":dbl)
            n1703 = Index Array(array=w3698, index=3) -> (element=→"IntR4":dbl)
          }
        }
        n1704 = Add(x=w3652, y=w3680) -> (x+y=w3678:dbl[])
        n1705 = Add(x=w3653, y=w3676) -> (x+y=w3675:dbl[])
        n1706 = Add(x=w3654, y=w3673) -> (x+y=w3672:dbl[])
        n1707 = Less?(x=w3645, y=5.0 ("x")) -> (x < y?=w3643:bool)
        n1708 = Less?(x=w3640, y=5.0 ("x")) -> (x < y?=w3639:bool)
        n1709 = Less?(x=w3636, y=5.0 ("x")) -> (x < y?=w3635:bool)
        n1710 = case shown="False" w3635 {
          tunnel: [u32 16448250 ("Plot.Plot Color") u32 16711680 ("Plot.Plot Color")] -> w3634
          frame False {
          }
          frame True {
          }
        }
        n1711 = case shown="True" "Show BG removed?" {
          tunnel: w3679 -> [w3738 w3754]
          tunnel: w3678 -> [_ w3744]
          tunnel: [w3738 w3753] -> w3671
          tunnel: w3677 -> [w3737 w3752]
          tunnel: [w3737 w3751] -> w3615
          tunnel: w3675 -> [_ w3740]
          tunnel: w3674 -> [w3736 w3750]
          tunnel: [w3736 w3749] -> w3666
          tunnel: w3672 -> [_ w3745]
          tunnel: [w3735 w3748] -> w3622
          tunnel: w3628 -> [_ w3742]
          tunnel: w3627 -> [w3735 w3747]
          frame False {
          }
          frame True {
            n1712 = Insert Into Array(array=w3750, index (row)=1, new element=w3745) -> (w3749:dbl[][])  [unwired: 1 in]
            n1713 = Insert Into Array(array=w3754, index (row)=1, new element=w3744) -> (w3753:dbl[][])  [unwired: 1 in]
            n1714 = Insert Into Array(array=w3752, index (row)=1, new element=w3740) -> (w3751:dbl[][])  [unwired: 1 in]
            n1715 = Insert Into Array(array=w3747, index (row)=1, new element=w3742) -> (w3748:dbl[][])  [unwired: 1 in]
          }
        }
        "Channel 1" <- w3671
        "Channel 2" <- w3615
        "Channel 3" <- w3666
        "Channel 4" <- w3622
        n1716 = case shown="False" w3643 {
          tunnel: [u32 16448250 ("Plot.Plot Color") u32 16711680 ("Plot.Plot Color")] -> w3642
          frame False {
          }
          frame True {
          }
        }
        n1717 = case shown="False" w3639 {
          tunnel: [u32 16448250 ("Plot.Plot Color") u32 16711680 ("Plot.Plot Color")] -> w3638
          frame False {
          }
          frame True {
          }
        }
        n1718 = case shown="False" w3623 {
          tunnel: [u32 16448250 ("Plot.Plot Color") u32 16711680 ("Plot.Plot Color")] -> w3619
          frame False {
          }
          frame True {
          }
        }
        n1719 = case shown="False" "Show BG removed?" {
          tunnel: [u32 16744703 ("Plot.Plot Color") u32 16741120 ("Plot.Plot Color")] -> w3612
          frame False {
          }
          frame True {
          }
        }
        n1720 = property on="Channel 1" class="WFGraph (strict)"("Active Plot"=w3613, "Plot.Plot Color"=w3612, "Plot.Line Style"=u8 1, "Plot.Line Width"=u8 2, "BG Color"=w3642) -> ()  [unwired: 2 in, 2 out]
        n1721 = property on="Channel 2" class="WFGraph (strict)"("Active Plot"=w3613, "Plot.Plot Color"=w3612, "Plot.Line Style"=u8 1, "Plot.Line Width"=u8 2, "BG Color"=w3638) -> ()  [unwired: 2 in, 2 out]
        n1722 = property on="Channel 4" class="WFGraph (strict)"("Active Plot"=w3613, "Plot.Plot Color"=w3612, "Plot.Line Style"=u8 1, "Plot.Line Width"=u8 2, "BG Color"=w3619) -> ()  [unwired: 2 in, 2 out]
        n1723 = property on="Channel 3" class="WFGraph (strict)"("Active Plot"=w3613, "Plot.Plot Color"=w3612, "Plot.Line Style"=u8 1, "Plot.Line Width"=u8 2, "BG Color"=w3634) -> ()  [unwired: 2 in, 2 out]
      }
      frame Error {
        w3755 = u32 16448250 ("Plot Area:Colors:BG Color")
        n1724 = property on="Channel 1" class="WFGraph (strict)"("BG Color"=w3755) -> ()  [unwired: 2 in, 2 out]
        n1725 = property on="Channel 2" class="WFGraph (strict)"("BG Color"=w3755) -> ()  [unwired: 2 in, 2 out]
        n1726 = property on="Channel 3" class="WFGraph (strict)"("BG Color"=w3755) -> ()  [unwired: 2 in, 2 out]
      }
    }
    "DisplayLoop" <- w3605
  }
  n1727 = disable-structure "Diagram Disable Structure" shown="Disabled" {
    frame Disabled {
      w3757 = T51 {"Horizontal"=500, "Vertical"=100}  # Top Left Corner
      n1728 = Control Help Window(0:w3757, 1:TRUE ("Show")) -> ()
      n1729 = call <vilib>:"TDMS - File Viewer.vi"() -> ()  [unwired: 6 in, 2 out]
    }
    frame Enabled {
    }
  }
  n1730 = while {
    tunnel: w19 -> [w3806]
    shift-right: [w3769] -> _
    shift-left: _ -> [w3802]
    tunnel: [w3760] -> w1 mode=indexing
    i -> [w3786]
    stop <- w3766 stop-if-true
    # "Channel 3"
    # "Channel 2"
    # "Channel 1"
    # "use FGV for gain value"
    # "stop on error"
    # "Gain adjustment and Data processing"
    n1731 = Tick Count (ms)() -> (millisecond timer value=w3769:u32)
    n1732 = Wait on Notification(notifier=w3806, ignore previous (F)=TRUE) -> (notification=w3780:T14, error out=w3759:errorcluster)  [unwired: 2 in, 2 out]
    n1733 = Subtract(x=w3769, y=w3802) -> (x-y=→"PID loop timing(ms)":u32)
    n1734 = Unbundle(w3780) -> ("CH1&2"=w3796:dbl[][], "CH3"=w3795:dbl[][])  [unwired: 2 out]
    n1735 = call "SeperateChanData.vi"("Input (Ch1&2)"=w3796) -> ("Ch1"=w3791:dbl[][], "Ch2"=w3789:dbl[][])
    n1736 = call "SeperateChanData.vi"("Input (Ch1&2)"=w3795) -> ("Ch1"=w3785:dbl[][], "Ch2"=w3778:dbl[][])
    n1737 = call "AvgArrayTimeCritical.vi"("2D array"=w3791) -> ("1D Avg"=w3790:dbl[])  [unwired: 10 in]
    n1738 = call "AvgArrayTimeCritical.vi"("2D array"=w3789) -> ("1D Avg"=w3800:dbl[])  [unwired: 10 in]
    n1739 = call "AvgArrayTimeCritical.vi"("2D array"=w3785) -> ("1D Avg"=w3797:dbl[])  [unwired: 10 in]
    n1740 = call "AvgArrayTimeCritical.vi"("2D array"=w3778) -> ("1D Avg"=w3777:dbl[])  [unwired: 10 in]
    n1741 = Array Max & Min(array=w3790) -> (max value=w3788:dbl)  [unwired: 3 out]
    n1742 = Array Max & Min(array=w3800) -> (max value=w3787:dbl)  [unwired: 3 out]
    n1743 = Array Max & Min(array=w3797) -> (max value=w3770:dbl)  [unwired: 3 out]
    n1744 = Array Max & Min(array=w3777) -> (max value=w3775:dbl)  [unwired: 3 out]
    n1745 = local read "Auto gain ch4"() -> (w3776:bool)
    n1746 = local read "Auto gain ch1"() -> (w3794:bool)
    n1747 = local read "Auto gain ch2"() -> (w3793:bool)
    n1748 = local read "Auto gain ch3"() -> (w3792:bool)
    n1749 = case shown="True" w3776 {
      tunnel: w3775 -> [_ w3853]
      tunnel: "V target(1.0)" -> [_ w3851]
      tunnel: [FALSE w3848] -> w3773
      tunnel: [0.0 ("CtrlV") w3843] -> w3774
      frame False {
        # "Manual control"
      }
      frame True {
        # "PID control"
        n1750 = global read "GlobalVariables.vi" "Ch4GainLim(Log)"() -> (w3854:cluster{"GainMax":dbl, "GainMin":dbl})
        n1751 = call-poly <vilib>:"PID.vi"("output range"=w3854, "PID gains"="Ch4 PID gains", "process variable"=w3853, "setpoint"=w3851) -> ("output"=w3852:dbl)  [unwired: 6 in, 1 out]
        n1752 = Power Of 10(x=w3852) -> (10^x=w3844:dbl)
        "Gain4" <- w3844
        n1753 = call "V4FGV.vi"("action(write)"=enum16{"write", "read"}."read") -> ("Error Out"=w3847:errorcluster, "V3 out"=w3849:dbl)  [unwired: 9 in]
        n1754 = call "GainToCtrlV.vi"("Gain"=w3844, "Channel"=enum16{"Ch1", "Ch2", "Ch3", "Ch4"}."Ch4") -> ("CtrlV"=w3843:dbl)  [unwired: 8 in, 1 out]
        n1755 = call "V4FGV.vi"("Error In"=w3847, "V3 in"=w3843) -> ()  [unwired: 8 in, 2 out]
        n1756 = local write "V 4"(w3843) -> ()
        n1757 = Not Equal?(x=w3843, y=w3849) -> (x != y?=w3848:bool)
      }
    }
    n1758 = case shown="True" w3794 {
      tunnel: "V target(1.0)" -> [_ w3868]
      tunnel: w3788 -> [_ w3865]
      tunnel: [0.0 ("CtrlV") w3857] -> w3767
      tunnel: [FALSE w3859] -> w3784
      frame False {
        # "Manual control"
      }
      frame True {
        # "PID control"
        n1759 = global read "GlobalVariables.vi" "Ch1GainLim(Log)"() -> (w3864:cluster{"GainMax":dbl, "GainMin":dbl})
        n1760 = call-poly <vilib>:"PID.vi"("output range"=w3864, "PID gains"="Ch1 PID gains", "process variable"=w3865, "setpoint"=w3868) -> ("output"=w3863:dbl)  [unwired: 6 in, 1 out]
        n1761 = Power Of 10(x=w3863) -> (10^x=w3862:dbl)
        "Gain1" <- w3862
        n1762 = call "V1FGV.vi"("action (write)"=enum16{"write", "read"}."read") -> ("Error Out"=w3858:errorcluster, "V1 out"=w3860:dbl)  [unwired: 9 in]
        n1763 = call "GainToCtrlV.vi"("Gain"=w3862, "Channel"=enum16{"Ch1", "Ch2", "Ch3"}."Ch1") -> ("CtrlV"=w3857:dbl)  [unwired: 8 in, 1 out]
        n1764 = local write "V 1"(w3857) -> ()
        n1765 = call "V1FGV.vi"("Error In"=w3858, "V1 in"=w3857) -> ()  [unwired: 8 in, 2 out]
        n1766 = Not Equal?(x=w3857, y=w3860) -> (x != y?=w3859:bool)
      }
    }
    n1767 = case shown="True" w3793 {
      tunnel: w3787 -> [_ w3895]
      tunnel: "V target(1.0)" -> [_ w3896]
      tunnel: [FALSE w3889] -> w3783
      tunnel: [0.0 ("CtrlV") w3885] -> w3779
      frame False {
        # "Manual control"
      }
      frame True {
        # "PID control"
        n1768 = global read "GlobalVariables.vi" "Ch2GainLim(Log)"() -> (w3893:cluster{"GainMax":dbl, "GainMin":dbl})
        n1769 = call-poly <vilib>:"PID.vi"("output range"=w3893, "PID gains"="Ch2 PID gains", "process variable"=w3895, "setpoint"=w3896) -> ("output"=w3892:dbl)  [unwired: 6 in, 1 out]
        n1770 = Power Of 10(x=w3892) -> (10^x=w3890:dbl)
        "Gain2" <- w3890
        n1771 = call "V2FGV.vi"("action(write)"=enum16{"write", "read"}."read") -> ("Error Out"=w3886:errorcluster, "V2 out"=w3887:dbl)  [unwired: 9 in]
        n1772 = call "GainToCtrlV.vi"("Gain"=w3890, "Channel"=enum16{"Ch1", "Ch2", "Ch3"}."Ch2") -> ("CtrlV"=w3885:dbl)  [unwired: 8 in, 1 out]
        n1773 = local write "V 2"(w3885) -> ()
        n1774 = call "V2FGV.vi"("Error In"=w3886, "V2 in"=w3885) -> ()  [unwired: 8 in, 2 out]
        n1775 = Not Equal?(x=w3885, y=w3887) -> (x != y?=w3889:bool)
      }
    }
    n1776 = case shown="True" w3792 {
      tunnel: w3770 -> [_ w3880]
      tunnel: "V target(1.0)" -> [_ w3877]
      tunnel: [FALSE w3873] -> w3782
      tunnel: [0.0 ("CtrlV") w3871] -> w3781
      frame False {
        # "Manual control"
      }
      frame True {
        # "PID control"
        n1777 = global read "GlobalVariables.vi" "Ch3GainLim(Log)"() -> (w3881:cluster{"GainMax":dbl, "GainMin":dbl})
        n1778 = call-poly <vilib>:"PID.vi"("output range"=w3881, "PID gains"="Ch3 PID gains", "process variable"=w3880, "setpoint"=w3877) -> ("output"=w3879:dbl)  [unwired: 6 in, 1 out]
        n1779 = Power Of 10(x=w3879) -> (10^x=w3876:dbl)
        "Gain3" <- w3876
        n1780 = call "V3FGV.vi"("action(write)"=enum16{"write", "read"}."read") -> ("Error Out"=w3872:errorcluster, "V3 out"=w3874:dbl)  [unwired: 9 in]
        n1781 = call "GainToCtrlV.vi"("Gain"=w3876, "Channel"=enum16{"Ch1", "Ch2", "Ch3"}."Ch3") -> ("CtrlV"=w3871:dbl)  [unwired: 8 in, 1 out]
        n1782 = local write "V 3"(w3871) -> ()
        n1783 = call "V3FGV.vi"("Error In"=w3872, "V3 in"=w3871) -> ()  [unwired: 8 in, 2 out]
        n1784 = Not Equal?(x=w3871, y=w3874) -> (x != y?=w3873:bool)
      }
    }
    n1785 = call "LabJack_FGV.vi"("Operation(Read)"=enum16{"Write", "Read"}."Read" ("Operation"), "error in (no error)"=w3759) -> ("error out"=w3768:errorcluster, "Read data"=w3804:i32)  [unwired: 8 in]
    n1786 = flat-sequence {
      tunnel: [w3808] -> w3765
      tunnel: w3759 -> [_]
      frame #0 {
        n1787 = Tick Count (ms)() -> (millisecond timer value=w3808:u32)
      }
    }
    n1788 = case "Channel 1" shown="True" w3784 {
      tunnel: w3768 -> [w3834 w3840]
      tunnel: w3804 -> [w3833 w3839]
      tunnel: [w3834 w3835] -> w3763
      tunnel: [w3833 w3838] -> w3799
      tunnel: w3767 -> [_ w3836]
      frame False {
        # "Do nothing"
      }
      frame True {
        # "request V\nupdate FGV"
        n1789 = global read "GlobalVariables.vi" "Ch1 LJ pin"() -> (w3837:string)
        n1790 = call "LJM_eWriteName.vi"("Handle In"=w3839, "Name"=w3837, "Value"=w3836, "error in"=w3840) -> ("Handle Out"=w3838:i32, "error out"=w3835:errorcluster)  [unwired: 10 in]
      }
    }
    n1791 = case "Channel 2" shown="True" w3783 {
      tunnel: w3763 -> [w3825 w3832]
      tunnel: [w3825 w3827] -> w3762
      tunnel: w3799 -> [w3826 w3831]
      tunnel: [w3826 w3830] -> w3798
      tunnel: w3779 -> [_ w3828]
      frame False {
        # "Do nothing"
      }
      frame True {
        # "request V\nupdate FGV"
        n1792 = global read "GlobalVariables.vi" "Ch2 LJ pin"() -> (w3829:string)
        n1793 = call "LJM_eWriteName.vi"("Handle In"=w3831, "Name"=w3829, "Value"=w3828, "error in"=w3832) -> ("Handle Out"=w3830:i32, "error out"=w3827:errorcluster)  [unwired: 10 in]
      }
    }
    n1794 = case "Channel 3" shown="True" w3782 {
      tunnel: w3762 -> [w3818 w3824]
      tunnel: [w3818 w3820] -> w3761
      tunnel: w3798 -> [w3817 w3823]
      tunnel: w3781 -> [_ w3821]
      tunnel: [w3817 w3819] -> w3772
      frame False {
        # "Do nothing"
      }
      frame True {
        # "request V\nupdate FGV"
        n1795 = global read "GlobalVariables.vi" "Ch3 LJ pin"() -> (w3822:string)
        n1796 = call "LJM_eWriteName.vi"("Handle In"=w3823, "Name"=w3822, "Value"=w3821, "error in"=w3824) -> ("Handle Out"=w3819:i32, "error out"=w3820:errorcluster)  [unwired: 10 in]
      }
    }
    n1797 = case "Channel 4" shown="True" w3773 {
      tunnel: w3761 -> [w3810 w3816]
      tunnel: w3772 -> [w3809 w3815]
      tunnel: [w3810 w3811] -> w3766
      tunnel: [w3809 w3814] -> _
      tunnel: w3774 -> [_ w3812]
      frame False {
        # "Do nothing"
      }
      frame True {
        # "request V\nupdate FGV"
        n1798 = global read "GlobalVariables.vi" "Ch4 LJ pin"() -> (w3813:string)
        n1799 = call "LJM_eWriteName.vi"("Handle In"=w3815, "Name"=w3813, "Value"=w3812, "error in"=w3816) -> ("Handle Out"=w3814:i32, "error out"=w3811:errorcluster)  [unwired: 10 in]
      }
    }
    "PID loop error out" <- w3766
    n1800 = flat-sequence {
      tunnel: [w3807] -> w3764
      tunnel: w3766 -> [_]
      frame #0 {
        n1801 = Tick Count (ms)() -> (millisecond timer value=w3807:u32)
      }
    }
    n1802 = Subtract(x=w3764, y=w3765) -> (x-y=w3760:u32)
    "LJ process (ms)" <- w3760
    "PID loop" <- w3786
  }
  "LJ time(ms)" <- w1
  n1803 = Release Notifier(notifier=w16, error in (no error)=w49) -> (error out=w50:errorcluster)  [unwired: 1 in, 2 out]
  n1804 = Release Notifier(notifier=w17, error in (no error)=w38) -> (error out=w43:errorcluster)  [unwired: 1 in, 2 out]
  n1805 = call <vilib>:"Simple Error Handler.vi"("error in (no error)"=w50) -> ()  [unwired: 4 in, 5 out]
  n1806 = call <vilib>:"Simple Error Handler.vi"("error in (no error)"=w43) -> ()  [unwired: 4 in, 5 out]
  n1807 = Unregister For Events(event registration refnum=w46, error in=w4) -> (error out=w52:errorcluster)
  n1808 = Destroy User Event(user event=w39, error in=w52) -> (error out=w3:errorcluster)
  n1809 = Close File(refnum=w21, error in=w3) -> ()  [unwired: 2 out]
  n1810 = Release Notifier(notifier=w59, error in (no error)=w58) -> (error out=w57:errorcluster)  [unwired: 1 in, 2 out]
  n1811 = Unregister For Events(event registration refnum=w63, error in=w61) -> (error out=w62:errorcluster)
  n1812 = call <vilib>:"Simple Error Handler.vi"("error in (no error)"=w57) -> ()  [unwired: 4 in, 5 out]
  n1813 = Destroy User Event(user event=w53, error in=w62) -> ()  [unwired: 1 out]
